vi "Lab Panel V4.8.vi"() -> ()   [LabVIEW 2013]
uses:
  <vilib>/Platform/TimedLoop/XDataNode/timing_clust.ctl
  <vilib>/Platform/TimedLoop/XDataNode/nitl_modes.ctl
  <vilib>/Platform/TimedLoop/XDataNode/wakeup.ctl
  Global 1.vi
  <vilib>/platform/TimedLoop/XDataNode/XDataNode.xnode
  <vilib>/Platform/TimedLoop/XDataNode/XDNodeRunTimeDep.lvlib
panel:
  in  "ADMIN PAGE":bool
  out "TEMP update":bool
  out "AI update":bool
  in  "Tab Control 2":T1(tab)
  out "SIG LAB05-2":T2 {"PF" format="%.2f"; "AMPS" format="%.1f"}
  out "SIG LAB05-1":T2 {"PF" format="%.2f"; "AMPS" format="%.1f"}
  out "SIG LAB04-2":T2 {"PF" format="%.2f"; "AMPS" format="%.1f"}
  out "SIG LAB04-1":T2 {"PF" format="%.2f"; "AMPS" format="%.1f"}
  out "SIG LAB03-2":T2 {"PF" format="%.2f"; "AMPS" format="%.1f"}
  out "SIG LAB03-1":T2 {"PF" format="%.2f"; "AMPS" format="%.1f"}
  out "SIG LAB02-2":T2 {"PF" format="%.2f"; "AMPS" format="%.1f"}
  in  "RUN LAB01-1":bool
  in  "O/I  LAB05-1":bool
  in  "O/I  LAB05-2":bool
  in  "O/I  LAB04-1":bool
  in  "O/I  LAB04-2":bool
  in  "O/I  LAB02-1":bool
  in  "O/I  LAB02-2":bool
  in  "O/I  LAB01-2":bool
  in  "O/I  LAB01-1":bool
  in  "O/I  LAB03-1":bool
  in  "RUN LAB05-2":bool
  in  "RUN LAB05-1":bool
  in  "RUN LAB04-2":bool
  in  "RUN LAB04-1":bool
  in  "RUN LAB03-2":bool
  in  "RUN LAB03-1":bool
  in  "RUN LAB02-2":bool
  in  "RUN LAB02-1":bool
  in  "RUN LAB01-2":bool
  in  "SELECT LAB05-2":T3(radio)
  in  "SELECT LAB05-1":T3(radio)
  in  "SELECT LAB04-2":T3(radio)
  in  "SELECT LAB04-1":T3(radio)
  in  "SELECT LAB03-2":T3(radio)
  in  "SELECT LAB03-1":T3(radio)
  in  "SELECT LAB02-2":T3(radio)
  in  "SELECT LAB02-1":T3(radio)
  in  "SELECT LAB01-2":T3(radio)
  in  "SELECT LAB01-1":T3(radio)
  in  "O/I  LAB03-2":bool
  out "SIG LAB01-1":T2 {"PF" format="%.2f"; "AMPS" format="%.1f"}
  out "SIG LAB01-2":T2 {"PF" format="%.2f"; "AMPS" format="%.1f"}
  out "SIG LAB02-1":T2 {"PF" format="%.2f"; "AMPS" format="%.1f"}
  out "DISP LAB05-2":T4 {"MINS" format="%.2g"}
  out "DISP LAB05-1":T4 {"MINS" format="%.2g"}
  out "DISP LAB04-2":T4 {"MINS" format="%.2g"}
  out "DISP LAB04-1":T4 {"MINS" format="%.2g"}
  out "DISP LAB03-2":T4 {"MINS" format="%.2g"}
  out "DISP LAB03-1":T4 {"MINS" format="%.2g"}
  in  "SET LAB05-2":T5={"NAME"="", "DESCRIPTION"="", "CYCLES"=5.0, "T-RISE mins"=0.0, "T-RISE deg C"=0.0} {"CYCLES" min=5.0 step=1.0}
  in  "SET LAB05-1":T5={"NAME"="", "DESCRIPTION"="", "CYCLES"=5.0, "T-RISE mins"=0.0, "T-RISE deg C"=0.0} {"CYCLES" min=5.0 step=1.0}
  in  "SET LAB04-2":T5={"NAME"="", "DESCRIPTION"="", "CYCLES"=5.0, "T-RISE mins"=0.0, "T-RISE deg C"=0.0} {"CYCLES" min=5.0 step=1.0}
  in  "SET LAB04-1":T5={"NAME"="", "DESCRIPTION"="", "CYCLES"=5.0, "T-RISE mins"=0.0, "T-RISE deg C"=0.0} {"CYCLES" min=5.0 step=1.0}
  in  "SET LAB03-2":T5={"NAME"="", "DESCRIPTION"="", "CYCLES"=5.0, "T-RISE mins"=0.0, "T-RISE deg C"=0.0} {"CYCLES" min=5.0 step=1.0}
  in  "SET LAB03-1":T5={"NAME"="", "DESCRIPTION"="", "CYCLES"=5.0, "T-RISE mins"=0.0, "T-RISE deg C"=0.0} {"CYCLES" min=5.0 step=1.0}
  out "DISP LAB02-2":T4 {"MINS" format="%.2g"}
  out "DISP LAB02-1":T4 {"MINS" format="%.2g"}
  in  "SET LAB02-2":T5={"NAME"="", "DESCRIPTION"="", "CYCLES"=5.0, "T-RISE mins"=0.0, "T-RISE deg C"=0.0} {"CYCLES" min=5.0 step=1.0}
  in  "SET LAB02-1":T5={"NAME"="", "DESCRIPTION"="", "CYCLES"=5.0, "T-RISE mins"=0.0, "T-RISE deg C"=0.0} {"CYCLES" min=5.0 step=1.0}
  out "RESULT LAB05-2":bool
  out "RESULT LAB05-1":bool
  out "RESULT LAB04-2":bool
  out "RESULT LAB04-1":bool
  out "RESULT LAB03-2":bool
  out "RESULT LAB03-1":bool
  out "RESULT LAB02-2":bool
  out "RESULT LAB02-1":bool
  out "RESULT LAB01-2":bool
  out "RESULT LAB01-1":bool
  in  "SET LAB01-1":T5={"NAME"="", "DESCRIPTION"="", "CYCLES"=5.0, "T-RISE mins"=0.0, "T-RISE deg C"=0.0} {"CYCLES" min=5.0 step=1.0}
  in  "SET LAB01-2":T5={"NAME"="", "DESCRIPTION"="", "CYCLES"=5.0, "T-RISE mins"=0.0, "T-RISE deg C"=0.0} {"CYCLES" min=5.0 step=1.0}
  out "DISP LAB01-1":T4 {"MINS" format="%.2g"}
  out "DISP LAB01-2":T4 {"MINS" format="%.2f"}
  out "TEMP RISE LAB05-2":cluster{"TL":dbl, "TN":dbl}
  out "TEMP RISE LAB05-1":cluster{"TL":dbl, "TN":dbl}
  out "TEMP RISE LAB04-2":cluster{"TL":dbl, "TN":dbl}
  out "TEMP RISE LAB04-1":cluster{"TL":dbl, "TN":dbl}
  out "TEMP RISE LAB03-2":cluster{"TL":dbl, "TN":dbl}
  out "TEMP RISE LAB03-1":cluster{"TL":dbl, "TN":dbl}
  out "TEMP RISE LAB02-2":cluster{"TL":dbl, "TN":dbl}
  out "TEMP RISE LAB02-1":cluster{"TL":dbl, "TN":dbl}
  out "TEMP RISE LAB01-2":cluster{"TL":dbl, "TN":dbl}
  out "TEMP RISE LAB01-1":cluster{"TL":dbl, "TN":dbl}
  in  "JIG OFF TIME (S)":dbl=2.0 min=2.0 max=10.0 step=0.5 format="%.1g"
  in  "JIG ON TIME (S)":dbl=1.0 min=1.0 max=10.0 step=0.5 format="%.1g"
  out "JIG LAB05-2":bool
  out "JIG LAB05-1":bool
  out "JIG LAB04-2":bool
  out "JIG LAB04-1":bool
  out "JIG LAB03-2":bool
  out "JIG LAB03-1":bool
  out "JIG LAB02-2":bool
  out "JIG LAB02-1":bool
  out "JIG LAB01-2":bool
  out "JIG LAB01-1":bool
  out "TEMP START LAB01-1":cluster{"TL":dbl, "TN":dbl}
  out "TEMP START LAB02-1":cluster{"TL":dbl, "TN":dbl}
  out "TEMP START LAB03-1":cluster{"TL":dbl, "TN":dbl}
  out "TEMP START LAB04-1":cluster{"TL":dbl, "TN":dbl}
  out "TEMP START LAB01-2":cluster{"TL":dbl, "TN":dbl}
  out "TEMP START LAB02-2":cluster{"TL":dbl, "TN":dbl}
  out "TEMP START LAB03-2":cluster{"TL":dbl, "TN":dbl}
  out "TEMP START LAB04-2":cluster{"TL":dbl, "TN":dbl}
  out "TEMP START LAB05-2":cluster{"TL":dbl, "TN":dbl}
  out "TEMP START LAB05-1":cluster{"TL":dbl, "TN":dbl}
  out "TEST VOLTS CHART":T6(graph)
  in  "Select  Cycle":enum32{"ON CYCLE", "OFF CYCLE"}(radio)
  out "TEST AMPS CHART":T6(graph)
  out "TEMPERATURE (N) CHART":T6(graph)
  out "TEMPERATURE (L) CHART":T6(graph)
  out "Message":string
  in  "MAIL SETTINGS":T7
  out "MAIL REPORT":string
  in  "TO (string):":string
  in  "Send Mail Now":bool
  in  "Auto Mail Send":bool
  in  "Network Directory":path
  out "CAL LAB01":T8 {"2 (TN) cal" min=0.0 step=0.01 format="%.2f"; "2 (TL) cal" min=0.0 step=0.01 format="%.2f"; "2 (PF) cal" min=0.0 step=0.01 format="%.2f"; "2 (V) cal" min=0.0 step=0.01 format="%.2f"; "2 (A) cal" min=0.0 step=0.01 format="%.2f"; "1 (TN) cal" min=0.0 step=0.01 format="%.2f"; "1 (TL) cal" min=0.0 step=0.01 format="%.2f"; "1 (PF) cal" min=0.0 step=0.01 format="%.2f"; "1 (V) cal" min=0.0 step=0.01 format="%.2f"; "1  (A) cal" min=0.0 step=0.01 format="%.2f"}
  out "CAL LAB03":T8 {"2 (TN) cal" min=0.0 step=0.01 format="%.2f"; "2 (TL) cal" min=0.0 step=0.01 format="%.2f"; "2 (PF) cal" min=0.0 step=0.01 format="%.2f"; "2 (V) cal" min=0.0 step=0.01 format="%.2f"; "2 (A) cal" min=0.0 step=0.01 format="%.2f"; "1 (TN) cal" min=0.0 step=0.01 format="%.2f"; "1 (TL) cal" min=0.0 step=0.01 format="%.2f"; "1 (PF) cal" min=0.0 step=0.01 format="%.2f"; "1 (V) cal" min=0.0 step=0.01 format="%.2f"; "1  (A) cal" min=0.0 step=0.01 format="%.2f"}
  out "CAL LAB02":T9 {"2 (TN) cal" min=0.0 step=0.01 format="%.2f"; "2 (TL) cal" min=0.0 step=0.01 format="%.2f"; "2 (PF) cal" min=0.0 step=0.01 format="%.2f"; "2 (V) cal" min=0.0 step=0.01 format="%.2f"; "2 (A) cal" min=0.0 step=0.01 format="%.2f"; "1 (TN) cal" min=0.0 step=0.01 format="%.2f"; "1 (TL) cal" min=0.0 step=0.01 format="%.2f"; "1 (PF) cal" min=0.0 step=0.01 format="%.2f"; "1 (V) cal" min=0.0 step=0.01 format="%.2f"; "1 (A) cal" min=0.0 step=0.01 format="%.2f"}
  out "CAL LAB05":T8 {"2 (TN) cal" min=0.0 step=0.01 format="%.2f"; "2 (TL) cal" min=0.0 step=0.01 format="%.2f"; "2 (PF) cal" min=0.0 step=0.01 format="%.2f"; "2 (V) cal" min=0.0 step=0.01 format="%.2f"; "2 (A) cal" min=0.0 step=0.01 format="%.2f"; "1 (TN) cal" min=0.0 step=0.01 format="%.2f"; "1 (TL) cal" min=0.0 step=0.01 format="%.2f"; "1 (PF) cal" min=0.0 step=0.01 format="%.2f"; "1 (V) cal" min=0.0 step=0.01 format="%.2f"; "1  (A) cal" min=0.0 step=0.01 format="%.2f"}
  out "CAL LAB04":T8 {"2 (TN) cal" min=0.0 step=0.01 format="%.2f"; "2 (TL) cal" min=0.0 step=0.01 format="%.2f"; "2 (PF) cal" min=0.0 step=0.01 format="%.2f"; "2 (V) cal" min=0.0 step=0.01 format="%.2f"; "2 (A) cal" min=0.0 step=0.01 format="%.2f"; "1 (TN) cal" min=0.0 step=0.01 format="%.2f"; "1 (TL) cal" min=0.0 step=0.01 format="%.2f"; "1 (PF) cal" min=0.0 step=0.01 format="%.2f"; "1 (V) cal" min=0.0 step=0.01 format="%.2f"; "1  (A) cal" min=0.0 step=0.01 format="%.2f"}
  out "calibration file error out":errorcluster
  in  "CALIBRATE":bool
  out "JIG RELAY CYCLES":T10
  out "ON L05-2":cluster{"amps":dbl, "volts":dbl, "pf":dbl}
  out "ON L05-1":cluster{"amps":dbl, "volts":dbl, "pf":dbl}
  out "FAIL LAB05-2":cluster{"LO":dbl, "HI":dbl}
  out "FAIL LAB05-1":cluster{"LO":dbl, "HI":dbl}
  out "FAIL LAB04-2":cluster{"LO":dbl, "HI":dbl}
  out "FAIL LAB04-1":cluster{"LO":dbl, "HI":dbl}
  out "FAIL LAB03-2":cluster{"LO":dbl, "HI":dbl}
  out "FAIL LAB03-1":cluster{"LO":dbl, "HI":dbl}
  out "FAIL LAB02-2":cluster{"LO":dbl, "HI":dbl}
  out "FAIL LAB02-1":cluster{"LO":dbl, "HI":dbl}
  out "FAIL LAB01-2":cluster{"LO":dbl, "HI":dbl}
  out "FAIL LAB01-1":cluster{"LO":dbl, "HI":dbl}
  out "ON L01-1":cluster{"amps":dbl, "volts":dbl, "pf":dbl}
  out "ON L01-2":cluster{"amps":dbl, "volts":dbl, "pf":dbl}
  out "ON L02-1":cluster{"amps":dbl, "volts":dbl, "pf":dbl}
  out "ON L02-2":cluster{"amps":dbl, "volts":dbl, "pf":dbl}
  out "ON L03-1":cluster{"amps":dbl, "volts":dbl, "pf":dbl}
  out "ON L03-2":cluster{"amps":dbl, "volts":dbl, "pf":dbl}
  out "ON L04-1":cluster{"amps":dbl, "volts":dbl, "pf":dbl}
  out "ON L04-2":cluster{"amps":dbl, "volts":dbl, "pf":dbl}
  out "TEMP LA05":T11
  out "TEMP LA04":T11
  out "TEMP LA03":T11
  out "TEMP LA02":T11
  out "TEMP LA01":T11
  in  "Fail Loops":dbl
  out "Save JC":bool
  out "simulate":bool
  in  "Temp Value":dbl
  in  "Temp Delay Lps":dbl
  in  "SAMPLES":dbl
  in  "RATE (Hz)":dbl
  in  "JIG TEST":T12
  in  "C drive data root dir":path
  out "run lab05-2":bool
  out "run lab05-1":bool
  out "run lab04-2":bool
  out "run lab04-1":bool
  out "run lab03-2":bool
  out "run lab03-1":bool
  out "run lab02-2":bool
  out "run lab02-1":bool
  out "run lab01-2":bool
  out "run lab01-1":bool
  in  "Tab Control":T13(tab)
  out "LAB01-2 (GRAPH)":dynamicdata(graph)
  out "LAB01-1 (GRAPH)":dynamicdata(graph)
  out "LAB02-2 (GRAPH)":dynamicdata(graph)
  out "LAB02-1 (GRAPH)":dynamicdata(graph)
  out "LAB03-2 (GRAPH)":dynamicdata(graph)
  out "LAB03-1 (GRAPH)":dynamicdata(graph)
  out "LAB04-2 (GRAPH)":dynamicdata(graph)
  out "LAB04-1 (GRAPH)":dynamicdata(graph)
  out "LAB05-2 (GRAPH)":dynamicdata(graph)
  out "LAB05-1 (GRAPH)":dynamicdata(graph)
  out "LAB05 TEMP":T14
  out "LAB04 TEMP":T14
  out "LAB02 TEMP":T14
  out "LAB01 TEMP":T14
  out "LAB03 TEMP":T14
  out "Analog Error Array":errorcluster[](array[cluster])
  out "AI loop time":dbl format="%.6g"
  out "loops":dbl
  in  "loop  delay(mS)":dbl
  out "on loops":dbl
  out "off loops":dbl
  out "jig cycle":dbl
  out "TDMS LAB01-1":refnum<k34>
  out "data file error":errorcluster
  out "TDMS LAB02-1":refnum<k34>
  out "TDMS LAB01-2":refnum<k34>
  out "TDMS LAB02-2":refnum<k34>
  out "TDMS LAB03-1":refnum<k34>
  out "TDMS LAB03-2":refnum<k34>
  out "TDMS LAB04-1":refnum<k34>
  out "TDMS LAB04-2":refnum<k34>
  out "TDMS LAB05-1":refnum<k34>
  out "TDMS LAB05-2":refnum<k34>
  out "mail control":string
  out "File Time Stamp":timestamp
  in  "stop":bool
  in  "Select COM port":refnum<visa-resource-name>="COM6"
  out "COM port":refnum<visa-resource-name>="COM6"
  # "LAB01"
  # "LAB02"
  # "LAB05"
  # "LAB03"
  # "LAB04"
  # "LAB01"
  # "LAB02"
  # "LAB03"
  # "LAB04"
  # "LAB05"
  # "JIG SET"
  # "(Enter recipients address seperated by comma)"
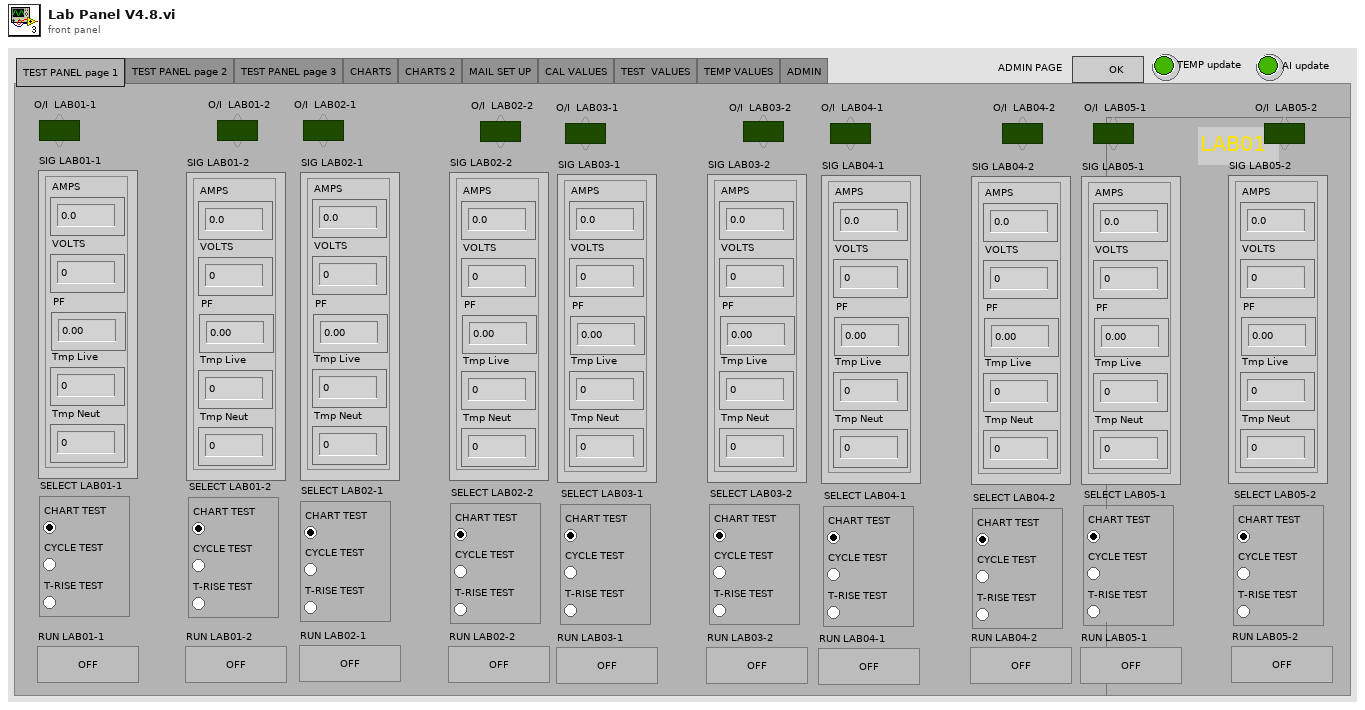
[diagram p1: front panel]
types:
  T1 = enum32{"TEST PANEL page 1", "TEST PANEL page 2", "TEST PANEL page 3", "CHARTS", "CHARTS 2", "MAIL SET UP", "CAL VALUES", "TEST  VALUES", "TEMP VALUES", "ADMIN"}
  T2 = cluster{"AMPS":dbl, "VOLTS":dbl, "PF":dbl, "Tmp Live":dbl, "Tmp Neut":dbl}
  T3 = enum32{"CHART TEST", "CYCLE TEST", "T-RISE TEST"}
  T4 = cluster{"CYCLE":dbl, "MINS":dbl, "STATUS":string}
  T5 = cluster{"NAME":string, "DESCRIPTION":string, "CYCLES":dbl, "T-RISE mins":dbl, "T-RISE deg C":dbl}
  T6 = cluster{"AMPS":dbl, "AMPS":dbl, "AMPS":dbl, "AMPS":dbl, "AMPS":dbl, "AMPS":dbl, "AMPS":dbl, "AMPS":dbl, "AMPS":dbl, "AMPS":dbl}
  T7 = cluster{"OUT SERVER ADDRESS":string, "FROM ACCOUNT":string, "USER NAME":string, "PASSWORD":string, "TEST MAIL":bool, "TEST MAIL STATUS":string, "mail error":errorcluster}
  T8 = cluster{"1  (A) cal":dbl, "1 (V) cal":dbl, "1 (PF) cal":dbl, "1 (TL) cal":dbl, "1 (TN) cal":dbl, "2 (A) cal":dbl, "2 (V) cal":dbl, "2 (PF) cal":dbl, "2 (TL) cal":dbl, "2 (TN) cal":dbl}
  T9 = cluster{"1 (A) cal":dbl, "1 (V) cal":dbl, "1 (PF) cal":dbl, "1 (TL) cal":dbl, "1 (TN) cal":dbl, "2 (A) cal":dbl, "2 (V) cal":dbl, "2 (PF) cal":dbl, "2 (TL) cal":dbl, "2 (TN) cal":dbl}
  T10 = cluster{"LAB01-1":dbl, "LAB01-2":dbl, "LAB02-1":dbl, "LAB02-2":dbl, "LAB03-1":dbl, "LAB03-2":dbl, "LAB04-1":dbl, "LAB04-2":dbl, "LAB05-1":dbl, "LAB05-2":dbl}
  T11 = cluster{"TL-1":dbl, "TN-1":dbl, "TL-2":dbl, "TN-2":dbl, "TL -1COUNT":dbl, "TN-1 COUNT":dbl, "TL-2 COUNT":dbl, "TN-2 COUNT":dbl}
  T12 = cluster{" LAB01-1":bool, " LAB01-2":bool, "LAB02-1":bool, " LAB02-2":bool, "LAB03-1":bool, "LAB03-2":bool, "LAB04-1":bool, "LAB04-2":bool, "LAB05-1":bool, "LAB05-2":bool}
  T13 = enum32{"LAB01", "LAB02", "LAB03", "LAB04", "LAB05", "TEMPERATURE", "ERROR"}
  T14 = cluster{"T1 Live":dbl, "T1 Neut":dbl, "T2 Live":dbl, "T2 Neut":dbl, "ID":dbl, "ER":dbl}
  T15 = enum8{"Enabled", "Disabled", "Disabled and Grayed Out"}
  T16 = typedef "XDNodeRunTimeDep.lvlib/timing_clust.ctl" = cluster{"Expected End [f-1]":u64, "Actual End [f-1]":u64, "Finished Late? [f-1]":bool, "Expected End [i-1]":u64, "Actual End [i-1]":u64, "Finished Late? [i-1]":bool, "Expected Start [i]":u64, "Actual Start [i]":u64, "Expected Start [f]":u64, "Actual Start [f]":u64, "Source Name":string, "Structure Name":string, "Period":i64, "Deadline":i64, "Offset":i64, "Start":i64, "Priority":i32, "Timeout":i32, "Mode":T17, "Wakeup Reason":T18, "Error":errorcluster, "Source Type":string, "Secondary Source Type":string, "Global End Time":u64, "Global Start Time":u64, "Frame Duration":u64, "Iteration Duration":u64, "Assigned CPU":i32, "I/O Scan Engine Mode":u32}
  T17 = typedef "XDNodeRunTimeDep.lvlib/nitl_modes.ctl" = enum32{"No Change", "Process missed periods, maintain original phase", "Discard missed periods, maintain original phase", "Process missed periods, ignore original phase", "Discard missed periods, ignore original phase"}
  T18 = typedef "XDNodeRunTimeDep.lvlib/wakeup.ctl" = enum32{"Normal", "Aborted", "Asynchronous wakeup", "Timing source error", "Timed loop error", "Timeout"}
  T19 = enum16{"open", "open or create", "create or replace", "create", "open (read-only)"}
  T20 = enum16{"open", "replace", "create", "open or create", "replace or create", "replace or create with confirmation"}
  T21 = cluster{"SET LAB01-1":cluster{"NAME":string, "DESCRIPTION":string, "CYCLES":dbl, "T-RISE mins":dbl, "T-RISE deg C":dbl}, "SET LAB01-2":cluster{"NAME":string, "DESCRIPTION":string, "CYCLES":dbl, "T-RISE mins":dbl, "T-RISE deg C":dbl}, "SET LAB02-1":cluster{"NAME":string, "DESCRIPTION":string, "CYCLES":dbl, "T-RISE mins":dbl, "T-RISE deg C":dbl}, "SET LAB02-2":cluster{"NAME":string, "DESCRIPTION":string, "CYCLES":dbl, "T-RISE mins":dbl, "T-RISE deg C":dbl}, "SET LAB03-1":cluster{"NAME":string, "DESCRIPTION":string, "CYCLES":dbl, "T-RISE mins":dbl, "T-RISE deg C":dbl}, "SET LAB03-2":cluster{"NAME":string, "DESCRIPTION":string, "CYCLES":dbl, "T-RISE mins":dbl, "T-RISE deg C":dbl}, "SET LAB04-1":cluster{"NAME":string, "DESCRIPTION":string, "CYCLES":dbl, "T-RISE mins":dbl, "T-RISE deg C":dbl}, "SET LAB04-2":cluster{"NAME":string, "DESCRIPTION":string, "CYCLES":dbl, "T-RISE mins":dbl, "T-RISE deg C":dbl}, "SET LAB05-1":cluster{"NAME":string, "DESCRIPTION":string, "CYCLES":dbl, "T-RISE mins":dbl, "T-RISE deg C":dbl}, "SET LAB05-2":cluster{"NAME":string, "DESCRIPTION":string, "CYCLES":dbl, "T-RISE mins":dbl, "T-RISE deg C":dbl}, "Network Directory":path, "C drive data root dir":path, "RATE (Hz)":dbl, "SAMPLES":dbl, "Select COM port":refnum<visa-resource-name>, "Temp Delay Lps":dbl, "Temp Value":dbl, "Fail Loops":dbl}
  T22 = cluster{"MAIL SETTINGS":cluster{"OUT SERVER ADDRESS":string, "FROM ACCOUNT":string, "USER NAME":string, "PASSWORD":string, "TEST MAIL":bool, "TEST MAIL STATUS":string, "mail error":errorcluster}, "Auto Mail Send":bool, string}
  T23 = cluster{"T1":dbl, "T2":dbl, "T3":dbl, "T4":dbl, "ID":dbl, "ER":dbl}
  T24 = cluster{"TP1-L":dbl, "TP1-N":dbl, "TP2-L":dbl, "TP2-N":dbl, "TP1-L COUNT":dbl, "TP1-N COUNT":dbl, "TP2-L COUNT":dbl, "TP2-N COUNT":dbl}
  T25 = cluster{"LAB01-1 (A)":dbl, "LAB01-1 (V)":dbl, "LAB01-1 (PF)":dbl, "LAB01-2 (A)":dbl, "LAB01-2 (V)":dbl, "LAB01-2 (PF)":dbl}
  T26 = cluster{"LAB02-1 (A)":dbl, "LAB02-1 (V)":dbl, "LAB02-1 (PF)":dbl, "LAB02-2 (A)":dbl, "LAB02-2 (V)":dbl, "LAB02-2 (PF)":dbl}
  T27 = cluster{"LAB03-1 (A)":dbl, "LAB03-1 (V)":dbl, "LAB03-1 (PF)":dbl, "LAB03-2 (A)":dbl, "LAB03-2 (V)":dbl, "LAB03-2 (PF)":dbl}
  T28 = cluster{"LAB04-1 (A)":dbl, "LAB04-1 (V)":dbl, "LAB04-1 (PF)":dbl, "LAB04-2 (A)":dbl, "LAB04-2 (V)":dbl, "LAB04-2 (PF)":dbl}
  T29 = cluster{"LAB05-1 (A)":dbl, "LAB05-1 (V)":dbl, "LAB05-1 (PF)":dbl, "LAB05-2 (A)":dbl, "LAB05-2 (V)":dbl, "LAB05-2 (PF)":dbl}
  T30 = cluster{"VOLTS":dbl, "VOLTS":dbl, "VOLTS":dbl, "VOLTS":dbl, "VOLTS":dbl, "VOLTS":dbl, "VOLTS":dbl, "VOLTS":dbl, "VOLTS":dbl, "VOLTS":dbl}
  T31 = cluster{"Tmp Live":dbl, "Tmp Live":dbl, "Tmp Live":dbl, "Tmp Live":dbl, "Tmp Live":dbl, "Tmp Live":dbl, "Tmp Live":dbl, "Tmp Live":dbl, "Tmp Live":dbl, "Tmp Live":dbl}
  T32 = cluster{"Tmp Neut":dbl, "Tmp Neut":dbl, "Tmp Neut":dbl, "Tmp Neut":dbl, "Tmp Neut":dbl, "Tmp Neut":dbl, "Tmp Neut":dbl, "Tmp Neut":dbl, "Tmp Neut":dbl, "Tmp Neut":dbl}
  T33 = cluster{"FAIL LAB01-1":cluster{"LO":dbl, "HI":dbl}, "SIG LAB01-1":cluster{"AMPS":dbl, "VOLTS":dbl, "PF":dbl, "Tmp Live":dbl, "Tmp Neut":dbl}, "TEMP START LAB01-1":cluster{"TL":dbl, "TN":dbl}, "DISP LAB01-1":cluster{"CYCLE":dbl, "MINS":dbl, "STATUS":string}, "SET LAB01-1":cluster{"NAME":string, "DESCRIPTION":string, "CYCLES":dbl, "T-RISE mins":dbl, "T-RISE deg C":dbl}, "TDMS LAB01-1":refnum<k34>}
  T34 = cluster{"FAIL LAB01-2":cluster{"LO":dbl, "HI":dbl}, "SIG LAB01-2":cluster{"AMPS":dbl, "VOLTS":dbl, "PF":dbl, "Tmp Live":dbl, "Tmp Neut":dbl}, "TEMP START LAB01-2":cluster{"TL":dbl, "TN":dbl}, "DISP LAB01-2":cluster{"CYCLE":dbl, "MINS":dbl, "STATUS":string}, "SET LAB01-2":cluster{"NAME":string, "DESCRIPTION":string, "CYCLES":dbl, "T-RISE mins":dbl, "T-RISE deg C":dbl}, "TDMS LAB01-2":refnum<k34>}
  T35 = cluster{"FAIL LAB02-1":cluster{"LO":dbl, "HI":dbl}, "SIG LAB02-1":cluster{"AMPS":dbl, "VOLTS":dbl, "PF":dbl, "Tmp Live":dbl, "Tmp Neut":dbl}, "TEMP START LAB02-1":cluster{"TL":dbl, "TN":dbl}, "DISP LAB02-1":cluster{"CYCLE":dbl, "MINS":dbl, "STATUS":string}, "SET LAB02-1":cluster{"NAME":string, "DESCRIPTION":string, "CYCLES":dbl, "T-RISE mins":dbl, "T-RISE deg C":dbl}, "TDMS LAB02-1":refnum<k34>}
  T36 = cluster{"FAIL LAB02-2":cluster{"LO":dbl, "HI":dbl}, "SIG LAB02-2":cluster{"AMPS":dbl, "VOLTS":dbl, "PF":dbl, "Tmp Live":dbl, "Tmp Neut":dbl}, "TEMP START LAB02-2":cluster{"TL":dbl, "TN":dbl}, "DISP LAB02-2":cluster{"CYCLE":dbl, "MINS":dbl, "STATUS":string}, "SET LAB02-2":cluster{"NAME":string, "DESCRIPTION":string, "CYCLES":dbl, "T-RISE mins":dbl, "T-RISE deg C":dbl}, "TDMS LAB02-2":refnum<k34>}
  T37 = cluster{"FAIL LAB03-1":cluster{"LO":dbl, "HI":dbl}, "SIG LAB03-1":cluster{"AMPS":dbl, "VOLTS":dbl, "PF":dbl, "Tmp Live":dbl, "Tmp Neut":dbl}, "TEMP START LAB03-1":cluster{"TL":dbl, "TN":dbl}, "DISP LAB03-1":cluster{"CYCLE":dbl, "MINS":dbl, "STATUS":string}, "SET LAB03-1":cluster{"NAME":string, "DESCRIPTION":string, "CYCLES":dbl, "T-RISE mins":dbl, "T-RISE deg C":dbl}, "TDMS LAB03-1":refnum<k34>}
  T38 = cluster{"FAIL LAB03-2":cluster{"LO":dbl, "HI":dbl}, "SIG LAB03-2":cluster{"AMPS":dbl, "VOLTS":dbl, "PF":dbl, "Tmp Live":dbl, "Tmp Neut":dbl}, "TEMP START LAB03-2":cluster{"TL":dbl, "TN":dbl}, "DISP LAB03-2":cluster{"CYCLE":dbl, "MINS":dbl, "STATUS":string}, "SET LAB03-2":cluster{"NAME":string, "DESCRIPTION":string, "CYCLES":dbl, "T-RISE mins":dbl, "T-RISE deg C":dbl}, "TDMS LAB03-2":refnum<k34>}
  T39 = cluster{"FAIL LAB04-1":cluster{"LO":dbl, "HI":dbl}, "SIG LAB04-1":cluster{"AMPS":dbl, "VOLTS":dbl, "PF":dbl, "Tmp Live":dbl, "Tmp Neut":dbl}, "TEMP START LAB04-1":cluster{"TL":dbl, "TN":dbl}, "DISP LAB04-1":cluster{"CYCLE":dbl, "MINS":dbl, "STATUS":string}, "SET LAB04-1":cluster{"NAME":string, "DESCRIPTION":string, "CYCLES":dbl, "T-RISE mins":dbl, "T-RISE deg C":dbl}, "TDMS LAB04-1":refnum<k34>}
  T40 = cluster{"FAIL LAB04-2":cluster{"LO":dbl, "HI":dbl}, "SIG LAB04-2":cluster{"AMPS":dbl, "VOLTS":dbl, "PF":dbl, "Tmp Live":dbl, "Tmp Neut":dbl}, "TEMP START LAB04-2":cluster{"TL":dbl, "TN":dbl}, "DISP LAB04-2":cluster{"CYCLE":dbl, "MINS":dbl, "STATUS":string}, "SET LAB04-2":cluster{"NAME":string, "DESCRIPTION":string, "CYCLES":dbl, "T-RISE mins":dbl, "T-RISE deg C":dbl}, "TDMS LAB04-2":refnum<k34>}
  T41 = cluster{"FAIL LAB05-1":cluster{"LO":dbl, "HI":dbl}, "SIG LAB05-1":cluster{"AMPS":dbl, "VOLTS":dbl, "PF":dbl, "Tmp Live":dbl, "Tmp Neut":dbl}, "TEMP START LAB05-1":cluster{"TL":dbl, "TN":dbl}, "DISP LAB05-1":cluster{"CYCLE":dbl, "MINS":dbl, "STATUS":string}, "SET LAB05-1":cluster{"NAME":string, "DESCRIPTION":string, "CYCLES":dbl, "T-RISE mins":dbl, "T-RISE deg C":dbl}, "TDMS LAB05-1":refnum<k34>}
  T42 = cluster{"FAIL LAB05-2":cluster{"LO":dbl, "HI":dbl}, "SIG LAB05-2":cluster{"AMPS":dbl, "VOLTS":dbl, "PF":dbl, "Tmp Live":dbl, "Tmp Neut":dbl}, "TEMP START LAB05-2":cluster{"TL":dbl, "TN":dbl}, "DISP LAB05-2":cluster{"CYCLE":dbl, "MINS":dbl, "STATUS":string}, "SET LAB05-2":cluster{"NAME":string, "DESCRIPTION":string, "CYCLES":dbl, "T-RISE mins":dbl, "T-RISE deg C":dbl}, "TDMS LAB05-2":refnum<k34>}
  T43 = cluster{"MAIL SETTINGS":cluster{"OUT SERVER ADDRESS":string, "FROM ACCOUNT":string, "USER NAME":string, "PASSWORD":string, "TEST MAIL":bool, "TEST MAIL STATUS":string, "mail error":errorcluster}, "Auto Mail Send":bool, "TO (string):":string}
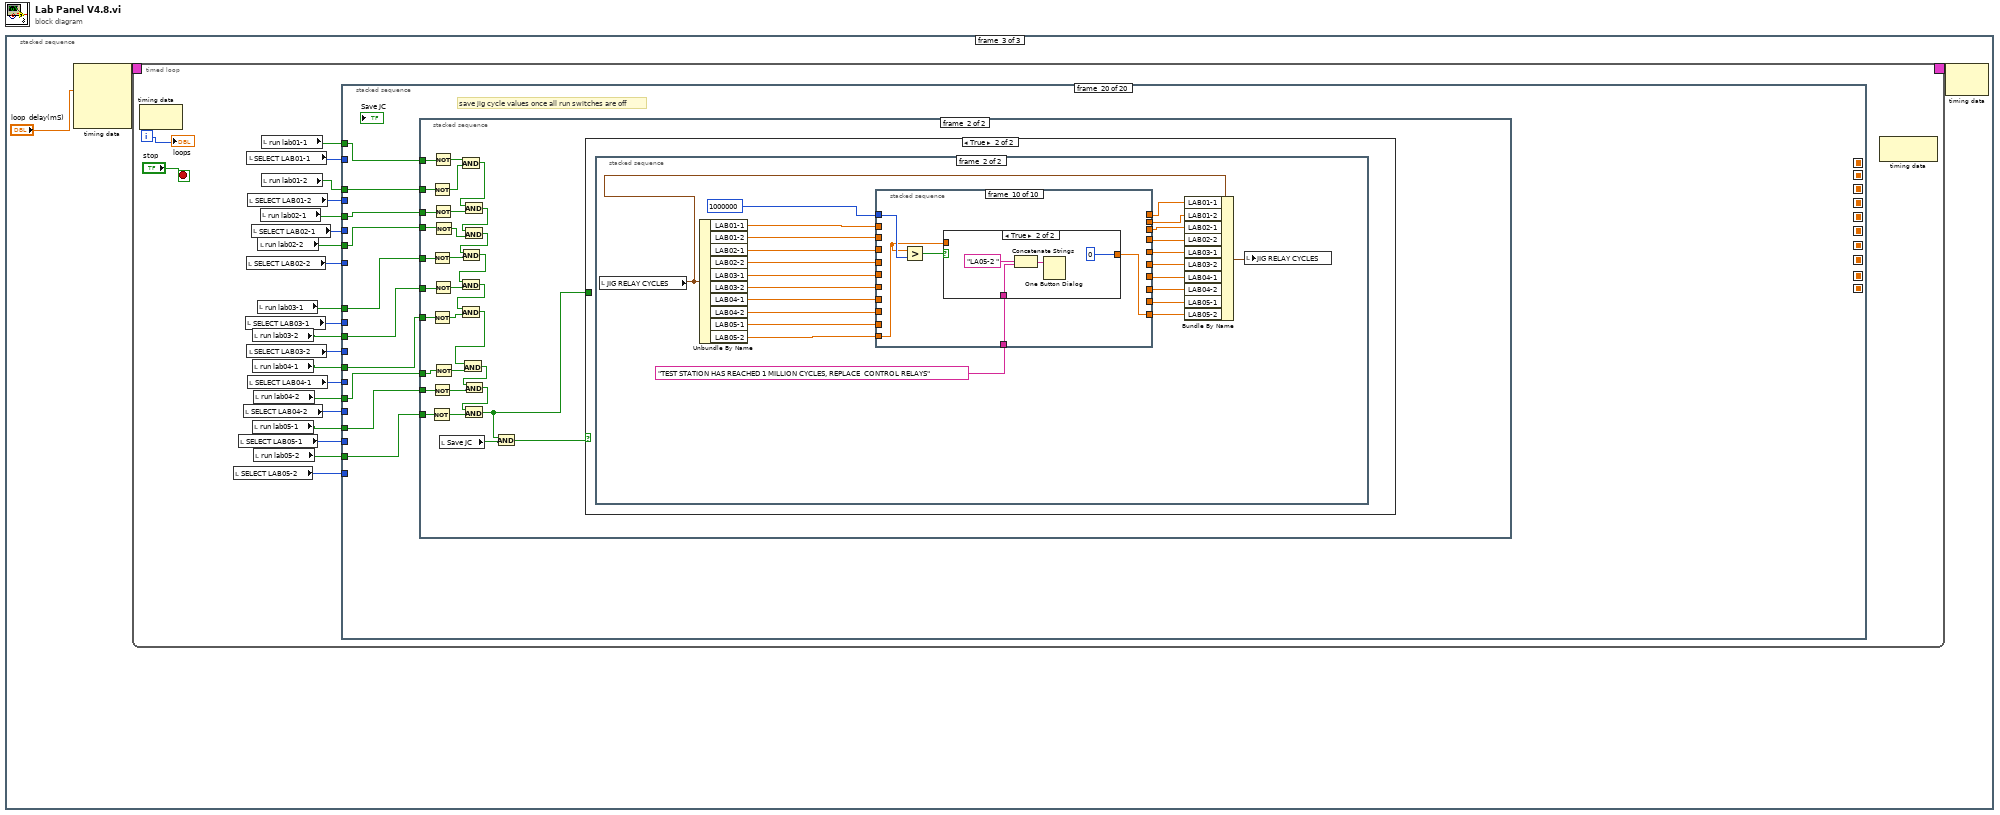
[diagram p0: block diagram]
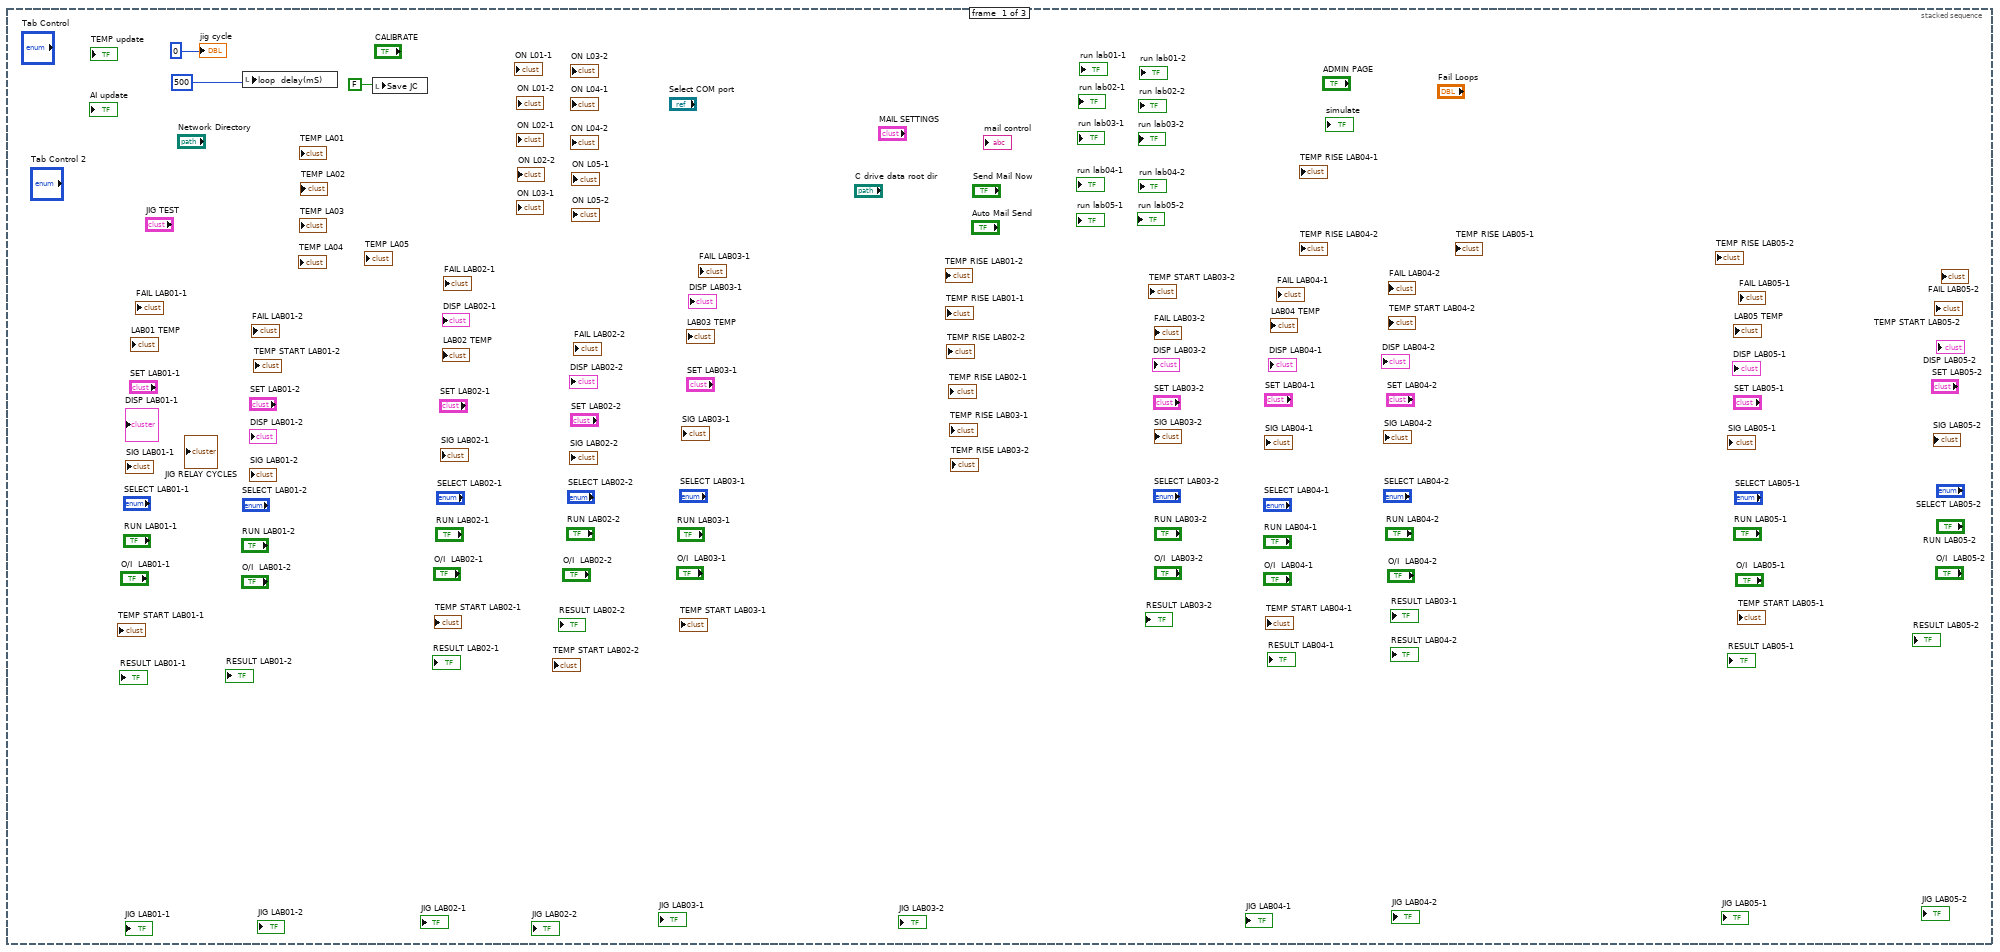
[diagram p2: hidden frame]
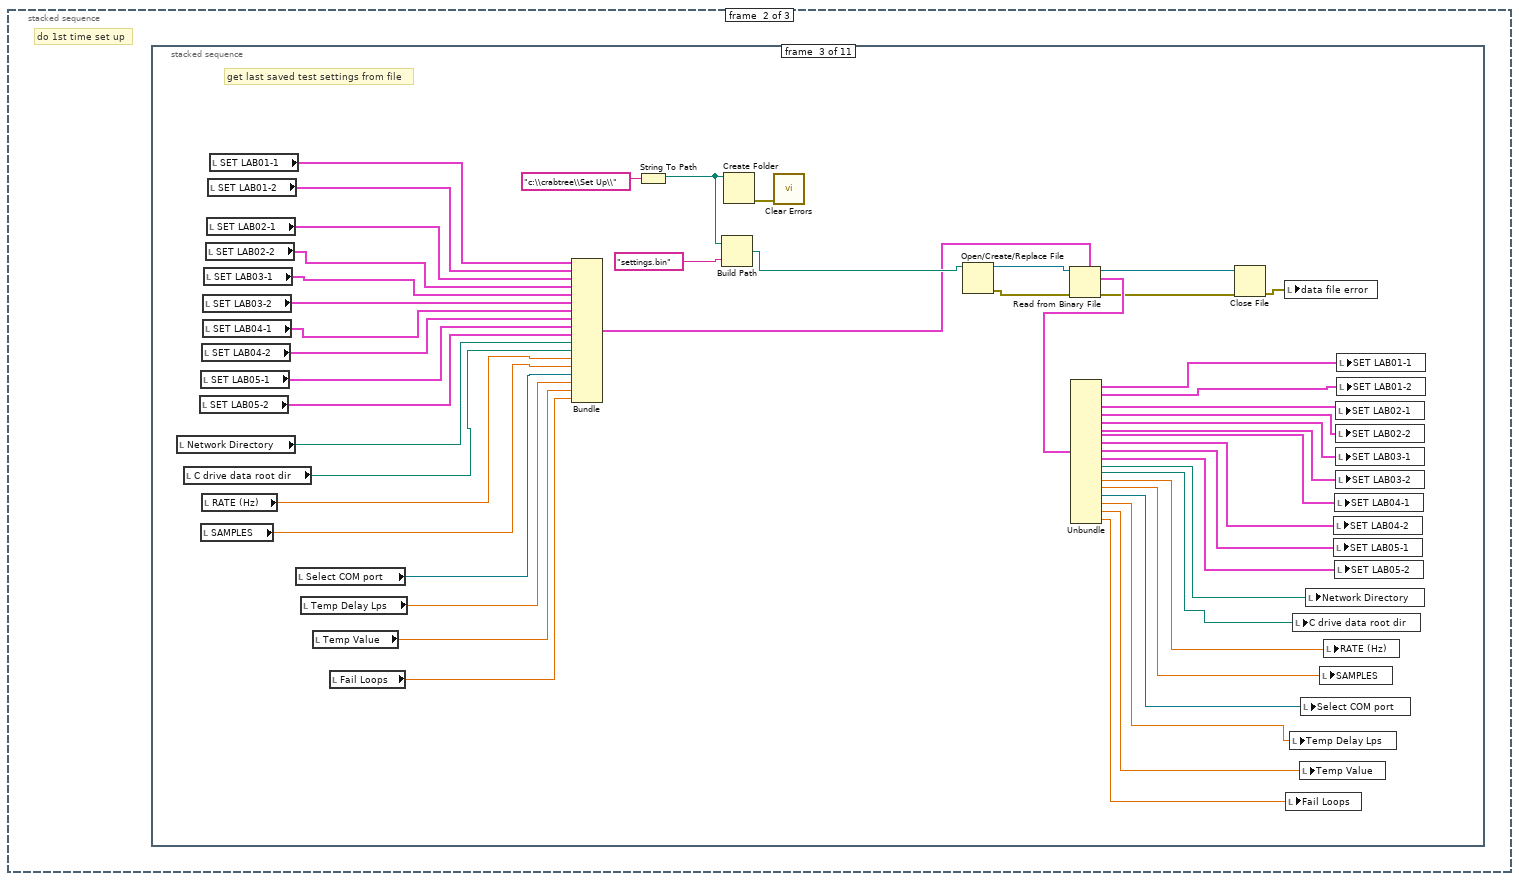
[diagram p3: hidden frame]
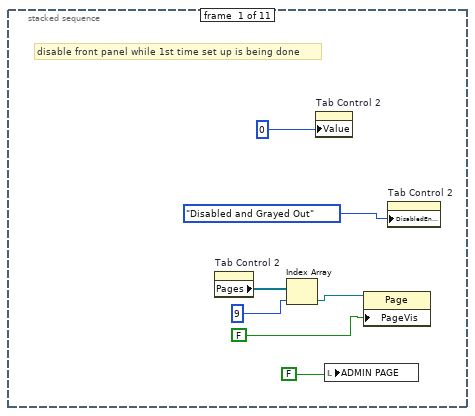
[diagram p4: hidden frame]
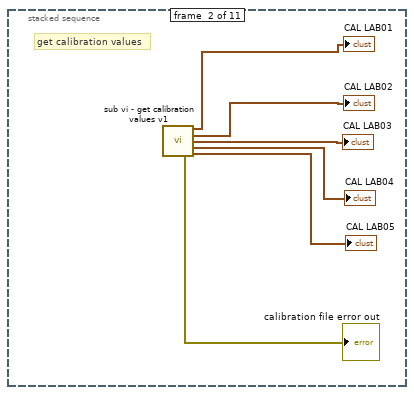
[diagram p5: hidden frame]
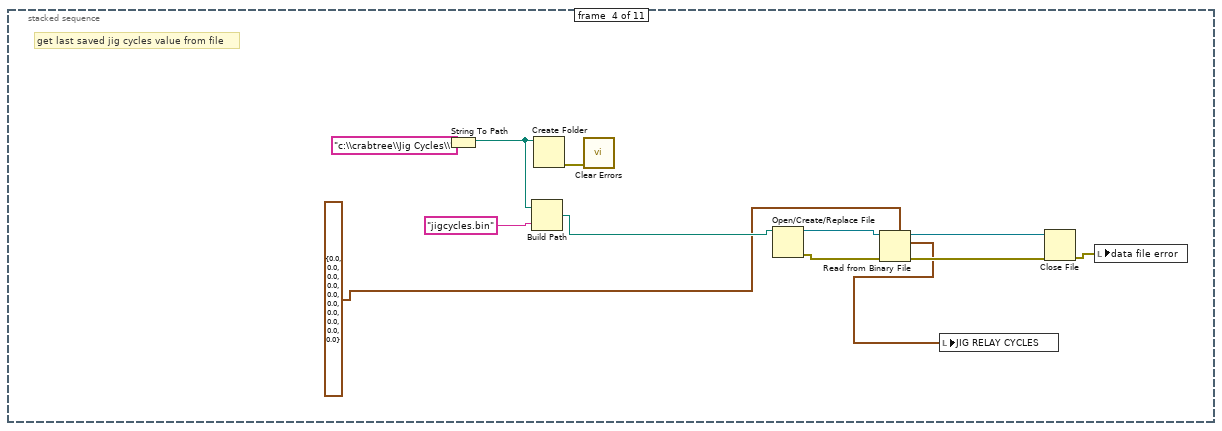
[diagram p6: hidden frame]
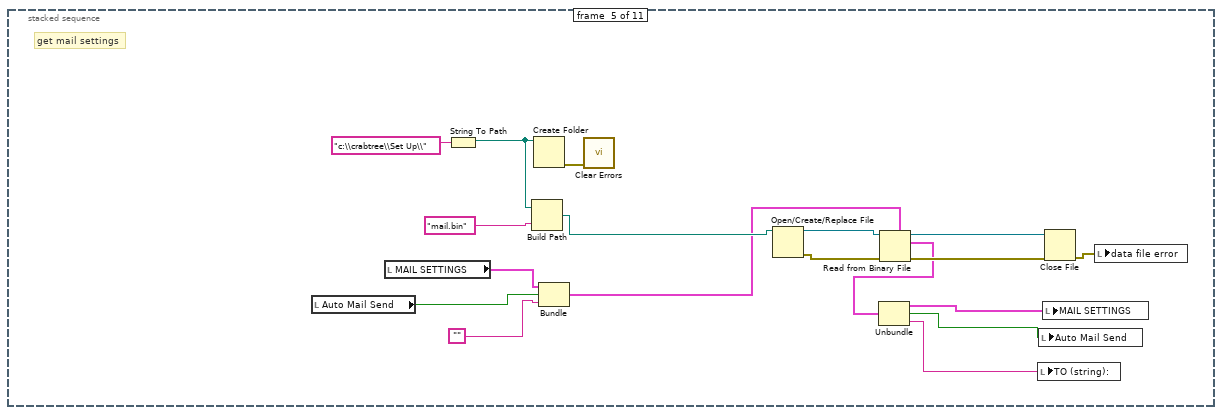
[diagram p7: hidden frame]
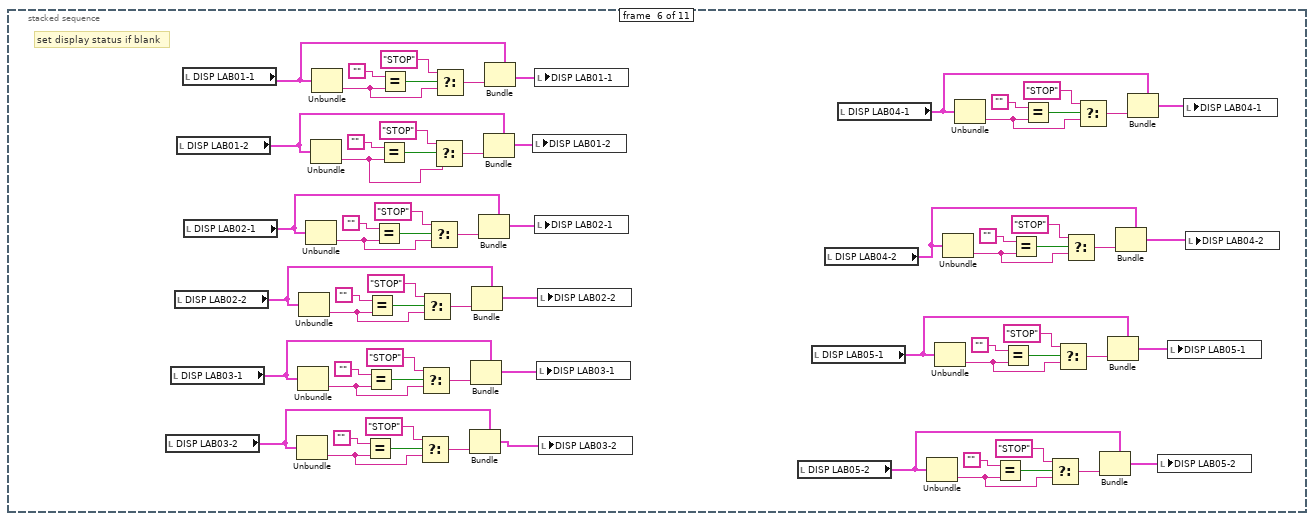
[diagram p8: hidden frame]
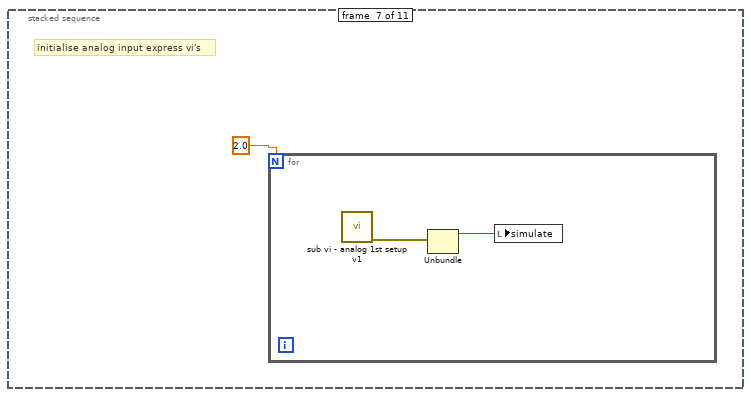
[diagram p9: hidden frame]
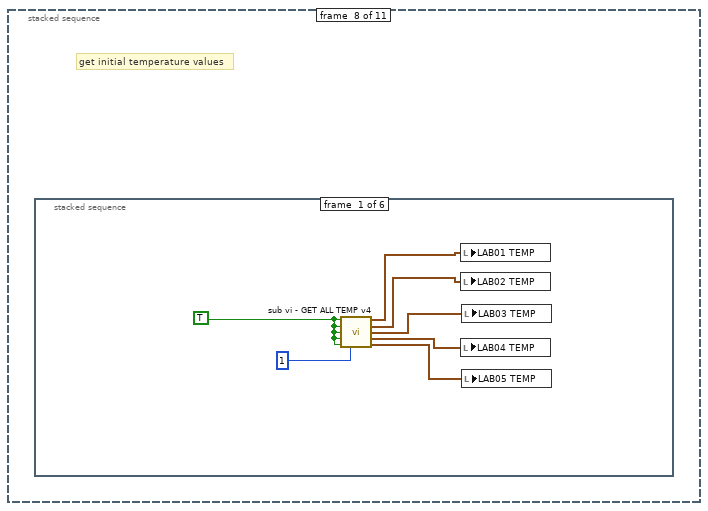
[diagram p10: hidden frame]
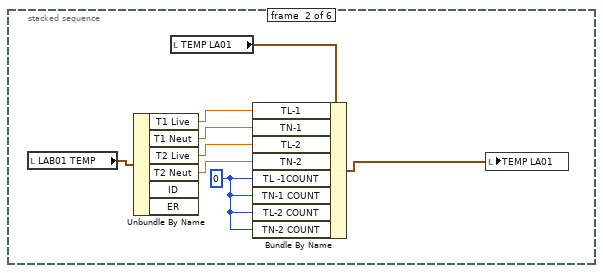
[diagram p11: hidden frame]
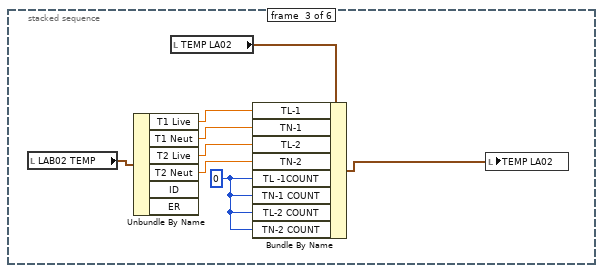
[diagram p12: hidden frame]
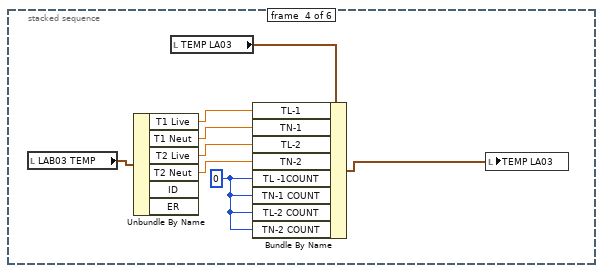
[diagram p13: hidden frame]
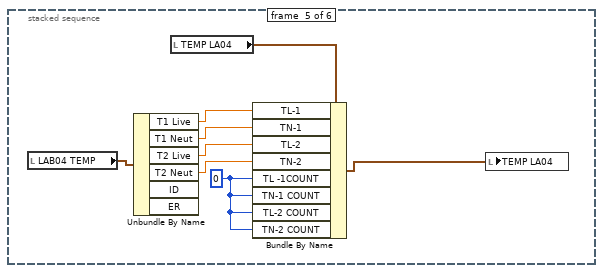
[diagram p14: hidden frame]
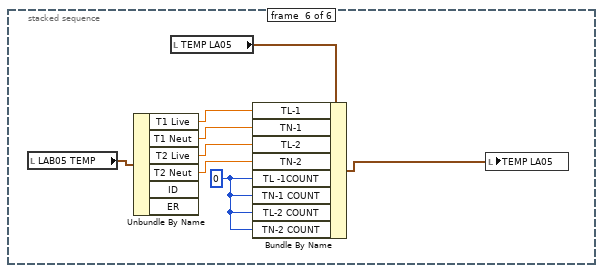
[diagram p15: hidden frame]
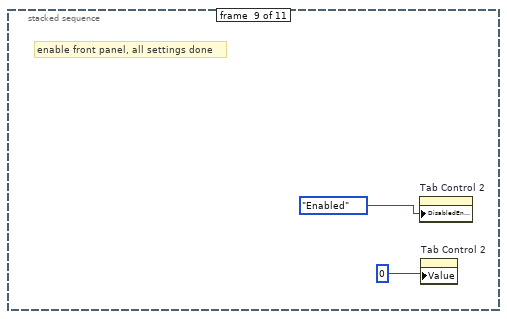
[diagram p16: hidden frame]
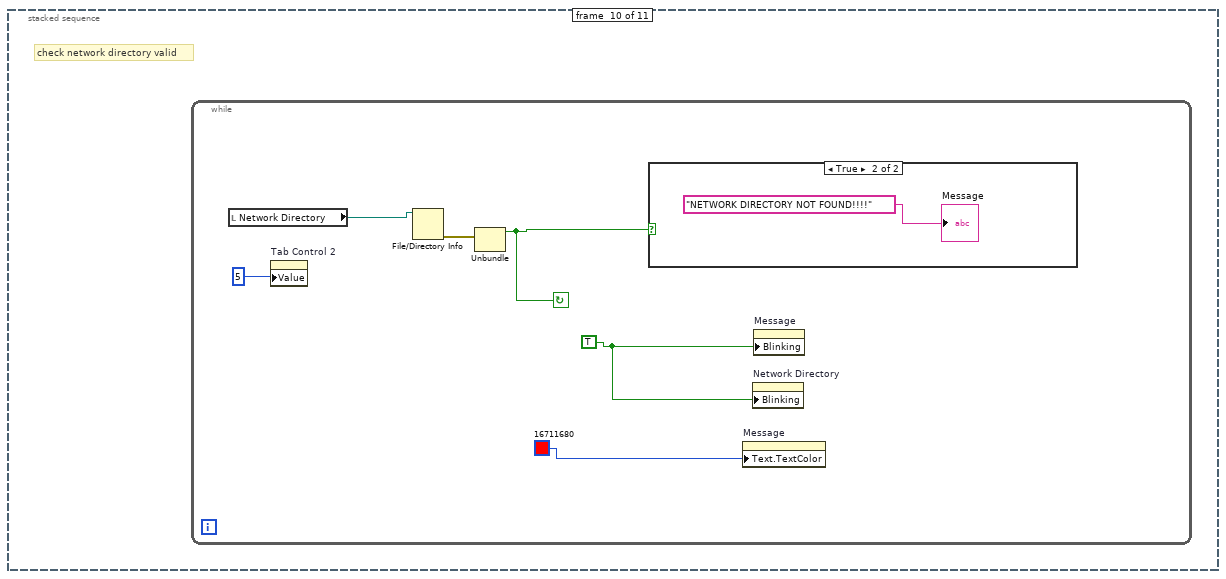
[diagram p17: hidden frame]
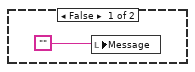
[diagram p18: hidden frame]
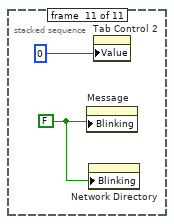
[diagram p19: hidden frame]
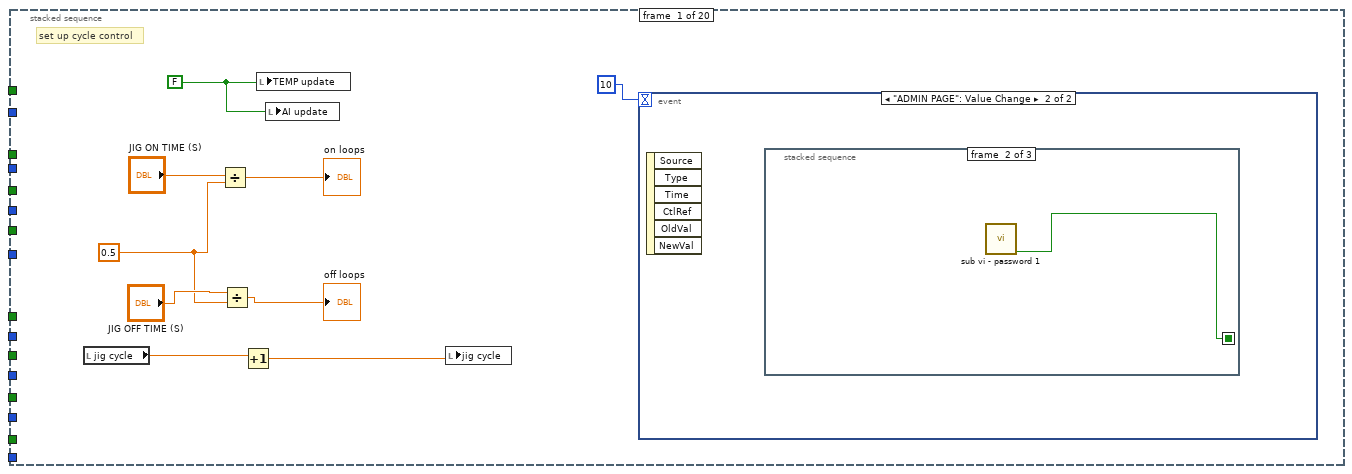
[diagram p20: hidden frame]
diagram:
  n1 = stacked-sequence {
    frame #0 {
      n2 = local write "loop  delay(mS)"(500) -> ()
      n3 = local write "Save JC"(FALSE) -> ()
      "jig cycle" <- 0
    }
    frame #1 {
      # "do 1st time set up"
      n4 = stacked-sequence {
        frame #0 {
          # "disable front panel while 1st time set up is being done"
          n5 = property on="Tab Control 2" class="TabCtl (strict)"() -> ("Pages"=w9:refnum<vi>[])  [unwired: 2 in, 2 out]
          n6 = Index Array(array=w9, index=9) -> (element=w7:refnum<vi>)
          n7 = property on="Tab Control 2" class="TabCtl (strict)"("Value"=0) -> ()  [unwired: 2 in, 2 out]
          n8 = local write "ADMIN PAGE"(FALSE) -> ()
          n9 = property class="Page"(reference=w7, "PageVis"=FALSE) -> ()  [unwired: 1 in, 2 out]
          n10 = property on="Tab Control 2" class="TabCtl (strict)"("DisabledEnum"=T15."Disabled and Grayed Out" ("Disabled")) -> ()  [unwired: 2 in, 2 out]
        }
        frame #1 {
          # "get calibration values"
          n11 = call "sub vi - get calibration values v1.vi"() -> ("LAB01 (CAL)"=→"CAL LAB01":T8, "LAB02 (CAL)"=→"CAL LAB02":T9, "LAB03 (CAL)"=→"CAL LAB03":T8, "LAB04 (CAL)"=→"CAL LAB04":T8, "calibration file error out"=→"calibration file error out":errorcluster, "LAB05 (CAL)"=→"CAL LAB05":T8)  [unwired: 10 in]
        }
        frame #2 {
          # "get last saved test settings from file"
          n12 = local read "Network Directory"() -> (w31:path)
          n13 = local read "C drive data root dir"() -> (w29:path)
          n14 = local read "SET LAB05-2"() -> (w61:T5)
          n15 = local read "SET LAB05-1"() -> (w62:T5)
          n16 = local read "SAMPLES"() -> (w27:dbl)
          n17 = local read "SET LAB04-2"() -> (w63:T5)
          n18 = local read "RATE (Hz)"() -> (w28:dbl)
          n19 = local read "SET LAB03-2"() -> (w60:T5)
          n20 = local read "SET LAB04-1"() -> (w64:T5)
          n21 = local read "SET LAB03-1"() -> (w59:T5)
          n22 = local read "SET LAB02-2"() -> (w58:T5)
          n23 = local read "SET LAB02-1"() -> (w57:T5)
          n24 = local read "SET LAB01-2"() -> (w56:T5)
          n25 = local read "SET LAB01-1"() -> (w55:T5)
          n26 = local read "Select COM port"() -> (w23:refnum<visa-resource-name>)
          n27 = local read "Temp Delay Lps"() -> (w22:dbl)
          n28 = local read "Temp Value"() -> (w21:dbl)
          n29 = local read "Fail Loops"() -> (w18:dbl)
          n30 = Bundle("SET LAB01-1"=w55, "SET LAB01-2"=w56, "SET LAB02-1"=w57, "SET LAB02-2"=w58, "SET LAB03-1"=w59, "SET LAB03-2"=w60, "SET LAB04-1"=w64, "SET LAB04-2"=w63, "SET LAB05-1"=w62, "SET LAB05-2"=w61, "Network Directory"=w31, "C drive data root dir"=w29, "RATE (Hz)"=w28, "SAMPLES"=w27, "Select COM port"=w23, "Temp Delay Lps"=w22, "Temp Value"=w21, "Fail Loops"=w18) -> (w48:T21)  [unwired: 1 in]
          n31 = String To Path(string="c:\\crabtree\\Set Up\\") -> (path=w52:path)
          n32 = Build Path(base path=w52, name or relative path="settings.bin") -> (appended path=w50:path)
          n33 = Create Folder(path (use dialog)=w52) -> (error out=w54:errorcluster)  [unwired: 2 in, 2 out]
          n34 = call <vilib>:"Clear Errors.vi"("error in (no error)"=w54) -> ()  [unwired: 6 in, 1 out]
          n35 = Open/Create/Replace File(file path (use dialog)=w50) -> (refnum out=w47:refnum<file>, error out=w49:errorcluster)  [unwired: 5 in, 1 out]
          n36 = Read from Binary File(5:w48, 8:w49, 11:w47) -> (0:w44:errorcluster, 2:w46:T21, 3:w45:refnum<file>)  [unwired: 3 in, 1 out]
          n37 = Unbundle(w46) -> ("SET LAB01-1"=w42:T5, "SET LAB01-2"=w41:T5, "SET LAB02-1"=w40:T5, "SET LAB02-2"=w39:T5, "SET LAB03-1"=w38:T5, "SET LAB03-2"=w37:T5, "SET LAB04-1"=w36:T5, "SET LAB04-2"=w35:T5, "SET LAB05-1"=w34:T5, "SET LAB05-2"=w33:T5, "Network Directory"=w32:path, "C drive data root dir"=w30:path, "RATE (Hz)"=w25:dbl, "SAMPLES"=w26:dbl, "Select COM port"=w24:refnum<visa-resource-name>, "Temp Delay Lps"=w20:dbl, "Temp Value"=w19:dbl, "Fail Loops"=w17:dbl)
          n38 = Close File(refnum=w45, error in=w44) -> (error out=w43:errorcluster)  [unwired: 1 out]
          n39 = local write "data file error"(w43) -> ()
          n40 = local write "Fail Loops"(w17) -> ()
          n41 = local write "Temp Delay Lps"(w20) -> ()
          n42 = local write "C drive data root dir"(w30) -> ()
          n43 = local write "Temp Value"(w19) -> ()
          n44 = local write "Select COM port"(w24) -> ()
          n45 = local write "Network Directory"(w32) -> ()
          n46 = local write "SAMPLES"(w26) -> ()
          n47 = local write "RATE (Hz)"(w25) -> ()
          n48 = local write "SET LAB04-2"(w35) -> ()
          n49 = local write "SET LAB05-1"(w34) -> ()
          n50 = local write "SET LAB04-1"(w36) -> ()
          n51 = local write "SET LAB05-2"(w33) -> ()
          n52 = local write "SET LAB02-1"(w40) -> ()
          n53 = local write "SET LAB02-2"(w39) -> ()
          n54 = local write "SET LAB03-1"(w38) -> ()
          n55 = local write "SET LAB03-2"(w37) -> ()
          n56 = local write "SET LAB01-1"(w42) -> ()
          n57 = local write "SET LAB01-2"(w41) -> ()
        }
        frame #3 {
          # "get last saved jig cycles value from file"
          n58 = String To Path(string="c:\\crabtree\\Jig Cycles\\") -> (path=w74:path)
          n59 = Build Path(base path=w74, name or relative path="jigcycles.bin") -> (appended path=w72:path)
          n60 = Create Folder(path (use dialog)=w74) -> (error out=w76:errorcluster)  [unwired: 2 in, 2 out]
          n61 = call <vilib>:"Clear Errors.vi"("error in (no error)"=w76) -> ()  [unwired: 6 in, 1 out]
          n62 = Open/Create/Replace File(file path (use dialog)=w72) -> (refnum out=w70:refnum<file>, error out=w71:errorcluster)  [unwired: 5 in, 1 out]
          n63 = Read from Binary File(5:T10 {"LAB01-1"=0.0, "LAB01-2"=0.0, "LAB02-1"=0.0, "LAB02-2"=0.0, "LAB03-1"=0.0, "LAB03-2"=0.0, "LAB04-1"=0.0, "LAB04-2"=0.0, "LAB05-1"=0.0, "LAB05-2"=0.0} ("JIG RELAY CYCLES"), 8:w71, 11:w70) -> (0:w68:errorcluster, 2:w65:T10, 3:w69:refnum<file>)  [unwired: 3 in, 1 out]
          n64 = local write "JIG RELAY CYCLES"(w65) -> ()
          n65 = Close File(refnum=w69, error in=w68) -> (error out=w67:errorcluster)  [unwired: 1 out]
          n66 = local write "data file error"(w67) -> ()
        }
        frame #4 {
          # "get mail settings"
          n67 = local read "Auto Mail Send"() -> (w80:bool)
          n68 = local read "MAIL SETTINGS"() -> (w84:T7)
          n69 = String To Path(string="c:\\crabtree\\Set Up\\") -> (path=w92:path)
          n70 = Build Path(base path=w92, name or relative path="mail.bin") -> (appended path=w90:path)
          n71 = Create Folder(path (use dialog)=w92) -> (error out=w94:errorcluster)  [unwired: 2 in, 2 out]
          n72 = Bundle("MAIL SETTINGS"=w84, "Auto Mail Send"=w80, "") -> (w83:T22)  [unwired: 1 in]
          n73 = call <vilib>:"Clear Errors.vi"("error in (no error)"=w94) -> ()  [unwired: 6 in, 1 out]
          n74 = Open/Create/Replace File(file path (use dialog)=w90) -> (refnum out=w88:refnum<file>, error out=w89:errorcluster)  [unwired: 5 in, 1 out]
          n75 = Read from Binary File(5:w83, 8:w89, 11:w88) -> (0:w86:errorcluster, 2:w82:T22, 3:w87:refnum<file>)  [unwired: 3 in, 1 out]
          n76 = Unbundle(w82) -> ("MAIL SETTINGS"=w81:T7, "Auto Mail Send"=w79:bool, w78:string)
          n77 = local write "TO (string):"(w78) -> ()
          n78 = local write "Auto Mail Send"(w79) -> ()
          n79 = local write "MAIL SETTINGS"(w81) -> ()
          n80 = Close File(refnum=w87, error in=w86) -> (error out=w85:errorcluster)  [unwired: 1 out]
          n81 = local write "data file error"(w85) -> ()
        }
        frame #5 {
          # "set display status if blank"
          n82 = local read "DISP LAB03-2"() -> (w124:T4)
          n83 = local read "DISP LAB03-1"() -> (w131:T4)
          n84 = local read "DISP LAB02-2"() -> (w138:T4)
          n85 = local read "DISP LAB01-2"() -> (w151:T4)
          n86 = local read "DISP LAB01-1"() -> (w160:T4)
          n87 = local read "DISP LAB02-1"() -> (w145:T4)
          n88 = Unbundle(w124) -> ("STATUS"=w126:string)  [unwired: 2 out]
          n89 = Unbundle(w131) -> ("STATUS"=w133:string)  [unwired: 2 out]
          n90 = Unbundle(w138) -> ("STATUS"=w140:string)  [unwired: 2 out]
          n91 = Unbundle(w145) -> ("STATUS"=w147:string)  [unwired: 2 out]
          n92 = Unbundle(w151) -> ("STATUS"=w154:string)  [unwired: 2 out]
          n93 = Unbundle(w160) -> ("STATUS"=w161:string)  [unwired: 2 out]
          n94 = Equal?(x="", y=w126) -> (x = y?=w128:bool)
          n95 = Equal?(x="", y=w133) -> (x = y?=w135:bool)
          n96 = Equal?(x="", y=w140) -> (x = y?=w142:bool)
          n97 = Equal?(x="", y=w147) -> (x = y?=w149:bool)
          n98 = Equal?(x="", y=w154) -> (x = y?=w156:bool)
          n99 = Equal?(x="", y=w161) -> (x = y?=w163:bool)
          n100 = Select(t="STOP", s=w128, f=w126) -> (s? t:f=w125:string)
          n101 = Select(t="STOP", s=w135, f=w133) -> (s? t:f=w132:string)
          n102 = Select(t="STOP", s=w142, f=w140) -> (s? t:f=w139:string)
          n103 = Select(t="STOP", s=w149, f=w147) -> (s? t:f=w146:string)
          n104 = Select(t="STOP", s=w156, f=w154) -> (s? t:f=w153:string)
          n105 = Select(t="STOP", s=w163, f=w161) -> (s? t:f=w159:string)
          n106 = Bundle(cluster=w124, "STATUS"=w125) -> (w123:T4)  [unwired: 2 in]
          n107 = Bundle(cluster=w131, "STATUS"=w132) -> (w130:T4)  [unwired: 2 in]
          n108 = Bundle(cluster=w138, "STATUS"=w139) -> (w137:T4)  [unwired: 2 in]
          n109 = Bundle(cluster=w145, "STATUS"=w146) -> (w144:T4)  [unwired: 2 in]
          n110 = Bundle(cluster=w151, "STATUS"=w153) -> (w152:T4)  [unwired: 2 in]
          n111 = Bundle(cluster=w160, "STATUS"=w159) -> (w158:T4)  [unwired: 2 in]
          n112 = local write "DISP LAB01-2"(w152) -> ()
          n113 = local write "DISP LAB01-1"(w158) -> ()
          n114 = local write "DISP LAB02-1"(w144) -> ()
          n115 = local write "DISP LAB03-1"(w130) -> ()
          n116 = local write "DISP LAB02-2"(w137) -> ()
          n117 = local write "DISP LAB03-2"(w123) -> ()
          n118 = local read "DISP LAB05-2"() -> (w96:T4)
          n119 = local read "DISP LAB05-1"() -> (w103:T4)
          n120 = local read "DISP LAB04-2"() -> (w105:T4)
          n121 = local read "DISP LAB04-1"() -> (w107:T4)
          n122 = Unbundle(w96) -> ("STATUS"=w98:string)  [unwired: 2 out]
          n123 = Unbundle(w103) -> ("STATUS"=w109:string)  [unwired: 2 out]
          n124 = Unbundle(w105) -> ("STATUS"=w114:string)  [unwired: 2 out]
          n125 = Unbundle(w107) -> ("STATUS"=w119:string)  [unwired: 2 out]
          n126 = Equal?(x="", y=w98) -> (x = y?=w100:bool)
          n127 = Equal?(x="", y=w109) -> (x = y?=w111:bool)
          n128 = Equal?(x="", y=w114) -> (x = y?=w116:bool)
          n129 = Equal?(x="", y=w119) -> (x = y?=w121:bool)
          n130 = Select(t="STOP", s=w100, f=w98) -> (s? t:f=w97:string)
          n131 = Select(t="STOP", s=w111, f=w109) -> (s? t:f=w108:string)
          n132 = Select(t="STOP", s=w116, f=w114) -> (s? t:f=w113:string)
          n133 = Select(t="STOP", s=w121, f=w119) -> (s? t:f=w118:string)
          n134 = Bundle(cluster=w96, "STATUS"=w97) -> (w95:T4)  [unwired: 2 in]
          n135 = Bundle(cluster=w103, "STATUS"=w108) -> (w102:T4)  [unwired: 2 in]
          n136 = Bundle(cluster=w105, "STATUS"=w113) -> (w104:T4)  [unwired: 2 in]
          n137 = Bundle(cluster=w107, "STATUS"=w118) -> (w106:T4)  [unwired: 2 in]
          n138 = local write "DISP LAB05-2"(w95) -> ()
          n139 = local write "DISP LAB05-1"(w102) -> ()
          n140 = local write "DISP LAB04-1"(w106) -> ()
          n141 = local write "DISP LAB04-2"(w104) -> ()
        }
        frame #6 {
          # "initialise analog input express vi's"
          n142 = for {
            N: 2.0 -> [_]
            n143 = call "sub vi - analog 1st setup v1.vi"() -> ("error out"=w167:errorcluster)  [unwired: 11 in, 4 out]
            n144 = Unbundle(w167) -> ("status"=w166:bool)  [unwired: 2 out]
            n145 = local write "simulate"(w166) -> ()
          }
        }
        frame #7 {
          # "get initial temperature values"
          n146 = stacked-sequence {
            frame #0 {
              w174 = TRUE
              n147 = call "sub vi - GET ALL TEMP v4.vi"("LA01-EN"=w174, "LA02-EN"=w174, "LA03-EN"=w174, "LA04-EN"=w174, "LA05-EN"=w174, "Gen Cal Value"=1) -> ("LA01 TEMP"=w172:T23, "LA02 TEMP"=w171:T23, "LA03 TEMP"=w170:T23, "LA04 TEMP"=w169:T23, "LA05 TEMP"=w168:T23)  [unwired: 4 in, 1 out]
              n148 = local write "LAB01 TEMP"(w172) -> ()
              n149 = local write "LAB02 TEMP"(w171) -> ()
              n150 = local write "LAB04 TEMP"(w169) -> ()
              n151 = local write "LAB03 TEMP"(w170) -> ()
              n152 = local write "LAB05 TEMP"(w168) -> ()
            }
            frame #1 {
              w175 = 0
              n153 = local read "LAB01 TEMP"() -> (w181:T14)
              n154 = Unbundle By Name(w181) -> ("T1 Live"=w180:dbl, "T1 Neut"=w179:dbl, "T2 Live"=w178:dbl, "T2 Neut"=w177:dbl)  [unwired: 2 out]
              n155 = local read "TEMP LA01"() -> (w182:T11)
              n156 = Bundle By Name(cluster=w182, "TL-1"=w180, "TN-1"=w179, "TL-2"=w178, "TN-2"=w177, "TL -1COUNT"=w175, "TN-1 COUNT"=w175, "TL-2 COUNT"=w175, "TN-2 COUNT"=w175) -> (w176:T11)
              n157 = local write "TEMP LA01"(w176) -> ()
            }
            frame #2 {
              w183 = 0
              n158 = local read "LAB02 TEMP"() -> (w189:T14)
              n159 = Unbundle By Name(w189) -> ("T1 Live"=w188:dbl, "T1 Neut"=w187:dbl, "T2 Live"=w186:dbl, "T2 Neut"=w185:dbl)  [unwired: 2 out]
              n160 = local read "TEMP LA02"() -> (w190:T11)
              n161 = Bundle By Name(cluster=w190, "TL-1"=w188, "TN-1"=w187, "TL-2"=w186, "TN-2"=w185, "TL -1COUNT"=w183, "TN-1 COUNT"=w183, "TL-2 COUNT"=w183, "TN-2 COUNT"=w183) -> (w184:T11)
              n162 = local write "TEMP LA02"(w184) -> ()
            }
            frame #3 {
              w191 = 0
              n163 = local read "LAB03 TEMP"() -> (w197:T14)
              n164 = Unbundle By Name(w197) -> ("T1 Live"=w196:dbl, "T1 Neut"=w195:dbl, "T2 Live"=w194:dbl, "T2 Neut"=w193:dbl)  [unwired: 2 out]
              n165 = local read "TEMP LA03"() -> (w198:T11)
              n166 = Bundle By Name(cluster=w198, "TL-1"=w196, "TN-1"=w195, "TL-2"=w194, "TN-2"=w193, "TL -1COUNT"=w191, "TN-1 COUNT"=w191, "TL-2 COUNT"=w191, "TN-2 COUNT"=w191) -> (w192:T11)
              n167 = local write "TEMP LA03"(w192) -> ()
            }
            frame #4 {
              w199 = 0
              n168 = local read "LAB04 TEMP"() -> (w205:T14)
              n169 = Unbundle By Name(w205) -> ("T1 Live"=w204:dbl, "T1 Neut"=w203:dbl, "T2 Live"=w202:dbl, "T2 Neut"=w201:dbl)  [unwired: 2 out]
              n170 = local read "TEMP LA04"() -> (w206:T11)
              n171 = Bundle By Name(cluster=w206, "TL-1"=w204, "TN-1"=w203, "TL-2"=w202, "TN-2"=w201, "TL -1COUNT"=w199, "TN-1 COUNT"=w199, "TL-2 COUNT"=w199, "TN-2 COUNT"=w199) -> (w200:T11)
              n172 = local write "TEMP LA04"(w200) -> ()
            }
            frame #5 {
              w207 = 0
              n173 = local read "LAB05 TEMP"() -> (w213:T14)
              n174 = Unbundle By Name(w213) -> ("T1 Live"=w212:dbl, "T1 Neut"=w211:dbl, "T2 Live"=w210:dbl, "T2 Neut"=w209:dbl)  [unwired: 2 out]
              n175 = local read "TEMP LA05"() -> (w214:T11)
              n176 = Bundle By Name(cluster=w214, "TL-1"=w212, "TN-1"=w211, "TL-2"=w210, "TN-2"=w209, "TL -1COUNT"=w207, "TN-1 COUNT"=w207, "TL-2 COUNT"=w207, "TN-2 COUNT"=w207) -> (w208:T11)
              n177 = local write "TEMP LA05"(w208) -> ()
            }
          }
        }
        frame #8 {
          # "enable front panel, all settings done"
          n178 = property on="Tab Control 2" class="TabCtl (strict)"("DisabledEnum"=T15."Enabled" ("Disabled")) -> ()  [unwired: 2 in, 2 out]
          n179 = property on="Tab Control 2" class="TabCtl (strict)"("Value"=0) -> ()  [unwired: 2 in, 2 out]
        }
        frame #9 {
          # "check network directory valid"
          n180 = while {
            stop <- w219 continue-if-true
            w217 = TRUE
            n181 = local read "Network Directory"() -> (w221:path)
            n182 = property on="Tab Control 2" class="TabCtl (strict)"("Value"=5) -> ()  [unwired: 2 in, 2 out]
            n183 = File/Directory Info(path=w221) -> (error out=w222:errorcluster)  [unwired: 1 in, 6 out]
            n184 = Unbundle(w222) -> ("status"=w219:bool)  [unwired: 2 out]
            n185 = case shown="True" w219 {
              frame False {
                n186 = local write "Message"("") -> ()
              }
              frame True {
                "Message" <- "NETWORK DIRECTORY NOT FOUND!!!!"
              }
            }
            n187 = property on="Message" class="Str"("Text.TextColor"=u32 16711680) -> ()  [unwired: 2 in, 2 out]
            n188 = property on="Network Directory" class="Path"("Blinking"=w217) -> ()  [unwired: 2 in, 2 out]
            n189 = property on="Message" class="Str"("Blinking"=w217) -> ()  [unwired: 2 in, 2 out]
          }
        }
        frame #10 {
          w225 = FALSE
          n190 = property on="Message" class="Str"("Blinking"=w225) -> ()  [unwired: 2 in, 2 out]
          n191 = property on="Network Directory" class="Path"("Blinking"=w225) -> ()  [unwired: 2 in, 2 out]
          n192 = property on="Tab Control 2" class="TabCtl (strict)"("Value"=0) -> ()  [unwired: 2 in, 2 out]
        }
      }
    }
    frame #2 {
      n193 = node-c288("loop  delay(mS)") -> (w229:T16)  [unwired: 3 in]
      n194 = timed-loop {
        timing: w229 -> [_]
        timing-out: [_] -> w228
        i -> [w251]
        stop <- "stop" stop-if-true
        n195 = node-c288() -> ()  [unwired: 1 in, 1 out]
        n196 = local read "SELECT LAB05-2"() -> (w231:T3)
        n197 = local read "SELECT LAB05-1"() -> (w232:T3)
        n198 = local read "SELECT LAB04-2"() -> (w233:T3)
        n199 = local read "SELECT LAB03-1"() -> (w236:T3)
        n200 = local read "SELECT LAB02-2"() -> (w237:T3)
        n201 = local read "SELECT LAB01-1"() -> (w240:T3)
        n202 = local read "SELECT LAB03-2"() -> (w235:T3)
        n203 = local read "SELECT LAB01-2"() -> (w239:T3)
        n204 = local read "SELECT LAB04-1"() -> (w234:T3)
        n205 = local read "SELECT LAB02-1"() -> (w238:T3)
        n206 = local read "run lab03-2"() -> (w245:bool)
        n207 = local read "run lab04-1"() -> (w244:bool)
        n208 = local read "run lab05-1"() -> (w242:bool)
        n209 = local read "run lab04-2"() -> (w243:bool)
        n210 = local read "run lab05-2"() -> (w241:bool)
        n211 = local read "run lab03-1"() -> (w246:bool)
        n212 = local read "run lab02-2"() -> (w247:bool)
        n213 = local read "run lab02-1"() -> (w248:bool)
        n214 = local read "run lab01-1"() -> (w250:bool)
        n215 = local read "run lab01-2"() -> (w249:bool)
        n216 = stacked-sequence {
          seq-local: [_ w313 _ _ _ _ _ _ _ _ _ _ _ _ _ _ _ _ _ _] -> [_ _ _ _ _ w1920 _ _ _ _ _ _ _ _ _ _ _ _ _ _]
          seq-local: [_ w312 _ _ _ _ _ _ _ _ _ _ _ _ _ _ _ _ _ _] -> [_ _ _ _ _ w1919 _ _ _ _ _ _ _ _ _ _ _ _ _ _]
          seq-local: [_ w299 _ _ _ _ _ _ _ _ _ _ _ _ _ _ _ _ _ _] -> [_ _ _ _ _ w1918 _ _ _ _ _ _ _ _ _ _ _ _ _ _]
          seq-local: [_ w298 _ _ _ _ _ _ _ _ _ _ _ _ _ _ _ _ _ _] -> [_ _ _ _ _ w1917 _ _ _ _ _ _ _ _ _ _ _ _ _ _]
          seq-local: [_ w297 _ _ _ _ _ _ _ _ _ _ _ _ _ _ _ _ _ _] -> [_ _ _ _ _ w1916 _ _ _ _ _ _ _ _ _ _ _ _ _ _]
          seq-local: [_ w296 _ _ _ _ _ _ _ _ _ _ _ _ _ _ _ _ _ _] -> [_ _ _ _ _ w1915 _ _ _ _ _ _ _ _ _ _ _ _ _ _]
          seq-local: [_ w295 _ _ _ _ _ _ _ _ _ _ _ _ _ _ _ _ _ _] -> [_ _ _ _ _ w1914 _ _ _ _ _ _ _ _ _ _ _ _ _ _]
          seq-local: [_ w294 _ _ _ _ _ _ _ _ _ _ _ _ _ _ _ _ _ _] -> [_ _ _ _ _ w1913 _ _ _ _ _ _ _ _ _ _ _ _ _ _]
          seq-local: [_ w293 _ _ _ _ _ _ _ _ _ _ _ _ _ _ _ _ _ _] -> [_ _ _ _ _ w1912 _ _ _ _ _ _ _ _ _ _ _ _ _ _]
          seq-local: [_ w292 _ _ _ _ _ _ _ _ _ _ _ _ _ _ _ _ _ _] -> [_ _ _ _ _ w1911 _ _ _ _ _ _ _ _ _ _ _ _ _ _]
          tunnel: w250 -> [_ _ w329 w566 w1510 w1940 w2250 w2495 _ _ _ _ _ w3054 _ w3982 _ _ w4263 w4566]
          tunnel: w249 -> [_ _ w328 w564 w1509 w1939 w2251 w2494 _ _ _ _ _ w3053 _ w3980 _ _ w4262 w4565]
          tunnel: w248 -> [_ _ w327 w562 w1508 w1938 w2249 w2493 _ _ _ _ _ w3052 _ w3978 _ _ w4261 w4564]
          tunnel: w247 -> [_ _ w326 w560 w1507 w1937 w2248 w2492 _ _ _ _ _ w3051 _ w3976 _ _ w4260 w4563]
          tunnel: w246 -> [_ _ w325 w558 w1506 w1936 w2247 w2491 _ _ _ _ _ w3050 _ w3974 _ _ w4259 w4562]
          tunnel: w245 -> [_ _ w324 w556 w1505 w1935 w2246 w2490 _ _ _ _ _ w3049 _ w3972 _ _ w4258 w4561]
          tunnel: w244 -> [_ _ w323 w554 w1504 w1934 w2245 w2489 _ _ _ _ _ w3048 _ w3970 _ _ w4257 w4560]
          tunnel: w243 -> [_ _ w322 w552 w1503 w1933 w2244 w2488 _ _ _ _ _ w3047 _ w3968 _ _ w4256 w4559]
          tunnel: w242 -> [_ _ w321 w550 w1502 w1932 w2243 w2487 _ _ _ _ _ w3046 _ w3966 _ _ w4255 w4558]
          tunnel: w241 -> [_ _ w320 w548 w1501 w1931 w2242 w2486 _ _ _ _ _ w3045 _ w3964 _ _ w4254 w4557]
          tunnel: w240 -> [_ _ _ w565 w1500 w1930 _ _ _ _ _ _ _ _ _ w3984 _ _ _ _]
          tunnel: w239 -> [_ _ _ w563 w1499 w1929 _ _ _ _ _ _ _ _ _ w3979 _ _ _ _]
          tunnel: w238 -> [_ _ _ w561 w1498 w1928 _ _ _ _ _ _ _ _ _ w3977 _ _ _ _]
          tunnel: w237 -> [_ _ _ w559 w1497 w1927 _ _ _ _ _ _ _ _ _ w3975 _ _ _ _]
          tunnel: w236 -> [_ _ _ w557 w1496 w1926 _ _ _ _ _ _ _ _ _ w3973 _ _ _ _]
          tunnel: w235 -> [_ _ _ w555 w1495 w1925 _ _ _ _ _ _ _ _ _ w3971 _ _ _ _]
          tunnel: w234 -> [_ _ _ w553 w1494 w1924 _ _ _ _ _ _ _ _ _ w3969 _ _ _ _]
          tunnel: w233 -> [_ _ _ w551 w1493 w1923 _ _ _ _ _ _ _ _ _ w3967 _ _ _ _]
          tunnel: w232 -> [_ _ _ w549 w1492 w1922 _ _ _ _ _ _ _ _ _ w3965 _ _ _ _]
          tunnel: w231 -> [_ _ _ w547 w1491 w1921 _ _ _ _ _ _ _ _ _ w3963 _ _ _ _]
          frame #0 {
            w255 = FALSE
            w260 = 0.5
            # "set up cycle control"
            n217 = local read "jig cycle"() -> (w259:dbl)
            n218 = Divide(x="JIG ON TIME (S)", y=w260) -> (x/y=→"on loops":dbl)
            n219 = Divide(x="JIG OFF TIME (S)", y=w260) -> (x/y=→"off loops":dbl)
            n220 = Increment(x=w259) -> (x+1=w258:dbl)
            n221 = local write "TEMP update"(w255) -> ()
            n222 = local write "AI update"(w255) -> ()
            n223 = local write "jig cycle"(w258) -> ()
            n224 = event shown="[1] \"ADMIN PAGE\": Value Change" {
              selector: _ -> [_ _]
              dyn-events: _ -> [_ _]
              timeout: 10 -> [_ _]
              event Timeout {
                n225 = event-data() -> ()  [unwired: 1 in, 3 out]
              }
              event "ADMIN PAGE": Value Change {
                n226 = event-data() -> ()  [unwired: 1 in, 6 out]
                n227 = stacked-sequence {
                  seq-local: [_ w264 _] -> [_ _ w265]
                  frame #0 {
                    n228 = global write "Global 1.vi" "password"("9999") -> ()
                  }
                  frame #1 {
                    n229 = call "sub vi - password 1.vi"() -> ("RESULT"=w264:bool)  [unwired: 11 in]
                  }
                  frame #2 {
                    w267 = FALSE
                    n230 = property on="Tab Control 2" class="TabCtl (strict)"() -> ("Pages"=w271:refnum<vi>[])  [unwired: 2 in, 2 out]
                    n231 = Select(t=TRUE, s=w265, f=w267) -> (s? t:f=w266:bool)
                    n232 = Index Array(array=w271, index=9) -> (element=w269:refnum<vi>)
                    n233 = property class="Page"(reference=w269, "PageVis"=w266) -> ()  [unwired: 1 in, 2 out]
                    n234 = local write "ADMIN PAGE"(w267) -> ()
                  }
                }
              }
            }
          }
          frame #1 {
            w309 = 60.0
            # "convert temperature rise minutes to cycles"
            n235 = local read "SET LAB05-2"() -> (w273:T5)
            n236 = local read "SET LAB05-1"() -> (w275:T5)
            n237 = local read "SET LAB04-2"() -> (w277:T5)
            n238 = local read "SET LAB01-1"() -> (w291:T5)
            n239 = local read "SET LAB01-2"() -> (w289:T5)
            n240 = local read "SET LAB02-2"() -> (w285:T5)
            n241 = local read "SET LAB04-1"() -> (w279:T5)
            n242 = local read "SET LAB03-1"() -> (w283:T5)
            n243 = local read "SET LAB03-2"() -> (w281:T5)
            n244 = local read "SET LAB02-1"() -> (w287:T5)
            n245 = local read "JIG OFF TIME (S)"() -> (w314:dbl)
            n246 = local read "JIG ON TIME (S)"() -> (w315:dbl)
            n247 = Unbundle(w273) -> ("T-RISE mins"=w272:dbl)  [unwired: 4 out]
            n248 = Unbundle(w275) -> ("T-RISE mins"=w274:dbl)  [unwired: 4 out]
            n249 = Unbundle(w291) -> ("T-RISE mins"=w290:dbl)  [unwired: 4 out]
            n250 = Unbundle(w277) -> ("T-RISE mins"=w276:dbl)  [unwired: 4 out]
            n251 = Unbundle(w289) -> ("T-RISE mins"=w288:dbl)  [unwired: 4 out]
            n252 = Unbundle(w287) -> ("T-RISE mins"=w286:dbl)  [unwired: 4 out]
            n253 = Unbundle(w279) -> ("T-RISE mins"=w278:dbl)  [unwired: 4 out]
            n254 = Unbundle(w285) -> ("T-RISE mins"=w284:dbl)  [unwired: 4 out]
            n255 = Unbundle(w281) -> ("T-RISE mins"=w280:dbl)  [unwired: 4 out]
            n256 = Unbundle(w283) -> ("T-RISE mins"=w282:dbl)  [unwired: 4 out]
            n257 = Add(x=w315, y=w314) -> (x+y=w308:dbl)
            n258 = Multiply(x=w309, y=w280) -> (x*y=w304:dbl)
            n259 = Multiply(x=w309, y=w278) -> (x*y=w303:dbl)
            n260 = Multiply(x=w309, y=w276) -> (x*y=w302:dbl)
            n261 = Multiply(x=w309, y=w274) -> (x*y=w301:dbl)
            n262 = Multiply(x=w309, y=w272) -> (x*y=w300:dbl)
            n263 = Multiply(x=w309, y=w288) -> (x*y=w310:dbl)
            n264 = Multiply(x=w309, y=w282) -> (x*y=w305:dbl)
            n265 = Multiply(x=w309, y=w290) -> (x*y=w311:dbl)
            n266 = Multiply(x=w309, y=w286) -> (x*y=w307:dbl)
            n267 = Multiply(x=w309, y=w284) -> (x*y=w306:dbl)
            n268 = Divide(x=w301, y=w308) -> (x/y=w293:dbl)
            n269 = Divide(x=w302, y=w308) -> (x/y=w294:dbl)
            n270 = Divide(x=w303, y=w308) -> (x/y=w295:dbl)
            n271 = Divide(x=w300, y=w308) -> (x/y=w292:dbl)
            n272 = Divide(x=w305, y=w308) -> (x/y=w297:dbl)
            n273 = Divide(x=w311, y=w308) -> (x/y=w313:dbl)
            n274 = Divide(x=w310, y=w308) -> (x/y=w312:dbl)
            n275 = Divide(x=w307, y=w308) -> (x/y=w299:dbl)
            n276 = Divide(x=w306, y=w308) -> (x/y=w298:dbl)
            n277 = Divide(x=w304, y=w308) -> (x/y=w296:dbl)
          }
          frame #2 {
            # "control cycle loops"
            n278 = local read "JIG OFF TIME (S)"() -> (w318:dbl)
            n279 = local read "JIG ON TIME (S)"() -> (w317:dbl)
            n280 = local read "jig cycle"() -> (w331:dbl)
            n281 = local read "on loops"() -> (w333:dbl)
            n282 = local read "off loops"() -> (w332:dbl)
            n283 = Add(x=w318, y=w317) -> (x+y=w316:dbl)
            n284 = Add(x=w333, y=w332) -> (x+y=w319:dbl)
            n285 = Greater Or Equal?(x=w331, y=w319) -> (x >= y?=w330:bool)
            n286 = case shown="True" w330 {
              tunnel: w329 -> [_ w366]
              tunnel: w328 -> [_ w365]
              tunnel: w327 -> [_ w364]
              tunnel: w326 -> [_ w363]
              tunnel: w325 -> [_ w362]
              tunnel: w324 -> [_ w361]
              tunnel: w323 -> [_ w360]
              tunnel: w322 -> [_ w359]
              tunnel: w321 -> [_ w358]
              tunnel: w320 -> [_ w357]
              tunnel: w316 -> [_ w356]
              frame False {
              }
              frame True {
                # "increment cycle value and convert cycles to minutes for temp rise"
                n287 = local read "JIG RELAY CYCLES"() -> (w355:T10)
                n288 = Unbundle By Name(w355) -> ("LAB01-1"=w353:dbl, "LAB01-2"=w351:dbl, "LAB02-1"=w349:dbl, "LAB02-2"=w347:dbl, "LAB03-1"=w345:dbl, "LAB03-2"=w343:dbl, "LAB04-1"=w341:dbl, "LAB04-2"=w339:dbl, "LAB05-1"=w337:dbl, "LAB05-2"=w335:dbl)
                n289 = stacked-sequence {
                  tunnel: w366 -> [w378 _ _ _ _ _ _ _ _ _]
                  tunnel: w365 -> [_ w395 _ _ _ _ _ _ _ _]
                  tunnel: w364 -> [_ _ w412 _ _ _ _ _ _ _]
                  tunnel: w363 -> [_ _ _ w429 _ _ _ _ _ _]
                  tunnel: w362 -> [_ _ _ _ w446 _ _ _ _ _]
                  tunnel: w361 -> [_ _ _ _ _ w463 _ _ _ _]
                  tunnel: w360 -> [_ _ _ _ _ _ w480 _ _ _]
                  tunnel: w359 -> [_ _ _ _ _ _ _ w497 _ _]
                  tunnel: w358 -> [_ _ _ _ _ _ _ _ w514 _]
                  tunnel: w357 -> [_ _ _ _ _ _ _ _ _ w531]
                  tunnel: w356 -> [w375 w392 w409 w426 w443 w460 w477 w494 w511 w528]
                  tunnel: w353 -> [w369 _ _ _ _ _ _ _ _ _]
                  tunnel: [w368 _ _ _ _ _ _ _ _ _] -> w352
                  tunnel: w351 -> [_ w386 _ _ _ _ _ _ _ _]
                  tunnel: [_ w385 _ _ _ _ _ _ _ _] -> w350
                  tunnel: w349 -> [_ _ w403 _ _ _ _ _ _ _]
                  tunnel: [_ _ w402 _ _ _ _ _ _ _] -> w348
                  tunnel: w347 -> [_ _ _ w420 _ _ _ _ _ _]
                  tunnel: [_ _ _ w419 _ _ _ _ _ _] -> w346
                  tunnel: w345 -> [_ _ _ _ w437 _ _ _ _ _]
                  tunnel: [_ _ _ _ w436 _ _ _ _ _] -> w344
                  tunnel: w343 -> [_ _ _ _ _ w454 _ _ _ _]
                  tunnel: [_ _ _ _ _ w453 _ _ _ _] -> w342
                  tunnel: w341 -> [_ _ _ _ _ _ w471 _ _ _]
                  tunnel: [_ _ _ _ _ _ w470 _ _ _] -> w340
                  tunnel: w339 -> [_ _ _ _ _ _ _ w488 _ _]
                  tunnel: [_ _ _ _ _ _ _ w487 _ _] -> w338
                  tunnel: w337 -> [_ _ _ _ _ _ _ _ w505 _]
                  tunnel: [_ _ _ _ _ _ _ _ w504 _] -> w336
                  tunnel: w335 -> [_ _ _ _ _ _ _ _ _ w522]
                  tunnel: [_ _ _ _ _ _ _ _ _ w521] -> w334
                  frame #0 {
                    n290 = local read "DISP LAB01-1"() -> (w373:T4)
                    n291 = Unbundle(w373) -> ("CYCLE"=w374:dbl)  [unwired: 2 out]
                    n292 = case shown="True" w378 {
                      tunnel: w374 -> [w380 w384]
                      tunnel: [w380 w383] -> w372
                      tunnel: w369 -> [w379 w382]
                      tunnel: [w379 w381] -> w368
                      frame False {
                      }
                      frame True {
                        n293 = Increment(x=w382) -> (x+1=w381:dbl)
                        n294 = Increment(x=w384) -> (x+1=w383:dbl)
                      }
                    }
                    n295 = Multiply(x=w372, y=w375) -> (x*y=w376:dbl)
                    n296 = Divide(x=w376, y=60.0) -> (x/y=w371:dbl)
                    n297 = Bundle(cluster=w373, "CYCLE"=w372, "MINS"=w371) -> (w370:T4)  [unwired: 1 in]
                    n298 = local write "DISP LAB01-1"(w370) -> ()
                  }
                  frame #1 {
                    n299 = local read "DISP LAB01-2"() -> (w390:T4)
                    n300 = Unbundle(w390) -> ("CYCLE"=w391:dbl)  [unwired: 2 out]
                    n301 = case shown="True" w395 {
                      tunnel: w391 -> [w397 w401]
                      tunnel: [w397 w400] -> w388
                      tunnel: w386 -> [w396 w399]
                      tunnel: [w396 w398] -> w385
                      frame False {
                      }
                      frame True {
                        n302 = Increment(x=w399) -> (x+1=w398:dbl)
                        n303 = Increment(x=w401) -> (x+1=w400:dbl)
                      }
                    }
                    n304 = Multiply(x=w388, y=w392) -> (x*y=w393:dbl)
                    n305 = Divide(x=w393, y=60.0) -> (x/y=w387:dbl)
                    n306 = Bundle(cluster=w390, "CYCLE"=w388, "MINS"=w387) -> (w389:T4)  [unwired: 1 in]
                    n307 = local write "DISP LAB01-2"(w389) -> ()
                  }
                  frame #2 {
                    n308 = local read "DISP LAB02-1"() -> (w407:T4)
                    n309 = Unbundle(w407) -> ("CYCLE"=w408:dbl)  [unwired: 2 out]
                    n310 = case shown="True" w412 {
                      tunnel: [w414 w418] -> w405
                      tunnel: w408 -> [w414 w417]
                      tunnel: w403 -> [w413 w416]
                      tunnel: [w413 w415] -> w402
                      frame False {
                      }
                      frame True {
                        n311 = Increment(x=w416) -> (x+1=w415:dbl)
                        n312 = Increment(x=w417) -> (x+1=w418:dbl)
                      }
                    }
                    n313 = Multiply(x=w405, y=w409) -> (x*y=w410:dbl)
                    n314 = Divide(x=w410, y=60.0) -> (x/y=w404:dbl)
                    n315 = Bundle(cluster=w407, "CYCLE"=w405, "MINS"=w404) -> (w406:T4)  [unwired: 1 in]
                    n316 = local write "DISP LAB02-1"(w406) -> ()
                  }
                  frame #3 {
                    n317 = local read "DISP LAB02-2"() -> (w424:T4)
                    n318 = Unbundle(w424) -> ("CYCLE"=w425:dbl)  [unwired: 2 out]
                    n319 = case shown="True" w429 {
                      tunnel: [w431 w435] -> w423
                      tunnel: w425 -> [w431 w434]
                      tunnel: w420 -> [w430 w433]
                      tunnel: [w430 w432] -> w419
                      frame False {
                      }
                      frame True {
                        n320 = Increment(x=w433) -> (x+1=w432:dbl)
                        n321 = Increment(x=w434) -> (x+1=w435:dbl)
                      }
                    }
                    n322 = Multiply(x=w423, y=w426) -> (x*y=w427:dbl)
                    n323 = Divide(x=w427, y=60.0) -> (x/y=w422:dbl)
                    n324 = Bundle(cluster=w424, "CYCLE"=w423, "MINS"=w422) -> (w421:T4)  [unwired: 1 in]
                    n325 = local write "DISP LAB02-2"(w421) -> ()
                  }
                  frame #4 {
                    n326 = local read "DISP LAB03-1"() -> (w441:T4)
                    n327 = Unbundle(w441) -> ("CYCLE"=w442:dbl)  [unwired: 2 out]
                    n328 = case shown="True" w446 {
                      tunnel: [w448 w452] -> w438
                      tunnel: w442 -> [w448 w451]
                      tunnel: w437 -> [w447 w450]
                      tunnel: [w447 w449] -> w436
                      frame False {
                      }
                      frame True {
                        n329 = Increment(x=w450) -> (x+1=w449:dbl)
                        n330 = Increment(x=w451) -> (x+1=w452:dbl)
                      }
                    }
                    n331 = Multiply(x=w438, y=w443) -> (x*y=w444:dbl)
                    n332 = Divide(x=w444, y=60.0) -> (x/y=w439:dbl)
                    n333 = Bundle(cluster=w441, "CYCLE"=w438, "MINS"=w439) -> (w440:T4)  [unwired: 1 in]
                    n334 = local write "DISP LAB03-1"(w440) -> ()
                  }
                  frame #5 {
                    n335 = local read "DISP LAB03-2"() -> (w458:T4)
                    n336 = Unbundle(w458) -> ("CYCLE"=w459:dbl)  [unwired: 2 out]
                    n337 = case shown="True" w463 {
                      tunnel: [w465 w469] -> w457
                      tunnel: w459 -> [w465 w468]
                      tunnel: w454 -> [w464 w467]
                      tunnel: [w464 w466] -> w453
                      frame False {
                      }
                      frame True {
                        n338 = Increment(x=w467) -> (x+1=w466:dbl)
                        n339 = Increment(x=w468) -> (x+1=w469:dbl)
                      }
                    }
                    n340 = Multiply(x=w457, y=w460) -> (x*y=w461:dbl)
                    n341 = Divide(x=w461, y=60.0) -> (x/y=w456:dbl)
                    n342 = Bundle(cluster=w458, "CYCLE"=w457, "MINS"=w456) -> (w455:T4)  [unwired: 1 in]
                    n343 = local write "DISP LAB03-2"(w455) -> ()
                  }
                  frame #6 {
                    n344 = local read "DISP LAB04-1"() -> (w475:T4)
                    n345 = Unbundle(w475) -> ("CYCLE"=w476:dbl)  [unwired: 2 out]
                    n346 = case shown="True" w480 {
                      tunnel: [w482 w486] -> w473
                      tunnel: w476 -> [w482 w485]
                      tunnel: w471 -> [w481 w484]
                      tunnel: [w481 w483] -> w470
                      frame False {
                      }
                      frame True {
                        n347 = Increment(x=w484) -> (x+1=w483:dbl)
                        n348 = Increment(x=w485) -> (x+1=w486:dbl)
                      }
                    }
                    n349 = Multiply(x=w473, y=w477) -> (x*y=w478:dbl)
                    n350 = Divide(x=w478, y=60.0) -> (x/y=w472:dbl)
                    n351 = Bundle(cluster=w475, "CYCLE"=w473, "MINS"=w472) -> (w474:T4)  [unwired: 1 in]
                    n352 = local write "DISP LAB04-1"(w474) -> ()
                  }
                  frame #7 {
                    n353 = local read "DISP LAB04-2"() -> (w492:T4)
                    n354 = Unbundle(w492) -> ("CYCLE"=w493:dbl)  [unwired: 2 out]
                    n355 = case shown="True" w497 {
                      tunnel: [w499 w503] -> w490
                      tunnel: w493 -> [w499 w502]
                      tunnel: w488 -> [w498 w501]
                      tunnel: [w498 w500] -> w487
                      frame False {
                      }
                      frame True {
                        n356 = Increment(x=w501) -> (x+1=w500:dbl)
                        n357 = Increment(x=w502) -> (x+1=w503:dbl)
                      }
                    }
                    n358 = Multiply(x=w490, y=w494) -> (x*y=w496:dbl)
                    n359 = Divide(x=w496, y=60.0) -> (x/y=w489:dbl)
                    n360 = Bundle(cluster=w492, "CYCLE"=w490, "MINS"=w489) -> (w491:T4)  [unwired: 1 in]
                    n361 = local write "DISP LAB04-2"(w491) -> ()
                  }
                  frame #8 {
                    n362 = local read "DISP LAB05-1"() -> (w509:T4)
                    n363 = Unbundle(w509) -> ("CYCLE"=w510:dbl)  [unwired: 2 out]
                    n364 = case shown="True" w514 {
                      tunnel: [w516 w520] -> w507
                      tunnel: w510 -> [w516 w519]
                      tunnel: w505 -> [w515 w518]
                      tunnel: [w515 w517] -> w504
                      frame False {
                      }
                      frame True {
                        n365 = Increment(x=w518) -> (x+1=w517:dbl)
                        n366 = Increment(x=w519) -> (x+1=w520:dbl)
                      }
                    }
                    n367 = Multiply(x=w507, y=w511) -> (x*y=w512:dbl)
                    n368 = Divide(x=w512, y=60.0) -> (x/y=w506:dbl)
                    n369 = Bundle(cluster=w509, "CYCLE"=w507, "MINS"=w506) -> (w508:T4)  [unwired: 1 in]
                    n370 = local write "DISP LAB05-1"(w508) -> ()
                  }
                  frame #9 {
                    n371 = local read "DISP LAB05-2"() -> (w527:T4)
                    n372 = Unbundle(w527) -> ("CYCLE"=w526:dbl)  [unwired: 2 out]
                    n373 = case shown="False" w531 {
                      tunnel: [w533 w537] -> w525
                      tunnel: w526 -> [w533 w536]
                      tunnel: w522 -> [w532 w535]
                      tunnel: [w532 w534] -> w521
                      frame False {
                      }
                      frame True {
                        n374 = Increment(x=w535) -> (x+1=w534:dbl)
                        n375 = Increment(x=w536) -> (x+1=w537:dbl)
                      }
                    }
                    n376 = Multiply(x=w525, y=w528) -> (x*y=w529:dbl)
                    n377 = Divide(x=w529, y=60.0) -> (x/y=w524:dbl)
                    n378 = Bundle(cluster=w527, "CYCLE"=w525, "MINS"=w524) -> (w523:T4)  [unwired: 1 in]
                    n379 = local write "DISP LAB05-2"(w523) -> ()
                  }
                }
                n380 = local write "jig cycle"(0) -> ()
                n381 = Bundle By Name(cluster=w355, "LAB01-1"=w352, "LAB01-2"=w350, "LAB02-1"=w348, "LAB02-2"=w346, "LAB03-1"=w344, "LAB03-2"=w342, "LAB04-1"=w340, "LAB04-2"=w338, "LAB05-1"=w336, "LAB05-2"=w334) -> (w354:T10)
                n382 = local write "JIG RELAY CYCLES"(w354) -> ()
              }
            }
          }
          frame #3 {
            # "START & STOP test RUN switch change, start test if true and stop test if false"
            n383 = Get Date/Time In Seconds() -> (seconds since 1Jan1904=w545:timestamp)
            n384 = local read "C drive data root dir"() -> (w538:path)
            n385 = Format Date/Time String(time format string (%c)="%b\\%a%d", seconds (now)=w545) -> (date/time string=w569:string)  [unwired: 1 in]
            n386 = Format Date/Time String(time format string (%c)="%H%M", seconds (now)=w545) -> (date/time string=w567:string)  [unwired: 1 in]
            n387 = Format Date/Time String(time format string (%c)="LabPanel%Y", seconds (now)=w545) -> (date/time string=w544:string)  [unwired: 1 in]
            n388 = Path To String(path=w538) -> (string=w541:string)
            n389 = global write "Global 1.vi" "C drive root path"(w538) -> ()
            n390 = Concatenate Strings(w541, "\\") -> (w539:string)
            n391 = event shown="[5] \"RUN LAB03-1\": Value Change" {
              selector: _ -> [_ _ _ _ _ _ _ _ _ _ _]
              dyn-events: _ -> [_ _ _ _ _ _ _ _ _ _ _]
              timeout: 10 -> [_ _ _ _ _ _ _ _ _ _ _]
              tunnel: w539 -> [_ w577 w669 w761 w853 w945 w1037 w1129 w1221 w1313 w1405]
              tunnel: w569 -> [_ w576 w668 w760 w852 w944 w1036 w1128 w1220 w1312 w1404]
              tunnel: w567 -> [_ w574 w667 w759 w851 w943 w1035 w1127 w1219 w1311 w1403]
              tunnel: w565 -> [_ w575 _ _ _ _ _ _ _ _ _]
              tunnel: w566 -> [_ _ _ _ _ _ _ _ _ _ _]
              tunnel: w564 -> [_ _ _ _ _ _ _ _ _ _ _]
              tunnel: w563 -> [_ _ w666 _ _ _ _ _ _ _ _]
              tunnel: w562 -> [_ _ _ _ _ _ _ _ _ _ _]
              tunnel: w561 -> [_ _ _ w758 _ _ _ _ _ _ _]
              tunnel: w560 -> [_ _ _ _ _ _ _ _ _ _ _]
              tunnel: w559 -> [_ _ _ _ w850 _ _ _ _ _ _]
              tunnel: w558 -> [_ _ _ _ _ _ _ _ _ _ _]
              tunnel: w557 -> [_ _ _ _ _ w942 _ _ _ _ _]
              tunnel: w556 -> [_ _ _ _ _ _ _ _ _ _ _]
              tunnel: w555 -> [_ _ _ _ _ _ w1034 _ _ _ _]
              tunnel: w554 -> [_ _ _ _ _ _ _ _ _ _ _]
              tunnel: w553 -> [_ _ _ _ _ _ _ w1126 _ _ _]
              tunnel: w552 -> [_ _ _ _ _ _ _ _ _ _ _]
              tunnel: w551 -> [_ _ _ _ _ _ _ _ w1218 _ _]
              tunnel: w550 -> [_ _ _ _ _ _ _ _ _ _ _]
              tunnel: w549 -> [_ _ _ _ _ _ _ _ _ w1310 _]
              tunnel: w548 -> [_ _ _ _ _ _ _ _ _ _ _]
              tunnel: w547 -> [_ _ _ _ _ _ _ _ _ _ w1402]
              tunnel: w544 -> [_ w573 w665 w757 w849 w941 w1033 w1125 w1217 w1309 w1401]
              tunnel: [_ w572 w664 w756 w848 w940 w1032 w1124 w1216 w1308 w1400] -> w542
              event Timeout {
                n392 = event-data() -> ()  [unwired: 1 in, 3 out]
              }
              event "RUN LAB01-1": Value Change {
                n393 = event-data() -> ("NewVal"=w571:bool)  [unwired: 1 in, 5 out]
                n394 = local write "run lab01-1"(w571) -> ()
                n395 = case shown="True" w571 {
                  tunnel: w577 -> [_ w610]
                  tunnel: w576 -> [_ w609]
                  tunnel: w575 -> [w579 w608]
                  tunnel: w574 -> [_ w607]
                  tunnel: w573 -> [_ w606]
                  tunnel: [w578 w605] -> w572
                  frame False {
                    # "stop test"
                    n396 = stacked-sequence {
                      tunnel: w579 -> [_ w591 _ _]
                      tunnel: [_ w583 _ _] -> w578
                      frame #0 {
                        n397 = local read "DISP LAB01-1"() -> (w582:T4)
                        n398 = Bundle(cluster=w582, "STATUS"="STOP") -> (w580:T4)  [unwired: 2 in]
                        n399 = local write "DISP LAB01-1"(w580) -> ()
                      }
                      frame #1 {
                        n400 = local read "DISP LAB01-1"() -> (w590:T4)
                        n401 = Unbundle(w590) -> ("CYCLE"=w588:dbl, "MINS"=w589:dbl)  [unwired: 1 out]
                        n402 = case shown="\"CYCLE TEST\"" w591 {
                          tunnel: w589 -> [_ _ w598]
                          tunnel: w588 -> [w596 w597 _]
                          tunnel: [w596 w597 w598] -> w587
                          frame "CHART TEST", Default {
                          }
                          frame "CYCLE TEST" {
                          }
                          frame "T-RISE TEST" {
                          }
                        }
                        n403 = local read "TDMS LAB01-1"() -> (w595:refnum<k34>)
                        n404 = Build Array("STOPPED") -> (w592:string[])
                        n405 = Build Array(w587) -> (w586:dbl[])
                        n406 = TDMS Write(0:w595, 5:"TEST RESULT", 7:w592, 9:w586) -> (4:w584:refnum<k34>, 15:w585:errorcluster)  [unwired: 2 in, 2 out]
                        n407 = TDMS Close(8:w585, 11:w584) -> (0:w583:errorcluster)  [unwired: 1 out]
                      }
                      frame #2 {
                        n408 = stacked-sequence {
                          tunnel: "LAB01-1" -> [w601 w603]
                          frame #0 {
                            n409 = call "sub vi - defrag tdms v1.vi"("panel id"=w601) -> ("error out"=w600:errorcluster)  [unwired: 10 in]
                            n410 = local write "data file error"(w600) -> ()
                          }
                          frame #1 {
                            n411 = call "Save data file to network drive v1.vi"("panel id"=w603) -> ("network file save error"=w602:errorcluster)  [unwired: 9 in, 1 out]
                            n412 = local write "RESULT LAB01-1"(FALSE) -> ()
                            n413 = local write "data file error"(w602) -> ()
                          }
                        }
                      }
                      frame #3 {
                      }
                    }
                  }
                  frame True {
                    # "start new test and create test file"
                    n414 = stacked-sequence {
                      seq-local: [w611 _ _ _ _] -> [_ w632 _ _ _]
                      tunnel: w610 -> [w616 _ _ _ _]
                      tunnel: w609 -> [w612 _ _ _ _]
                      tunnel: w608 -> [w626 _ _ _ _]
                      tunnel: w607 -> [w619 _ _ _ _]
                      tunnel: w606 -> [w614 _ _ _ _]
                      tunnel: [_ w633 _ _ _] -> w605
                      frame #0 {
                        w613 = "\\"
                        n415 = case shown="\"CHART TEST\", Default" w626 {
                          tunnel: ["L01-1-CHART TEST-" "L01-1-CYCLE TEST-" "L01-1-T-RISE TEST-"] -> w622
                          frame "CHART TEST", Default {
                          }
                          frame "CYCLE TEST" {
                          }
                          frame "T-RISE TEST" {
                          }
                        }
                        n416 = local read "SET LAB01-1"() -> (w621:T5)
                        n417 = Unbundle(w621) -> ("DESCRIPTION"=w620:string)  [unwired: 4 out]
                        n418 = Concatenate Strings(w616, "\\", w614, w613, w612, w613) -> (w623:string)
                        n419 = String To Path(string=w623) -> (path=w625:path)
                        n420 = Concatenate Strings(w623, w622, w620, "-", w619, ".tdms") -> (w611:string)
                        n421 = Create Folder(path (use dialog)=w625) -> (error out=w624:errorcluster)  [unwired: 2 in, 2 out]
                        n422 = call <vilib>:"Clear Errors.vi"("error in (no error)"=w624) -> ()  [unwired: 6 in, 1 out]
                        n423 = global write "Global 1.vi" "LAB01-1 FILE"(w611) -> ()
                      }
                      frame #1 {
                        n424 = String To Path(string=w632) -> (path=w630:path)
                        n425 = TDMS Open(5:FALSE, 6:FALSE, 10:T19."create or replace" ("operation (0:open)"), 11:w630) -> (0:w633:errorcluster, 3:→"TDMS LAB01-1":refnum<k34>)  [unwired: 3 in]
                      }
                      frame #2 {
                        n426 = local read "TDMS LAB01-1"() -> (w653:refnum<k34>)
                        n427 = local read "SET LAB01-1"() -> (w642:T5)
                        n428 = Build Array("Testers Name", "Description", "Set Test Cycles", "T-Rise minutes", "T-Rise Deg C") -> (w643:string[])
                        n429 = Unbundle(w642) -> ("NAME"=w641:string, "DESCRIPTION"=w640:string, "CYCLES"=w639:dbl, "T-RISE mins"=w638:dbl, "T-RISE deg C"=w637:dbl)
                        n430 = Number To Decimal String(number=w639) -> (decimal integer string=w652:string)  [unwired: 1 in]
                        n431 = Number To Decimal String(number=w638) -> (decimal integer string=w651:string)  [unwired: 1 in]
                        n432 = Number To Decimal String(number=w637) -> (decimal integer string=w650:string)  [unwired: 1 in]
                        n433 = Build Array(w641, w640, w652, w651, w650) -> (w649:string[])
                        n434 = TDMS Set Properties(5:w649, 7:w643, 11:w653) -> ()  [unwired: 3 in, 4 out]
                      }
                      frame #3 {
                        w654 = 0.0
                        n435 = local read "DISP LAB01-1"() -> (w657:T4)
                        n436 = Bundle(cluster=w657, "CYCLE"=w654, "MINS"=w654, "STATUS"="RUN") -> (w656:T4)
                        n437 = local write "DISP LAB01-1"(w656) -> ()
                      }
                      frame #4 {
                        n438 = local read "SIG LAB01-1"() -> (w660:T2)
                        n439 = local read "TEMP START LAB01-1"() -> (w662:cluster{"TL":dbl, "TN":dbl})
                        n440 = Unbundle(w660) -> ("Tmp Live"=w659:dbl, "Tmp Neut"=w658:dbl)  [unwired: 3 out]
                        n441 = Bundle(cluster=w662, "TL"=w659, "TN"=w658) -> (w661:cluster{"TL":dbl, "TN":dbl})
                        n442 = local write "TEMP START LAB01-1"(w661) -> ()
                      }
                    }
                  }
                }
              }
              event "RUN LAB01-2": Value Change {
                n443 = event-data() -> ("NewVal"=w663:bool)  [unwired: 1 in, 5 out]
                n444 = local write "run lab01-2"(w663) -> ()
                n445 = case shown="True" w663 {
                  tunnel: w669 -> [_ w702]
                  tunnel: w668 -> [_ w701]
                  tunnel: w666 -> [w671 w700]
                  tunnel: w667 -> [_ w699]
                  tunnel: w665 -> [_ w698]
                  tunnel: [w670 w697] -> w664
                  frame False {
                    # "stop test"
                    n446 = stacked-sequence {
                      tunnel: w671 -> [w680 _]
                      tunnel: [w672 _] -> w670
                      frame #0 {
                        n447 = local read "DISP LAB01-2"() -> (w679:T4)
                        n448 = Unbundle(w679) -> ("CYCLE"=w677:dbl, "MINS"=w678:dbl)  [unwired: 1 out]
                        n449 = case shown="\"CHART TEST\", Default" w680 {
                          tunnel: w678 -> [_ _ w687]
                          tunnel: w677 -> [w685 w686 _]
                          tunnel: [w685 w686 w687] -> w676
                          frame "CHART TEST", Default {
                          }
                          frame "CYCLE TEST" {
                          }
                          frame "T-RISE TEST" {
                          }
                        }
                        n450 = local read "TDMS LAB01-2"() -> (w684:refnum<k34>)
                        n451 = Build Array("STOPPED") -> (w681:string[])
                        n452 = Build Array(w676) -> (w675:dbl[])
                        n453 = TDMS Write(0:w684, 5:"TEST RESULT", 7:w681, 9:w675) -> (4:w673:refnum<k34>, 15:w674:errorcluster)  [unwired: 2 in, 2 out]
                        n454 = TDMS Close(8:w674, 11:w673) -> (0:w672:errorcluster)  [unwired: 1 out]
                      }
                      frame #1 {
                        n455 = local read "DISP LAB01-2"() -> (w691:T4)
                        n456 = stacked-sequence {
                          tunnel: "LAB01-2" -> [w693 w695]
                          frame #0 {
                            n457 = call "sub vi - defrag tdms v1.vi"("panel id"=w693) -> ("error out"=w692:errorcluster)  [unwired: 10 in]
                            n458 = local write "data file error"(w692) -> ()
                          }
                          frame #1 {
                            n459 = call "Save data file to network drive v1.vi"("panel id"=w695) -> ("network file save error"=w694:errorcluster)  [unwired: 9 in, 1 out]
                            n460 = local write "RESULT LAB01-2"(FALSE) -> ()
                            n461 = local write "data file error"(w694) -> ()
                          }
                        }
                        n462 = Bundle(cluster=w691, "STATUS"="STOP") -> (w689:T4)  [unwired: 2 in]
                        n463 = local write "DISP LAB01-2"(w689) -> ()
                      }
                    }
                  }
                  frame True {
                    # "start new test and create test file"
                    n464 = stacked-sequence {
                      seq-local: [w703 _ _ _ _] -> [_ w728 _ _ _]
                      tunnel: w702 -> [w708 _ _ _ _]
                      tunnel: w701 -> [w705 _ _ _ _]
                      tunnel: w700 -> [w718 _ _ _ _]
                      tunnel: w699 -> [w711 _ _ _ _]
                      tunnel: w698 -> [w706 _ _ _ _]
                      tunnel: [_ w722 _ _ _] -> w697
                      frame #0 {
                        w704 = "\\"
                        n465 = local read "SET LAB01-2"() -> (w713:T5)
                        n466 = case shown="\"CYCLE TEST\"" w718 {
                          tunnel: ["L01-2-CHART TEST-" "L01-2-CYCLE TEST-" "L01-2-T-RISE TEST-"] -> w714
                          frame "CHART TEST", Default {
                          }
                          frame "CYCLE TEST" {
                          }
                          frame "T-RISE TEST" {
                          }
                        }
                        n467 = Unbundle(w713) -> ("DESCRIPTION"=w712:string)  [unwired: 4 out]
                        n468 = Concatenate Strings(w708, "\\", w706, w704, w705, w704) -> (w715:string)
                        n469 = String To Path(string=w715) -> (path=w717:path)
                        n470 = Concatenate Strings(w715, w714, w712, "-", w711, ".tdms") -> (w703:string)
                        n471 = Create Folder(path (use dialog)=w717) -> (error out=w716:errorcluster)  [unwired: 2 in, 2 out]
                        n472 = global write "Global 1.vi" "LAB01-2 FILE"(w703) -> ()
                        n473 = call <vilib>:"Clear Errors.vi"("error in (no error)"=w716) -> ()  [unwired: 6 in, 1 out]
                      }
                      frame #1 {
                        n474 = String To Path(string=w728) -> (path=w723:path)
                        n475 = TDMS Open(5:FALSE, 6:FALSE, 10:T19."create or replace" ("operation (0:open)"), 11:w723) -> (0:w722:errorcluster, 3:→"TDMS LAB01-2":refnum<k34>)  [unwired: 3 in]
                      }
                      frame #2 {
                        n476 = local read "SET LAB01-2"() -> (w734:T5)
                        n477 = local read "TDMS LAB01-2"() -> (w745:refnum<k34>)
                        n478 = Build Array("Testers Name", "Description", "Set Test Cycles", "T-Rise minutes", "T-Rise Deg C") -> (w735:string[])
                        n479 = Unbundle(w734) -> ("NAME"=w733:string, "DESCRIPTION"=w732:string, "CYCLES"=w731:dbl, "T-RISE mins"=w730:dbl, "T-RISE deg C"=w729:dbl)
                        n480 = Number To Decimal String(number=w731) -> (decimal integer string=w744:string)  [unwired: 1 in]
                        n481 = Number To Decimal String(number=w730) -> (decimal integer string=w743:string)  [unwired: 1 in]
                        n482 = Number To Decimal String(number=w729) -> (decimal integer string=w742:string)  [unwired: 1 in]
                        n483 = Build Array(w733, w732, w744, w743, w742) -> (w741:string[])
                        n484 = TDMS Set Properties(5:w741, 7:w735, 11:w745) -> ()  [unwired: 3 in, 4 out]
                      }
                      frame #3 {
                        w747 = 0.0
                        n485 = local read "DISP LAB01-2"() -> (w749:T4)
                        n486 = Bundle(cluster=w749, "CYCLE"=w747, "MINS"=w747, "STATUS"="RUN") -> (w748:T4)
                        n487 = local write "DISP LAB01-2"(w748) -> ()
                      }
                      frame #4 {
                        n488 = local read "SIG LAB01-2"() -> (w752:T2)
                        n489 = local read "TEMP START LAB01-2"() -> (w754:cluster{"TL":dbl, "TN":dbl})
                        n490 = Unbundle(w752) -> ("Tmp Live"=w751:dbl, "Tmp Neut"=w750:dbl)  [unwired: 3 out]
                        n491 = Bundle(cluster=w754, "TL"=w751, "TN"=w750) -> (w753:cluster{"TL":dbl, "TN":dbl})
                        n492 = local write "TEMP START LAB01-2"(w753) -> ()
                      }
                    }
                  }
                }
              }
              event "RUN LAB02-1": Value Change {
                n493 = event-data() -> ("NewVal"=w755:bool)  [unwired: 1 in, 5 out]
                n494 = local write "run lab02-1"(w755) -> ()
                n495 = case shown="True" w755 {
                  tunnel: w761 -> [_ w794]
                  tunnel: w760 -> [_ w793]
                  tunnel: w758 -> [w763 w792]
                  tunnel: w759 -> [_ w791]
                  tunnel: w757 -> [_ w790]
                  tunnel: [w762 w789] -> w756
                  frame False {
                    # "stop test"
                    n496 = stacked-sequence {
                      tunnel: w763 -> [w772 _]
                      tunnel: [w764 _] -> w762
                      frame #0 {
                        n497 = local read "DISP LAB02-1"() -> (w771:T4)
                        n498 = Unbundle(w771) -> ("CYCLE"=w769:dbl, "MINS"=w770:dbl)  [unwired: 1 out]
                        n499 = case shown="\"CYCLE TEST\"" w772 {
                          tunnel: w770 -> [_ _ w779]
                          tunnel: w769 -> [w777 w778 _]
                          tunnel: [w777 w778 w779] -> w768
                          frame "CHART TEST", Default {
                          }
                          frame "CYCLE TEST" {
                          }
                          frame "T-RISE TEST" {
                          }
                        }
                        n500 = local read "TDMS LAB02-1"() -> (w776:refnum<k34>)
                        n501 = Build Array("STOPPED") -> (w773:string[])
                        n502 = Build Array(w768) -> (w767:dbl[])
                        n503 = TDMS Write(0:w776, 5:"TEST RESULT", 7:w773, 9:w767) -> (4:w765:refnum<k34>, 15:w766:errorcluster)  [unwired: 2 in, 2 out]
                        n504 = TDMS Close(8:w766, 11:w765) -> (0:w764:errorcluster)  [unwired: 1 out]
                      }
                      frame #1 {
                        n505 = local read "DISP LAB02-1"() -> (w783:T4)
                        n506 = stacked-sequence {
                          tunnel: "LAB02-1" -> [w785 w787]
                          frame #0 {
                            n507 = call "sub vi - defrag tdms v1.vi"("panel id"=w785) -> ("error out"=w784:errorcluster)  [unwired: 10 in]
                            n508 = local write "data file error"(w784) -> ()
                          }
                          frame #1 {
                            n509 = local write "RESULT LAB02-1"(FALSE) -> ()
                            n510 = call "Save data file to network drive v1.vi"("panel id"=w787) -> ("network file save error"=w786:errorcluster)  [unwired: 9 in, 1 out]
                            n511 = local write "data file error"(w786) -> ()
                          }
                        }
                        n512 = Bundle(cluster=w783, "STATUS"="STOP") -> (w781:T4)  [unwired: 2 in]
                        n513 = local write "DISP LAB02-1"(w781) -> ()
                      }
                    }
                  }
                  frame True {
                    # "start new test and create test file"
                    n514 = stacked-sequence {
                      seq-local: [w795 _ _ _ _] -> [_ w820 _ _ _]
                      tunnel: w794 -> [w800 _ _ _ _]
                      tunnel: w793 -> [w797 _ _ _ _]
                      tunnel: w792 -> [w810 _ _ _ _]
                      tunnel: w791 -> [w803 _ _ _ _]
                      tunnel: w790 -> [w798 _ _ _ _]
                      tunnel: [_ w814 _ _ _] -> w789
                      frame #0 {
                        w796 = "\\"
                        n515 = local read "SET LAB02-1"() -> (w805:T5)
                        n516 = case shown="\"CYCLE TEST\"" w810 {
                          tunnel: ["L02-1-CHART TEST-" "L02-1-CYCLE TEST-" "L02-1-T-RISE TEST-"] -> w806
                          frame "CHART TEST", Default {
                          }
                          frame "CYCLE TEST" {
                          }
                          frame "T-RISE TEST" {
                          }
                        }
                        n517 = Unbundle(w805) -> ("DESCRIPTION"=w804:string)  [unwired: 4 out]
                        n518 = Concatenate Strings(w800, "\\", w798, w796, w797, w796) -> (w807:string)
                        n519 = String To Path(string=w807) -> (path=w809:path)
                        n520 = Concatenate Strings(w807, w806, w804, "-", w803, ".tdms") -> (w795:string)
                        n521 = Create Folder(path (use dialog)=w809) -> (error out=w808:errorcluster)  [unwired: 2 in, 2 out]
                        n522 = global write "Global 1.vi" "LAB02-1 FILE"(w795) -> ()
                        n523 = call <vilib>:"Clear Errors.vi"("error in (no error)"=w808) -> ()  [unwired: 6 in, 1 out]
                      }
                      frame #1 {
                        n524 = String To Path(string=w820) -> (path=w815:path)
                        n525 = TDMS Open(5:FALSE, 6:FALSE, 10:T19."create or replace" ("operation (0:open)"), 11:w815) -> (0:w814:errorcluster, 3:→"TDMS LAB02-1":refnum<k34>)  [unwired: 3 in]
                      }
                      frame #2 {
                        n526 = local read "SET LAB02-1"() -> (w826:T5)
                        n527 = local read "TDMS LAB02-1"() -> (w837:refnum<k34>)
                        n528 = Build Array("Testers Name", "Description", "Set Test Cycles", "T-Rise minutes", "T-Rise Deg C") -> (w827:string[])
                        n529 = Unbundle(w826) -> ("NAME"=w825:string, "DESCRIPTION"=w824:string, "CYCLES"=w823:dbl, "T-RISE mins"=w822:dbl, "T-RISE deg C"=w821:dbl)
                        n530 = Number To Decimal String(number=w823) -> (decimal integer string=w836:string)  [unwired: 1 in]
                        n531 = Number To Decimal String(number=w822) -> (decimal integer string=w835:string)  [unwired: 1 in]
                        n532 = Number To Decimal String(number=w821) -> (decimal integer string=w834:string)  [unwired: 1 in]
                        n533 = Build Array(w825, w824, w836, w835, w834) -> (w833:string[])
                        n534 = TDMS Set Properties(5:w833, 7:w827, 11:w837) -> ()  [unwired: 3 in, 4 out]
                      }
                      frame #3 {
                        w839 = 0.0
                        n535 = local read "DISP LAB02-1"() -> (w841:T4)
                        n536 = Bundle(cluster=w841, "CYCLE"=w839, "MINS"=w839, "STATUS"="RUN") -> (w840:T4)
                        n537 = local write "DISP LAB02-1"(w840) -> ()
                      }
                      frame #4 {
                        n538 = local read "SIG LAB02-1"() -> (w844:T2)
                        n539 = local read "TEMP START LAB02-1"() -> (w846:cluster{"TL":dbl, "TN":dbl})
                        n540 = Unbundle(w844) -> ("Tmp Live"=w843:dbl, "Tmp Neut"=w842:dbl)  [unwired: 3 out]
                        n541 = Bundle(cluster=w846, "TL"=w843, "TN"=w842) -> (w845:cluster{"TL":dbl, "TN":dbl})
                        n542 = local write "TEMP START LAB02-1"(w845) -> ()
                      }
                    }
                  }
                }
              }
              event "RUN LAB02-2": Value Change {
                n543 = event-data() -> ("NewVal"=w847:bool)  [unwired: 1 in, 5 out]
                n544 = local write "run lab02-2"(w847) -> ()
                n545 = case shown="True" w847 {
                  tunnel: w853 -> [_ w886]
                  tunnel: w852 -> [_ w885]
                  tunnel: w850 -> [w855 w884]
                  tunnel: w851 -> [_ w883]
                  tunnel: w849 -> [_ w882]
                  tunnel: [w854 w881] -> w848
                  frame False {
                    # "stop test"
                    n546 = stacked-sequence {
                      tunnel: w855 -> [w864 _]
                      tunnel: [w856 _] -> w854
                      frame #0 {
                        n547 = local read "DISP LAB02-2"() -> (w863:T4)
                        n548 = Unbundle(w863) -> ("CYCLE"=w861:dbl, "MINS"=w862:dbl)  [unwired: 1 out]
                        n549 = case shown="\"CYCLE TEST\"" w864 {
                          tunnel: w862 -> [_ _ w871]
                          tunnel: w861 -> [w869 w870 _]
                          tunnel: [w869 w870 w871] -> w860
                          frame "CHART TEST", Default {
                          }
                          frame "CYCLE TEST" {
                          }
                          frame "T-RISE TEST" {
                          }
                        }
                        n550 = local read "TDMS LAB02-2"() -> (w868:refnum<k34>)
                        n551 = Build Array("STOPPED") -> (w865:string[])
                        n552 = Build Array(w860) -> (w859:dbl[])
                        n553 = TDMS Write(0:w868, 5:"TEST RESULT", 7:w865, 9:w859) -> (4:w857:refnum<k34>, 15:w858:errorcluster)  [unwired: 2 in, 2 out]
                        n554 = TDMS Close(8:w858, 11:w857) -> (0:w856:errorcluster)  [unwired: 1 out]
                      }
                      frame #1 {
                        n555 = local read "DISP LAB02-2"() -> (w875:T4)
                        n556 = stacked-sequence {
                          tunnel: "LAB02-2" -> [w877 w879]
                          frame #0 {
                            n557 = call "sub vi - defrag tdms v1.vi"("panel id"=w877) -> ("error out"=w876:errorcluster)  [unwired: 10 in]
                            n558 = local write "data file error"(w876) -> ()
                          }
                          frame #1 {
                            n559 = call "Save data file to network drive v1.vi"("panel id"=w879) -> ("network file save error"=w878:errorcluster)  [unwired: 9 in, 1 out]
                            n560 = local write "RESULT LAB02-2"(FALSE) -> ()
                            n561 = local write "data file error"(w878) -> ()
                          }
                        }
                        n562 = Bundle(cluster=w875, "STATUS"="STOP") -> (w873:T4)  [unwired: 2 in]
                        n563 = local write "DISP LAB02-2"(w873) -> ()
                      }
                    }
                  }
                  frame True {
                    # "start new test and create test file"
                    n564 = stacked-sequence {
                      seq-local: [w887 _ _ _ _] -> [_ w912 _ _ _]
                      tunnel: w886 -> [w892 _ _ _ _]
                      tunnel: w885 -> [w889 _ _ _ _]
                      tunnel: w884 -> [w902 _ _ _ _]
                      tunnel: w883 -> [w895 _ _ _ _]
                      tunnel: w882 -> [w890 _ _ _ _]
                      tunnel: [_ w906 _ _ _] -> w881
                      frame #0 {
                        w888 = "\\"
                        n565 = local read "SET LAB02-2"() -> (w897:T5)
                        n566 = case shown="\"CYCLE TEST\"" w902 {
                          tunnel: ["L02-2-CHART TEST-" "L02-2-CYCLE TEST-" "L02-2-T-RISE TEST-"] -> w898
                          frame "CHART TEST", Default {
                          }
                          frame "CYCLE TEST" {
                          }
                          frame "T-RISE TEST" {
                          }
                        }
                        n567 = Unbundle(w897) -> ("DESCRIPTION"=w896:string)  [unwired: 4 out]
                        n568 = Concatenate Strings(w892, "\\", w890, w888, w889, w888) -> (w899:string)
                        n569 = String To Path(string=w899) -> (path=w901:path)
                        n570 = Concatenate Strings(w899, w898, w896, "-", w895, ".tdms") -> (w887:string)
                        n571 = Create Folder(path (use dialog)=w901) -> (error out=w900:errorcluster)  [unwired: 2 in, 2 out]
                        n572 = global write "Global 1.vi" "LAB02-2 FILE"(w887) -> ()
                        n573 = call <vilib>:"Clear Errors.vi"("error in (no error)"=w900) -> ()  [unwired: 6 in, 1 out]
                      }
                      frame #1 {
                        n574 = String To Path(string=w912) -> (path=w907:path)
                        n575 = TDMS Open(5:FALSE, 6:FALSE, 10:T19."create or replace" ("operation (0:open)"), 11:w907) -> (0:w906:errorcluster, 3:→"TDMS LAB02-2":refnum<k34>)  [unwired: 3 in]
                      }
                      frame #2 {
                        n576 = local read "SET LAB02-2"() -> (w918:T5)
                        n577 = local read "TDMS LAB02-2"() -> (w929:refnum<k34>)
                        n578 = Build Array("Testers Name", "Description", "Set Test Cycles", "T-Rise minutes", "T-Rise Deg C") -> (w919:string[])
                        n579 = Unbundle(w918) -> ("NAME"=w917:string, "DESCRIPTION"=w916:string, "CYCLES"=w915:dbl, "T-RISE mins"=w914:dbl, "T-RISE deg C"=w913:dbl)
                        n580 = Number To Decimal String(number=w915) -> (decimal integer string=w928:string)  [unwired: 1 in]
                        n581 = Number To Decimal String(number=w914) -> (decimal integer string=w927:string)  [unwired: 1 in]
                        n582 = Number To Decimal String(number=w913) -> (decimal integer string=w926:string)  [unwired: 1 in]
                        n583 = Build Array(w917, w916, w928, w927, w926) -> (w925:string[])
                        n584 = TDMS Set Properties(5:w925, 7:w919, 11:w929) -> ()  [unwired: 3 in, 4 out]
                      }
                      frame #3 {
                        w931 = 0.0
                        n585 = local read "DISP LAB02-2"() -> (w933:T4)
                        n586 = Bundle(cluster=w933, "CYCLE"=w931, "MINS"=w931, "STATUS"="RUN") -> (w932:T4)
                        n587 = local write "DISP LAB02-2"(w932) -> ()
                      }
                      frame #4 {
                        n588 = local read "SIG LAB02-2"() -> (w936:T2)
                        n589 = local read "TEMP START LAB02-2"() -> (w938:cluster{"TL":dbl, "TN":dbl})
                        n590 = Unbundle(w936) -> ("Tmp Live"=w935:dbl, "Tmp Neut"=w934:dbl)  [unwired: 3 out]
                        n591 = Bundle(cluster=w938, "TL"=w935, "TN"=w934) -> (w937:cluster{"TL":dbl, "TN":dbl})
                        n592 = local write "TEMP START LAB02-2"(w937) -> ()
                      }
                    }
                  }
                }
              }
              event "RUN LAB03-1": Value Change {
                n593 = event-data() -> ("NewVal"=w939:bool)  [unwired: 1 in, 5 out]
                n594 = local write "run lab03-1"(w939) -> ()
                n595 = case shown="True" w939 {
                  tunnel: w945 -> [_ w978]
                  tunnel: w944 -> [_ w977]
                  tunnel: w942 -> [w947 w976]
                  tunnel: w943 -> [_ w975]
                  tunnel: w941 -> [_ w974]
                  tunnel: [w946 w973] -> w940
                  frame False {
                    # "stop test"
                    n596 = stacked-sequence {
                      tunnel: w947 -> [w956 _]
                      tunnel: [w948 _] -> w946
                      frame #0 {
                        n597 = local read "DISP LAB03-1"() -> (w955:T4)
                        n598 = Unbundle(w955) -> ("CYCLE"=w953:dbl, "MINS"=w954:dbl)  [unwired: 1 out]
                        n599 = case shown="\"CYCLE TEST\"" w956 {
                          tunnel: w954 -> [_ _ w963]
                          tunnel: w953 -> [w961 w962 _]
                          tunnel: [w961 w962 w963] -> w952
                          frame "CHART TEST", Default {
                          }
                          frame "CYCLE TEST" {
                          }
                          frame "T-RISE TEST" {
                          }
                        }
                        n600 = local read "TDMS LAB03-1"() -> (w960:refnum<k34>)
                        n601 = Build Array("STOPPED") -> (w957:string[])
                        n602 = Build Array(w952) -> (w951:dbl[])
                        n603 = TDMS Write(0:w960, 5:"TEST RESULT", 7:w957, 9:w951) -> (4:w949:refnum<k34>, 15:w950:errorcluster)  [unwired: 2 in, 2 out]
                        n604 = TDMS Close(8:w950, 11:w949) -> (0:w948:errorcluster)  [unwired: 1 out]
                      }
                      frame #1 {
                        n605 = local read "DISP LAB03-1"() -> (w967:T4)
                        n606 = stacked-sequence {
                          tunnel: "LAB03-1" -> [w969 w971]
                          frame #0 {
                            n607 = call "sub vi - defrag tdms v1.vi"("panel id"=w969) -> ("error out"=w968:errorcluster)  [unwired: 10 in]
                            n608 = local write "data file error"(w968) -> ()
                          }
                          frame #1 {
                            n609 = call "Save data file to network drive v1.vi"("panel id"=w971) -> ("network file save error"=w970:errorcluster)  [unwired: 9 in, 1 out]
                            n610 = local write "RESULT LAB03-1"(FALSE) -> ()
                            n611 = local write "data file error"(w970) -> ()
                          }
                        }
                        n612 = Bundle(cluster=w967, "STATUS"="STOP") -> (w965:T4)  [unwired: 2 in]
                        n613 = local write "DISP LAB03-1"(w965) -> ()
                      }
                    }
                  }
                  frame True {
                    # "start new test and create test file"
                    n614 = stacked-sequence {
                      seq-local: [w979 _ _ _ _] -> [_ w1004 _ _ _]
                      tunnel: w978 -> [w984 _ _ _ _]
                      tunnel: w977 -> [w981 _ _ _ _]
                      tunnel: w976 -> [w994 _ _ _ _]
                      tunnel: w975 -> [w987 _ _ _ _]
                      tunnel: w974 -> [w982 _ _ _ _]
                      tunnel: [_ w998 _ _ _] -> w973
                      frame #0 {
                        w980 = "\\"
                        n615 = local read "SET LAB03-1"() -> (w989:T5)
                        n616 = case shown="\"T-RISE TEST\"" w994 {
                          tunnel: ["L03-1-CHART TEST-" "L03-1-CYCLE TEST-" "L03-1-T-RISE TEST-"] -> w990
                          frame "CHART TEST", Default {
                          }
                          frame "CYCLE TEST" {
                          }
                          frame "T-RISE TEST" {
                          }
                        }
                        n617 = Unbundle(w989) -> ("DESCRIPTION"=w988:string)  [unwired: 4 out]
                        n618 = Concatenate Strings(w984, "\\", w982, w980, w981, w980) -> (w991:string)
                        n619 = String To Path(string=w991) -> (path=w993:path)
                        n620 = Concatenate Strings(w991, w990, w988, "-", w987, ".tdms") -> (w979:string)
                        n621 = Create Folder(path (use dialog)=w993) -> (error out=w992:errorcluster)  [unwired: 2 in, 2 out]
                        n622 = global write "Global 1.vi" "LAB03-1 FILE"(w979) -> ()
                        n623 = call <vilib>:"Clear Errors.vi"("error in (no error)"=w992) -> ()  [unwired: 6 in, 1 out]
                      }
                      frame #1 {
                        n624 = String To Path(string=w1004) -> (path=w999:path)
                        n625 = TDMS Open(5:FALSE, 6:FALSE, 10:T19."create or replace" ("operation (0:open)"), 11:w999) -> (0:w998:errorcluster, 3:→"TDMS LAB03-1":refnum<k34>)  [unwired: 3 in]
                      }
                      frame #2 {
                        n626 = local read "SET LAB03-1"() -> (w1010:T5)
                        n627 = local read "TDMS LAB03-1"() -> (w1021:refnum<k34>)
                        n628 = Build Array("Testers Name", "Description", "Set Test Cycles", "T-Rise minutes", "T-Rise Deg C") -> (w1011:string[])
                        n629 = Unbundle(w1010) -> ("NAME"=w1009:string, "DESCRIPTION"=w1008:string, "CYCLES"=w1007:dbl, "T-RISE mins"=w1006:dbl, "T-RISE deg C"=w1005:dbl)
                        n630 = Number To Decimal String(number=w1007) -> (decimal integer string=w1020:string)  [unwired: 1 in]
                        n631 = Number To Decimal String(number=w1006) -> (decimal integer string=w1019:string)  [unwired: 1 in]
                        n632 = Number To Decimal String(number=w1005) -> (decimal integer string=w1018:string)  [unwired: 1 in]
                        n633 = Build Array(w1009, w1008, w1020, w1019, w1018) -> (w1017:string[])
                        n634 = TDMS Set Properties(5:w1017, 7:w1011, 11:w1021) -> ()  [unwired: 3 in, 4 out]
                      }
                      frame #3 {
                        w1023 = 0.0
                        n635 = local read "DISP LAB03-1"() -> (w1025:T4)
                        n636 = Bundle(cluster=w1025, "CYCLE"=w1023, "MINS"=w1023, "STATUS"="RUN") -> (w1024:T4)
                        n637 = local write "DISP LAB03-1"(w1024) -> ()
                      }
                      frame #4 {
                        n638 = local read "SIG LAB03-1"() -> (w1028:T2)
                        n639 = local read "TEMP START LAB03-1"() -> (w1030:cluster{"TL":dbl, "TN":dbl})
                        n640 = Unbundle(w1028) -> ("Tmp Live"=w1027:dbl, "Tmp Neut"=w1026:dbl)  [unwired: 3 out]
                        n641 = Bundle(cluster=w1030, "TL"=w1027, "TN"=w1026) -> (w1029:cluster{"TL":dbl, "TN":dbl})
                        n642 = local write "TEMP START LAB03-1"(w1029) -> ()
                      }
                    }
                  }
                }
              }
              event "RUN LAB03-2": Value Change {
                n643 = event-data() -> ("NewVal"=w1031:bool)  [unwired: 1 in, 5 out]
                n644 = local write "run lab03-2"(w1031) -> ()
                n645 = case shown="True" w1031 {
                  tunnel: w1037 -> [_ w1070]
                  tunnel: w1036 -> [_ w1069]
                  tunnel: w1034 -> [w1039 w1068]
                  tunnel: w1035 -> [_ w1067]
                  tunnel: w1033 -> [_ w1066]
                  tunnel: [w1038 w1065] -> w1032
                  frame False {
                    # "stop test"
                    n646 = stacked-sequence {
                      tunnel: w1039 -> [w1048 _]
                      tunnel: [w1040 _] -> w1038
                      frame #0 {
                        n647 = local read "DISP LAB03-2"() -> (w1047:T4)
                        n648 = Unbundle(w1047) -> ("CYCLE"=w1045:dbl, "MINS"=w1046:dbl)  [unwired: 1 out]
                        n649 = case shown="\"CYCLE TEST\"" w1048 {
                          tunnel: w1046 -> [_ _ w1055]
                          tunnel: w1045 -> [w1053 w1054 _]
                          tunnel: [w1053 w1054 w1055] -> w1044
                          frame "CHART TEST", Default {
                          }
                          frame "CYCLE TEST" {
                          }
                          frame "T-RISE TEST" {
                          }
                        }
                        n650 = local read "TDMS LAB03-2"() -> (w1052:refnum<k34>)
                        n651 = Build Array("STOPPED") -> (w1049:string[])
                        n652 = Build Array(w1044) -> (w1043:dbl[])
                        n653 = TDMS Write(0:w1052, 5:"TEST RESULT", 7:w1049, 9:w1043) -> (4:w1041:refnum<k34>, 15:w1042:errorcluster)  [unwired: 2 in, 2 out]
                        n654 = TDMS Close(8:w1042, 11:w1041) -> (0:w1040:errorcluster)  [unwired: 1 out]
                      }
                      frame #1 {
                        n655 = local read "DISP LAB03-2"() -> (w1059:T4)
                        n656 = stacked-sequence {
                          tunnel: "LAB03-2" -> [w1061 w1063]
                          frame #0 {
                            n657 = call "sub vi - defrag tdms v1.vi"("panel id"=w1061) -> ("error out"=w1060:errorcluster)  [unwired: 10 in]
                            n658 = local write "data file error"(w1060) -> ()
                          }
                          frame #1 {
                            n659 = call "Save data file to network drive v1.vi"("panel id"=w1063) -> ("network file save error"=w1062:errorcluster)  [unwired: 9 in, 1 out]
                            n660 = local write "RESULT LAB03-2"(FALSE) -> ()
                            n661 = local write "data file error"(w1062) -> ()
                          }
                        }
                        n662 = Bundle(cluster=w1059, "STATUS"="STOP") -> (w1057:T4)  [unwired: 2 in]
                        n663 = local write "DISP LAB03-2"(w1057) -> ()
                      }
                    }
                  }
                  frame True {
                    # "start new test and create test file"
                    n664 = stacked-sequence {
                      seq-local: [w1071 _ _ _ _] -> [_ w1096 _ _ _]
                      tunnel: w1070 -> [w1076 _ _ _ _]
                      tunnel: w1069 -> [w1073 _ _ _ _]
                      tunnel: w1068 -> [w1086 _ _ _ _]
                      tunnel: w1067 -> [w1079 _ _ _ _]
                      tunnel: w1066 -> [w1074 _ _ _ _]
                      tunnel: [_ w1090 _ _ _] -> w1065
                      frame #0 {
                        w1072 = "\\"
                        n665 = local read "SET LAB03-2"() -> (w1081:T5)
                        n666 = case shown="\"T-RISE TEST\"" w1086 {
                          tunnel: ["L03-2-CHART TEST-" "L03-2-CYCLE TEST-" "L03-2-T-RISE TEST-"] -> w1082
                          frame "CHART TEST", Default {
                          }
                          frame "CYCLE TEST" {
                          }
                          frame "T-RISE TEST" {
                          }
                        }
                        n667 = Unbundle(w1081) -> ("DESCRIPTION"=w1080:string)  [unwired: 4 out]
                        n668 = Concatenate Strings(w1076, "\\", w1074, w1072, w1073, w1072) -> (w1083:string)
                        n669 = String To Path(string=w1083) -> (path=w1085:path)
                        n670 = Concatenate Strings(w1083, w1082, w1080, "-", w1079, ".tdms") -> (w1071:string)
                        n671 = Create Folder(path (use dialog)=w1085) -> (error out=w1084:errorcluster)  [unwired: 2 in, 2 out]
                        n672 = global write "Global 1.vi" "LAB03-2 FILE"(w1071) -> ()
                        n673 = call <vilib>:"Clear Errors.vi"("error in (no error)"=w1084) -> ()  [unwired: 6 in, 1 out]
                      }
                      frame #1 {
                        n674 = String To Path(string=w1096) -> (path=w1091:path)
                        n675 = TDMS Open(5:FALSE, 6:FALSE, 10:T19."create or replace" ("operation (0:open)"), 11:w1091) -> (0:w1090:errorcluster, 3:→"TDMS LAB03-2":refnum<k34>)  [unwired: 3 in]
                      }
                      frame #2 {
                        n676 = local read "SET LAB03-2"() -> (w1102:T5)
                        n677 = local read "TDMS LAB03-2"() -> (w1113:refnum<k34>)
                        n678 = Build Array("Testers Name", "Description", "Set Test Cycles", "T-Rise minutes", "T-Rise Deg C") -> (w1103:string[])
                        n679 = Unbundle(w1102) -> ("NAME"=w1101:string, "DESCRIPTION"=w1100:string, "CYCLES"=w1099:dbl, "T-RISE mins"=w1098:dbl, "T-RISE deg C"=w1097:dbl)
                        n680 = Number To Decimal String(number=w1099) -> (decimal integer string=w1112:string)  [unwired: 1 in]
                        n681 = Number To Decimal String(number=w1098) -> (decimal integer string=w1111:string)  [unwired: 1 in]
                        n682 = Number To Decimal String(number=w1097) -> (decimal integer string=w1110:string)  [unwired: 1 in]
                        n683 = Build Array(w1101, w1100, w1112, w1111, w1110) -> (w1109:string[])
                        n684 = TDMS Set Properties(5:w1109, 7:w1103, 11:w1113) -> ()  [unwired: 3 in, 4 out]
                      }
                      frame #3 {
                        w1115 = 0.0
                        n685 = local read "DISP LAB03-2"() -> (w1117:T4)
                        n686 = Bundle(cluster=w1117, "CYCLE"=w1115, "MINS"=w1115, "STATUS"="RUN") -> (w1116:T4)
                        n687 = local write "DISP LAB03-2"(w1116) -> ()
                      }
                      frame #4 {
                        n688 = local read "SIG LAB03-2"() -> (w1120:T2)
                        n689 = local read "TEMP START LAB03-2"() -> (w1122:cluster{"TL":dbl, "TN":dbl})
                        n690 = Unbundle(w1120) -> ("Tmp Live"=w1119:dbl, "Tmp Neut"=w1118:dbl)  [unwired: 3 out]
                        n691 = Bundle(cluster=w1122, "TL"=w1119, "TN"=w1118) -> (w1121:cluster{"TL":dbl, "TN":dbl})
                        n692 = local write "TEMP START LAB03-2"(w1121) -> ()
                      }
                    }
                  }
                }
              }
              event "RUN LAB04-1": Value Change {
                n693 = event-data() -> ("NewVal"=w1123:bool)  [unwired: 1 in, 5 out]
                n694 = local write "run lab04-1"(w1123) -> ()
                n695 = case shown="True" w1123 {
                  tunnel: w1129 -> [_ w1162]
                  tunnel: w1128 -> [_ w1161]
                  tunnel: w1126 -> [w1131 w1160]
                  tunnel: w1127 -> [_ w1159]
                  tunnel: w1125 -> [_ w1158]
                  tunnel: [w1130 w1157] -> w1124
                  frame False {
                    # "stop test"
                    n696 = stacked-sequence {
                      tunnel: w1131 -> [w1140 _]
                      tunnel: [w1132 _] -> w1130
                      frame #0 {
                        n697 = local read "DISP LAB04-1"() -> (w1139:T4)
                        n698 = Unbundle(w1139) -> ("CYCLE"=w1137:dbl, "MINS"=w1138:dbl)  [unwired: 1 out]
                        n699 = case shown="\"CYCLE TEST\"" w1140 {
                          tunnel: w1138 -> [_ _ w1147]
                          tunnel: w1137 -> [w1145 w1146 _]
                          tunnel: [w1145 w1146 w1147] -> w1136
                          frame "CHART TEST", Default {
                          }
                          frame "CYCLE TEST" {
                          }
                          frame "T-RISE TEST" {
                          }
                        }
                        n700 = local read "TDMS LAB04-1"() -> (w1144:refnum<k34>)
                        n701 = Build Array("STOPPED") -> (w1141:string[])
                        n702 = Build Array(w1136) -> (w1135:dbl[])
                        n703 = TDMS Write(0:w1144, 5:"TEST RESULT", 7:w1141, 9:w1135) -> (4:w1133:refnum<k34>, 15:w1134:errorcluster)  [unwired: 2 in, 2 out]
                        n704 = TDMS Close(8:w1134, 11:w1133) -> (0:w1132:errorcluster)  [unwired: 1 out]
                      }
                      frame #1 {
                        n705 = local read "DISP LAB04-1"() -> (w1151:T4)
                        n706 = stacked-sequence {
                          tunnel: "LAB04-1" -> [w1153 w1155]
                          frame #0 {
                            n707 = call "sub vi - defrag tdms v1.vi"("panel id"=w1153) -> ("error out"=w1152:errorcluster)  [unwired: 10 in]
                            n708 = local write "data file error"(w1152) -> ()
                          }
                          frame #1 {
                            n709 = call "Save data file to network drive v1.vi"("panel id"=w1155) -> ("network file save error"=w1154:errorcluster)  [unwired: 9 in, 1 out]
                            n710 = local write "RESULT LAB04-1"(FALSE) -> ()
                            n711 = local write "data file error"(w1154) -> ()
                          }
                        }
                        n712 = Bundle(cluster=w1151, "STATUS"="STOP") -> (w1149:T4)  [unwired: 2 in]
                        n713 = local write "DISP LAB04-1"(w1149) -> ()
                      }
                    }
                  }
                  frame True {
                    # "start new test and create test file"
                    n714 = stacked-sequence {
                      seq-local: [w1163 _ _ _ _] -> [_ w1188 _ _ _]
                      tunnel: w1162 -> [w1168 _ _ _ _]
                      tunnel: w1161 -> [w1164 _ _ _ _]
                      tunnel: w1160 -> [w1178 _ _ _ _]
                      tunnel: w1159 -> [w1171 _ _ _ _]
                      tunnel: w1158 -> [w1166 _ _ _ _]
                      tunnel: [_ w1182 _ _ _] -> w1157
                      frame #0 {
                        w1165 = "\\"
                        n715 = local read "SET LAB04-1"() -> (w1173:T5)
                        n716 = case shown="\"CYCLE TEST\"" w1178 {
                          tunnel: ["L04-1-CHART TEST-" "L04-1-CYCLE TEST-" "L04-1-T-RISE TEST-"] -> w1174
                          frame "CHART TEST", Default {
                          }
                          frame "CYCLE TEST" {
                          }
                          frame "T-RISE TEST" {
                          }
                        }
                        n717 = Unbundle(w1173) -> ("DESCRIPTION"=w1172:string)  [unwired: 4 out]
                        n718 = Concatenate Strings(w1168, "\\", w1166, w1165, w1164, w1165) -> (w1175:string)
                        n719 = String To Path(string=w1175) -> (path=w1177:path)
                        n720 = Concatenate Strings(w1175, w1174, w1172, "-", w1171, ".tdms") -> (w1163:string)
                        n721 = Create Folder(path (use dialog)=w1177) -> (error out=w1176:errorcluster)  [unwired: 2 in, 2 out]
                        n722 = global write "Global 1.vi" "LAB04-1 FILE"(w1163) -> ()
                        n723 = call <vilib>:"Clear Errors.vi"("error in (no error)"=w1176) -> ()  [unwired: 6 in, 1 out]
                      }
                      frame #1 {
                        n724 = String To Path(string=w1188) -> (path=w1183:path)
                        n725 = TDMS Open(5:FALSE, 6:FALSE, 10:T19."create or replace" ("operation (0:open)"), 11:w1183) -> (0:w1182:errorcluster, 3:→"TDMS LAB04-1":refnum<k34>)  [unwired: 3 in]
                      }
                      frame #2 {
                        n726 = local read "SET LAB04-1"() -> (w1194:T5)
                        n727 = local read "TDMS LAB04-1"() -> (w1205:refnum<k34>)
                        n728 = Build Array("Testers Name", "Description", "Set Test Cycles", "T-Rise minutes", "T-Rise Deg C") -> (w1195:string[])
                        n729 = Unbundle(w1194) -> ("NAME"=w1193:string, "DESCRIPTION"=w1192:string, "CYCLES"=w1191:dbl, "T-RISE mins"=w1190:dbl, "T-RISE deg C"=w1189:dbl)
                        n730 = Number To Decimal String(number=w1191) -> (decimal integer string=w1204:string)  [unwired: 1 in]
                        n731 = Number To Decimal String(number=w1190) -> (decimal integer string=w1203:string)  [unwired: 1 in]
                        n732 = Number To Decimal String(number=w1189) -> (decimal integer string=w1202:string)  [unwired: 1 in]
                        n733 = Build Array(w1193, w1192, w1204, w1203, w1202) -> (w1201:string[])
                        n734 = TDMS Set Properties(5:w1201, 7:w1195, 11:w1205) -> ()  [unwired: 3 in, 4 out]
                      }
                      frame #3 {
                        w1207 = 0.0
                        n735 = local read "DISP LAB04-1"() -> (w1209:T4)
                        n736 = Bundle(cluster=w1209, "CYCLE"=w1207, "MINS"=w1207, "STATUS"="RUN") -> (w1208:T4)
                        n737 = local write "DISP LAB04-1"(w1208) -> ()
                      }
                      frame #4 {
                        n738 = local read "SIG LAB04-1"() -> (w1212:T2)
                        n739 = local read "TEMP START LAB04-1"() -> (w1214:cluster{"TL":dbl, "TN":dbl})
                        n740 = Unbundle(w1212) -> ("Tmp Live"=w1211:dbl, "Tmp Neut"=w1210:dbl)  [unwired: 3 out]
                        n741 = Bundle(cluster=w1214, "TL"=w1211, "TN"=w1210) -> (w1213:cluster{"TL":dbl, "TN":dbl})
                        n742 = local write "TEMP START LAB04-1"(w1213) -> ()
                      }
                    }
                  }
                }
              }
              event "RUN LAB04-2": Value Change {
                n743 = event-data() -> ("NewVal"=w1215:bool)  [unwired: 1 in, 5 out]
                n744 = local write "run lab04-2"(w1215) -> ()
                n745 = case shown="True" w1215 {
                  tunnel: w1221 -> [_ w1254]
                  tunnel: w1220 -> [_ w1253]
                  tunnel: w1218 -> [w1223 w1252]
                  tunnel: w1219 -> [_ w1251]
                  tunnel: w1217 -> [_ w1250]
                  tunnel: [w1222 w1249] -> w1216
                  frame False {
                    # "stop test"
                    n746 = stacked-sequence {
                      tunnel: w1223 -> [w1232 _]
                      tunnel: [w1224 _] -> w1222
                      frame #0 {
                        n747 = local read "DISP LAB04-2"() -> (w1231:T4)
                        n748 = Unbundle(w1231) -> ("CYCLE"=w1229:dbl, "MINS"=w1230:dbl)  [unwired: 1 out]
                        n749 = case shown="\"CYCLE TEST\"" w1232 {
                          tunnel: w1230 -> [_ _ w1239]
                          tunnel: w1229 -> [w1237 w1238 _]
                          tunnel: [w1237 w1238 w1239] -> w1228
                          frame "CHART TEST", Default {
                          }
                          frame "CYCLE TEST" {
                          }
                          frame "T-RISE TEST" {
                          }
                        }
                        n750 = local read "TDMS LAB04-2"() -> (w1236:refnum<k34>)
                        n751 = Build Array("STOPPED") -> (w1233:string[])
                        n752 = Build Array(w1228) -> (w1227:dbl[])
                        n753 = TDMS Write(0:w1236, 5:"TEST RESULT", 7:w1233, 9:w1227) -> (4:w1225:refnum<k34>, 15:w1226:errorcluster)  [unwired: 2 in, 2 out]
                        n754 = TDMS Close(8:w1226, 11:w1225) -> (0:w1224:errorcluster)  [unwired: 1 out]
                      }
                      frame #1 {
                        n755 = local read "DISP LAB04-2"() -> (w1243:T4)
                        n756 = stacked-sequence {
                          tunnel: "LAB04-2" -> [w1245 w1247]
                          frame #0 {
                            n757 = call "sub vi - defrag tdms v1.vi"("panel id"=w1245) -> ("error out"=w1244:errorcluster)  [unwired: 10 in]
                            n758 = local write "data file error"(w1244) -> ()
                          }
                          frame #1 {
                            n759 = call "Save data file to network drive v1.vi"("panel id"=w1247) -> ("network file save error"=w1246:errorcluster)  [unwired: 9 in, 1 out]
                            n760 = local write "RESULT LAB04-2"(FALSE) -> ()
                            n761 = local write "data file error"(w1246) -> ()
                          }
                        }
                        n762 = Bundle(cluster=w1243, "STATUS"="STOP") -> (w1241:T4)  [unwired: 2 in]
                        n763 = local write "DISP LAB04-2"(w1241) -> ()
                      }
                    }
                  }
                  frame True {
                    # "start new test and create test file"
                    n764 = stacked-sequence {
                      seq-local: [w1255 _ _ _ _] -> [_ w1280 _ _ _]
                      tunnel: w1254 -> [w1260 _ _ _ _]
                      tunnel: w1253 -> [w1256 _ _ _ _]
                      tunnel: w1252 -> [w1270 _ _ _ _]
                      tunnel: w1251 -> [w1263 _ _ _ _]
                      tunnel: w1250 -> [w1258 _ _ _ _]
                      tunnel: [_ w1274 _ _ _] -> w1249
                      frame #0 {
                        w1257 = "\\"
                        n765 = local read "SET LAB04-2"() -> (w1265:T5)
                        n766 = case shown="\"CHART TEST\", Default" w1270 {
                          tunnel: ["L04-2-CHART TEST-" "L04-2-CYCLE TEST-" "L04-2-T-RISE TEST-"] -> w1266
                          frame "CHART TEST", Default {
                          }
                          frame "CYCLE TEST" {
                          }
                          frame "T-RISE TEST" {
                          }
                        }
                        n767 = Unbundle(w1265) -> ("DESCRIPTION"=w1264:string)  [unwired: 4 out]
                        n768 = Concatenate Strings(w1260, "\\", w1258, w1257, w1256, w1257) -> (w1267:string)
                        n769 = String To Path(string=w1267) -> (path=w1269:path)
                        n770 = Concatenate Strings(w1267, w1266, w1264, "-", w1263, ".tdms") -> (w1255:string)
                        n771 = Create Folder(path (use dialog)=w1269) -> (error out=w1268:errorcluster)  [unwired: 2 in, 2 out]
                        n772 = global write "Global 1.vi" "LAB04-2 FILE"(w1255) -> ()
                        n773 = call <vilib>:"Clear Errors.vi"("error in (no error)"=w1268) -> ()  [unwired: 6 in, 1 out]
                      }
                      frame #1 {
                        n774 = String To Path(string=w1280) -> (path=w1275:path)
                        n775 = TDMS Open(5:FALSE, 6:FALSE, 10:T19."create or replace" ("operation (0:open)"), 11:w1275) -> (0:w1274:errorcluster, 3:→"TDMS LAB04-2":refnum<k34>)  [unwired: 3 in]
                      }
                      frame #2 {
                        n776 = local read "SET LAB04-2"() -> (w1286:T5)
                        n777 = local read "TDMS LAB04-2"() -> (w1297:refnum<k34>)
                        n778 = Build Array("Testers Name", "Description", "Set Test Cycles", "T-Rise minutes", "T-Rise Deg C") -> (w1287:string[])
                        n779 = Unbundle(w1286) -> ("NAME"=w1285:string, "DESCRIPTION"=w1284:string, "CYCLES"=w1283:dbl, "T-RISE mins"=w1282:dbl, "T-RISE deg C"=w1281:dbl)
                        n780 = Number To Decimal String(number=w1283) -> (decimal integer string=w1296:string)  [unwired: 1 in]
                        n781 = Number To Decimal String(number=w1282) -> (decimal integer string=w1295:string)  [unwired: 1 in]
                        n782 = Number To Decimal String(number=w1281) -> (decimal integer string=w1294:string)  [unwired: 1 in]
                        n783 = Build Array(w1285, w1284, w1296, w1295, w1294) -> (w1293:string[])
                        n784 = TDMS Set Properties(5:w1293, 7:w1287, 11:w1297) -> ()  [unwired: 3 in, 4 out]
                      }
                      frame #3 {
                        w1299 = 0.0
                        n785 = local read "DISP LAB04-2"() -> (w1301:T4)
                        n786 = Bundle(cluster=w1301, "CYCLE"=w1299, "MINS"=w1299, "STATUS"="RUN") -> (w1300:T4)
                        n787 = local write "DISP LAB04-2"(w1300) -> ()
                      }
                      frame #4 {
                        n788 = local read "SIG LAB04-2"() -> (w1304:T2)
                        n789 = local read "TEMP START LAB04-2"() -> (w1306:cluster{"TL":dbl, "TN":dbl})
                        n790 = Unbundle(w1304) -> ("Tmp Live"=w1303:dbl, "Tmp Neut"=w1302:dbl)  [unwired: 3 out]
                        n791 = Bundle(cluster=w1306, "TL"=w1303, "TN"=w1302) -> (w1305:cluster{"TL":dbl, "TN":dbl})
                        n792 = local write "TEMP START LAB04-2"(w1305) -> ()
                      }
                    }
                  }
                }
              }
              event "RUN LAB05-1": Value Change {
                n793 = event-data() -> ("NewVal"=w1307:bool)  [unwired: 1 in, 5 out]
                n794 = local write "run lab05-1"(w1307) -> ()
                n795 = case shown="True" w1307 {
                  tunnel: w1313 -> [_ w1346]
                  tunnel: w1312 -> [_ w1345]
                  tunnel: w1310 -> [w1315 w1344]
                  tunnel: w1311 -> [_ w1343]
                  tunnel: w1309 -> [_ w1342]
                  tunnel: [w1314 w1341] -> w1308
                  frame False {
                    # "stop test"
                    n796 = stacked-sequence {
                      tunnel: w1315 -> [w1324 _]
                      tunnel: [w1316 _] -> w1314
                      frame #0 {
                        n797 = local read "DISP LAB05-1"() -> (w1323:T4)
                        n798 = Unbundle(w1323) -> ("CYCLE"=w1321:dbl, "MINS"=w1322:dbl)  [unwired: 1 out]
                        n799 = case shown="\"CYCLE TEST\"" w1324 {
                          tunnel: w1322 -> [_ _ w1331]
                          tunnel: w1321 -> [w1329 w1330 _]
                          tunnel: [w1329 w1330 w1331] -> w1320
                          frame "CHART TEST", Default {
                          }
                          frame "CYCLE TEST" {
                          }
                          frame "T-RISE TEST" {
                          }
                        }
                        n800 = local read "TDMS LAB05-1"() -> (w1328:refnum<k34>)
                        n801 = Build Array("STOPPED") -> (w1325:string[])
                        n802 = Build Array(w1320) -> (w1319:dbl[])
                        n803 = TDMS Write(0:w1328, 5:"TEST RESULT", 7:w1325, 9:w1319) -> (4:w1317:refnum<k34>, 15:w1318:errorcluster)  [unwired: 2 in, 2 out]
                        n804 = TDMS Close(8:w1318, 11:w1317) -> (0:w1316:errorcluster)  [unwired: 1 out]
                      }
                      frame #1 {
                        n805 = local read "DISP LAB05-1"() -> (w1335:T4)
                        n806 = stacked-sequence {
                          tunnel: "LAB05-1" -> [w1337 w1339]
                          frame #0 {
                            n807 = call "sub vi - defrag tdms v1.vi"("panel id"=w1337) -> ("error out"=w1336:errorcluster)  [unwired: 10 in]
                            n808 = local write "data file error"(w1336) -> ()
                          }
                          frame #1 {
                            n809 = call "Save data file to network drive v1.vi"("panel id"=w1339) -> ("network file save error"=w1338:errorcluster)  [unwired: 9 in, 1 out]
                            n810 = local write "RESULT LAB05-1"(FALSE) -> ()
                            n811 = local write "data file error"(w1338) -> ()
                          }
                        }
                        n812 = Bundle(cluster=w1335, "STATUS"="STOP") -> (w1333:T4)  [unwired: 2 in]
                        n813 = local write "DISP LAB05-1"(w1333) -> ()
                      }
                    }
                  }
                  frame True {
                    # "start new test and create test file"
                    n814 = stacked-sequence {
                      seq-local: [w1347 _ _ _ _] -> [_ w1372 _ _ _]
                      tunnel: w1346 -> [w1352 _ _ _ _]
                      tunnel: w1345 -> [w1348 _ _ _ _]
                      tunnel: w1344 -> [w1362 _ _ _ _]
                      tunnel: w1343 -> [w1355 _ _ _ _]
                      tunnel: w1342 -> [w1350 _ _ _ _]
                      tunnel: [_ w1366 _ _ _] -> w1341
                      frame #0 {
                        w1349 = "\\"
                        n815 = local read "SET LAB05-1"() -> (w1357:T5)
                        n816 = case shown="\"CYCLE TEST\"" w1362 {
                          tunnel: ["L05-1-CHART TEST-" "L05-1-CYCLE TEST-" "L05-1-T-RISE TEST-"] -> w1358
                          frame "CHART TEST", Default {
                          }
                          frame "CYCLE TEST" {
                          }
                          frame "T-RISE TEST" {
                          }
                        }
                        n817 = Unbundle(w1357) -> ("DESCRIPTION"=w1356:string)  [unwired: 4 out]
                        n818 = Concatenate Strings(w1352, "\\", w1350, w1349, w1348, w1349) -> (w1359:string)
                        n819 = String To Path(string=w1359) -> (path=w1361:path)
                        n820 = Concatenate Strings(w1359, w1358, w1356, "-", w1355, ".tdms") -> (w1347:string)
                        n821 = Create Folder(path (use dialog)=w1361) -> (error out=w1360:errorcluster)  [unwired: 2 in, 2 out]
                        n822 = global write "Global 1.vi" "LAB05-1 FILE"(w1347) -> ()
                        n823 = call <vilib>:"Clear Errors.vi"("error in (no error)"=w1360) -> ()  [unwired: 6 in, 1 out]
                      }
                      frame #1 {
                        n824 = String To Path(string=w1372) -> (path=w1367:path)
                        n825 = TDMS Open(5:FALSE, 6:FALSE, 10:T19."create or replace" ("operation (0:open)"), 11:w1367) -> (0:w1366:errorcluster, 3:→"TDMS LAB05-1":refnum<k34>)  [unwired: 3 in]
                      }
                      frame #2 {
                        n826 = local read "SET LAB05-1"() -> (w1378:T5)
                        n827 = local read "TDMS LAB05-1"() -> (w1389:refnum<k34>)
                        n828 = Build Array("Testers Name", "Description", "Set Test Cycles", "T-Rise minutes", "T-Rise Deg C") -> (w1379:string[])
                        n829 = Unbundle(w1378) -> ("NAME"=w1377:string, "DESCRIPTION"=w1376:string, "CYCLES"=w1375:dbl, "T-RISE mins"=w1374:dbl, "T-RISE deg C"=w1373:dbl)
                        n830 = Number To Decimal String(number=w1375) -> (decimal integer string=w1388:string)  [unwired: 1 in]
                        n831 = Number To Decimal String(number=w1374) -> (decimal integer string=w1387:string)  [unwired: 1 in]
                        n832 = Number To Decimal String(number=w1373) -> (decimal integer string=w1386:string)  [unwired: 1 in]
                        n833 = Build Array(w1377, w1376, w1388, w1387, w1386) -> (w1385:string[])
                        n834 = TDMS Set Properties(5:w1385, 7:w1379, 11:w1389) -> ()  [unwired: 3 in, 4 out]
                      }
                      frame #3 {
                        w1391 = 0.0
                        n835 = local read "DISP LAB05-1"() -> (w1393:T4)
                        n836 = Bundle(cluster=w1393, "CYCLE"=w1391, "MINS"=w1391, "STATUS"="RUN") -> (w1392:T4)
                        n837 = local write "DISP LAB05-1"(w1392) -> ()
                      }
                      frame #4 {
                        n838 = local read "SIG LAB05-1"() -> (w1396:T2)
                        n839 = local read "TEMP START LAB05-1"() -> (w1398:cluster{"TL":dbl, "TN":dbl})
                        n840 = Unbundle(w1396) -> ("Tmp Live"=w1395:dbl, "Tmp Neut"=w1394:dbl)  [unwired: 3 out]
                        n841 = Bundle(cluster=w1398, "TL"=w1395, "TN"=w1394) -> (w1397:cluster{"TL":dbl, "TN":dbl})
                        n842 = local write "TEMP START LAB05-1"(w1397) -> ()
                      }
                    }
                  }
                }
              }
              event "RUN LAB05-2": Value Change {
                n843 = event-data() -> ("NewVal"=w1399:bool)  [unwired: 1 in, 5 out]
                n844 = local write "run lab05-2"(w1399) -> ()
                n845 = case shown="True" w1399 {
                  tunnel: w1405 -> [_ w1438]
                  tunnel: w1404 -> [_ w1437]
                  tunnel: w1402 -> [w1407 w1436]
                  tunnel: w1403 -> [_ w1435]
                  tunnel: w1401 -> [_ w1434]
                  tunnel: [w1406 w1433] -> w1400
                  frame False {
                    # "stop test"
                    n846 = stacked-sequence {
                      tunnel: w1407 -> [w1416 _]
                      tunnel: [w1408 _] -> w1406
                      frame #0 {
                        n847 = local read "DISP LAB05-2"() -> (w1415:T4)
                        n848 = Unbundle(w1415) -> ("CYCLE"=w1413:dbl, "MINS"=w1414:dbl)  [unwired: 1 out]
                        n849 = case shown="\"CYCLE TEST\"" w1416 {
                          tunnel: w1414 -> [_ _ w1423]
                          tunnel: w1413 -> [w1421 w1422 _]
                          tunnel: [w1421 w1422 w1423] -> w1412
                          frame "CHART TEST", Default {
                          }
                          frame "CYCLE TEST" {
                          }
                          frame "T-RISE TEST" {
                          }
                        }
                        n850 = local read "TDMS LAB05-2"() -> (w1420:refnum<k34>)
                        n851 = Build Array("STOPPED") -> (w1417:string[])
                        n852 = Build Array(w1412) -> (w1411:dbl[])
                        n853 = TDMS Write(0:w1420, 5:"TEST RESULT", 7:w1417, 9:w1411) -> (4:w1409:refnum<k34>, 15:w1410:errorcluster)  [unwired: 2 in, 2 out]
                        n854 = TDMS Close(8:w1410, 11:w1409) -> (0:w1408:errorcluster)  [unwired: 1 out]
                      }
                      frame #1 {
                        n855 = local read "DISP LAB05-2"() -> (w1427:T4)
                        n856 = stacked-sequence {
                          tunnel: "LAB05-2" -> [w1429 w1431]
                          frame #0 {
                            n857 = call "sub vi - defrag tdms v1.vi"("panel id"=w1429) -> ("error out"=w1428:errorcluster)  [unwired: 10 in]
                            n858 = local write "data file error"(w1428) -> ()
                          }
                          frame #1 {
                            n859 = local write "RESULT LAB05-2"(FALSE) -> ()
                            n860 = call "Save data file to network drive v1.vi"("panel id"=w1431) -> ("network file save error"=w1430:errorcluster)  [unwired: 9 in, 1 out]
                            n861 = local write "data file error"(w1430) -> ()
                          }
                        }
                        n862 = Bundle(cluster=w1427, "STATUS"="STOP") -> (w1425:T4)  [unwired: 2 in]
                        n863 = local write "DISP LAB05-2"(w1425) -> ()
                      }
                    }
                  }
                  frame True {
                    # "start new test and create test file"
                    n864 = stacked-sequence {
                      seq-local: [w1439 _ _ _ _] -> [_ w1464 _ _ _]
                      tunnel: w1438 -> [w1444 _ _ _ _]
                      tunnel: w1437 -> [w1440 _ _ _ _]
                      tunnel: w1436 -> [w1454 _ _ _ _]
                      tunnel: w1435 -> [w1447 _ _ _ _]
                      tunnel: w1434 -> [w1442 _ _ _ _]
                      tunnel: [_ w1458 _ _ _] -> w1433
                      frame #0 {
                        w1441 = "\\"
                        n865 = local read "SET LAB05-2"() -> (w1449:T5)
                        n866 = case shown="\"CYCLE TEST\"" w1454 {
                          tunnel: ["L05-2-CHART TEST-" "L05-2-CYCLE TEST-" "L05-2-T-RISE TEST-"] -> w1450
                          frame "CHART TEST", Default {
                          }
                          frame "CYCLE TEST" {
                          }
                          frame "T-RISE TEST" {
                          }
                        }
                        n867 = Unbundle(w1449) -> ("DESCRIPTION"=w1448:string)  [unwired: 4 out]
                        n868 = Concatenate Strings(w1444, "\\", w1442, w1441, w1440, w1441) -> (w1451:string)
                        n869 = String To Path(string=w1451) -> (path=w1453:path)
                        n870 = Concatenate Strings(w1451, w1450, w1448, "-", w1447, ".tdms") -> (w1439:string)
                        n871 = Create Folder(path (use dialog)=w1453) -> (error out=w1452:errorcluster)  [unwired: 2 in, 2 out]
                        n872 = global write "Global 1.vi" "LAB05-2 FILE"(w1439) -> ()
                        n873 = call <vilib>:"Clear Errors.vi"("error in (no error)"=w1452) -> ()  [unwired: 6 in, 1 out]
                      }
                      frame #1 {
                        n874 = String To Path(string=w1464) -> (path=w1459:path)
                        n875 = TDMS Open(5:FALSE, 6:FALSE, 10:T19."create or replace" ("operation (0:open)"), 11:w1459) -> (0:w1458:errorcluster, 3:→"TDMS LAB05-2":refnum<k34>)  [unwired: 3 in]
                      }
                      frame #2 {
                        n876 = local read "SET LAB05-2"() -> (w1470:T5)
                        n877 = local read "TDMS LAB05-2"() -> (w1481:refnum<k34>)
                        n878 = Build Array("Testers Name", "Description", "Set Test Cycles", "T-Rise minutes", "T-Rise Deg C") -> (w1471:string[])
                        n879 = Unbundle(w1470) -> ("NAME"=w1469:string, "DESCRIPTION"=w1468:string, "CYCLES"=w1467:dbl, "T-RISE mins"=w1466:dbl, "T-RISE deg C"=w1465:dbl)
                        n880 = Number To Decimal String(number=w1467) -> (decimal integer string=w1480:string)  [unwired: 1 in]
                        n881 = Number To Decimal String(number=w1466) -> (decimal integer string=w1479:string)  [unwired: 1 in]
                        n882 = Number To Decimal String(number=w1465) -> (decimal integer string=w1478:string)  [unwired: 1 in]
                        n883 = Build Array(w1469, w1468, w1480, w1479, w1478) -> (w1477:string[])
                        n884 = TDMS Set Properties(5:w1477, 7:w1471, 11:w1481) -> ()  [unwired: 3 in, 4 out]
                      }
                      frame #3 {
                        w1483 = 0.0
                        n885 = local read "DISP LAB05-2"() -> (w1485:T4)
                        n886 = Bundle(cluster=w1485, "CYCLE"=w1483, "MINS"=w1483, "STATUS"="RUN") -> (w1484:T4)
                        n887 = local write "DISP LAB05-2"(w1484) -> ()
                      }
                      frame #4 {
                        n888 = local read "SIG LAB05-2"() -> (w1488:T2)
                        n889 = local read "TEMP START LAB05-2"() -> (w1490:cluster{"TL":dbl, "TN":dbl})
                        n890 = Unbundle(w1488) -> ("Tmp Live"=w1487:dbl, "Tmp Neut"=w1486:dbl)  [unwired: 3 out]
                        n891 = Bundle(cluster=w1490, "TL"=w1487, "TN"=w1486) -> (w1489:cluster{"TL":dbl, "TN":dbl})
                        n892 = local write "TEMP START LAB05-2"(w1489) -> ()
                      }
                    }
                  }
                }
              }
            }
            n893 = local write "data file error"(w542) -> ()
          }
          frame #4 {
            # "check if test cycles reached for cycle tests, if so then test pass"
            n894 = stacked-sequence {
              tunnel: w1510 -> [_ _ _ _ _ _ _ _ _ _]
              tunnel: w1509 -> [_ _ _ _ _ _ _ _ _ _]
              tunnel: w1508 -> [_ _ _ _ _ _ _ _ _ _]
              tunnel: w1507 -> [_ _ _ _ _ _ _ _ _ _]
              tunnel: w1506 -> [_ _ _ _ _ _ _ _ _ _]
              tunnel: w1505 -> [_ _ _ _ _ _ _ _ _ _]
              tunnel: w1504 -> [_ _ _ _ _ _ _ _ _ _]
              tunnel: w1503 -> [_ _ _ _ _ _ _ _ _ _]
              tunnel: w1502 -> [_ _ _ _ _ _ _ _ _ _]
              tunnel: w1501 -> [_ _ _ _ _ _ _ _ _ _]
              tunnel: w1500 -> [w1516 _ _ _ _ _ _ _ _ _]
              tunnel: w1499 -> [_ w1551 _ _ _ _ _ _ _ _]
              tunnel: w1498 -> [_ _ w1591 _ _ _ _ _ _ _]
              tunnel: w1497 -> [_ _ _ w1631 _ _ _ _ _ _]
              tunnel: w1496 -> [_ _ _ _ w1671 _ _ _ _ _]
              tunnel: w1495 -> [_ _ _ _ _ w1711 _ _ _ _]
              tunnel: w1494 -> [_ _ _ _ _ _ w1751 _ _ _]
              tunnel: w1493 -> [_ _ _ _ _ _ _ w1791 _ _]
              tunnel: w1492 -> [_ _ _ _ _ _ _ _ w1831 _]
              tunnel: w1491 -> [_ _ _ _ _ _ _ _ _ w1871]
              frame #0 {
                # "LAB01-1"
                n895 = Less?(x=w1516, y=2) -> (x < y?=w1514:bool)
                n896 = local read "DISP LAB01-1"() -> (w1517:T4)
                n897 = Unbundle(w1517) -> ("STATUS"=w1511:string)  [unwired: 2 out]
                n898 = Equal?(x=w1511, y="RUN") -> (x = y?=w1513:bool)
                n899 = And(x=w1513, y=w1514) -> (x .and. y?=w1512:bool)
                n900 = case shown="True" w1512 {
                  tunnel: w1517 -> [_ w1522]
                  tunnel: w1516 -> [_ w1526]
                  frame False {
                  }
                  frame True {
                    n901 = local read "SET LAB01-1"() -> (w1528:T5)
                    n902 = local read "TDMS LAB01-1"() -> (w1521:refnum<k34>)
                    n903 = Unbundle(w1528) -> ("CYCLES"=w1519:dbl, "T-RISE mins"=w1525:dbl)  [unwired: 3 out]
                    n904 = case shown="\"CYCLE TEST\"" w1526 {
                      tunnel: w1525 -> [_ _ w1535]
                      tunnel: [w1530 w1532 w1535] -> w1524
                      tunnel: w1519 -> [w1530 w1532 _]
                      tunnel: ["CHART PASS" "CYCLE PASS" "T-RISE PASS"] -> w1523
                      frame "CHART TEST", Default {
                      }
                      frame "CYCLE TEST" {
                      }
                      frame "T-RISE TEST" {
                      }
                    }
                    n905 = Unbundle(w1522) -> ("CYCLE"=w1527:dbl)  [unwired: 2 out]
                    n906 = Increment(x=w1519) -> (x+1=w1520:dbl)
                    n907 = Greater Or Equal?(x=w1527, y=w1520) -> (x >= y?=w1529:bool)
                    n908 = case shown="True" w1529 {
                      tunnel: w1524 -> [w1539 _]
                      tunnel: w1523 -> [w1538 _]
                      tunnel: w1522 -> [w1537 _]
                      tunnel: w1521 -> [w1536 _]
                      frame True {
                        n909 = stacked-sequence {
                          tunnel: w1539 -> [w1543 _]
                          tunnel: w1538 -> [w1541 w1547]
                          tunnel: w1537 -> [_ w1550]
                          tunnel: w1536 -> [w1540 _]
                          frame #0 {
                            n910 = Build Array(w1541) -> (w1544:string[])
                            n911 = Build Array(w1543) -> (w1542:dbl[])
                            n912 = TDMS Write(0:w1540, 5:"TEST PASS", 7:w1544, 9:w1542) -> (15:w1546:errorcluster)  [unwired: 2 in, 3 out]
                            n913 = local write "data file error"(w1546) -> ()
                          }
                          frame #1 {
                            n914 = Bundle(cluster=w1550, "STATUS"=w1547) -> (w1548:T4)  [unwired: 2 in]
                            n915 = local write "RESULT LAB01-1"(TRUE) -> ()
                            n916 = local write "DISP LAB01-1"(w1548) -> ()
                          }
                        }
                      }
                      frame False {
                      }
                    }
                  }
                }
              }
              frame #1 {
                # "LAB01-2"
                n917 = Less?(x=w1551, y=2) -> (x < y?=w1554:bool)
                n918 = local read "DISP LAB01-2"() -> (w1556:T4)
                n919 = Unbundle(w1556) -> ("STATUS"=w1557:string)  [unwired: 2 out]
                n920 = Equal?(x=w1557, y="RUN") -> (x = y?=w1553:bool)
                n921 = And(x=w1553, y=w1554) -> (x .and. y?=w1552:bool)
                n922 = case shown="True" w1552 {
                  tunnel: w1556 -> [_ w1562]
                  tunnel: w1551 -> [_ w1566]
                  frame False {
                  }
                  frame True {
                    n923 = local read "SET LAB01-2"() -> (w1568:T5)
                    n924 = local read "TDMS LAB01-2"() -> (w1561:refnum<k34>)
                    n925 = Unbundle(w1568) -> ("CYCLES"=w1559:dbl, "T-RISE mins"=w1565:dbl)  [unwired: 3 out]
                    n926 = case shown="\"T-RISE TEST\"" w1566 {
                      tunnel: w1565 -> [_ _ w1575]
                      tunnel: [w1570 w1572 w1575] -> w1564
                      tunnel: w1559 -> [w1570 w1572 _]
                      tunnel: ["CHART PASS" "CYCLE PASS" "T-RISE PASS"] -> w1563
                      frame "CHART TEST", Default {
                      }
                      frame "CYCLE TEST" {
                      }
                      frame "T-RISE TEST" {
                      }
                    }
                    n927 = Unbundle(w1562) -> ("CYCLE"=w1567:dbl)  [unwired: 2 out]
                    n928 = Increment(x=w1559) -> (x+1=w1560:dbl)
                    n929 = Greater Or Equal?(x=w1567, y=w1560) -> (x >= y?=w1569:bool)
                    n930 = case shown="True" w1569 {
                      tunnel: w1564 -> [w1579 _]
                      tunnel: w1563 -> [w1578 _]
                      tunnel: w1562 -> [w1577 _]
                      tunnel: w1561 -> [w1576 _]
                      frame True {
                        n931 = stacked-sequence {
                          tunnel: w1579 -> [w1583 _]
                          tunnel: w1578 -> [w1581 w1587]
                          tunnel: w1577 -> [_ w1590]
                          tunnel: w1576 -> [w1580 _]
                          frame #0 {
                            n932 = Build Array(w1581) -> (w1584:string[])
                            n933 = Build Array(w1583) -> (w1582:dbl[])
                            n934 = TDMS Write(0:w1580, 5:"TEST PASS", 7:w1584, 9:w1582) -> (15:w1586:errorcluster)  [unwired: 2 in, 3 out]
                            n935 = local write "data file error"(w1586) -> ()
                          }
                          frame #1 {
                            n936 = Bundle(cluster=w1590, "STATUS"=w1587) -> (w1588:T4)  [unwired: 2 in]
                            n937 = local write "RESULT LAB01-2"(TRUE) -> ()
                            n938 = local write "DISP LAB01-2"(w1588) -> ()
                          }
                        }
                      }
                      frame False {
                      }
                    }
                  }
                }
              }
              frame #2 {
                # "LAB02-1"
                n939 = Less?(x=w1591, y=2) -> (x < y?=w1594:bool)
                n940 = local read "DISP LAB02-1"() -> (w1596:T4)
                n941 = Unbundle(w1596) -> ("STATUS"=w1597:string)  [unwired: 2 out]
                n942 = Equal?(x=w1597, y="RUN") -> (x = y?=w1593:bool)
                n943 = And(x=w1593, y=w1594) -> (x .and. y?=w1592:bool)
                n944 = case shown="True" w1592 {
                  tunnel: w1596 -> [_ w1602]
                  tunnel: w1591 -> [_ w1606]
                  frame False {
                  }
                  frame True {
                    n945 = local read "SET LAB02-1"() -> (w1608:T5)
                    n946 = local read "TDMS LAB02-1"() -> (w1601:refnum<k34>)
                    n947 = Unbundle(w1602) -> ("CYCLE"=w1607:dbl)  [unwired: 2 out]
                    n948 = Unbundle(w1608) -> ("CYCLES"=w1599:dbl, "T-RISE mins"=w1605:dbl)  [unwired: 3 out]
                    n949 = case shown="\"T-RISE TEST\"" w1606 {
                      tunnel: w1605 -> [_ _ w1615]
                      tunnel: [w1610 w1612 w1615] -> w1604
                      tunnel: w1599 -> [w1610 w1612 _]
                      tunnel: ["CHART PASS" "CYCLE PASS" "T-RISE PASS"] -> w1603
                      frame "CHART TEST", Default {
                      }
                      frame "CYCLE TEST" {
                      }
                      frame "T-RISE TEST" {
                      }
                    }
                    n950 = Increment(x=w1599) -> (x+1=w1600:dbl)
                    n951 = Greater Or Equal?(x=w1607, y=w1600) -> (x >= y?=w1609:bool)
                    n952 = case shown="True" w1609 {
                      tunnel: w1604 -> [w1619 _]
                      tunnel: w1603 -> [w1618 _]
                      tunnel: w1602 -> [w1617 _]
                      tunnel: w1601 -> [w1616 _]
                      frame True {
                        n953 = stacked-sequence {
                          tunnel: w1619 -> [w1623 _]
                          tunnel: w1618 -> [w1621 w1627]
                          tunnel: w1617 -> [_ w1630]
                          tunnel: w1616 -> [w1620 _]
                          frame #0 {
                            n954 = Build Array(w1621) -> (w1624:string[])
                            n955 = Build Array(w1623) -> (w1622:dbl[])
                            n956 = TDMS Write(0:w1620, 5:"TEST PASS", 7:w1624, 9:w1622) -> (15:w1626:errorcluster)  [unwired: 2 in, 3 out]
                            n957 = local write "data file error"(w1626) -> ()
                          }
                          frame #1 {
                            n958 = Bundle(cluster=w1630, "STATUS"=w1627) -> (w1628:T4)  [unwired: 2 in]
                            n959 = local write "RESULT LAB02-1"(TRUE) -> ()
                            n960 = local write "DISP LAB02-1"(w1628) -> ()
                          }
                        }
                      }
                      frame False {
                      }
                    }
                  }
                }
              }
              frame #3 {
                # "LAB02-2"
                n961 = Less?(x=w1631, y=2) -> (x < y?=w1634:bool)
                n962 = local read "DISP LAB02-2"() -> (w1636:T4)
                n963 = Unbundle(w1636) -> ("STATUS"=w1637:string)  [unwired: 2 out]
                n964 = Equal?(x=w1637, y="RUN") -> (x = y?=w1633:bool)
                n965 = And(x=w1633, y=w1634) -> (x .and. y?=w1632:bool)
                n966 = case shown="True" w1632 {
                  tunnel: w1636 -> [_ w1642]
                  tunnel: w1631 -> [_ w1646]
                  frame False {
                  }
                  frame True {
                    n967 = local read "SET LAB02-2"() -> (w1648:T5)
                    n968 = local read "TDMS LAB02-2"() -> (w1641:refnum<k34>)
                    n969 = Unbundle(w1642) -> ("CYCLE"=w1647:dbl)  [unwired: 2 out]
                    n970 = Unbundle(w1648) -> ("CYCLES"=w1639:dbl, "T-RISE mins"=w1645:dbl)  [unwired: 3 out]
                    n971 = case shown="\"T-RISE TEST\"" w1646 {
                      tunnel: w1645 -> [_ _ w1655]
                      tunnel: [w1650 w1652 w1655] -> w1644
                      tunnel: w1639 -> [w1650 w1652 _]
                      tunnel: ["CHART PASS" "CYCLE PASS" "T-RISE PASS"] -> w1643
                      frame "CHART TEST", Default {
                      }
                      frame "CYCLE TEST" {
                      }
                      frame "T-RISE TEST" {
                      }
                    }
                    n972 = Increment(x=w1639) -> (x+1=w1640:dbl)
                    n973 = Greater Or Equal?(x=w1647, y=w1640) -> (x >= y?=w1649:bool)
                    n974 = case shown="True" w1649 {
                      tunnel: w1644 -> [w1659 _]
                      tunnel: w1643 -> [w1658 _]
                      tunnel: w1642 -> [w1657 _]
                      tunnel: w1641 -> [w1656 _]
                      frame True {
                        n975 = stacked-sequence {
                          tunnel: w1659 -> [w1663 _]
                          tunnel: w1658 -> [w1661 w1667]
                          tunnel: w1657 -> [_ w1670]
                          tunnel: w1656 -> [w1660 _]
                          frame #0 {
                            n976 = Build Array(w1661) -> (w1664:string[])
                            n977 = Build Array(w1663) -> (w1662:dbl[])
                            n978 = TDMS Write(0:w1660, 5:"TEST PASS", 7:w1664, 9:w1662) -> (15:w1666:errorcluster)  [unwired: 2 in, 3 out]
                            n979 = local write "data file error"(w1666) -> ()
                          }
                          frame #1 {
                            n980 = Bundle(cluster=w1670, "STATUS"=w1667) -> (w1668:T4)  [unwired: 2 in]
                            n981 = local write "RESULT LAB02-2"(TRUE) -> ()
                            n982 = local write "DISP LAB02-2"(w1668) -> ()
                          }
                        }
                      }
                      frame False {
                      }
                    }
                  }
                }
              }
              frame #4 {
                # "LAB03-1"
                n983 = Less?(x=w1671, y=2) -> (x < y?=w1674:bool)
                n984 = local read "DISP LAB03-1"() -> (w1676:T4)
                n985 = Unbundle(w1676) -> ("STATUS"=w1677:string)  [unwired: 2 out]
                n986 = Equal?(x=w1677, y="RUN") -> (x = y?=w1673:bool)
                n987 = And(x=w1673, y=w1674) -> (x .and. y?=w1672:bool)
                n988 = case shown="True" w1672 {
                  tunnel: w1676 -> [_ w1682]
                  tunnel: w1671 -> [_ w1686]
                  frame False {
                  }
                  frame True {
                    n989 = local read "SET LAB03-1"() -> (w1688:T5)
                    n990 = local read "TDMS LAB03-1"() -> (w1681:refnum<k34>)
                    n991 = Unbundle(w1682) -> ("CYCLE"=w1687:dbl)  [unwired: 2 out]
                    n992 = Unbundle(w1688) -> ("CYCLES"=w1679:dbl, "T-RISE mins"=w1685:dbl)  [unwired: 3 out]
                    n993 = case shown="\"T-RISE TEST\"" w1686 {
                      tunnel: w1685 -> [_ _ w1695]
                      tunnel: [w1690 w1692 w1695] -> w1684
                      tunnel: w1679 -> [w1690 w1692 _]
                      tunnel: ["CHART PASS" "CYCLE PASS" "T-RISE PASS"] -> w1683
                      frame "CHART TEST", Default {
                      }
                      frame "CYCLE TEST" {
                      }
                      frame "T-RISE TEST" {
                      }
                    }
                    n994 = Increment(x=w1679) -> (x+1=w1680:dbl)
                    n995 = Greater Or Equal?(x=w1687, y=w1680) -> (x >= y?=w1689:bool)
                    n996 = case shown="True" w1689 {
                      tunnel: w1684 -> [w1699 _]
                      tunnel: w1683 -> [w1698 _]
                      tunnel: w1682 -> [w1697 _]
                      tunnel: w1681 -> [w1696 _]
                      frame True {
                        n997 = stacked-sequence {
                          tunnel: w1699 -> [w1703 _]
                          tunnel: w1698 -> [w1701 w1707]
                          tunnel: w1697 -> [_ w1710]
                          tunnel: w1696 -> [w1700 _]
                          frame #0 {
                            n998 = Build Array(w1701) -> (w1704:string[])
                            n999 = Build Array(w1703) -> (w1702:dbl[])
                            n1000 = TDMS Write(0:w1700, 5:"TEST PASS", 7:w1704, 9:w1702) -> (15:w1706:errorcluster)  [unwired: 2 in, 3 out]
                            n1001 = local write "data file error"(w1706) -> ()
                          }
                          frame #1 {
                            n1002 = Bundle(cluster=w1710, "STATUS"=w1707) -> (w1708:T4)  [unwired: 2 in]
                            n1003 = local write "RESULT LAB03-1"(TRUE) -> ()
                            n1004 = local write "DISP LAB03-1"(w1708) -> ()
                          }
                        }
                      }
                      frame False {
                      }
                    }
                  }
                }
              }
              frame #5 {
                # "LAB03-2"
                n1005 = Less?(x=w1711, y=2) -> (x < y?=w1714:bool)
                n1006 = local read "DISP LAB03-2"() -> (w1716:T4)
                n1007 = Unbundle(w1716) -> ("STATUS"=w1717:string)  [unwired: 2 out]
                n1008 = Equal?(x=w1717, y="RUN") -> (x = y?=w1713:bool)
                n1009 = And(x=w1713, y=w1714) -> (x .and. y?=w1712:bool)
                n1010 = case shown="True" w1712 {
                  tunnel: w1716 -> [_ w1722]
                  tunnel: w1711 -> [_ w1726]
                  frame False {
                  }
                  frame True {
                    n1011 = local read "SET LAB03-2"() -> (w1728:T5)
                    n1012 = local read "TDMS LAB03-2"() -> (w1721:refnum<k34>)
                    n1013 = Unbundle(w1722) -> ("CYCLE"=w1727:dbl)  [unwired: 2 out]
                    n1014 = Unbundle(w1728) -> ("CYCLES"=w1719:dbl, "T-RISE mins"=w1725:dbl)  [unwired: 3 out]
                    n1015 = case shown="\"T-RISE TEST\"" w1726 {
                      tunnel: w1725 -> [_ _ w1735]
                      tunnel: [w1730 w1732 w1735] -> w1724
                      tunnel: w1719 -> [w1730 w1732 _]
                      tunnel: ["CHART PASS" "CYCLE PASS" "T-RISE PASS"] -> w1723
                      frame "CHART TEST", Default {
                      }
                      frame "CYCLE TEST" {
                      }
                      frame "T-RISE TEST" {
                      }
                    }
                    n1016 = Increment(x=w1719) -> (x+1=w1720:dbl)
                    n1017 = Greater Or Equal?(x=w1727, y=w1720) -> (x >= y?=w1729:bool)
                    n1018 = case shown="True" w1729 {
                      tunnel: w1724 -> [w1739 _]
                      tunnel: w1723 -> [w1738 _]
                      tunnel: w1722 -> [w1737 _]
                      tunnel: w1721 -> [w1736 _]
                      frame True {
                        n1019 = stacked-sequence {
                          tunnel: w1739 -> [w1743 _]
                          tunnel: w1738 -> [w1741 w1747]
                          tunnel: w1737 -> [_ w1750]
                          tunnel: w1736 -> [w1740 _]
                          frame #0 {
                            n1020 = Build Array(w1741) -> (w1744:string[])
                            n1021 = Build Array(w1743) -> (w1742:dbl[])
                            n1022 = TDMS Write(0:w1740, 5:"TEST PASS", 7:w1744, 9:w1742) -> (15:w1746:errorcluster)  [unwired: 2 in, 3 out]
                            n1023 = local write "data file error"(w1746) -> ()
                          }
                          frame #1 {
                            n1024 = Bundle(cluster=w1750, "STATUS"=w1747) -> (w1748:T4)  [unwired: 2 in]
                            n1025 = local write "RESULT LAB03-2"(TRUE) -> ()
                            n1026 = local write "DISP LAB03-2"(w1748) -> ()
                          }
                        }
                      }
                      frame False {
                      }
                    }
                  }
                }
              }
              frame #6 {
                # "LAB04-1"
                n1027 = Less?(x=w1751, y=2) -> (x < y?=w1754:bool)
                n1028 = local read "DISP LAB04-1"() -> (w1756:T4)
                n1029 = Unbundle(w1756) -> ("STATUS"=w1757:string)  [unwired: 2 out]
                n1030 = Equal?(x=w1757, y="RUN") -> (x = y?=w1753:bool)
                n1031 = And(x=w1753, y=w1754) -> (x .and. y?=w1752:bool)
                n1032 = case shown="True" w1752 {
                  tunnel: w1756 -> [_ w1762]
                  tunnel: w1751 -> [_ w1766]
                  frame False {
                  }
                  frame True {
                    n1033 = local read "SET LAB04-1"() -> (w1768:T5)
                    n1034 = local read "TDMS LAB04-1"() -> (w1761:refnum<k34>)
                    n1035 = Unbundle(w1762) -> ("CYCLE"=w1767:dbl)  [unwired: 2 out]
                    n1036 = Unbundle(w1768) -> ("CYCLES"=w1759:dbl, "T-RISE mins"=w1765:dbl)  [unwired: 3 out]
                    n1037 = case shown="\"T-RISE TEST\"" w1766 {
                      tunnel: w1765 -> [_ _ w1775]
                      tunnel: [w1770 w1772 w1775] -> w1764
                      tunnel: w1759 -> [w1770 w1772 _]
                      tunnel: ["CHART PASS" "CYCLE PASS" "T-RISE PASS"] -> w1763
                      frame "CHART TEST", Default {
                      }
                      frame "CYCLE TEST" {
                      }
                      frame "T-RISE TEST" {
                      }
                    }
                    n1038 = Increment(x=w1759) -> (x+1=w1760:dbl)
                    n1039 = Greater Or Equal?(x=w1767, y=w1760) -> (x >= y?=w1769:bool)
                    n1040 = case shown="True" w1769 {
                      tunnel: w1764 -> [w1779 _]
                      tunnel: w1763 -> [w1778 _]
                      tunnel: w1762 -> [w1777 _]
                      tunnel: w1761 -> [w1776 _]
                      frame True {
                        n1041 = stacked-sequence {
                          tunnel: w1779 -> [w1783 _]
                          tunnel: w1778 -> [w1781 w1787]
                          tunnel: w1777 -> [_ w1790]
                          tunnel: w1776 -> [w1780 _]
                          frame #0 {
                            n1042 = Build Array(w1781) -> (w1784:string[])
                            n1043 = Build Array(w1783) -> (w1782:dbl[])
                            n1044 = TDMS Write(0:w1780, 5:"TEST PASS", 7:w1784, 9:w1782) -> (15:w1786:errorcluster)  [unwired: 2 in, 3 out]
                            n1045 = local write "data file error"(w1786) -> ()
                          }
                          frame #1 {
                            n1046 = Bundle(cluster=w1790, "STATUS"=w1787) -> (w1788:T4)  [unwired: 2 in]
                            n1047 = local write "RESULT LAB04-1"(TRUE) -> ()
                            n1048 = local write "DISP LAB04-1"(w1788) -> ()
                          }
                        }
                      }
                      frame False {
                      }
                    }
                  }
                }
              }
              frame #7 {
                # "LAB04-2"
                n1049 = Less?(x=w1791, y=2) -> (x < y?=w1794:bool)
                n1050 = local read "DISP LAB04-2"() -> (w1796:T4)
                n1051 = Unbundle(w1796) -> ("STATUS"=w1797:string)  [unwired: 2 out]
                n1052 = Equal?(x=w1797, y="RUN") -> (x = y?=w1793:bool)
                n1053 = And(x=w1793, y=w1794) -> (x .and. y?=w1792:bool)
                n1054 = case shown="True" w1792 {
                  tunnel: w1796 -> [_ w1802]
                  tunnel: w1791 -> [_ w1806]
                  frame False {
                  }
                  frame True {
                    n1055 = local read "SET LAB04-2"() -> (w1808:T5)
                    n1056 = local read "TDMS LAB04-2"() -> (w1801:refnum<k34>)
                    n1057 = Unbundle(w1802) -> ("CYCLE"=w1807:dbl)  [unwired: 2 out]
                    n1058 = Unbundle(w1808) -> ("CYCLES"=w1799:dbl, "T-RISE mins"=w1805:dbl)  [unwired: 3 out]
                    n1059 = case shown="\"T-RISE TEST\"" w1806 {
                      tunnel: w1805 -> [_ _ w1815]
                      tunnel: [w1810 w1812 w1815] -> w1804
                      tunnel: w1799 -> [w1810 w1812 _]
                      tunnel: ["CHART PASS" "CYCLE PASS" "T-RISE PASS"] -> w1803
                      frame "CHART TEST", Default {
                      }
                      frame "CYCLE TEST" {
                      }
                      frame "T-RISE TEST" {
                      }
                    }
                    n1060 = Increment(x=w1799) -> (x+1=w1800:dbl)
                    n1061 = Greater Or Equal?(x=w1807, y=w1800) -> (x >= y?=w1809:bool)
                    n1062 = case shown="True" w1809 {
                      tunnel: w1804 -> [w1819 _]
                      tunnel: w1803 -> [w1818 _]
                      tunnel: w1802 -> [w1817 _]
                      tunnel: w1801 -> [w1816 _]
                      frame True {
                        n1063 = stacked-sequence {
                          tunnel: w1819 -> [w1823 _]
                          tunnel: w1818 -> [w1821 w1827]
                          tunnel: w1817 -> [_ w1830]
                          tunnel: w1816 -> [w1820 _]
                          frame #0 {
                            n1064 = Build Array(w1821) -> (w1824:string[])
                            n1065 = Build Array(w1823) -> (w1822:dbl[])
                            n1066 = TDMS Write(0:w1820, 5:"TEST PASS", 7:w1824, 9:w1822) -> (15:w1826:errorcluster)  [unwired: 2 in, 3 out]
                            n1067 = local write "data file error"(w1826) -> ()
                          }
                          frame #1 {
                            n1068 = Bundle(cluster=w1830, "STATUS"=w1827) -> (w1828:T4)  [unwired: 2 in]
                            n1069 = local write "RESULT LAB04-2"(TRUE) -> ()
                            n1070 = local write "DISP LAB04-2"(w1828) -> ()
                          }
                        }
                      }
                      frame False {
                      }
                    }
                  }
                }
              }
              frame #8 {
                # "LAB05-1"
                n1071 = Less?(x=w1831, y=2) -> (x < y?=w1834:bool)
                n1072 = local read "DISP LAB05-1"() -> (w1836:T4)
                n1073 = Unbundle(w1836) -> ("STATUS"=w1837:string)  [unwired: 2 out]
                n1074 = Equal?(x=w1837, y="RUN") -> (x = y?=w1833:bool)
                n1075 = And(x=w1833, y=w1834) -> (x .and. y?=w1832:bool)
                n1076 = case shown="True" w1832 {
                  tunnel: w1836 -> [_ w1842]
                  tunnel: w1831 -> [_ w1846]
                  frame False {
                  }
                  frame True {
                    n1077 = local read "SET LAB05-1"() -> (w1848:T5)
                    n1078 = local read "TDMS LAB05-1"() -> (w1841:refnum<k34>)
                    n1079 = Unbundle(w1842) -> ("CYCLE"=w1847:dbl)  [unwired: 2 out]
                    n1080 = Unbundle(w1848) -> ("CYCLES"=w1839:dbl, "T-RISE mins"=w1845:dbl)  [unwired: 3 out]
                    n1081 = case shown="\"T-RISE TEST\"" w1846 {
                      tunnel: w1845 -> [_ _ w1855]
                      tunnel: [w1850 w1852 w1855] -> w1844
                      tunnel: w1839 -> [w1850 w1852 _]
                      tunnel: ["CHART PASS" "CYCLE PASS" "T-RISE PASS"] -> w1843
                      frame "CHART TEST", Default {
                      }
                      frame "CYCLE TEST" {
                      }
                      frame "T-RISE TEST" {
                      }
                    }
                    n1082 = Increment(x=w1839) -> (x+1=w1840:dbl)
                    n1083 = Greater Or Equal?(x=w1847, y=w1840) -> (x >= y?=w1849:bool)
                    n1084 = case shown="True" w1849 {
                      tunnel: w1844 -> [w1859 _]
                      tunnel: w1843 -> [w1858 _]
                      tunnel: w1842 -> [w1857 _]
                      tunnel: w1841 -> [w1856 _]
                      frame True {
                        n1085 = stacked-sequence {
                          tunnel: w1859 -> [w1863 _]
                          tunnel: w1858 -> [w1861 w1867]
                          tunnel: w1857 -> [_ w1870]
                          tunnel: w1856 -> [w1860 _]
                          frame #0 {
                            n1086 = Build Array(w1861) -> (w1864:string[])
                            n1087 = Build Array(w1863) -> (w1862:dbl[])
                            n1088 = TDMS Write(0:w1860, 5:"TEST PASS", 7:w1864, 9:w1862) -> (15:w1866:errorcluster)  [unwired: 2 in, 3 out]
                            n1089 = local write "data file error"(w1866) -> ()
                          }
                          frame #1 {
                            n1090 = Bundle(cluster=w1870, "STATUS"=w1867) -> (w1868:T4)  [unwired: 2 in]
                            n1091 = local write "RESULT LAB05-1"(TRUE) -> ()
                            n1092 = local write "DISP LAB05-1"(w1868) -> ()
                          }
                        }
                      }
                      frame False {
                      }
                    }
                  }
                }
              }
              frame #9 {
                # "LAB05-2"
                n1093 = Less?(x=w1871, y=2) -> (x < y?=w1874:bool)
                n1094 = local read "DISP LAB05-2"() -> (w1876:T4)
                n1095 = Unbundle(w1876) -> ("STATUS"=w1877:string)  [unwired: 2 out]
                n1096 = Equal?(x=w1877, y="RUN") -> (x = y?=w1873:bool)
                n1097 = And(x=w1873, y=w1874) -> (x .and. y?=w1872:bool)
                n1098 = case shown="True" w1872 {
                  tunnel: w1876 -> [_ w1882]
                  tunnel: w1871 -> [_ w1886]
                  frame False {
                  }
                  frame True {
                    n1099 = local read "SET LAB05-2"() -> (w1888:T5)
                    n1100 = local read "TDMS LAB05-2"() -> (w1881:refnum<k34>)
                    n1101 = Unbundle(w1882) -> ("CYCLE"=w1887:dbl)  [unwired: 2 out]
                    n1102 = Unbundle(w1888) -> ("CYCLES"=w1879:dbl, "T-RISE mins"=w1885:dbl)  [unwired: 3 out]
                    n1103 = case shown="\"T-RISE TEST\"" w1886 {
                      tunnel: w1885 -> [_ _ w1895]
                      tunnel: [w1890 w1892 w1895] -> w1884
                      tunnel: w1879 -> [w1890 w1892 _]
                      tunnel: ["CHART PASS" "CYCLE PASS" "T-RISE PASS"] -> w1883
                      frame "CHART TEST", Default {
                      }
                      frame "CYCLE TEST" {
                      }
                      frame "T-RISE TEST" {
                      }
                    }
                    n1104 = Increment(x=w1879) -> (x+1=w1880:dbl)
                    n1105 = Greater Or Equal?(x=w1887, y=w1880) -> (x >= y?=w1889:bool)
                    n1106 = case shown="True" w1889 {
                      tunnel: w1884 -> [w1899 _]
                      tunnel: w1883 -> [w1898 _]
                      tunnel: w1882 -> [w1897 _]
                      tunnel: w1881 -> [w1896 _]
                      frame True {
                        n1107 = stacked-sequence {
                          tunnel: w1899 -> [w1903 _]
                          tunnel: w1898 -> [w1901 w1907]
                          tunnel: w1897 -> [_ w1910]
                          tunnel: w1896 -> [w1900 _]
                          frame #0 {
                            n1108 = Build Array(w1901) -> (w1904:string[])
                            n1109 = Build Array(w1903) -> (w1902:dbl[])
                            n1110 = TDMS Write(0:w1900, 5:"TEST PASS", 7:w1904, 9:w1902) -> (15:w1906:errorcluster)  [unwired: 2 in, 3 out]
                            n1111 = local write "data file error"(w1906) -> ()
                          }
                          frame #1 {
                            n1112 = Bundle(cluster=w1910, "STATUS"=w1907) -> (w1908:T4)  [unwired: 2 in]
                            n1113 = local write "RESULT LAB05-2"(TRUE) -> ()
                            n1114 = local write "DISP LAB05-2"(w1908) -> ()
                          }
                        }
                      }
                      frame False {
                      }
                    }
                  }
                }
              }
            }
          }
          frame #5 {
            # "check if test cycles reached for temperature rise test"
            n1115 = stacked-sequence {
              tunnel: w1940 -> [_ _ _ _ _ _ _ _ _ _]
              tunnel: w1939 -> [_ _ _ _ _ _ _ _ _ _]
              tunnel: w1938 -> [_ _ _ _ _ _ _ _ _ _]
              tunnel: w1937 -> [_ _ _ _ _ _ _ _ _ _]
              tunnel: w1936 -> [_ _ _ _ _ _ _ _ _ _]
              tunnel: w1935 -> [_ _ _ _ _ _ _ _ _ _]
              tunnel: w1934 -> [_ _ _ _ _ _ _ _ _ _]
              tunnel: w1933 -> [_ _ _ _ _ _ _ _ _ _]
              tunnel: w1932 -> [_ _ _ _ _ _ _ _ _ _]
              tunnel: w1931 -> [_ _ _ _ _ _ _ _ _ _]
              tunnel: w1930 -> [w1946 _ _ _ _ _ _ _ _ _]
              tunnel: w1920 -> [w1941 _ _ _ _ _ _ _ _ _]
              tunnel: w1929 -> [_ w1972 _ _ _ _ _ _ _ _]
              tunnel: w1928 -> [_ _ w2002 _ _ _ _ _ _ _]
              tunnel: w1927 -> [_ _ _ w2032 _ _ _ _ _ _]
              tunnel: w1926 -> [_ _ _ _ w2062 _ _ _ _ _]
              tunnel: w1925 -> [_ _ _ _ _ w2092 _ _ _ _]
              tunnel: w1924 -> [_ _ _ _ _ _ w2122 _ _ _]
              tunnel: w1923 -> [_ _ _ _ _ _ _ w2152 _ _]
              tunnel: w1922 -> [_ _ _ _ _ _ _ _ w2182 _]
              tunnel: w1921 -> [_ _ _ _ _ _ _ _ _ w2212]
              tunnel: w1919 -> [_ w1971 _ _ _ _ _ _ _ _]
              tunnel: w1918 -> [_ _ w2001 _ _ _ _ _ _ _]
              tunnel: w1917 -> [_ _ _ w2031 _ _ _ _ _ _]
              tunnel: w1916 -> [_ _ _ _ w2061 _ _ _ _ _]
              tunnel: w1915 -> [_ _ _ _ _ w2091 _ _ _ _]
              tunnel: w1914 -> [_ _ _ _ _ _ w2121 _ _ _]
              tunnel: w1913 -> [_ _ _ _ _ _ _ w2151 _ _]
              tunnel: w1912 -> [_ _ _ _ _ _ _ _ w2181 _]
              tunnel: w1911 -> [_ _ _ _ _ _ _ _ _ w2211]
              frame #0 {
                # "LAB01-1"
                n1116 = Equal?(x=w1946, y=2) -> (x = y?=w1944:bool)
                n1117 = local read "DISP LAB01-1"() -> (w1947:T4)
                n1118 = Unbundle(w1947) -> ("STATUS"=w1948:string)  [unwired: 2 out]
                n1119 = Equal?(x=w1948, y="RUN") -> (x = y?=w1943:bool)
                n1120 = And(x=w1943, y=w1944) -> (x .and. y?=w1942:bool)
                n1121 = case shown="True" w1942 {
                  tunnel: w1947 -> [_ w1951]
                  tunnel: w1941 -> [_ w1954]
                  frame False {
                  }
                  frame True {
                    n1122 = local read "SET LAB01-1"() -> (w1953:T5)
                    n1123 = local read "TDMS LAB01-1"() -> (w1950:refnum<k34>)
                    n1124 = Unbundle(w1951) -> ("CYCLE"=w1955:dbl)  [unwired: 2 out]
                    n1125 = Unbundle(w1953) -> ("T-RISE mins"=w1952:dbl)  [unwired: 4 out]
                    n1126 = Greater Or Equal?(x=w1955, y=w1954) -> (x >= y?=w1956:bool)
                    n1127 = case shown="True" w1956 {
                      tunnel: w1952 -> [w1959 _]
                      tunnel: w1951 -> [w1958 _]
                      tunnel: w1950 -> [w1957 _]
                      frame True {
                        n1128 = stacked-sequence {
                          tunnel: w1959 -> [w1962 _]
                          tunnel: w1958 -> [_ w1967]
                          tunnel: w1957 -> [w1960 _]
                          frame #0 {
                            n1129 = Build Array("T-RISE") -> (w1964:string[])
                            n1130 = Build Array(w1962) -> (w1963:dbl[])
                            n1131 = TDMS Write(0:w1960, 5:"TEST PASS", 7:w1964, 9:w1963) -> (15:w1966:errorcluster)  [unwired: 2 in, 3 out]
                            n1132 = local write "data file error"(w1966) -> ()
                          }
                          frame #1 {
                            n1133 = Bundle(cluster=w1967, "STATUS"="T-RISE PASS") -> (w1969:T4)  [unwired: 2 in]
                            n1134 = local write "RESULT LAB01-1"(TRUE) -> ()
                            n1135 = local write "DISP LAB01-1"(w1969) -> ()
                          }
                        }
                      }
                      frame False {
                      }
                    }
                  }
                }
              }
              frame #1 {
                # "LAB01-2"
                n1136 = Equal?(x=w1972, y=2) -> (x = y?=w1975:bool)
                n1137 = local read "DISP LAB01-2"() -> (w1977:T4)
                n1138 = Unbundle(w1977) -> ("STATUS"=w1978:string)  [unwired: 2 out]
                n1139 = Equal?(x=w1978, y="RUN") -> (x = y?=w1974:bool)
                n1140 = And(x=w1974, y=w1975) -> (x .and. y?=w1973:bool)
                n1141 = case shown="True" w1973 {
                  tunnel: w1977 -> [_ w1981]
                  tunnel: w1971 -> [_ w1984]
                  frame False {
                  }
                  frame True {
                    n1142 = local read "SET LAB01-2"() -> (w1983:T5)
                    n1143 = local read "TDMS LAB01-2"() -> (w1980:refnum<k34>)
                    n1144 = Unbundle(w1981) -> ("CYCLE"=w1985:dbl)  [unwired: 2 out]
                    n1145 = Unbundle(w1983) -> ("T-RISE mins"=w1982:dbl)  [unwired: 4 out]
                    n1146 = Greater Or Equal?(x=w1985, y=w1984) -> (x >= y?=w1986:bool)
                    n1147 = case shown="True" w1986 {
                      tunnel: w1982 -> [w1989 _]
                      tunnel: w1981 -> [w1988 _]
                      tunnel: w1980 -> [w1987 _]
                      frame True {
                        n1148 = stacked-sequence {
                          tunnel: w1989 -> [w1992 _]
                          tunnel: w1988 -> [_ w1997]
                          tunnel: w1987 -> [w1990 _]
                          frame #0 {
                            n1149 = Build Array("T-RISE") -> (w1994:string[])
                            n1150 = Build Array(w1992) -> (w1993:dbl[])
                            n1151 = TDMS Write(0:w1990, 5:"TEST PASS", 7:w1994, 9:w1993) -> (15:w1996:errorcluster)  [unwired: 2 in, 3 out]
                            n1152 = local write "data file error"(w1996) -> ()
                          }
                          frame #1 {
                            n1153 = Bundle(cluster=w1997, "STATUS"="T-RISE PASS") -> (w1999:T4)  [unwired: 2 in]
                            n1154 = local write "RESULT LAB01-2"(TRUE) -> ()
                            n1155 = local write "DISP LAB01-2"(w1999) -> ()
                          }
                        }
                      }
                      frame False {
                      }
                    }
                  }
                }
              }
              frame #2 {
                # "LAB02-1"
                n1156 = Equal?(x=w2002, y=2) -> (x = y?=w2005:bool)
                n1157 = local read "DISP LAB02-1"() -> (w2007:T4)
                n1158 = Unbundle(w2007) -> ("STATUS"=w2008:string)  [unwired: 2 out]
                n1159 = Equal?(x=w2008, y="RUN") -> (x = y?=w2004:bool)
                n1160 = And(x=w2004, y=w2005) -> (x .and. y?=w2003:bool)
                n1161 = case shown="True" w2003 {
                  tunnel: w2007 -> [_ w2011]
                  tunnel: w2001 -> [_ w2014]
                  frame False {
                  }
                  frame True {
                    n1162 = local read "SET LAB02-1"() -> (w2013:T5)
                    n1163 = local read "TDMS LAB02-1"() -> (w2010:refnum<k34>)
                    n1164 = Unbundle(w2011) -> ("CYCLE"=w2015:dbl)  [unwired: 2 out]
                    n1165 = Unbundle(w2013) -> ("T-RISE mins"=w2012:dbl)  [unwired: 4 out]
                    n1166 = Greater Or Equal?(x=w2015, y=w2014) -> (x >= y?=w2016:bool)
                    n1167 = case shown="True" w2016 {
                      tunnel: w2012 -> [w2019 _]
                      tunnel: w2011 -> [w2018 _]
                      tunnel: w2010 -> [w2017 _]
                      frame True {
                        n1168 = stacked-sequence {
                          tunnel: w2019 -> [w2022 _]
                          tunnel: w2018 -> [_ w2027]
                          tunnel: w2017 -> [w2020 _]
                          frame #0 {
                            n1169 = Build Array("T-RISE") -> (w2024:string[])
                            n1170 = Build Array(w2022) -> (w2023:dbl[])
                            n1171 = TDMS Write(0:w2020, 5:"TEST PASS", 7:w2024, 9:w2023) -> (15:w2026:errorcluster)  [unwired: 2 in, 3 out]
                            n1172 = local write "data file error"(w2026) -> ()
                          }
                          frame #1 {
                            n1173 = Bundle(cluster=w2027, "STATUS"="T-RISE PASS") -> (w2029:T4)  [unwired: 2 in]
                            n1174 = local write "RESULT LAB02-1"(TRUE) -> ()
                            n1175 = local write "DISP LAB02-1"(w2029) -> ()
                          }
                        }
                      }
                      frame False {
                      }
                    }
                  }
                }
              }
              frame #3 {
                # "LAB02-2"
                n1176 = Equal?(x=w2032, y=2) -> (x = y?=w2035:bool)
                n1177 = local read "DISP LAB02-2"() -> (w2037:T4)
                n1178 = Unbundle(w2037) -> ("STATUS"=w2038:string)  [unwired: 2 out]
                n1179 = Equal?(x=w2038, y="RUN") -> (x = y?=w2034:bool)
                n1180 = And(x=w2034, y=w2035) -> (x .and. y?=w2033:bool)
                n1181 = case shown="True" w2033 {
                  tunnel: w2037 -> [_ w2041]
                  tunnel: w2031 -> [_ w2044]
                  frame False {
                  }
                  frame True {
                    n1182 = local read "SET LAB02-2"() -> (w2043:T5)
                    n1183 = local read "TDMS LAB02-2"() -> (w2040:refnum<k34>)
                    n1184 = Unbundle(w2041) -> ("CYCLE"=w2045:dbl)  [unwired: 2 out]
                    n1185 = Unbundle(w2043) -> ("T-RISE mins"=w2042:dbl)  [unwired: 4 out]
                    n1186 = Greater Or Equal?(x=w2045, y=w2044) -> (x >= y?=w2046:bool)
                    n1187 = case shown="True" w2046 {
                      tunnel: w2042 -> [w2049 _]
                      tunnel: w2041 -> [w2048 _]
                      tunnel: w2040 -> [w2047 _]
                      frame True {
                        n1188 = stacked-sequence {
                          tunnel: w2049 -> [w2052 _]
                          tunnel: w2048 -> [_ w2057]
                          tunnel: w2047 -> [w2050 _]
                          frame #0 {
                            n1189 = Build Array("T-RISE") -> (w2054:string[])
                            n1190 = Build Array(w2052) -> (w2053:dbl[])
                            n1191 = TDMS Write(0:w2050, 5:"TEST PASS", 7:w2054, 9:w2053) -> (15:w2056:errorcluster)  [unwired: 2 in, 3 out]
                            n1192 = local write "data file error"(w2056) -> ()
                          }
                          frame #1 {
                            n1193 = Bundle(cluster=w2057, "STATUS"="T-RISE PASS") -> (w2059:T4)  [unwired: 2 in]
                            n1194 = local write "RESULT LAB02-2"(TRUE) -> ()
                            n1195 = local write "DISP LAB02-2"(w2059) -> ()
                          }
                        }
                      }
                      frame False {
                      }
                    }
                  }
                }
              }
              frame #4 {
                # "LAB03-1"
                n1196 = Equal?(x=w2062, y=2) -> (x = y?=w2065:bool)
                n1197 = local read "DISP LAB03-1"() -> (w2067:T4)
                n1198 = Unbundle(w2067) -> ("STATUS"=w2068:string)  [unwired: 2 out]
                n1199 = Equal?(x=w2068, y="RUN") -> (x = y?=w2064:bool)
                n1200 = And(x=w2064, y=w2065) -> (x .and. y?=w2063:bool)
                n1201 = case shown="True" w2063 {
                  tunnel: w2067 -> [_ w2071]
                  tunnel: w2061 -> [_ w2074]
                  frame False {
                  }
                  frame True {
                    n1202 = local read "SET LAB03-1"() -> (w2073:T5)
                    n1203 = local read "TDMS LAB03-1"() -> (w2070:refnum<k34>)
                    n1204 = Unbundle(w2071) -> ("CYCLE"=w2075:dbl)  [unwired: 2 out]
                    n1205 = Unbundle(w2073) -> ("T-RISE mins"=w2072:dbl)  [unwired: 4 out]
                    n1206 = Greater Or Equal?(x=w2075, y=w2074) -> (x >= y?=w2076:bool)
                    n1207 = case shown="True" w2076 {
                      tunnel: w2072 -> [w2079 _]
                      tunnel: w2071 -> [w2078 _]
                      tunnel: w2070 -> [w2077 _]
                      frame True {
                        n1208 = stacked-sequence {
                          tunnel: w2079 -> [w2082 _]
                          tunnel: w2078 -> [_ w2087]
                          tunnel: w2077 -> [w2080 _]
                          frame #0 {
                            n1209 = Build Array("T-RISE") -> (w2084:string[])
                            n1210 = Build Array(w2082) -> (w2083:dbl[])
                            n1211 = TDMS Write(0:w2080, 5:"TEST PASS", 7:w2084, 9:w2083) -> (15:w2086:errorcluster)  [unwired: 2 in, 3 out]
                            n1212 = local write "data file error"(w2086) -> ()
                          }
                          frame #1 {
                            n1213 = Bundle(cluster=w2087, "STATUS"="T-RISE PASS") -> (w2089:T4)  [unwired: 2 in]
                            n1214 = local write "RESULT LAB03-1"(TRUE) -> ()
                            n1215 = local write "DISP LAB03-1"(w2089) -> ()
                          }
                        }
                      }
                      frame False {
                      }
                    }
                  }
                }
              }
              frame #5 {
                # "LAB03-2"
                n1216 = Equal?(x=w2092, y=2) -> (x = y?=w2095:bool)
                n1217 = local read "DISP LAB03-2"() -> (w2097:T4)
                n1218 = Unbundle(w2097) -> ("STATUS"=w2098:string)  [unwired: 2 out]
                n1219 = Equal?(x=w2098, y="RUN") -> (x = y?=w2094:bool)
                n1220 = And(x=w2094, y=w2095) -> (x .and. y?=w2093:bool)
                n1221 = case shown="True" w2093 {
                  tunnel: w2097 -> [_ w2101]
                  tunnel: w2091 -> [_ w2104]
                  frame False {
                  }
                  frame True {
                    n1222 = local read "SET LAB03-2"() -> (w2103:T5)
                    n1223 = local read "TDMS LAB03-2"() -> (w2100:refnum<k34>)
                    n1224 = Unbundle(w2101) -> ("CYCLE"=w2105:dbl)  [unwired: 2 out]
                    n1225 = Unbundle(w2103) -> ("T-RISE mins"=w2102:dbl)  [unwired: 4 out]
                    n1226 = Greater Or Equal?(x=w2105, y=w2104) -> (x >= y?=w2106:bool)
                    n1227 = case shown="True" w2106 {
                      tunnel: w2102 -> [w2109 _]
                      tunnel: w2101 -> [w2108 _]
                      tunnel: w2100 -> [w2107 _]
                      frame True {
                        n1228 = stacked-sequence {
                          tunnel: w2109 -> [w2112 _]
                          tunnel: w2108 -> [_ w2117]
                          tunnel: w2107 -> [w2110 _]
                          frame #0 {
                            n1229 = Build Array("T-RISE") -> (w2114:string[])
                            n1230 = Build Array(w2112) -> (w2113:dbl[])
                            n1231 = TDMS Write(0:w2110, 5:"TEST PASS", 7:w2114, 9:w2113) -> (15:w2116:errorcluster)  [unwired: 2 in, 3 out]
                            n1232 = local write "data file error"(w2116) -> ()
                          }
                          frame #1 {
                            n1233 = Bundle(cluster=w2117, "STATUS"="T-RISE PASS") -> (w2119:T4)  [unwired: 2 in]
                            n1234 = local write "RESULT LAB03-2"(TRUE) -> ()
                            n1235 = local write "DISP LAB03-2"(w2119) -> ()
                          }
                        }
                      }
                      frame False {
                      }
                    }
                  }
                }
              }
              frame #6 {
                # "LAB04-1"
                n1236 = Equal?(x=w2122, y=2) -> (x = y?=w2125:bool)
                n1237 = local read "DISP LAB04-1"() -> (w2127:T4)
                n1238 = Unbundle(w2127) -> ("STATUS"=w2128:string)  [unwired: 2 out]
                n1239 = Equal?(x=w2128, y="RUN") -> (x = y?=w2124:bool)
                n1240 = And(x=w2124, y=w2125) -> (x .and. y?=w2123:bool)
                n1241 = case shown="True" w2123 {
                  tunnel: w2127 -> [_ w2131]
                  tunnel: w2121 -> [_ w2134]
                  frame False {
                  }
                  frame True {
                    n1242 = local read "SET LAB04-1"() -> (w2133:T5)
                    n1243 = local read "TDMS LAB04-1"() -> (w2130:refnum<k34>)
                    n1244 = Unbundle(w2131) -> ("CYCLE"=w2135:dbl)  [unwired: 2 out]
                    n1245 = Unbundle(w2133) -> ("T-RISE mins"=w2132:dbl)  [unwired: 4 out]
                    n1246 = Greater Or Equal?(x=w2135, y=w2134) -> (x >= y?=w2136:bool)
                    n1247 = case shown="True" w2136 {
                      tunnel: w2132 -> [w2139 _]
                      tunnel: w2131 -> [w2138 _]
                      tunnel: w2130 -> [w2137 _]
                      frame True {
                        n1248 = stacked-sequence {
                          tunnel: w2139 -> [w2142 _]
                          tunnel: w2138 -> [_ w2147]
                          tunnel: w2137 -> [w2140 _]
                          frame #0 {
                            n1249 = Build Array("T-RISE") -> (w2144:string[])
                            n1250 = Build Array(w2142) -> (w2143:dbl[])
                            n1251 = TDMS Write(0:w2140, 5:"TEST PASS", 7:w2144, 9:w2143) -> (15:w2146:errorcluster)  [unwired: 2 in, 3 out]
                            n1252 = local write "data file error"(w2146) -> ()
                          }
                          frame #1 {
                            n1253 = Bundle(cluster=w2147, "STATUS"="T-RISE PASS") -> (w2149:T4)  [unwired: 2 in]
                            n1254 = local write "RESULT LAB04-1"(TRUE) -> ()
                            n1255 = local write "DISP LAB04-1"(w2149) -> ()
                          }
                        }
                      }
                      frame False {
                      }
                    }
                  }
                }
              }
              frame #7 {
                # "LAB04-2"
                n1256 = Equal?(x=w2152, y=2) -> (x = y?=w2155:bool)
                n1257 = local read "DISP LAB04-2"() -> (w2157:T4)
                n1258 = Unbundle(w2157) -> ("STATUS"=w2158:string)  [unwired: 2 out]
                n1259 = Equal?(x=w2158, y="RUN") -> (x = y?=w2154:bool)
                n1260 = And(x=w2154, y=w2155) -> (x .and. y?=w2153:bool)
                n1261 = case shown="True" w2153 {
                  tunnel: w2157 -> [_ w2161]
                  tunnel: w2151 -> [_ w2164]
                  frame False {
                  }
                  frame True {
                    n1262 = local read "SET LAB04-2"() -> (w2163:T5)
                    n1263 = local read "TDMS LAB04-2"() -> (w2160:refnum<k34>)
                    n1264 = Unbundle(w2161) -> ("CYCLE"=w2165:dbl)  [unwired: 2 out]
                    n1265 = Unbundle(w2163) -> ("T-RISE mins"=w2162:dbl)  [unwired: 4 out]
                    n1266 = Greater Or Equal?(x=w2165, y=w2164) -> (x >= y?=w2166:bool)
                    n1267 = case shown="True" w2166 {
                      tunnel: w2162 -> [w2169 _]
                      tunnel: w2161 -> [w2168 _]
                      tunnel: w2160 -> [w2167 _]
                      frame True {
                        n1268 = stacked-sequence {
                          tunnel: w2169 -> [w2172 _]
                          tunnel: w2168 -> [_ w2177]
                          tunnel: w2167 -> [w2170 _]
                          frame #0 {
                            n1269 = Build Array("T-RISE") -> (w2174:string[])
                            n1270 = Build Array(w2172) -> (w2173:dbl[])
                            n1271 = TDMS Write(0:w2170, 5:"TEST PASS", 7:w2174, 9:w2173) -> (15:w2176:errorcluster)  [unwired: 2 in, 3 out]
                            n1272 = local write "data file error"(w2176) -> ()
                          }
                          frame #1 {
                            n1273 = Bundle(cluster=w2177, "STATUS"="T-RISE PASS") -> (w2179:T4)  [unwired: 2 in]
                            n1274 = local write "RESULT LAB04-2"(TRUE) -> ()
                            n1275 = local write "DISP LAB04-2"(w2179) -> ()
                          }
                        }
                      }
                      frame False {
                      }
                    }
                  }
                }
              }
              frame #8 {
                # "LAB05-1"
                n1276 = Equal?(x=w2182, y=2) -> (x = y?=w2185:bool)
                n1277 = local read "DISP LAB05-1"() -> (w2187:T4)
                n1278 = Unbundle(w2187) -> ("STATUS"=w2188:string)  [unwired: 2 out]
                n1279 = Equal?(x=w2188, y="RUN") -> (x = y?=w2184:bool)
                n1280 = And(x=w2184, y=w2185) -> (x .and. y?=w2183:bool)
                n1281 = case shown="True" w2183 {
                  tunnel: w2187 -> [_ w2191]
                  tunnel: w2181 -> [_ w2194]
                  frame False {
                  }
                  frame True {
                    n1282 = local read "SET LAB05-1"() -> (w2193:T5)
                    n1283 = local read "TDMS LAB05-1"() -> (w2190:refnum<k34>)
                    n1284 = Unbundle(w2191) -> ("CYCLE"=w2195:dbl)  [unwired: 2 out]
                    n1285 = Unbundle(w2193) -> ("T-RISE mins"=w2192:dbl)  [unwired: 4 out]
                    n1286 = Greater Or Equal?(x=w2195, y=w2194) -> (x >= y?=w2196:bool)
                    n1287 = case shown="True" w2196 {
                      tunnel: w2192 -> [w2199 _]
                      tunnel: w2191 -> [w2198 _]
                      tunnel: w2190 -> [w2197 _]
                      frame True {
                        n1288 = stacked-sequence {
                          tunnel: w2199 -> [w2202 _]
                          tunnel: w2198 -> [_ w2207]
                          tunnel: w2197 -> [w2200 _]
                          frame #0 {
                            n1289 = Build Array("T-RISE") -> (w2204:string[])
                            n1290 = Build Array(w2202) -> (w2203:dbl[])
                            n1291 = TDMS Write(0:w2200, 5:"TEST PASS", 7:w2204, 9:w2203) -> (15:w2206:errorcluster)  [unwired: 2 in, 3 out]
                            n1292 = local write "data file error"(w2206) -> ()
                          }
                          frame #1 {
                            n1293 = Bundle(cluster=w2207, "STATUS"="T-RISE PASS") -> (w2209:T4)  [unwired: 2 in]
                            n1294 = local write "RESULT LAB05-1"(TRUE) -> ()
                            n1295 = local write "DISP LAB05-1"(w2209) -> ()
                          }
                        }
                      }
                      frame False {
                      }
                    }
                  }
                }
              }
              frame #9 {
                # "LAB05-2"
                n1296 = Equal?(x=w2212, y=2) -> (x = y?=w2215:bool)
                n1297 = local read "DISP LAB05-2"() -> (w2217:T4)
                n1298 = Unbundle(w2217) -> ("STATUS"=w2218:string)  [unwired: 2 out]
                n1299 = Equal?(x=w2218, y="RUN") -> (x = y?=w2214:bool)
                n1300 = And(x=w2214, y=w2215) -> (x .and. y?=w2213:bool)
                n1301 = case shown="True" w2213 {
                  tunnel: w2217 -> [_ w2221]
                  tunnel: w2211 -> [_ w2224]
                  frame False {
                  }
                  frame True {
                    n1302 = local read "SET LAB05-2"() -> (w2223:T5)
                    n1303 = local read "TDMS LAB05-2"() -> (w2220:refnum<k34>)
                    n1304 = Unbundle(w2221) -> ("CYCLE"=w2225:dbl)  [unwired: 2 out]
                    n1305 = Unbundle(w2223) -> ("T-RISE mins"=w2222:dbl)  [unwired: 4 out]
                    n1306 = Greater Or Equal?(x=w2225, y=w2224) -> (x >= y?=w2226:bool)
                    n1307 = case shown="True" w2226 {
                      tunnel: w2222 -> [w2229 _]
                      tunnel: w2221 -> [w2228 _]
                      tunnel: w2220 -> [w2227 _]
                      frame True {
                        n1308 = stacked-sequence {
                          tunnel: w2229 -> [w2232 _]
                          tunnel: w2228 -> [_ w2237]
                          tunnel: w2227 -> [w2230 _]
                          frame #0 {
                            n1309 = Build Array("T-RISE") -> (w2234:string[])
                            n1310 = Build Array(w2232) -> (w2233:dbl[])
                            n1311 = TDMS Write(0:w2230, 5:"TEST PASS", 7:w2234, 9:w2233) -> (15:w2236:errorcluster)  [unwired: 2 in, 3 out]
                            n1312 = local write "data file error"(w2236) -> ()
                          }
                          frame #1 {
                            n1313 = Bundle(cluster=w2237, "STATUS"="T-RISE PASS") -> (w2239:T4)  [unwired: 2 in]
                            n1314 = local write "RESULT LAB05-2"(TRUE) -> ()
                            n1315 = local write "DISP LAB05-2"(w2239) -> ()
                          }
                        }
                      }
                      frame False {
                      }
                    }
                  }
                }
              }
            }
          }
          frame #6 {
            # "end test & close test files"
            n1316 = stacked-sequence {
              tunnel: w2250 -> [_ _ _ _ _ _ _ _ _ _]
              tunnel: w2251 -> [_ _ _ _ _ _ _ _ _ _]
              tunnel: w2249 -> [_ _ _ _ _ _ _ _ _ _]
              tunnel: w2248 -> [_ _ _ _ _ _ _ _ _ _]
              tunnel: w2247 -> [_ _ _ _ _ _ _ _ _ _]
              tunnel: w2246 -> [_ _ _ _ _ _ _ _ _ _]
              tunnel: w2245 -> [_ _ _ _ _ _ _ _ _ _]
              tunnel: w2244 -> [_ _ _ _ _ _ _ _ _ _]
              tunnel: w2243 -> [_ _ _ _ _ _ _ _ _ _]
              tunnel: w2242 -> [_ _ _ _ _ _ _ _ _ _]
              frame #0 {
                # "LAB01-1"
                n1317 = local read "DISP LAB01-1"() -> (w2255:T4)
                n1318 = local read "run lab01-1"() -> (w2252:bool)
                n1319 = local read "TDMS LAB01-1"() -> (w2253:refnum<k34>)
                n1320 = Unbundle(w2255) -> ("CYCLE"=w2256:dbl, "STATUS"=w2254:string)  [unwired: 1 out]
                n1321 = case shown="True" w2252 {
                  tunnel: w2256 -> [_ w2260]
                  tunnel: w2255 -> [_ w2259]
                  tunnel: w2254 -> [_ w2258]
                  tunnel: w2253 -> [_ w2257]
                  frame False {
                  }
                  frame True {
                    n1322 = Not Equal?(x=w2258, y="RUN") -> (x != y?=w2261:bool)
                    n1323 = Greater?(x=w2260, y=2.0) -> (0:w2263:bool)
                    n1324 = And(x=w2263, y=w2261) -> (x .and. y?=w2262:bool)
                    n1325 = case shown="True" w2262 {
                      tunnel: w2259 -> [_ w2267]
                      tunnel: w2257 -> [_ w2266]
                      frame False {
                      }
                      frame True {
                        n1326 = stacked-sequence {
                          tunnel: w2267 -> [w2271 _ _]
                          tunnel: w2266 -> [_ w2273 _]
                          frame #0 {
                            w2268 = FALSE
                            n1327 = local write "mail control"("END") -> ()
                            n1328 = Bundle(cluster=w2271) -> (w2270:T4)  [unwired: 3 in]
                            n1329 = local write "DISP LAB01-1"(w2270) -> ()
                            n1330 = local write "O/I  LAB01-1"(w2268) -> ()
                            n1331 = local write "run lab01-1"(w2268) -> ()
                            n1332 = local write "RUN LAB01-1"(w2268) -> ()
                          }
                          frame #1 {
                            n1333 = TDMS Close(11:w2273) -> (0:w2272:errorcluster)  [unwired: 1 in, 1 out]
                            n1334 = local write "data file error"(w2272) -> ()
                          }
                          frame #2 {
                            n1335 = stacked-sequence {
                              tunnel: "LAB01-1" -> [w2276 w2278]
                              frame #0 {
                                n1336 = call "sub vi - defrag tdms v1.vi"("panel id"=w2276) -> ("error out"=w2275:errorcluster)  [unwired: 10 in]
                                n1337 = local write "data file error"(w2275) -> ()
                              }
                              frame #1 {
                                n1338 = call "Save data file to network drive v1.vi"("panel id"=w2278) -> ("network file save error"=w2277:errorcluster)  [unwired: 9 in, 1 out]
                                n1339 = local write "data file error"(w2277) -> ()
                              }
                            }
                          }
                        }
                      }
                    }
                  }
                }
              }
              frame #1 {
                # "LAB01-2"
                n1340 = local read "run lab01-2"() -> (w2279:bool)
                n1341 = case shown="True" w2279 {
                  frame False {
                  }
                  frame True {
                    n1342 = local read "DISP LAB01-2"() -> (w2286:T4)
                    n1343 = local read "TDMS LAB01-2"() -> (w2285:refnum<k34>)
                    n1344 = Unbundle(w2286) -> ("CYCLE"=w2282:dbl, "STATUS"=w2287:string)  [unwired: 1 out]
                    n1345 = Not Equal?(x=w2287, y="RUN") -> (x != y?=w2281:bool)
                    n1346 = Greater?(x=w2282, y=2.0) -> (0:w2283:bool)
                    n1347 = And(x=w2283, y=w2281) -> (x .and. y?=w2280:bool)
                    n1348 = case shown="True" w2280 {
                      tunnel: w2286 -> [_ w2290]
                      tunnel: w2285 -> [_ w2289]
                      frame False {
                      }
                      frame True {
                        n1349 = stacked-sequence {
                          tunnel: w2290 -> [w2293 _ _]
                          tunnel: w2289 -> [_ w2295 _]
                          frame #0 {
                            w2291 = FALSE
                            n1350 = local write "mail control"("END") -> ()
                            n1351 = Bundle(cluster=w2293) -> (w2294:T4)  [unwired: 3 in]
                            n1352 = local write "RUN LAB01-2"(w2291) -> ()
                            n1353 = local write "run lab01-2"(w2291) -> ()
                            n1354 = local write "O/I  LAB01-2"(w2291) -> ()
                            n1355 = local write "DISP LAB01-2"(w2294) -> ()
                          }
                          frame #1 {
                            n1356 = TDMS Close(11:w2295) -> (0:w2296:errorcluster)  [unwired: 1 in, 1 out]
                            n1357 = local write "data file error"(w2296) -> ()
                          }
                          frame #2 {
                            n1358 = stacked-sequence {
                              tunnel: "LAB01-2" -> [w2299 w2301]
                              frame #0 {
                                n1359 = call "sub vi - defrag tdms v1.vi"("panel id"=w2299) -> ("error out"=w2298:errorcluster)  [unwired: 10 in]
                                n1360 = local write "data file error"(w2298) -> ()
                              }
                              frame #1 {
                                n1361 = call "Save data file to network drive v1.vi"("panel id"=w2301) -> ("network file save error"=w2300:errorcluster)  [unwired: 9 in, 1 out]
                                n1362 = local write "data file error"(w2300) -> ()
                              }
                            }
                          }
                        }
                      }
                    }
                  }
                }
              }
              frame #2 {
                # "LAB02-1"
                n1363 = local read "run lab02-1"() -> (w2302:bool)
                n1364 = case shown="True" w2302 {
                  frame False {
                  }
                  frame True {
                    n1365 = local read "DISP LAB02-1"() -> (w2309:T4)
                    n1366 = Unbundle(w2309) -> ("CYCLE"=w2305:dbl, "STATUS"=w2310:string)  [unwired: 1 out]
                    n1367 = local read "TDMS LAB02-1"() -> (w2308:refnum<k34>)
                    n1368 = Not Equal?(x=w2310, y="RUN") -> (x != y?=w2304:bool)
                    n1369 = Greater?(x=w2305, y=2.0) -> (0:w2306:bool)
                    n1370 = And(x=w2306, y=w2304) -> (x .and. y?=w2303:bool)
                    n1371 = case shown="True" w2303 {
                      tunnel: w2309 -> [_ w2313]
                      tunnel: w2308 -> [_ w2312]
                      frame False {
                      }
                      frame True {
                        n1372 = stacked-sequence {
                          tunnel: w2313 -> [w2316 _ _]
                          tunnel: w2312 -> [_ w2318 _]
                          frame #0 {
                            w2314 = FALSE
                            n1373 = local write "mail control"("END") -> ()
                            n1374 = Bundle(cluster=w2316) -> (w2317:T4)  [unwired: 3 in]
                            n1375 = local write "O/I  LAB02-1"(w2314) -> ()
                            n1376 = local write "RUN LAB02-1"(w2314) -> ()
                            n1377 = local write "run lab02-1"(w2314) -> ()
                            n1378 = local write "DISP LAB02-1"(w2317) -> ()
                          }
                          frame #1 {
                            n1379 = TDMS Close(11:w2318) -> (0:w2319:errorcluster)  [unwired: 1 in, 1 out]
                            n1380 = local write "data file error"(w2319) -> ()
                          }
                          frame #2 {
                            n1381 = stacked-sequence {
                              tunnel: "LAB02-1" -> [w2322 w2324]
                              frame #0 {
                                n1382 = call "sub vi - defrag tdms v1.vi"("panel id"=w2322) -> ("error out"=w2321:errorcluster)  [unwired: 10 in]
                                n1383 = local write "data file error"(w2321) -> ()
                              }
                              frame #1 {
                                n1384 = call "Save data file to network drive v1.vi"("panel id"=w2324) -> ("network file save error"=w2323:errorcluster)  [unwired: 9 in, 1 out]
                                n1385 = local write "data file error"(w2323) -> ()
                              }
                            }
                          }
                        }
                      }
                    }
                  }
                }
              }
              frame #3 {
                # "LAB02-2"
                n1386 = local read "run lab02-2"() -> (w2325:bool)
                n1387 = case shown="True" w2325 {
                  frame False {
                  }
                  frame True {
                    n1388 = local read "DISP LAB02-2"() -> (w2332:T4)
                    n1389 = local read "TDMS LAB02-2"() -> (w2331:refnum<k34>)
                    n1390 = Unbundle(w2332) -> ("CYCLE"=w2328:dbl, "STATUS"=w2333:string)  [unwired: 1 out]
                    n1391 = Not Equal?(x=w2333, y="RUN") -> (x != y?=w2327:bool)
                    n1392 = Greater?(x=w2328, y=2.0) -> (0:w2329:bool)
                    n1393 = And(x=w2329, y=w2327) -> (x .and. y?=w2326:bool)
                    n1394 = case shown="True" w2326 {
                      tunnel: w2332 -> [_ w2336]
                      tunnel: w2331 -> [_ w2335]
                      frame False {
                      }
                      frame True {
                        n1395 = stacked-sequence {
                          tunnel: w2336 -> [w2339 _ _]
                          tunnel: w2335 -> [_ w2341 _]
                          frame #0 {
                            w2337 = FALSE
                            n1396 = local write "mail control"("END") -> ()
                            n1397 = Bundle(cluster=w2339) -> (w2340:T4)  [unwired: 3 in]
                            n1398 = local write "O/I  LAB02-2"(w2337) -> ()
                            n1399 = local write "run lab02-2"(w2337) -> ()
                            n1400 = local write "RUN LAB02-2"(w2337) -> ()
                            n1401 = local write "DISP LAB02-2"(w2340) -> ()
                          }
                          frame #1 {
                            n1402 = TDMS Close(11:w2341) -> (0:w2342:errorcluster)  [unwired: 1 in, 1 out]
                            n1403 = local write "data file error"(w2342) -> ()
                          }
                          frame #2 {
                            n1404 = stacked-sequence {
                              tunnel: "LAB02-2" -> [w2345 w2347]
                              frame #0 {
                                n1405 = call "sub vi - defrag tdms v1.vi"("panel id"=w2345) -> ("error out"=w2344:errorcluster)  [unwired: 10 in]
                                n1406 = local write "data file error"(w2344) -> ()
                              }
                              frame #1 {
                                n1407 = call "Save data file to network drive v1.vi"("panel id"=w2347) -> ("network file save error"=w2346:errorcluster)  [unwired: 9 in, 1 out]
                                n1408 = local write "data file error"(w2346) -> ()
                              }
                            }
                          }
                        }
                      }
                    }
                  }
                }
              }
              frame #4 {
                # "LAB03-1"
                n1409 = local read "run lab03-1"() -> (w2348:bool)
                n1410 = case shown="True" w2348 {
                  frame False {
                  }
                  frame True {
                    n1411 = local read "DISP LAB03-1"() -> (w2355:T4)
                    n1412 = local read "TDMS LAB03-1"() -> (w2354:refnum<k34>)
                    n1413 = Unbundle(w2355) -> ("CYCLE"=w2351:dbl, "STATUS"=w2356:string)  [unwired: 1 out]
                    n1414 = Not Equal?(x=w2356, y="RUN") -> (x != y?=w2350:bool)
                    n1415 = Greater?(x=w2351, y=2.0) -> (0:w2352:bool)
                    n1416 = And(x=w2352, y=w2350) -> (x .and. y?=w2349:bool)
                    n1417 = case shown="True" w2349 {
                      tunnel: w2355 -> [_ w2359]
                      tunnel: w2354 -> [_ w2358]
                      frame False {
                      }
                      frame True {
                        n1418 = stacked-sequence {
                          tunnel: w2359 -> [w2362 _ _]
                          tunnel: w2358 -> [_ w2364 _]
                          frame #0 {
                            w2360 = FALSE
                            n1419 = local write "mail control"("END") -> ()
                            n1420 = Bundle(cluster=w2362) -> (w2363:T4)  [unwired: 3 in]
                            n1421 = local write "O/I  LAB03-1"(w2360) -> ()
                            n1422 = local write "run lab03-1"(w2360) -> ()
                            n1423 = local write "RUN LAB03-1"(w2360) -> ()
                            n1424 = local write "DISP LAB03-1"(w2363) -> ()
                          }
                          frame #1 {
                            n1425 = TDMS Close(11:w2364) -> (0:w2365:errorcluster)  [unwired: 1 in, 1 out]
                            n1426 = local write "data file error"(w2365) -> ()
                          }
                          frame #2 {
                            n1427 = stacked-sequence {
                              tunnel: "LAB03-1" -> [w2368 w2370]
                              frame #0 {
                                n1428 = call "sub vi - defrag tdms v1.vi"("panel id"=w2368) -> ("error out"=w2367:errorcluster)  [unwired: 10 in]
                                n1429 = local write "data file error"(w2367) -> ()
                              }
                              frame #1 {
                                n1430 = call "Save data file to network drive v1.vi"("panel id"=w2370) -> ("network file save error"=w2369:errorcluster)  [unwired: 9 in, 1 out]
                                n1431 = local write "data file error"(w2369) -> ()
                              }
                            }
                          }
                        }
                      }
                    }
                  }
                }
              }
              frame #5 {
                # "LAB03-2"
                n1432 = local read "run lab03-2"() -> (w2371:bool)
                n1433 = case shown="True" w2371 {
                  frame False {
                  }
                  frame True {
                    n1434 = local read "DISP LAB03-2"() -> (w2378:T4)
                    n1435 = Unbundle(w2378) -> ("CYCLE"=w2374:dbl, "STATUS"=w2379:string)  [unwired: 1 out]
                    n1436 = local read "TDMS LAB03-2"() -> (w2377:refnum<k34>)
                    n1437 = Not Equal?(x=w2379, y="RUN") -> (x != y?=w2373:bool)
                    n1438 = Greater?(x=w2374, y=2.0) -> (0:w2375:bool)
                    n1439 = And(x=w2375, y=w2373) -> (x .and. y?=w2372:bool)
                    n1440 = case shown="True" w2372 {
                      tunnel: w2378 -> [_ w2382]
                      tunnel: w2377 -> [_ w2381]
                      frame False {
                      }
                      frame True {
                        n1441 = stacked-sequence {
                          tunnel: w2382 -> [w2385 _ _]
                          tunnel: w2381 -> [_ w2387 _]
                          frame #0 {
                            w2383 = FALSE
                            n1442 = local write "mail control"("END") -> ()
                            n1443 = Bundle(cluster=w2385) -> (w2386:T4)  [unwired: 3 in]
                            n1444 = local write "RUN LAB03-2"(w2383) -> ()
                            n1445 = local write "O/I  LAB03-2"(w2383) -> ()
                            n1446 = local write "DISP LAB03-2"(w2386) -> ()
                            n1447 = local write "run lab03-2"(w2383) -> ()
                          }
                          frame #1 {
                            n1448 = TDMS Close(11:w2387) -> (0:w2388:errorcluster)  [unwired: 1 in, 1 out]
                            n1449 = local write "data file error"(w2388) -> ()
                          }
                          frame #2 {
                            n1450 = stacked-sequence {
                              tunnel: "LAB03-2" -> [w2391 w2393]
                              frame #0 {
                                n1451 = call "sub vi - defrag tdms v1.vi"("panel id"=w2391) -> ("error out"=w2390:errorcluster)  [unwired: 10 in]
                                n1452 = local write "data file error"(w2390) -> ()
                              }
                              frame #1 {
                                n1453 = call "Save data file to network drive v1.vi"("panel id"=w2393) -> ("network file save error"=w2392:errorcluster)  [unwired: 9 in, 1 out]
                                n1454 = local write "data file error"(w2392) -> ()
                              }
                            }
                          }
                        }
                      }
                    }
                  }
                }
              }
              frame #6 {
                # "LAB04-1"
                n1455 = local read "run lab04-1"() -> (w2394:bool)
                n1456 = case shown="True" w2394 {
                  frame False {
                  }
                  frame True {
                    n1457 = local read "DISP LAB04-1"() -> (w2401:T4)
                    n1458 = Unbundle(w2401) -> ("CYCLE"=w2397:dbl, "STATUS"=w2402:string)  [unwired: 1 out]
                    n1459 = local read "TDMS LAB04-1"() -> (w2400:refnum<k34>)
                    n1460 = Not Equal?(x=w2402, y="RUN") -> (x != y?=w2396:bool)
                    n1461 = Greater?(x=w2397, y=2.0) -> (0:w2398:bool)
                    n1462 = And(x=w2398, y=w2396) -> (x .and. y?=w2395:bool)
                    n1463 = case shown="True" w2395 {
                      tunnel: w2401 -> [_ w2405]
                      tunnel: w2400 -> [_ w2404]
                      frame False {
                      }
                      frame True {
                        n1464 = stacked-sequence {
                          tunnel: w2405 -> [w2408 _ _]
                          tunnel: w2404 -> [_ w2410 _]
                          frame #0 {
                            w2406 = FALSE
                            n1465 = local write "mail control"("END") -> ()
                            n1466 = Bundle(cluster=w2408) -> (w2409:T4)  [unwired: 3 in]
                            n1467 = local write "RUN LAB04-1"(w2406) -> ()
                            n1468 = local write "O/I  LAB04-1"(w2406) -> ()
                            n1469 = local write "run lab04-1"(w2406) -> ()
                            n1470 = local write "DISP LAB04-1"(w2409) -> ()
                          }
                          frame #1 {
                            n1471 = TDMS Close(11:w2410) -> (0:w2411:errorcluster)  [unwired: 1 in, 1 out]
                            n1472 = local write "data file error"(w2411) -> ()
                          }
                          frame #2 {
                            n1473 = stacked-sequence {
                              tunnel: "LAB04-1" -> [w2414 w2416]
                              frame #0 {
                                n1474 = call "sub vi - defrag tdms v1.vi"("panel id"=w2414) -> ("error out"=w2413:errorcluster)  [unwired: 10 in]
                                n1475 = local write "data file error"(w2413) -> ()
                              }
                              frame #1 {
                                n1476 = call "Save data file to network drive v1.vi"("panel id"=w2416) -> ("network file save error"=w2415:errorcluster)  [unwired: 9 in, 1 out]
                                n1477 = local write "data file error"(w2415) -> ()
                              }
                            }
                          }
                        }
                      }
                    }
                  }
                }
              }
              frame #7 {
                # "LAB04-2"
                n1478 = local read "run lab04-2"() -> (w2417:bool)
                n1479 = case shown="True" w2417 {
                  frame False {
                  }
                  frame True {
                    n1480 = local read "DISP LAB04-2"() -> (w2424:T4)
                    n1481 = Unbundle(w2424) -> ("CYCLE"=w2420:dbl, "STATUS"=w2425:string)  [unwired: 1 out]
                    n1482 = Not Equal?(x=w2425, y="RUN") -> (x != y?=w2419:bool)
                    n1483 = local read "TDMS LAB04-2"() -> (w2423:refnum<k34>)
                    n1484 = Greater?(x=w2420, y=2.0) -> (0:w2421:bool)
                    n1485 = And(x=w2421, y=w2419) -> (x .and. y?=w2418:bool)
                    n1486 = case shown="True" w2418 {
                      tunnel: w2424 -> [_ w2428]
                      tunnel: w2423 -> [_ w2427]
                      frame False {
                      }
                      frame True {
                        n1487 = stacked-sequence {
                          tunnel: w2428 -> [w2431 _ _]
                          tunnel: w2427 -> [_ w2433 _]
                          frame #0 {
                            w2429 = FALSE
                            n1488 = local write "mail control"("END") -> ()
                            n1489 = Bundle(cluster=w2431) -> (w2432:T4)  [unwired: 3 in]
                            n1490 = local write "O/I  LAB04-2"(w2429) -> ()
                            n1491 = local write "RUN LAB04-2"(w2429) -> ()
                            n1492 = local write "run lab04-2"(w2429) -> ()
                            n1493 = local write "DISP LAB04-2"(w2432) -> ()
                          }
                          frame #1 {
                            n1494 = TDMS Close(11:w2433) -> (0:w2434:errorcluster)  [unwired: 1 in, 1 out]
                            n1495 = local write "data file error"(w2434) -> ()
                          }
                          frame #2 {
                            n1496 = stacked-sequence {
                              tunnel: "LAB04-2" -> [w2437 w2439]
                              frame #0 {
                                n1497 = call "sub vi - defrag tdms v1.vi"("panel id"=w2437) -> ("error out"=w2436:errorcluster)  [unwired: 10 in]
                                n1498 = local write "data file error"(w2436) -> ()
                              }
                              frame #1 {
                                n1499 = call "Save data file to network drive v1.vi"("panel id"=w2439) -> ("network file save error"=w2438:errorcluster)  [unwired: 9 in, 1 out]
                                n1500 = local write "data file error"(w2438) -> ()
                              }
                            }
                          }
                        }
                      }
                    }
                  }
                }
              }
              frame #8 {
                # "LAB05-1"
                n1501 = local read "run lab05-1"() -> (w2440:bool)
                n1502 = case shown="True" w2440 {
                  frame False {
                  }
                  frame True {
                    n1503 = local read "DISP LAB05-1"() -> (w2447:T4)
                    n1504 = Unbundle(w2447) -> ("CYCLE"=w2443:dbl, "STATUS"=w2448:string)  [unwired: 1 out]
                    n1505 = Not Equal?(x=w2448, y="RUN") -> (x != y?=w2442:bool)
                    n1506 = local read "TDMS LAB05-1"() -> (w2446:refnum<k34>)
                    n1507 = Greater?(x=w2443, y=2.0) -> (0:w2444:bool)
                    n1508 = And(x=w2444, y=w2442) -> (x .and. y?=w2441:bool)
                    n1509 = case shown="True" w2441 {
                      tunnel: w2447 -> [_ w2451]
                      tunnel: w2446 -> [_ w2450]
                      frame False {
                      }
                      frame True {
                        n1510 = stacked-sequence {
                          tunnel: w2451 -> [w2454 _ _]
                          tunnel: w2450 -> [_ w2456 _]
                          frame #0 {
                            w2452 = FALSE
                            n1511 = local write "mail control"("END") -> ()
                            n1512 = Bundle(cluster=w2454) -> (w2455:T4)  [unwired: 3 in]
                            n1513 = local write "O/I  LAB05-1"(w2452) -> ()
                            n1514 = local write "RUN LAB05-1"(w2452) -> ()
                            n1515 = local write "run lab05-1"(w2452) -> ()
                            n1516 = local write "DISP LAB05-1"(w2455) -> ()
                          }
                          frame #1 {
                            n1517 = TDMS Close(11:w2456) -> (0:w2457:errorcluster)  [unwired: 1 in, 1 out]
                            n1518 = local write "data file error"(w2457) -> ()
                          }
                          frame #2 {
                            n1519 = stacked-sequence {
                              tunnel: "LAB05-1" -> [w2460 w2462]
                              frame #0 {
                                n1520 = call "sub vi - defrag tdms v1.vi"("panel id"=w2460) -> ("error out"=w2459:errorcluster)  [unwired: 10 in]
                                n1521 = local write "data file error"(w2459) -> ()
                              }
                              frame #1 {
                                n1522 = call "Save data file to network drive v1.vi"("panel id"=w2462) -> ("network file save error"=w2461:errorcluster)  [unwired: 9 in, 1 out]
                                n1523 = local write "data file error"(w2461) -> ()
                              }
                            }
                          }
                        }
                      }
                    }
                  }
                }
              }
              frame #9 {
                # "LAB05-2"
                n1524 = local read "run lab05-2"() -> (w2463:bool)
                n1525 = case shown="True" w2463 {
                  frame False {
                  }
                  frame True {
                    n1526 = local read "DISP LAB05-2"() -> (w2470:T4)
                    n1527 = Unbundle(w2470) -> ("CYCLE"=w2466:dbl, "STATUS"=w2471:string)  [unwired: 1 out]
                    n1528 = Not Equal?(x=w2471, y="RUN") -> (x != y?=w2465:bool)
                    n1529 = local read "TDMS LAB05-2"() -> (w2469:refnum<k34>)
                    n1530 = Greater?(x=w2466, y=2.0) -> (0:w2467:bool)
                    n1531 = And(x=w2467, y=w2465) -> (x .and. y?=w2464:bool)
                    n1532 = case shown="True" w2464 {
                      tunnel: w2470 -> [_ w2474]
                      tunnel: w2469 -> [_ w2473]
                      frame False {
                      }
                      frame True {
                        n1533 = stacked-sequence {
                          tunnel: w2474 -> [w2477 _ _]
                          tunnel: w2473 -> [_ w2479 _]
                          frame #0 {
                            w2475 = FALSE
                            n1534 = local write "mail control"("END") -> ()
                            n1535 = Bundle(cluster=w2477) -> (w2478:T4)  [unwired: 3 in]
                            n1536 = local write "RUN LAB05-2"(w2475) -> ()
                            n1537 = local write "O/I  LAB05-2"(w2475) -> ()
                            n1538 = local write "run lab05-2"(w2475) -> ()
                            n1539 = local write "DISP LAB05-2"(w2478) -> ()
                          }
                          frame #1 {
                            n1540 = TDMS Close(11:w2479) -> (0:w2480:errorcluster)  [unwired: 1 in, 1 out]
                            n1541 = local write "data file error"(w2480) -> ()
                          }
                          frame #2 {
                            n1542 = stacked-sequence {
                              tunnel: "LAB05-2" -> [w2483 w2485]
                              frame #0 {
                                n1543 = call "sub vi - defrag tdms v1.vi"("panel id"=w2483) -> ("error out"=w2482:errorcluster)  [unwired: 10 in]
                                n1544 = local write "data file error"(w2482) -> ()
                              }
                              frame #1 {
                                n1545 = call "Save data file to network drive v1.vi"("panel id"=w2485) -> ("network file save error"=w2484:errorcluster)  [unwired: 9 in, 1 out]
                                n1546 = local write "data file error"(w2484) -> ()
                              }
                            }
                          }
                        }
                      }
                    }
                  }
                }
              }
            }
            n1547 = local read "Network Directory"() -> (w2241:path)
            n1548 = global write "Global 1.vi" "Network Drive"(w2241) -> ()
          }
          frame #7 {
            # "disable functions"
            n1549 = stacked-sequence {
              tunnel: w2495 -> [w2509 _ w2565]
              tunnel: w2494 -> [w2504 _ w2564]
              tunnel: w2493 -> [w2503 _ w2563]
              tunnel: w2492 -> [w2501 _ w2562]
              tunnel: w2491 -> [w2502 _ w2561]
              tunnel: w2490 -> [_ w2526 w2560]
              tunnel: w2489 -> [_ w2527 w2559]
              tunnel: w2488 -> [_ w2528 w2558]
              tunnel: w2487 -> [_ w2529 w2557]
              tunnel: w2486 -> [_ w2530 w2556]
              frame #0 {
                n1550 = Select(t=2, s=w2501, f=0) -> (s? t:f=w2497:i32)
                n1551 = Select(t=2, s=w2503, f=0) -> (s? t:f=w2498:i32)
                n1552 = Select(t=2, s=w2502, f=0) -> (s? t:f=w2496:i32)
                n1553 = Select(t=2, s=w2509, f=0) -> (s? t:f=w2500:i32)
                n1554 = Select(t=2, s=w2504, f=0) -> (s? t:f=w2499:i32)
                n1555 = property on="SELECT LAB02-2" class="RadioBtnsControl (strict)"("DisabledEnum"=w2497) -> ()  [unwired: 2 in, 2 out]
                n1556 = property on="SELECT LAB02-1" class="RadioBtnsControl (strict)"("DisabledEnum"=w2498) -> ()  [unwired: 2 in, 2 out]
                n1557 = property on="SELECT LAB03-1" class="RadioBtnsControl (strict)"("DisabledEnum"=w2496) -> ()  [unwired: 2 in, 2 out]
                n1558 = property on="SELECT LAB01-1" class="RadioBtnsControl (strict)"("DisabledEnum"=w2500) -> ()  [unwired: 2 in, 2 out]
                n1559 = property on="SELECT LAB01-2" class="RadioBtnsControl (strict)"("DisabledEnum"=w2499) -> ()  [unwired: 2 in, 2 out]
                n1560 = Not(x=w2509) -> (.not. x?=w2510:bool)
                n1561 = property on="RESULT LAB01-1" class="Bool (strict)"("Visible"=w2510) -> ()  [unwired: 2 in, 2 out]
                n1562 = Not(x=w2504) -> (.not. x?=w2508:bool)
                n1563 = Not(x=w2503) -> (.not. x?=w2507:bool)
                n1564 = Not(x=w2501) -> (.not. x?=w2506:bool)
                n1565 = property on="RESULT LAB01-2" class="Bool (strict)"("Visible"=w2508) -> ()  [unwired: 2 in, 2 out]
                n1566 = Not(x=w2502) -> (.not. x?=w2505:bool)
                n1567 = property on="RESULT LAB02-1" class="Bool (strict)"("Visible"=w2507) -> ()  [unwired: 2 in, 2 out]
                n1568 = property on="RESULT LAB02-2" class="Bool (strict)"("Visible"=w2506) -> ()  [unwired: 2 in, 2 out]
                n1569 = property on="RESULT LAB03-1" class="Bool (strict)"("Visible"=w2505) -> ()  [unwired: 2 in, 2 out]
                n1570 = property on="SET LAB01-1" class="Clust (strict)"("DisabledEnum"=w2500) -> ()  [unwired: 2 in, 2 out]
                n1571 = property on="SET LAB01-2" class="Clust (strict)"("DisabledEnum"=w2499) -> ()  [unwired: 2 in, 2 out]
                n1572 = property on="SET LAB02-1" class="Clust (strict)"("DisabledEnum"=w2498) -> ()  [unwired: 2 in, 2 out]
                n1573 = property on="SET LAB02-2" class="Clust (strict)"("DisabledEnum"=w2497) -> ()  [unwired: 2 in, 2 out]
                n1574 = property on="SET LAB03-1" class="Clust (strict)"("DisabledEnum"=w2496) -> ()  [unwired: 2 in, 2 out]
                n1575 = property on="O/I  LAB01-1" class="Bool (strict)"("DisabledEnum"=w2500) -> ()  [unwired: 2 in, 2 out]
                n1576 = property on="O/I  LAB01-2" class="Bool (strict)"("DisabledEnum"=w2499) -> ()  [unwired: 2 in, 2 out]
                n1577 = property on="O/I  LAB02-1" class="Bool (strict)"("DisabledEnum"=w2498) -> ()  [unwired: 2 in, 2 out]
                n1578 = property on="O/I  LAB02-2" class="Bool (strict)"("DisabledEnum"=w2497) -> ()  [unwired: 2 in, 2 out]
                n1579 = property on="O/I  LAB03-1" class="Bool (strict)"("DisabledEnum"=w2496) -> ()  [unwired: 2 in, 2 out]
              }
              frame #1 {
                n1580 = Select(t=2, s=w2530, f=0) -> (s? t:f=w2521:i32)
                n1581 = Select(t=2, s=w2529, f=0) -> (s? t:f=w2522:i32)
                n1582 = Select(t=2, s=w2526, f=0) -> (s? t:f=w2525:i32)
                n1583 = Select(t=2, s=w2527, f=0) -> (s? t:f=w2524:i32)
                n1584 = Select(t=2, s=w2528, f=0) -> (s? t:f=w2523:i32)
                n1585 = property on="SELECT LAB05-2" class="RadioBtnsControl (strict)"("DisabledEnum"=w2521) -> ()  [unwired: 2 in, 2 out]
                n1586 = property on="SELECT LAB05-1" class="RadioBtnsControl (strict)"("DisabledEnum"=w2522) -> ()  [unwired: 2 in, 2 out]
                n1587 = property on="SELECT LAB03-2" class="RadioBtnsControl (strict)"("DisabledEnum"=w2525) -> ()  [unwired: 2 in, 2 out]
                n1588 = property on="SELECT LAB04-1" class="RadioBtnsControl (strict)"("DisabledEnum"=w2524) -> ()  [unwired: 2 in, 2 out]
                n1589 = property on="SELECT LAB04-2" class="RadioBtnsControl (strict)"("DisabledEnum"=w2523) -> ()  [unwired: 2 in, 2 out]
                n1590 = property on="SET LAB05-2" class="Clust (strict)"("DisabledEnum"=w2521) -> ()  [unwired: 2 in, 2 out]
                n1591 = property on="SET LAB05-1" class="Clust (strict)"("DisabledEnum"=w2522) -> ()  [unwired: 2 in, 2 out]
                n1592 = property on="SET LAB03-2" class="Clust (strict)"("DisabledEnum"=w2525) -> ()  [unwired: 2 in, 2 out]
                n1593 = property on="SET LAB04-1" class="Clust (strict)"("DisabledEnum"=w2524) -> ()  [unwired: 2 in, 2 out]
                n1594 = property on="SET LAB04-2" class="Clust (strict)"("DisabledEnum"=w2523) -> ()  [unwired: 2 in, 2 out]
                n1595 = property on="O/I  LAB05-2" class="Bool (strict)"("DisabledEnum"=w2521) -> ()  [unwired: 2 in, 2 out]
                n1596 = property on="O/I  LAB05-1" class="Bool (strict)"("DisabledEnum"=w2522) -> ()  [unwired: 2 in, 2 out]
                n1597 = property on="O/I  LAB04-1" class="Bool (strict)"("DisabledEnum"=w2524) -> ()  [unwired: 2 in, 2 out]
                n1598 = property on="O/I  LAB04-2" class="Bool (strict)"("DisabledEnum"=w2523) -> ()  [unwired: 2 in, 2 out]
                n1599 = property on="O/I  LAB03-2" class="Bool (strict)"("DisabledEnum"=w2525) -> ()  [unwired: 2 in, 2 out]
                n1600 = Not(x=w2530) -> (.not. x?=w2531:bool)
                n1601 = Not(x=w2529) -> (.not. x?=w2532:bool)
                n1602 = Not(x=w2528) -> (.not. x?=w2533:bool)
                n1603 = property on="RESULT LAB05-2" class="Bool (strict)"("Visible"=w2531) -> ()  [unwired: 2 in, 2 out]
                n1604 = property on="RESULT LAB05-1" class="Bool (strict)"("Visible"=w2532) -> ()  [unwired: 2 in, 2 out]
                n1605 = Not(x=w2527) -> (.not. x?=w2534:bool)
                n1606 = property on="RESULT LAB04-2" class="Bool (strict)"("Visible"=w2533) -> ()  [unwired: 2 in, 2 out]
                n1607 = Not(x=w2526) -> (.not. x?=w2535:bool)
                n1608 = property on="RESULT LAB04-1" class="Bool (strict)"("Visible"=w2534) -> ()  [unwired: 2 in, 2 out]
                n1609 = property on="RESULT LAB03-2" class="Bool (strict)"("Visible"=w2535) -> ()  [unwired: 2 in, 2 out]
              }
              frame #2 {
                # "disable calibrate if any test running"
                n1610 = Or(x=w2557, y=w2556) -> (x .or. y?=w2550:bool)
                n1611 = Or(x=w2559, y=w2558) -> (x .or. y?=w2552:bool)
                n1612 = Or(x=w2563, y=w2562) -> (x .or. y?=w2554:bool)
                n1613 = Or(x=w2561, y=w2560) -> (x .or. y?=w2553:bool)
                n1614 = Or(x=w2565, y=w2564) -> (x .or. y?=w2555:bool)
                n1615 = Or(x=w2553, y=w2552) -> (x .or. y?=w2551:bool)
                n1616 = Or(x=w2555, y=w2554) -> (x .or. y?=w2549:bool)
                n1617 = Or(x=w2551, y=w2550) -> (x .or. y?=w2548:bool)
                n1618 = Or(x=w2549, y=w2548) -> (x .or. y?=w2547:bool)
                n1619 = case shown="True" w2547 {
                  tunnel: [0 2] -> w2546
                  frame False {
                  }
                  frame True {
                  }
                }
                n1620 = property on="JIG TEST" class="Clust (strict)"("DisabledEnum"=w2546) -> ()  [unwired: 2 in, 2 out]
                n1621 = property on="Network Directory" class="Path"("DisabledEnum"=w2546) -> ()  [unwired: 2 in, 2 out]
                n1622 = property on="MAIL SETTINGS" class="Clust (strict)"("DisabledEnum"=w2546) -> ()  [unwired: 2 in, 2 out]
                n1623 = property on="CALIBRATE" class="Bool (strict)"("DisabledEnum"=w2546) -> ()  [unwired: 2 in, 2 out]
                n1624 = property on="ADMIN PAGE" class="Bool (strict)"("DisabledEnum"=w2546) -> ()  [unwired: 2 in, 2 out]
              }
            }
          }
          frame #8 {
            # "drive jigs"
            n1625 = stacked-sequence {
              frame #0 {
                # "jig on"
                n1626 = local read "jig cycle"() -> (w2573:dbl)
                n1627 = property on="JIG TEST" class="Clust (strict)"() -> ("DisabledEnum"=w2570:T15)  [unwired: 2 in, 2 out]
                n1628 = Equal?(x=w2570, y=2) -> (x = y?=w2569:bool)
                n1629 = Equal?(x=w2573, y=0) -> (x = y?=w2571:bool)
                n1630 = And(x=w2571, y=w2569) -> (x .and. y?=w2568:bool)
                n1631 = case shown="True" w2568 {
                  frame False {
                  }
                  frame True {
                    n1632 = local read "run lab01-1"() -> (w2584:bool)
                    n1633 = local read "run lab01-2"() -> (w2583:bool)
                    n1634 = local read "run lab02-1"() -> (w2582:bool)
                    n1635 = local read "run lab02-2"() -> (w2581:bool)
                    n1636 = local read "run lab03-1"() -> (w2580:bool)
                    n1637 = local read "run lab03-2"() -> (w2579:bool)
                    n1638 = local read "run lab04-1"() -> (w2578:bool)
                    n1639 = local read "run lab04-2"() -> (w2577:bool)
                    n1640 = local read "run lab05-1"() -> (w2576:bool)
                    n1641 = local read "run lab05-2"() -> (w2575:bool)
                    n1642 = local write "JIG LAB03-2"(w2579) -> ()
                    n1643 = local write "JIG LAB01-1"(w2584) -> ()
                    n1644 = local write "JIG LAB01-2"(w2583) -> ()
                    n1645 = local write "JIG LAB02-1"(w2582) -> ()
                    n1646 = local write "JIG LAB02-2"(w2581) -> ()
                    n1647 = local write "JIG LAB03-1"(w2580) -> ()
                    n1648 = local write "JIG LAB04-1"(w2578) -> ()
                    n1649 = local write "JIG LAB04-2"(w2577) -> ()
                    n1650 = local write "JIG LAB05-1"(w2576) -> ()
                    n1651 = local write "JIG LAB05-2"(w2575) -> ()
                  }
                }
              }
              frame #1 {
                # "jig off"
                n1652 = local read "jig cycle"() -> (w2591:dbl)
                n1653 = local read "on loops"() -> (w2590:dbl)
                n1654 = property on="JIG TEST" class="Clust (strict)"() -> ("DisabledEnum"=w2589:T15)  [unwired: 2 in, 2 out]
                n1655 = Equal?(x=w2589, y=2) -> (x = y?=w2587:bool)
                n1656 = Equal?(x=w2591, y=w2590) -> (x = y?=w2586:bool)
                n1657 = And(x=w2586, y=w2587) -> (x .and. y?=w2585:bool)
                n1658 = case shown="True" w2585 {
                  frame False {
                  }
                  frame True {
                    w2642 = FALSE
                    w2643 = TRUE
                    w2641 = 2
                    n1659 = local read "SELECT LAB05-2"() -> (w2632:T3)
                    n1660 = local read "SELECT LAB04-2"() -> (w2634:T3)
                    n1661 = local read "SELECT LAB04-1"() -> (w2635:T3)
                    n1662 = local read "SELECT LAB05-1"() -> (w2633:T3)
                    n1663 = local read "SELECT LAB03-2"() -> (w2636:T3)
                    n1664 = local read "SELECT LAB02-1"() -> (w2639:T3)
                    n1665 = local read "SELECT LAB03-1"() -> (w2637:T3)
                    n1666 = local read "SELECT LAB02-2"() -> (w2638:T3)
                    n1667 = local read "SELECT LAB01-2"() -> (w2640:T3)
                    n1668 = local read "run lab05-1"() -> (w2602:bool)
                    n1669 = local read "run lab05-2"() -> (w2601:bool)
                    n1670 = local read "SELECT LAB01-1"() -> (w2644:T3)
                    n1671 = local read "run lab04-2"() -> (w2603:bool)
                    n1672 = local read "run lab04-1"() -> (w2604:bool)
                    n1673 = local read "run lab01-1"() -> (w2620:bool)
                    n1674 = local read "run lab01-2"() -> (w2609:bool)
                    n1675 = local read "run lab03-2"() -> (w2605:bool)
                    n1676 = local read "run lab03-1"() -> (w2606:bool)
                    n1677 = local read "run lab02-1"() -> (w2608:bool)
                    n1678 = local read "run lab02-2"() -> (w2607:bool)
                    n1679 = Equal?(x=w2641, y=w2637) -> (x = y?=w2615:bool)
                    n1680 = Equal?(x=w2641, y=w2636) -> (x = y?=w2614:bool)
                    n1681 = Equal?(x=w2641, y=w2635) -> (x = y?=w2613:bool)
                    n1682 = Equal?(x=w2641, y=w2634) -> (x = y?=w2612:bool)
                    n1683 = Equal?(x=w2641, y=w2633) -> (x = y?=w2611:bool)
                    n1684 = Equal?(x=w2641, y=w2632) -> (x = y?=w2610:bool)
                    n1685 = Equal?(x=w2641, y=w2644) -> (x = y?=w2621:bool)
                    n1686 = Equal?(x=w2641, y=w2639) -> (x = y?=w2617:bool)
                    n1687 = Equal?(x=w2641, y=w2638) -> (x = y?=w2616:bool)
                    n1688 = Equal?(x=w2641, y=w2640) -> (x = y?=w2618:bool)
                    n1689 = And(x=w2612, y=w2603) -> (x .and. y?=w2594:bool)
                    n1690 = And(x=w2615, y=w2606) -> (x .and. y?=w2597:bool)
                    n1691 = And(x=w2613, y=w2604) -> (x .and. y?=w2595:bool)
                    n1692 = And(x=w2610, y=w2601) -> (x .and. y?=w2592:bool)
                    n1693 = And(x=w2616, y=w2607) -> (x .and. y?=w2598:bool)
                    n1694 = And(x=w2614, y=w2605) -> (x .and. y?=w2596:bool)
                    n1695 = And(x=w2611, y=w2602) -> (x .and. y?=w2593:bool)
                    n1696 = And(x=w2618, y=w2609) -> (x .and. y?=w2600:bool)
                    n1697 = And(x=w2621, y=w2620) -> (x .and. y?=w2619:bool)
                    n1698 = And(x=w2617, y=w2608) -> (x .and. y?=w2599:bool)
                    n1699 = Select(t=w2643, s=w2619, f=w2642) -> (s? t:f=w2622:bool)
                    n1700 = Select(t=w2643, s=w2600, f=w2642) -> (s? t:f=w2623:bool)
                    n1701 = Select(t=w2643, s=w2599, f=w2642) -> (s? t:f=w2624:bool)
                    n1702 = Select(t=w2643, s=w2598, f=w2642) -> (s? t:f=w2625:bool)
                    n1703 = Select(t=w2643, s=w2597, f=w2642) -> (s? t:f=w2626:bool)
                    n1704 = Select(t=w2643, s=w2596, f=w2642) -> (s? t:f=w2627:bool)
                    n1705 = Select(t=w2643, s=w2595, f=w2642) -> (s? t:f=w2628:bool)
                    n1706 = Select(t=w2643, s=w2594, f=w2642) -> (s? t:f=w2629:bool)
                    n1707 = Select(t=w2643, s=w2593, f=w2642) -> (s? t:f=w2630:bool)
                    n1708 = Select(t=w2643, s=w2592, f=w2642) -> (s? t:f=w2631:bool)
                    n1709 = local write "JIG LAB03-2"(w2627) -> ()
                    n1710 = local write "JIG LAB02-1"(w2624) -> ()
                    n1711 = local write "JIG LAB02-2"(w2625) -> ()
                    n1712 = local write "JIG LAB01-2"(w2623) -> ()
                    n1713 = local write "JIG LAB03-1"(w2626) -> ()
                    n1714 = local write "JIG LAB01-1"(w2622) -> ()
                    n1715 = local write "JIG LAB05-2"(w2631) -> ()
                    n1716 = local write "JIG LAB04-1"(w2628) -> ()
                    n1717 = local write "JIG LAB05-1"(w2630) -> ()
                    n1718 = local write "JIG LAB04-2"(w2629) -> ()
                  }
                }
              }
            }
          }
          frame #9 {
            # "enable  jig test output if no test busy"
            n1719 = property on="JIG TEST" class="Clust (strict)"() -> ("DisabledEnum"=w2647:T15)  [unwired: 2 in, 2 out]
            n1720 = Equal?(x=w2647, y=0) -> (x = y?=w2645:bool)
            n1721 = case shown="True" w2645 {
              frame False {
              }
              frame True {
                n1722 = local read "JIG TEST"() -> (w2658:T12)
                n1723 = Unbundle(w2658) -> ("LAB01-1"=w2657:bool, "LAB01-2"=w2656:bool, "LAB02-1"=w2655:bool, "LAB02-2"=w2654:bool, "LAB03-1"=w2653:bool, "LAB03-2"=w2652:bool, "LAB04-1"=w2651:bool, "LAB04-2"=w2650:bool, "LAB05-1"=w2649:bool, "LAB05-2"=w2648:bool)
                n1724 = local write "JIG LAB05-1"(w2649) -> ()
                n1725 = local write "JIG LAB05-2"(w2648) -> ()
                n1726 = local write "JIG LAB04-1"(w2651) -> ()
                n1727 = local write "JIG LAB04-2"(w2650) -> ()
                n1728 = local write "JIG LAB03-2"(w2652) -> ()
                n1729 = local write "JIG LAB01-1"(w2657) -> ()
                n1730 = local write "JIG LAB02-1"(w2655) -> ()
                n1731 = local write "JIG LAB03-1"(w2653) -> ()
                n1732 = local write "JIG LAB01-2"(w2656) -> ()
                n1733 = local write "JIG LAB02-2"(w2654) -> ()
              }
            }
          }
          frame #10 {
            # "drive digital output"
            n1734 = local read "O/I  LAB05-2"() -> (w2665:bool)
            n1735 = local read "O/I  LAB05-1"() -> (w2667:bool)
            n1736 = local read "JIG LAB05-2"() -> (w2664:bool)
            n1737 = local read "O/I  LAB04-2"() -> (w2669:bool)
            n1738 = local read "JIG LAB05-1"() -> (w2666:bool)
            n1739 = local read "JIG LAB04-2"() -> (w2668:bool)
            n1740 = local read "O/I  LAB03-1"() -> (w2674:bool)
            n1741 = local read "O/I  LAB04-1"() -> (w2670:bool)
            n1742 = local read "O/I  LAB02-1"() -> (w2678:bool)
            n1743 = local read "O/I  LAB02-2"() -> (w2676:bool)
            n1744 = local read "O/I  LAB03-2"() -> (w2672:bool)
            n1745 = local read "JIG LAB04-1"() -> (w2663:bool)
            n1746 = local read "JIG LAB03-2"() -> (w2671:bool)
            n1747 = local read "O/I  LAB01-2"() -> (w2680:bool)
            n1748 = local read "JIG LAB02-1"() -> (w2677:bool)
            n1749 = local read "JIG LAB02-2"() -> (w2675:bool)
            n1750 = local read "JIG LAB03-1"() -> (w2673:bool)
            n1751 = local read "O/I  LAB01-1"() -> (w2682:bool)
            n1752 = local read "JIG LAB01-2"() -> (w2679:bool)
            n1753 = local read "JIG LAB01-1"() -> (w2681:bool)
            n1754 = Build Array(w2669, w2668, w2667, w2666, w2665, w2664) -> (w2660:bool[])
            n1755 = Build Array(w2675, w2674, w2673, w2672, w2671, w2670, w2663) -> (w2661:bool[])
            n1756 = Build Array(w2682, w2681, w2680, w2679, w2678, w2677, w2676) -> (w2662:bool[])
            n1757 = local read "simulate"() -> (w2659:bool)
            n1758 = case shown="False" w2659 {
              tunnel: w2662 -> [w2685 _]
              tunnel: w2661 -> [w2684 _]
              tunnel: w2660 -> [w2683 _]
              frame False {
                n1759 = call "sub vi - Drive Relays All v6.vi"("Array #2"=w2683, "Array #1"=w2684, "Array #0"=w2685) -> ()  [unwired: 8 in, 1 out]
              }
              frame True {
              }
            }
          }
          frame #11 {
            # "get temperature values"
            n1760 = local read "simulate"() -> (w2687:bool)
            n1761 = stacked-sequence {
              tunnel: w2687 -> [_ w2723 w2747 w2771 w2795 w2819]
              tunnel: T8 {"1  (A) cal"=1.0, "1 (V) cal"=1.0, "1 (PF) cal"=1.0, "1 (TL) cal"=1.0, "1 (TN) cal"=1.0, "2 (A) cal"=1.0, "2 (V) cal"=1.0, "2 (PF) cal"=1.0, "2 (TL) cal"=1.0, "2 (TN) cal"=1.0} ("CAL LAB01") -> [_ w2722 w2746 w2770 w2794 w2818]
              frame #0 {
                n1762 = local read "Select COM port"() -> (w2691:refnum<visa-resource-name>)
                "COM port" <- w2691
                n1763 = local read "jig cycle"() -> (w2692:dbl)
                n1764 = local read "on loops"() -> (w2695:dbl)
                n1765 = local read "jig cycle"() -> (w2697:dbl)
                n1766 = global write "Global 1.vi" "tmp dly lps"("Temp Delay Lps") -> ()
                n1767 = global write "Global 1.vi" "dly value"("Temp Value") -> ()
                n1768 = Add(x=w2695, y=2) -> (x+y=w2696:dbl)
                n1769 = global write "Global 1.vi" "COM port"(w2691) -> ()
                n1770 = Equal?(x=w2697, y=0) -> (x = y?=w2698:bool)
                n1771 = Equal?(x=w2692, y=w2696) -> (x = y?=w2693:bool)
                n1772 = local read "simulate"() -> (w2688:bool)
                n1773 = case shown="True" w2693 {
                  tunnel: w2688 -> [_ w2700]
                  frame False {
                  }
                  frame True {
                    n1774 = case shown="False" w2700 {
                      tunnel: [w2705 w2709] -> w2702
                      tunnel: [w2704 w2709] -> w2701
                      frame False {
                        w2707 = TRUE
                        w2708 = FALSE
                        n1775 = call "sub vi - GET ALL TEMP v4.vi"("LA01-EN"=w2708, "LA02-EN"=w2708, "LA03-EN"=w2708, "LA04-EN"=w2707, "LA05-EN"=w2707, "Gen Cal Value"=1.0) -> ("LA04 TEMP"=w2705:T23, "LA05 TEMP"=w2704:T23)  [unwired: 4 in, 4 out]
                      }
                      frame True {
                        w2709 = T14 {"T1 Live"=21.0, "T1 Neut"=22.0, "T2 Live"=23.0, "T2 Neut"=24.0, "ID"=6.0, "ER"=10.0} ("LAB01 TEMP")
                      }
                    }
                    n1776 = local write "TEMP update"(TRUE) -> ()
                    n1777 = local write "LAB04 TEMP"(w2702) -> ()
                    n1778 = local write "LAB05 TEMP"(w2701) -> ()
                  }
                }
                n1779 = case shown="True" w2698 {
                  tunnel: w2688 -> [_ w2713]
                  frame False {
                  }
                  frame True {
                    n1780 = case shown="False" w2713 {
                      tunnel: [w2717 w2721] -> w2712
                      tunnel: [w2716 w2721] -> w2711
                      tunnel: [w2715 w2721] -> w2710
                      frame False {
                        w2719 = FALSE
                        w2720 = TRUE
                        n1781 = call "sub vi - GET ALL TEMP v4.vi"("LA01-EN"=w2720, "LA02-EN"=w2720, "LA03-EN"=w2720, "LA04-EN"=w2719, "LA05-EN"=w2719, "Gen Cal Value"=1.0) -> ("LA01 TEMP"=w2717:T23, "LA02 TEMP"=w2716:T23, "LA03 TEMP"=w2715:T23)  [unwired: 4 in, 3 out]
                      }
                      frame True {
                        w2721 = T14 {"T1 Live"=21.0, "T1 Neut"=22.0, "T2 Live"=23.0, "T2 Neut"=24.0, "ID"=6.0, "ER"=10.0} ("LAB01 TEMP")
                      }
                    }
                    n1782 = local write "TEMP update"(TRUE) -> ()
                    n1783 = local write "LAB03 TEMP"(w2710) -> ()
                    n1784 = local write "LAB02 TEMP"(w2711) -> ()
                    n1785 = local write "LAB01 TEMP"(w2712) -> ()
                  }
                }
              }
              frame #1 {
                n1786 = case shown="False" w2723 {
                  tunnel: [w2744 w2745] -> w2743
                  tunnel: w2722 -> [_ w2745]
                  frame False {
                    n1787 = local read "CAL LAB01"() -> (w2744:T8)
                  }
                  frame True {
                  }
                }
                n1788 = local read "LAB01 TEMP"() -> (w2729:T14)
                n1789 = local read "TEMP LA01"() -> (w2730:T11)
                n1790 = call "sub vi - temperature delay v2.vi"("temp values IN"=w2730, "temp signals"=w2729) -> ("T2-N"=w2725:dbl, "T2-L"=w2726:dbl, "T1-N"=w2727:dbl, "T1-L"=w2728:dbl, "temp values OUT"=w2724:T24)  [unwired: 5 in]
                n1791 = Unbundle By Name(w2743) -> ("1 (TL) cal"=w2734:dbl, "1 (TN) cal"=w2733:dbl, "2 (TL) cal"=w2732:dbl, "2 (TN) cal"=w2731:dbl)  [unwired: 6 out]
                n1792 = local write "TEMP LA01"(w2724) -> ()
                n1793 = Multiply(x=w2728, y=w2734) -> (x*y=w2740:dbl)
                n1794 = Multiply(x=w2727, y=w2733) -> (x*y=w2739:dbl)
                n1795 = Multiply(x=w2726, y=w2732) -> (x*y=w2736:dbl)
                n1796 = Multiply(x=w2725, y=w2731) -> (x*y=w2735:dbl)
                n1797 = local read "SIG LAB01-2"() -> (w2738:T2)
                n1798 = local read "SIG LAB01-1"() -> (w2742:T2)
                n1799 = Bundle By Name(cluster=w2742, "Tmp Live"=w2740, "Tmp Neut"=w2739) -> (w2741:T2)
                n1800 = Bundle By Name(cluster=w2738, "Tmp Live"=w2736, "Tmp Neut"=w2735) -> (w2737:T2)
                n1801 = local write "SIG LAB01-1"(w2741) -> ()
                n1802 = local write "SIG LAB01-2"(w2737) -> ()
              }
              frame #2 {
                n1803 = case shown="True" w2747 {
                  tunnel: [w2768 w2769] -> w2767
                  tunnel: w2746 -> [_ w2769]
                  frame False {
                    n1804 = local read "CAL LAB02"() -> (w2768:T9)
                  }
                  frame True {
                  }
                }
                n1805 = local read "LAB02 TEMP"() -> (w2754:T14)
                n1806 = local read "TEMP LA02"() -> (w2753:T11)
                n1807 = call "sub vi - temperature delay v2.vi"("temp values IN"=w2753, "temp signals"=w2754) -> ("T2-N"=w2748:dbl, "T2-L"=w2749:dbl, "T1-N"=w2750:dbl, "T1-L"=w2751:dbl, "temp values OUT"=w2752:T24)  [unwired: 5 in]
                n1808 = Unbundle By Name(w2767) -> ("1 (TL) cal"=w2758:dbl, "1 (TN) cal"=w2757:dbl, "2 (TL) cal"=w2756:dbl, "2 (TN) cal"=w2755:dbl)  [unwired: 6 out]
                n1809 = local write "TEMP LA02"(w2752) -> ()
                n1810 = Multiply(x=w2751, y=w2758) -> (x*y=w2764:dbl)
                n1811 = Multiply(x=w2750, y=w2757) -> (x*y=w2763:dbl)
                n1812 = Multiply(x=w2749, y=w2756) -> (x*y=w2760:dbl)
                n1813 = Multiply(x=w2748, y=w2755) -> (x*y=w2759:dbl)
                n1814 = local read "SIG LAB02-2"() -> (w2762:T2)
                n1815 = local read "SIG LAB02-1"() -> (w2766:T2)
                n1816 = Bundle By Name(cluster=w2766, "Tmp Live"=w2764, "Tmp Neut"=w2763) -> (w2765:T2)
                n1817 = Bundle By Name(cluster=w2762, "Tmp Live"=w2760, "Tmp Neut"=w2759) -> (w2761:T2)
                n1818 = local write "SIG LAB02-1"(w2765) -> ()
                n1819 = local write "SIG LAB02-2"(w2761) -> ()
              }
              frame #3 {
                n1820 = case shown="False" w2771 {
                  tunnel: [w2792 w2793] -> w2791
                  tunnel: w2770 -> [_ w2793]
                  frame False {
                    n1821 = local read "CAL LAB03"() -> (w2792:T8)
                  }
                  frame True {
                  }
                }
                n1822 = local read "TEMP LA03"() -> (w2777:T11)
                n1823 = local read "LAB03 TEMP"() -> (w2778:T14)
                n1824 = call "sub vi - temperature delay v2.vi"("temp values IN"=w2777, "temp signals"=w2778) -> ("T2-N"=w2772:dbl, "T2-L"=w2773:dbl, "T1-N"=w2774:dbl, "T1-L"=w2775:dbl, "temp values OUT"=w2776:T24)  [unwired: 5 in]
                n1825 = Unbundle By Name(w2791) -> ("1 (TL) cal"=w2782:dbl, "1 (TN) cal"=w2781:dbl, "2 (TL) cal"=w2780:dbl, "2 (TN) cal"=w2779:dbl)  [unwired: 6 out]
                n1826 = local write "TEMP LA03"(w2776) -> ()
                n1827 = Multiply(x=w2775, y=w2782) -> (x*y=w2788:dbl)
                n1828 = Multiply(x=w2774, y=w2781) -> (x*y=w2787:dbl)
                n1829 = Multiply(x=w2773, y=w2780) -> (x*y=w2784:dbl)
                n1830 = Multiply(x=w2772, y=w2779) -> (x*y=w2783:dbl)
                n1831 = local read "SIG LAB03-2"() -> (w2786:T2)
                n1832 = local read "SIG LAB03-1"() -> (w2790:T2)
                n1833 = Bundle By Name(cluster=w2790, "Tmp Live"=w2788, "Tmp Neut"=w2787) -> (w2789:T2)
                n1834 = Bundle By Name(cluster=w2786, "Tmp Live"=w2784, "Tmp Neut"=w2783) -> (w2785:T2)
                n1835 = local write "SIG LAB03-1"(w2789) -> ()
                n1836 = local write "SIG LAB03-2"(w2785) -> ()
              }
              frame #4 {
                n1837 = case shown="False" w2795 {
                  tunnel: [w2816 w2817] -> w2815
                  tunnel: w2794 -> [_ w2817]
                  frame False {
                    n1838 = local read "CAL LAB04"() -> (w2816:T8)
                  }
                  frame True {
                  }
                }
                n1839 = local read "LAB04 TEMP"() -> (w2801:T14)
                n1840 = local read "TEMP LA04"() -> (w2802:T11)
                n1841 = call "sub vi - temperature delay v2.vi"("temp values IN"=w2802, "temp signals"=w2801) -> ("T2-N"=w2796:dbl, "T2-L"=w2797:dbl, "T1-N"=w2798:dbl, "T1-L"=w2799:dbl, "temp values OUT"=w2800:T24)  [unwired: 5 in]
                n1842 = Unbundle By Name(w2815) -> ("1 (TL) cal"=w2806:dbl, "1 (TN) cal"=w2805:dbl, "2 (TL) cal"=w2804:dbl, "2 (TN) cal"=w2803:dbl)  [unwired: 6 out]
                n1843 = local write "TEMP LA04"(w2800) -> ()
                n1844 = Multiply(x=w2799, y=w2806) -> (x*y=w2812:dbl)
                n1845 = Multiply(x=w2798, y=w2805) -> (x*y=w2811:dbl)
                n1846 = Multiply(x=w2797, y=w2804) -> (x*y=w2808:dbl)
                n1847 = Multiply(x=w2796, y=w2803) -> (x*y=w2807:dbl)
                n1848 = local read "SIG LAB04-2"() -> (w2810:T2)
                n1849 = local read "SIG LAB04-1"() -> (w2814:T2)
                n1850 = Bundle By Name(cluster=w2814, "Tmp Live"=w2812, "Tmp Neut"=w2811) -> (w2813:T2)
                n1851 = Bundle By Name(cluster=w2810, "Tmp Live"=w2808, "Tmp Neut"=w2807) -> (w2809:T2)
                n1852 = local write "SIG LAB04-1"(w2813) -> ()
                n1853 = local write "SIG LAB04-2"(w2809) -> ()
              }
              frame #5 {
                n1854 = case shown="False" w2819 {
                  tunnel: [w2840 w2841] -> w2839
                  tunnel: w2818 -> [_ w2841]
                  frame False {
                    n1855 = local read "CAL LAB05"() -> (w2840:T8)
                  }
                  frame True {
                  }
                }
                n1856 = local read "LAB05 TEMP"() -> (w2825:T14)
                n1857 = local read "TEMP LA05"() -> (w2826:T11)
                n1858 = call "sub vi - temperature delay v2.vi"("temp values IN"=w2826, "temp signals"=w2825) -> ("T2-N"=w2821:dbl, "T2-L"=w2822:dbl, "T1-N"=w2823:dbl, "T1-L"=w2824:dbl, "temp values OUT"=w2820:T24)  [unwired: 5 in]
                n1859 = local write "TEMP LA05"(w2820) -> ()
                n1860 = Unbundle By Name(w2839) -> ("1 (TL) cal"=w2827:dbl, "1 (TN) cal"=w2830:dbl, "2 (TL) cal"=w2829:dbl, "2 (TN) cal"=w2828:dbl)  [unwired: 6 out]
                n1861 = Multiply(x=w2824, y=w2827) -> (x*y=w2836:dbl)
                n1862 = Multiply(x=w2823, y=w2830) -> (x*y=w2835:dbl)
                n1863 = Multiply(x=w2822, y=w2829) -> (x*y=w2832:dbl)
                n1864 = Multiply(x=w2821, y=w2828) -> (x*y=w2831:dbl)
                n1865 = local read "SIG LAB05-2"() -> (w2834:T2)
                n1866 = local read "SIG LAB05-1"() -> (w2838:T2)
                n1867 = Bundle By Name(cluster=w2838, "Tmp Live"=w2836, "Tmp Neut"=w2835) -> (w2837:T2)
                n1868 = Bundle By Name(cluster=w2834, "Tmp Live"=w2832, "Tmp Neut"=w2831) -> (w2833:T2)
                n1869 = local write "SIG LAB05-1"(w2837) -> ()
                n1870 = local write "SIG LAB05-2"(w2833) -> ()
              }
            }
          }
          frame #12 {
            # "get analog values"
            n1871 = local read "on loops"() -> (w2848:dbl)
            n1872 = local read "jig cycle"() -> (w2845:dbl)
            n1873 = Add(x=w2848, y=1) -> (x+y=w2846:dbl)
            n1874 = Equal?(x=w2845, y=1) -> (x = y?=w2843:bool)
            n1875 = Equal?(x=w2845, y=w2846) -> (x = y?=w2844:bool)
            n1876 = Or(x=w2843, y=w2844) -> (x .or. y?=w2842:bool)
            n1877 = case shown="True" w2842 {
              frame False {
              }
              frame True {
                n1878 = local read "simulate"() -> (w2852:bool)
                n1879 = case shown="False" w2852 {
                  tunnel: [w2868 errorcluster[] [] ("array ERROR")] -> w2860
                  tunnel: [w2867 0.3 ("Analog loop time")] -> w2859
                  tunnel: [w2866 dynamicdata[] [] ("array GRAPH")] -> w2858
                  tunnel: [w2865 w2870] -> w2857
                  tunnel: [w2864 w2870] -> w2856
                  tunnel: [w2863 w2870] -> w2855
                  tunnel: [w2862 w2870] -> w2854
                  tunnel: [w2861 w2870] -> w2853
                  frame False {
                    n1880 = call "sub vi - Read Analog All v8.vi"() -> ("Analog loop time"=w2867:dbl, "array GRAPH"=w2866:dynamicdata[], "LAB01"=w2865:T25, "LAB02"=w2864:T26, "LAB03"=w2863:T27, "LAB04"=w2862:T28, "array ERROR"=w2868:errorcluster[], "LAB05"=w2861:T29)  [unwired: 8 in]
                  }
                  frame True {
                    w2870 = T29 {"LAB05-1 (A)"=10.0, "LAB05-1 (V)"=220.0, "LAB05-1 (PF)"=0.5, "LAB05-2 (A)"=15.0, "LAB05-2 (V)"=225.0, "LAB05-2 (PF)"=0.6} ("LAB05")
                  }
                }
                n1881 = local read "simulate"() -> (w2851:bool)
                n1882 = stacked-sequence {
                  tunnel: w2860 -> [w2877 _ _ _ _ _]
                  tunnel: w2859 -> [w2876 _ _ _ _ _]
                  tunnel: w2858 -> [w2875 _ _ _ _ _]
                  tunnel: w2857 -> [_ w2924 _ _ _ _]
                  tunnel: w2856 -> [_ _ w2929 _ _ _]
                  tunnel: w2855 -> [_ _ _ w2958 _ _]
                  tunnel: w2854 -> [_ _ _ _ w2985 _]
                  tunnel: w2853 -> [_ _ _ _ _ w3014]
                  tunnel: w2851 -> [_ w2900 w2928 w2956 w2984 w3012]
                  tunnel: T8 {"1  (A) cal"=1.0, "1 (V) cal"=1.0, "1 (PF) cal"=1.0, "1 (TL) cal"=1.0, "1 (TN) cal"=1.0, "2 (A) cal"=1.0, "2 (V) cal"=1.0, "2 (PF) cal"=1.0, "2 (TL) cal"=1.0, "2 (TN) cal"=1.0} ("CAL LAB01") -> [_ w2899 w2927 w2955 w2983 w3011]
                  frame #0 {
                    n1883 = local write "AI update"(TRUE) -> ()
                    n1884 = global write "Global 1.vi" "RATE(Hz)"("RATE (Hz)") -> ()
                    n1885 = global write "Global 1.vi" "SAMPLES"("SAMPLES") -> ()
                    n1886 = Index Array(array=w2875, index=6) -> (element=→"LAB04-1 (GRAPH)":dynamicdata)
                    n1887 = Index Array(array=w2875, index=7) -> (element=→"LAB04-2 (GRAPH)":dynamicdata)
                    n1888 = Index Array(array=w2875, index=9) -> (element=→"LAB05-2 (GRAPH)":dynamicdata)
                    n1889 = Index Array(array=w2875, index=8) -> (element=→"LAB05-1 (GRAPH)":dynamicdata)
                    n1890 = Index Array(array=w2875, index=5) -> (element=→"LAB03-2 (GRAPH)":dynamicdata)
                    n1891 = Index Array(array=w2875, index=0) -> (element=→"LAB01-1 (GRAPH)":dynamicdata)
                    n1892 = Index Array(array=w2875, index=1) -> (element=→"LAB01-2 (GRAPH)":dynamicdata)
                    n1893 = Index Array(array=w2875, index=2) -> (element=→"LAB02-1 (GRAPH)":dynamicdata)
                    n1894 = Index Array(array=w2875, index=3) -> (element=→"LAB02-2 (GRAPH)":dynamicdata)
                    n1895 = Index Array(array=w2875, index=4) -> (element=→"LAB03-1 (GRAPH)":dynamicdata)
                    "AI loop time" <- w2876
                    "Analog Error Array" <- w2877
                  }
                  frame #1 {
                    n1896 = Unbundle By Name(w2924) -> ("LAB05-1 (A)"=w2922:dbl, "LAB05-1 (V)"=w2921:dbl, "LAB05-1 (PF)"=w2920:dbl, "LAB05-2 (A)"=w2919:dbl, "LAB05-2 (V)"=w2918:dbl, "LAB05-2 (PF)"=w2917:dbl)
                    n1897 = case shown="False" w2900 {
                      tunnel: [w2925 w2926] -> w2923
                      tunnel: w2899 -> [_ w2926]
                      frame False {
                        n1898 = local read "CAL LAB01"() -> (w2925:T8)
                      }
                      frame True {
                      }
                    }
                    n1899 = Unbundle By Name(w2923) -> ("1  (A) cal"=w2916:dbl, "1 (V) cal"=w2915:dbl, "1 (PF) cal"=w2914:dbl, "2 (A) cal"=w2913:dbl, "2 (V) cal"=w2912:dbl, "2 (PF) cal"=w2911:dbl)  [unwired: 4 out]
                    n1900 = Multiply(x=w2922, y=w2916) -> (x*y=w2909:dbl)
                    n1901 = Multiply(x=w2921, y=w2915) -> (x*y=w2908:dbl)
                    n1902 = Multiply(x=w2920, y=w2914) -> (x*y=w2907:dbl)
                    n1903 = Multiply(x=w2919, y=w2913) -> (x*y=w2903:dbl)
                    n1904 = Multiply(x=w2918, y=w2912) -> (x*y=w2902:dbl)
                    n1905 = Multiply(x=w2917, y=w2911) -> (x*y=w2901:dbl)
                    n1906 = local read "SIG LAB01-1"() -> (w2910:T2)
                    n1907 = local read "SIG LAB01-2"() -> (w2905:T2)
                    n1908 = Bundle By Name(cluster=w2910, "AMPS"=w2909, "VOLTS"=w2908, "PF"=w2907) -> (w2906:T2)
                    n1909 = Bundle By Name(cluster=w2905, "AMPS"=w2903, "VOLTS"=w2902, "PF"=w2901) -> (w2904:T2)
                    n1910 = local write "SIG LAB01-2"(w2904) -> ()
                    n1911 = local write "SIG LAB01-1"(w2906) -> ()
                  }
                  frame #2 {
                    n1912 = Unbundle By Name(w2929) -> ("LAB05-1 (A)"=w2951:dbl, "LAB05-1 (V)"=w2950:dbl, "LAB05-1 (PF)"=w2949:dbl, "LAB05-2 (A)"=w2948:dbl, "LAB05-2 (V)"=w2947:dbl, "LAB05-2 (PF)"=w2946:dbl)
                    n1913 = case shown="True" w2928 {
                      tunnel: [w2953 w2954] -> w2952
                      tunnel: w2927 -> [_ w2954]
                      frame False {
                        n1914 = local read "CAL LAB02"() -> (w2953:T9)
                      }
                      frame True {
                      }
                    }
                    n1915 = Unbundle By Name(w2952) -> ("1  (A) cal"=w2945:dbl, "1 (V) cal"=w2944:dbl, "1 (PF) cal"=w2943:dbl, "2 (A) cal"=w2942:dbl, "2 (V) cal"=w2941:dbl, "2 (PF) cal"=w2940:dbl)  [unwired: 4 out]
                    n1916 = Multiply(x=w2951, y=w2945) -> (x*y=w2938:dbl)
                    n1917 = Multiply(x=w2950, y=w2944) -> (x*y=w2937:dbl)
                    n1918 = Multiply(x=w2949, y=w2943) -> (x*y=w2936:dbl)
                    n1919 = Multiply(x=w2948, y=w2942) -> (x*y=w2932:dbl)
                    n1920 = Multiply(x=w2947, y=w2941) -> (x*y=w2931:dbl)
                    n1921 = Multiply(x=w2946, y=w2940) -> (x*y=w2930:dbl)
                    n1922 = local read "SIG LAB02-1"() -> (w2939:T2)
                    n1923 = local read "SIG LAB02-2"() -> (w2934:T2)
                    n1924 = Bundle By Name(cluster=w2939, "AMPS"=w2938, "VOLTS"=w2937, "PF"=w2936) -> (w2935:T2)
                    n1925 = Bundle By Name(cluster=w2934, "AMPS"=w2932, "VOLTS"=w2931, "PF"=w2930) -> (w2933:T2)
                    n1926 = local write "SIG LAB02-2"(w2933) -> ()
                    n1927 = local write "SIG LAB02-1"(w2935) -> ()
                  }
                  frame #3 {
                    n1928 = Unbundle By Name(w2958) -> ("LAB05-1 (A)"=w2979:dbl, "LAB05-1 (V)"=w2978:dbl, "LAB05-1 (PF)"=w2977:dbl, "LAB05-2 (A)"=w2976:dbl, "LAB05-2 (V)"=w2975:dbl, "LAB05-2 (PF)"=w2974:dbl)
                    n1929 = case shown="True" w2956 {
                      tunnel: [w2981 w2982] -> w2980
                      tunnel: w2955 -> [_ w2982]
                      frame False {
                        n1930 = local read "CAL LAB03"() -> (w2981:T8)
                      }
                      frame True {
                      }
                    }
                    n1931 = Unbundle By Name(w2980) -> ("1  (A) cal"=w2973:dbl, "1 (V) cal"=w2972:dbl, "1 (PF) cal"=w2971:dbl, "2 (A) cal"=w2970:dbl, "2 (V) cal"=w2969:dbl, "2 (PF) cal"=w2968:dbl)  [unwired: 4 out]
                    n1932 = Multiply(x=w2979, y=w2973) -> (x*y=w2966:dbl)
                    n1933 = Multiply(x=w2978, y=w2972) -> (x*y=w2957:dbl)
                    n1934 = Multiply(x=w2977, y=w2971) -> (x*y=w2965:dbl)
                    n1935 = Multiply(x=w2976, y=w2970) -> (x*y=w2961:dbl)
                    n1936 = Multiply(x=w2975, y=w2969) -> (x*y=w2960:dbl)
                    n1937 = Multiply(x=w2974, y=w2968) -> (x*y=w2959:dbl)
                    n1938 = local read "SIG LAB03-1"() -> (w2967:T2)
                    n1939 = local read "SIG LAB03-2"() -> (w2963:T2)
                    n1940 = Bundle By Name(cluster=w2967, "AMPS"=w2966, "VOLTS"=w2957, "PF"=w2965) -> (w2964:T2)
                    n1941 = Bundle By Name(cluster=w2963, "AMPS"=w2961, "VOLTS"=w2960, "PF"=w2959) -> (w2962:T2)
                    n1942 = local write "SIG LAB03-2"(w2962) -> ()
                    n1943 = local write "SIG LAB03-1"(w2964) -> ()
                  }
                  frame #4 {
                    n1944 = Unbundle By Name(w2985) -> ("LAB05-1 (A)"=w3007:dbl, "LAB05-1 (V)"=w3006:dbl, "LAB05-1 (PF)"=w3005:dbl, "LAB05-2 (A)"=w3004:dbl, "LAB05-2 (V)"=w3003:dbl, "LAB05-2 (PF)"=w3002:dbl)
                    n1945 = case shown="False" w2984 {
                      tunnel: [w3009 w3010] -> w3008
                      tunnel: w2983 -> [_ w3010]
                      frame False {
                        n1946 = local read "CAL LAB04"() -> (w3009:T8)
                      }
                      frame True {
                      }
                    }
                    n1947 = Unbundle By Name(w3008) -> ("1  (A) cal"=w3001:dbl, "1 (V) cal"=w3000:dbl, "1 (PF) cal"=w2999:dbl, "2 (A) cal"=w2998:dbl, "2 (V) cal"=w2997:dbl, "2 (PF) cal"=w2996:dbl)  [unwired: 4 out]
                    n1948 = Multiply(x=w3007, y=w3001) -> (x*y=w2994:dbl)
                    n1949 = Multiply(x=w3006, y=w3000) -> (x*y=w2993:dbl)
                    n1950 = Multiply(x=w3005, y=w2999) -> (x*y=w2992:dbl)
                    n1951 = Multiply(x=w3004, y=w2998) -> (x*y=w2988:dbl)
                    n1952 = Multiply(x=w3003, y=w2997) -> (x*y=w2987:dbl)
                    n1953 = Multiply(x=w3002, y=w2996) -> (x*y=w2986:dbl)
                    n1954 = local read "SIG LAB04-1"() -> (w2995:T2)
                    n1955 = local read "SIG LAB04-2"() -> (w2990:T2)
                    n1956 = Bundle By Name(cluster=w2995, "AMPS"=w2994, "VOLTS"=w2993, "PF"=w2992) -> (w2991:T2)
                    n1957 = Bundle By Name(cluster=w2990, "AMPS"=w2988, "VOLTS"=w2987, "PF"=w2986) -> (w2989:T2)
                    n1958 = local write "SIG LAB04-2"(w2989) -> ()
                    n1959 = local write "SIG LAB04-1"(w2991) -> ()
                  }
                  frame #5 {
                    n1960 = Unbundle By Name(w3014) -> ("LAB05-1 (A)"=w3035:dbl, "LAB05-1 (V)"=w3013:dbl, "LAB05-1 (PF)"=w3034:dbl, "LAB05-2 (A)"=w3033:dbl, "LAB05-2 (V)"=w3032:dbl, "LAB05-2 (PF)"=w3031:dbl)
                    n1961 = case shown="False" w3012 {
                      tunnel: [w3037 w3038] -> w3036
                      tunnel: w3011 -> [_ w3038]
                      frame False {
                        n1962 = local read "CAL LAB05"() -> (w3037:T8)
                      }
                      frame True {
                      }
                    }
                    n1963 = Unbundle By Name(w3036) -> ("1  (A) cal"=w3030:dbl, "1 (V) cal"=w3029:dbl, "1 (PF) cal"=w3028:dbl, "2 (A) cal"=w3027:dbl, "2 (V) cal"=w3026:dbl, "2 (PF) cal"=w3025:dbl)  [unwired: 4 out]
                    n1964 = Multiply(x=w3035, y=w3030) -> (x*y=w3023:dbl)
                    n1965 = Multiply(x=w3013, y=w3029) -> (x*y=w3022:dbl)
                    n1966 = Multiply(x=w3034, y=w3028) -> (x*y=w3021:dbl)
                    n1967 = Multiply(x=w3033, y=w3027) -> (x*y=w3017:dbl)
                    n1968 = Multiply(x=w3032, y=w3026) -> (x*y=w3016:dbl)
                    n1969 = Multiply(x=w3031, y=w3025) -> (x*y=w3015:dbl)
                    n1970 = local read "SIG LAB05-1"() -> (w3024:T2)
                    n1971 = local read "SIG LAB05-2"() -> (w3019:T2)
                    n1972 = Bundle By Name(cluster=w3024, "AMPS"=w3023, "VOLTS"=w3022, "PF"=w3021) -> (w3020:T2)
                    n1973 = Bundle By Name(cluster=w3019, "AMPS"=w3017, "VOLTS"=w3016, "PF"=w3015) -> (w3018:T2)
                    n1974 = local write "SIG LAB05-2"(w3018) -> ()
                    n1975 = local write "SIG LAB05-1"(w3020) -> ()
                  }
                }
              }
            }
          }
          frame #13 {
            # "save test data to file"
            n1976 = Get Date/Time In Seconds() -> (seconds since 1Jan1904=w3039:timestamp)
            "File Time Stamp" <- w3039
            n1977 = local read "on loops"() -> (w3058:dbl)
            n1978 = local read "jig cycle"() -> (w3055:dbl)
            n1979 = Format Date/Time String(time format string (%c)="%H:%M%:%S", seconds (now)=w3039) -> (date/time string=w3043:string)  [unwired: 1 in]
            n1980 = Add(x=w3058, y=2) -> (x+y=w3056:dbl)
            n1981 = Build Array(w3043) -> (w3042:string[])
            n1982 = Equal?(x=w3055, y=1) -> (x = y?=w3041:bool)
            n1983 = Equal?(x=w3055, y=w3056) -> (x = y?=w3040:bool)
            n1984 = stacked-sequence {
              tunnel: w3054 -> [w3064 _ _ _ _ _ _ _ _ _]
              tunnel: w3053 -> [_ w3140 _ _ _ _ _ _ _ _]
              tunnel: w3052 -> [_ _ w3220 _ _ _ _ _ _ _]
              tunnel: w3051 -> [_ _ _ w3300 _ _ _ _ _ _]
              tunnel: w3050 -> [_ _ _ _ w3380 _ _ _ _ _]
              tunnel: w3049 -> [_ _ _ _ _ w3460 _ _ _ _]
              tunnel: w3048 -> [_ _ _ _ _ _ w3540 _ _ _]
              tunnel: w3047 -> [_ _ _ _ _ _ _ w3620 _ _]
              tunnel: w3046 -> [_ _ _ _ _ _ _ _ w3700 _]
              tunnel: w3045 -> [_ _ _ _ _ _ _ _ _ w3780]
              tunnel: w3042 -> [w3063 w3144 w3224 w3304 w3384 w3464 w3544 w3624 w3704 w3784]
              tunnel: w3041 -> [w3062 w3143 w3223 w3303 w3383 w3463 w3543 w3623 w3703 w3783]
              tunnel: w3040 -> [w3061 w3142 w3222 w3302 w3382 w3462 w3542 w3622 w3702 w3782]
              tunnel: w3039 -> [w3060 w3141 w3221 w3301 w3381 w3461 w3541 w3621 w3701 w3781]
              frame #0 {
                n1985 = case shown="True" w3064 {
                  tunnel: w3063 -> [_ w3069]
                  tunnel: w3062 -> [_ w3068]
                  tunnel: w3061 -> [_ w3066]
                  tunnel: w3060 -> [_ w3065]
                  frame False {
                  }
                  frame True {
                    n1986 = local read "DISP LAB01-1"() -> (w3070:T4)
                    n1987 = local read "SIG LAB01-1"() -> (w3071:T2)
                    n1988 = local read "ON L01-1"() -> (w3067:cluster{"amps":dbl, "volts":dbl, "pf":dbl})
                    n1989 = Unbundle(w3071) -> ("AMPS"=w3077:dbl, "VOLTS"=w3075:dbl, "PF"=w3074:dbl, "Tmp Live"=w3073:dbl, "Tmp Neut"=w3076:dbl)
                    n1990 = Unbundle(w3070) -> ("CYCLE"=w3072:dbl)  [unwired: 2 out]
                    n1991 = stacked-sequence {
                      tunnel: w3077 -> [w3081 w3100]
                      tunnel: w3076 -> [_ w3099]
                      tunnel: w3075 -> [w3080 w3098]
                      tunnel: w3074 -> [w3079 w3097]
                      tunnel: w3073 -> [_ w3096]
                      tunnel: w3072 -> [_ w3095]
                      tunnel: w3069 -> [_ w3094]
                      tunnel: w3068 -> [w3082 _]
                      tunnel: w3067 -> [w3078 w3092]
                      tunnel: w3066 -> [_ w3093]
                      tunnel: w3065 -> [_ w3088]
                      frame #0 {
                        n1992 = case shown="True" w3082 {
                          tunnel: w3081 -> [_ w3087]
                          tunnel: w3080 -> [_ w3086]
                          tunnel: w3079 -> [_ w3085]
                          tunnel: w3078 -> [_ w3083]
                          frame False {
                          }
                          frame True {
                            n1993 = Bundle(cluster=w3083, "amps"=w3087, "volts"=w3086, "pf"=w3085) -> (w3084:cluster{"amps":dbl, "volts":dbl, "pf":dbl})
                            n1994 = local write "ON L01-1"(w3084) -> ()
                          }
                        }
                      }
                      frame #1 {
                        n1995 = Unbundle(w3092) -> ("amps"=w3091:dbl, "volts"=w3090:dbl, "pf"=w3089:dbl)
                        n1996 = case shown="True" w3093 {
                          tunnel: w3100 -> [_ w3101]
                          tunnel: w3099 -> [_ w3139]
                          tunnel: w3098 -> [_ _]
                          tunnel: w3097 -> [_ _]
                          tunnel: w3096 -> [_ w3138]
                          tunnel: w3095 -> [_ w3137]
                          tunnel: w3094 -> [_ w3105]
                          tunnel: w3091 -> [_ w3102]
                          tunnel: w3090 -> [_ w3134]
                          tunnel: w3089 -> [_ w3133]
                          tunnel: w3088 -> [_ w3103]
                          frame False {
                          }
                          frame True {
                            n1997 = local read "TDMS LAB01-1"() -> (w3136:refnum<k34>)
                            n1998 = Build Array(w3134) -> (w3130:dbl[])
                            n1999 = Build Array(w3133) -> (w3129:dbl[])
                            n2000 = Build Array(w3138) -> (w3128:dbl[])
                            n2001 = Build Array(w3139) -> (w3127:dbl[])
                            n2002 = Build Array(w3102) -> (w3132:dbl[])
                            n2003 = Build Array(w3101) -> (w3131:dbl[])
                            n2004 = Build Array(w3137) -> (w3126:dbl[])
                            n2005 = Build Array("AMPS ON", "AMPS OFF", "VOLTS", "PF", "TEMP Live", "TEMP Neut", "CYCLE") -> (w3110:string[])
                            n2006 = Bundle By Name("Y"=w3132, "t0"=w3103) -> (w3125:waveform(dbl))  [unwired: 1 in]
                            n2007 = Bundle By Name("Y"=w3131, "t0"=w3103) -> (w3124:waveform(dbl))  [unwired: 1 in]
                            n2008 = Bundle By Name("Y"=w3130, "t0"=w3103) -> (w3123:waveform(dbl))  [unwired: 1 in]
                            n2009 = Bundle By Name("Y"=w3129, "t0"=w3103) -> (w3122:waveform(dbl))  [unwired: 1 in]
                            n2010 = Bundle By Name("Y"=w3128, "t0"=w3103) -> (w3121:waveform(dbl))  [unwired: 1 in]
                            n2011 = Bundle By Name("Y"=w3127, "t0"=w3103) -> (w3120:waveform(dbl))  [unwired: 1 in]
                            n2012 = Bundle By Name("Y"=w3126, "t0"=w3103) -> (w3119:waveform(dbl))  [unwired: 1 in]
                            n2013 = Build Array(w3125, w3124, w3123, w3122, w3121, w3120, w3119) -> (w3118:waveform(dbl)[])
                            n2014 = TDMS Write(0:w3136, 5:"TEST VALUES", 7:w3110, 9:w3118) -> (4:w3109:refnum<k34>, 6:w3108:string, 15:w3107:errorcluster)  [unwired: 2 in, 1 out]
                            n2015 = TDMS Write(0:w3109, 5:w3108, 7:"TIME", 9:w3105, 11:w3107) -> (15:w3104:errorcluster)  [unwired: 1 in, 3 out]
                            n2016 = local write "data file error"(w3104) -> ()
                          }
                        }
                      }
                    }
                  }
                }
              }
              frame #1 {
                n2017 = case shown="True" w3140 {
                  tunnel: w3144 -> [_ w3149]
                  tunnel: w3143 -> [_ w3148]
                  tunnel: w3142 -> [_ w3146]
                  tunnel: w3141 -> [_ w3145]
                  frame False {
                  }
                  frame True {
                    n2018 = local read "DISP LAB01-2"() -> (w3150:T4)
                    n2019 = local read "SIG LAB01-2"() -> (w3151:T2)
                    n2020 = local read "ON L01-2"() -> (w3147:cluster{"amps":dbl, "volts":dbl, "pf":dbl})
                    n2021 = Unbundle(w3151) -> ("AMPS"=w3157:dbl, "VOLTS"=w3155:dbl, "PF"=w3154:dbl, "Tmp Live"=w3153:dbl, "Tmp Neut"=w3156:dbl)
                    n2022 = Unbundle(w3150) -> ("CYCLE"=w3152:dbl)  [unwired: 2 out]
                    n2023 = stacked-sequence {
                      tunnel: w3157 -> [w3161 w3180]
                      tunnel: w3156 -> [_ w3179]
                      tunnel: w3155 -> [w3160 w3178]
                      tunnel: w3154 -> [w3159 w3177]
                      tunnel: w3153 -> [_ w3176]
                      tunnel: w3152 -> [_ w3175]
                      tunnel: w3149 -> [_ w3174]
                      tunnel: w3148 -> [w3162 _]
                      tunnel: w3147 -> [w3158 w3172]
                      tunnel: w3146 -> [_ w3173]
                      tunnel: w3145 -> [_ w3168]
                      frame #0 {
                        n2024 = case shown="True" w3162 {
                          tunnel: w3161 -> [_ w3167]
                          tunnel: w3160 -> [_ w3166]
                          tunnel: w3159 -> [_ w3165]
                          tunnel: w3158 -> [_ w3163]
                          frame False {
                          }
                          frame True {
                            n2025 = Bundle(cluster=w3163, "amps"=w3167, "volts"=w3166, "pf"=w3165) -> (w3164:cluster{"amps":dbl, "volts":dbl, "pf":dbl})
                            n2026 = local write "ON L01-2"(w3164) -> ()
                          }
                        }
                      }
                      frame #1 {
                        n2027 = Unbundle(w3172) -> ("amps"=w3171:dbl, "volts"=w3170:dbl, "pf"=w3169:dbl)
                        n2028 = case shown="True" w3173 {
                          tunnel: w3180 -> [_ w3212]
                          tunnel: w3179 -> [_ w3219]
                          tunnel: w3178 -> [_ _]
                          tunnel: w3177 -> [_ _]
                          tunnel: w3176 -> [_ w3218]
                          tunnel: w3175 -> [_ w3217]
                          tunnel: w3174 -> [_ w3182]
                          tunnel: w3171 -> [_ w3214]
                          tunnel: w3170 -> [_ w3213]
                          tunnel: w3169 -> [_ w3211]
                          tunnel: w3168 -> [_ w3203]
                          frame False {
                          }
                          frame True {
                            n2029 = local read "TDMS LAB01-2"() -> (w3216:refnum<k34>)
                            n2030 = Build Array(w3213) -> (w3208:dbl[])
                            n2031 = Build Array(w3211) -> (w3207:dbl[])
                            n2032 = Build Array(w3218) -> (w3206:dbl[])
                            n2033 = Build Array(w3219) -> (w3205:dbl[])
                            n2034 = Build Array(w3214) -> (w3210:dbl[])
                            n2035 = Build Array(w3212) -> (w3209:dbl[])
                            n2036 = Build Array(w3217) -> (w3204:dbl[])
                            n2037 = Build Array("AMPS ON", "AMPS OFF", "VOLTS", "PF", "TEMP Live", "TEMP Neut", "CYCLE") -> (w3187:string[])
                            n2038 = Bundle By Name("Y"=w3210, "t0"=w3203) -> (w3202:waveform(dbl))  [unwired: 1 in]
                            n2039 = Bundle By Name("Y"=w3209, "t0"=w3203) -> (w3201:waveform(dbl))  [unwired: 1 in]
                            n2040 = Bundle By Name("Y"=w3208, "t0"=w3203) -> (w3200:waveform(dbl))  [unwired: 1 in]
                            n2041 = Bundle By Name("Y"=w3207, "t0"=w3203) -> (w3199:waveform(dbl))  [unwired: 1 in]
                            n2042 = Bundle By Name("Y"=w3206, "t0"=w3203) -> (w3198:waveform(dbl))  [unwired: 1 in]
                            n2043 = Bundle By Name("Y"=w3205, "t0"=w3203) -> (w3197:waveform(dbl))  [unwired: 1 in]
                            n2044 = Bundle By Name("Y"=w3204, "t0"=w3203) -> (w3196:waveform(dbl))  [unwired: 1 in]
                            n2045 = Build Array(w3202, w3201, w3200, w3199, w3198, w3197, w3196) -> (w3195:waveform(dbl)[])
                            n2046 = TDMS Write(0:w3216, 5:"TEST VALUES", 7:w3187, 9:w3195) -> (4:w3186:refnum<k34>, 6:w3185:string, 15:w3184:errorcluster)  [unwired: 2 in, 1 out]
                            n2047 = TDMS Write(0:w3186, 5:w3185, 7:"TIME", 9:w3182, 11:w3184) -> (15:w3181:errorcluster)  [unwired: 1 in, 3 out]
                            n2048 = local write "data file error"(w3181) -> ()
                          }
                        }
                      }
                    }
                  }
                }
              }
              frame #2 {
                n2049 = case shown="True" w3220 {
                  tunnel: w3224 -> [_ w3229]
                  tunnel: w3223 -> [_ w3228]
                  tunnel: w3222 -> [_ w3226]
                  tunnel: w3221 -> [_ w3225]
                  frame False {
                  }
                  frame True {
                    n2050 = local read "DISP LAB02-1"() -> (w3230:T4)
                    n2051 = local read "SIG LAB02-1"() -> (w3231:T2)
                    n2052 = local read "ON L02-1"() -> (w3227:cluster{"amps":dbl, "volts":dbl, "pf":dbl})
                    n2053 = Unbundle(w3231) -> ("AMPS"=w3237:dbl, "VOLTS"=w3235:dbl, "PF"=w3234:dbl, "Tmp Live"=w3233:dbl, "Tmp Neut"=w3236:dbl)
                    n2054 = Unbundle(w3230) -> ("CYCLE"=w3232:dbl)  [unwired: 2 out]
                    n2055 = stacked-sequence {
                      tunnel: w3237 -> [w3241 w3260]
                      tunnel: w3236 -> [_ w3259]
                      tunnel: w3235 -> [w3240 w3258]
                      tunnel: w3234 -> [w3239 w3257]
                      tunnel: w3233 -> [_ w3256]
                      tunnel: w3232 -> [_ w3255]
                      tunnel: w3229 -> [_ w3254]
                      tunnel: w3228 -> [w3242 _]
                      tunnel: w3227 -> [w3238 w3252]
                      tunnel: w3226 -> [_ w3253]
                      tunnel: w3225 -> [_ w3248]
                      frame #0 {
                        n2056 = case shown="True" w3242 {
                          tunnel: w3241 -> [_ w3247]
                          tunnel: w3240 -> [_ w3246]
                          tunnel: w3239 -> [_ w3245]
                          tunnel: w3238 -> [_ w3243]
                          frame False {
                          }
                          frame True {
                            n2057 = Bundle(cluster=w3243, "amps"=w3247, "volts"=w3246, "pf"=w3245) -> (w3244:cluster{"amps":dbl, "volts":dbl, "pf":dbl})
                            n2058 = local write "ON L02-1"(w3244) -> ()
                          }
                        }
                      }
                      frame #1 {
                        n2059 = Unbundle(w3252) -> ("amps"=w3251:dbl, "volts"=w3250:dbl, "pf"=w3249:dbl)
                        n2060 = case shown="True" w3253 {
                          tunnel: w3260 -> [_ w3292]
                          tunnel: w3259 -> [_ w3299]
                          tunnel: w3258 -> [_ _]
                          tunnel: w3257 -> [_ _]
                          tunnel: w3256 -> [_ w3298]
                          tunnel: w3255 -> [_ w3297]
                          tunnel: w3254 -> [_ w3262]
                          tunnel: w3251 -> [_ w3294]
                          tunnel: w3250 -> [_ w3293]
                          tunnel: w3249 -> [_ w3291]
                          tunnel: w3248 -> [_ w3283]
                          frame False {
                          }
                          frame True {
                            n2061 = local read "TDMS LAB02-1"() -> (w3296:refnum<k34>)
                            n2062 = Build Array(w3293) -> (w3288:dbl[])
                            n2063 = Build Array(w3291) -> (w3287:dbl[])
                            n2064 = Build Array(w3298) -> (w3286:dbl[])
                            n2065 = Build Array(w3299) -> (w3285:dbl[])
                            n2066 = Build Array(w3294) -> (w3290:dbl[])
                            n2067 = Build Array(w3292) -> (w3289:dbl[])
                            n2068 = Build Array(w3297) -> (w3284:dbl[])
                            n2069 = Build Array("AMPS ON", "AMPS OFF", "VOLTS", "PF", "TEMP Live", "TEMP Neut", "CYCLE") -> (w3267:string[])
                            n2070 = Bundle By Name("Y"=w3290, "t0"=w3283) -> (w3282:waveform(dbl))  [unwired: 1 in]
                            n2071 = Bundle By Name("Y"=w3289, "t0"=w3283) -> (w3281:waveform(dbl))  [unwired: 1 in]
                            n2072 = Bundle By Name("Y"=w3288, "t0"=w3283) -> (w3280:waveform(dbl))  [unwired: 1 in]
                            n2073 = Bundle By Name("Y"=w3287, "t0"=w3283) -> (w3279:waveform(dbl))  [unwired: 1 in]
                            n2074 = Bundle By Name("Y"=w3286, "t0"=w3283) -> (w3278:waveform(dbl))  [unwired: 1 in]
                            n2075 = Bundle By Name("Y"=w3285, "t0"=w3283) -> (w3277:waveform(dbl))  [unwired: 1 in]
                            n2076 = Bundle By Name("Y"=w3284, "t0"=w3283) -> (w3276:waveform(dbl))  [unwired: 1 in]
                            n2077 = Build Array(w3282, w3281, w3280, w3279, w3278, w3277, w3276) -> (w3275:waveform(dbl)[])
                            n2078 = TDMS Write(0:w3296, 5:"TEST VALUES", 7:w3267, 9:w3275) -> (4:w3266:refnum<k34>, 6:w3265:string, 15:w3264:errorcluster)  [unwired: 2 in, 1 out]
                            n2079 = TDMS Write(0:w3266, 5:w3265, 7:"TIME", 9:w3262, 11:w3264) -> (15:w3261:errorcluster)  [unwired: 1 in, 3 out]
                            n2080 = local write "data file error"(w3261) -> ()
                          }
                        }
                      }
                    }
                  }
                }
              }
              frame #3 {
                n2081 = case shown="True" w3300 {
                  tunnel: w3304 -> [_ w3309]
                  tunnel: w3303 -> [_ w3308]
                  tunnel: w3302 -> [_ w3306]
                  tunnel: w3301 -> [_ w3305]
                  frame False {
                  }
                  frame True {
                    n2082 = local read "DISP LAB02-2"() -> (w3310:T4)
                    n2083 = local read "SIG LAB02-2"() -> (w3311:T2)
                    n2084 = local read "ON L02-2"() -> (w3307:cluster{"amps":dbl, "volts":dbl, "pf":dbl})
                    n2085 = Unbundle(w3311) -> ("AMPS"=w3317:dbl, "VOLTS"=w3315:dbl, "PF"=w3314:dbl, "Tmp Live"=w3313:dbl, "Tmp Neut"=w3316:dbl)
                    n2086 = Unbundle(w3310) -> ("CYCLE"=w3312:dbl)  [unwired: 2 out]
                    n2087 = stacked-sequence {
                      tunnel: w3317 -> [w3321 w3340]
                      tunnel: w3316 -> [_ w3339]
                      tunnel: w3315 -> [w3320 w3338]
                      tunnel: w3314 -> [w3319 w3337]
                      tunnel: w3313 -> [_ w3336]
                      tunnel: w3312 -> [_ w3335]
                      tunnel: w3309 -> [_ w3334]
                      tunnel: w3308 -> [w3322 _]
                      tunnel: w3307 -> [w3318 w3332]
                      tunnel: w3306 -> [_ w3333]
                      tunnel: w3305 -> [_ w3328]
                      frame #0 {
                        n2088 = case shown="True" w3322 {
                          tunnel: w3321 -> [_ w3327]
                          tunnel: w3320 -> [_ w3326]
                          tunnel: w3319 -> [_ w3325]
                          tunnel: w3318 -> [_ w3323]
                          frame False {
                          }
                          frame True {
                            n2089 = Bundle(cluster=w3323, "amps"=w3327, "volts"=w3326, "pf"=w3325) -> (w3324:cluster{"amps":dbl, "volts":dbl, "pf":dbl})
                            n2090 = local write "ON L02-2"(w3324) -> ()
                          }
                        }
                      }
                      frame #1 {
                        n2091 = Unbundle(w3332) -> ("amps"=w3331:dbl, "volts"=w3330:dbl, "pf"=w3329:dbl)
                        n2092 = case shown="True" w3333 {
                          tunnel: w3340 -> [_ w3372]
                          tunnel: w3339 -> [_ w3379]
                          tunnel: w3338 -> [_ _]
                          tunnel: w3337 -> [_ _]
                          tunnel: w3336 -> [_ w3378]
                          tunnel: w3335 -> [_ w3377]
                          tunnel: w3334 -> [_ w3342]
                          tunnel: w3331 -> [_ w3374]
                          tunnel: w3330 -> [_ w3373]
                          tunnel: w3329 -> [_ w3371]
                          tunnel: w3328 -> [_ w3363]
                          frame False {
                          }
                          frame True {
                            n2093 = local read "TDMS LAB02-2"() -> (w3376:refnum<k34>)
                            n2094 = Build Array(w3373) -> (w3368:dbl[])
                            n2095 = Build Array(w3371) -> (w3367:dbl[])
                            n2096 = Build Array(w3378) -> (w3366:dbl[])
                            n2097 = Build Array(w3379) -> (w3365:dbl[])
                            n2098 = Build Array(w3374) -> (w3370:dbl[])
                            n2099 = Build Array(w3372) -> (w3369:dbl[])
                            n2100 = Build Array(w3377) -> (w3364:dbl[])
                            n2101 = Build Array("AMPS ON", "AMPS OFF", "VOLTS", "PF", "TEMP Live", "TEMP Neut", "CYCLE") -> (w3347:string[])
                            n2102 = Bundle By Name("Y"=w3370, "t0"=w3363) -> (w3362:waveform(dbl))  [unwired: 1 in]
                            n2103 = Bundle By Name("Y"=w3369, "t0"=w3363) -> (w3361:waveform(dbl))  [unwired: 1 in]
                            n2104 = Bundle By Name("Y"=w3368, "t0"=w3363) -> (w3360:waveform(dbl))  [unwired: 1 in]
                            n2105 = Bundle By Name("Y"=w3367, "t0"=w3363) -> (w3359:waveform(dbl))  [unwired: 1 in]
                            n2106 = Bundle By Name("Y"=w3366, "t0"=w3363) -> (w3358:waveform(dbl))  [unwired: 1 in]
                            n2107 = Bundle By Name("Y"=w3365, "t0"=w3363) -> (w3357:waveform(dbl))  [unwired: 1 in]
                            n2108 = Bundle By Name("Y"=w3364, "t0"=w3363) -> (w3356:waveform(dbl))  [unwired: 1 in]
                            n2109 = Build Array(w3362, w3361, w3360, w3359, w3358, w3357, w3356) -> (w3355:waveform(dbl)[])
                            n2110 = TDMS Write(0:w3376, 5:"TEST VALUES", 7:w3347, 9:w3355) -> (4:w3346:refnum<k34>, 6:w3345:string, 15:w3344:errorcluster)  [unwired: 2 in, 1 out]
                            n2111 = TDMS Write(0:w3346, 5:w3345, 7:"TIME", 9:w3342, 11:w3344) -> (15:w3341:errorcluster)  [unwired: 1 in, 3 out]
                            n2112 = local write "data file error"(w3341) -> ()
                          }
                        }
                      }
                    }
                  }
                }
              }
              frame #4 {
                n2113 = case shown="True" w3380 {
                  tunnel: w3384 -> [_ w3389]
                  tunnel: w3383 -> [_ w3388]
                  tunnel: w3382 -> [_ w3386]
                  tunnel: w3381 -> [_ w3385]
                  frame False {
                  }
                  frame True {
                    n2114 = local read "DISP LAB03-1"() -> (w3390:T4)
                    n2115 = local read "SIG LAB03-1"() -> (w3391:T2)
                    n2116 = local read "ON L03-1"() -> (w3387:cluster{"amps":dbl, "volts":dbl, "pf":dbl})
                    n2117 = Unbundle(w3391) -> ("AMPS"=w3397:dbl, "VOLTS"=w3395:dbl, "PF"=w3394:dbl, "Tmp Live"=w3393:dbl, "Tmp Neut"=w3396:dbl)
                    n2118 = Unbundle(w3390) -> ("CYCLE"=w3392:dbl)  [unwired: 2 out]
                    n2119 = stacked-sequence {
                      tunnel: w3397 -> [w3401 w3420]
                      tunnel: w3396 -> [_ w3419]
                      tunnel: w3395 -> [w3400 w3418]
                      tunnel: w3394 -> [w3399 w3417]
                      tunnel: w3393 -> [_ w3416]
                      tunnel: w3392 -> [_ w3415]
                      tunnel: w3389 -> [_ w3414]
                      tunnel: w3388 -> [w3402 _]
                      tunnel: w3387 -> [w3398 w3412]
                      tunnel: w3386 -> [_ w3413]
                      tunnel: w3385 -> [_ w3408]
                      frame #0 {
                        n2120 = case shown="True" w3402 {
                          tunnel: w3401 -> [_ w3407]
                          tunnel: w3400 -> [_ w3406]
                          tunnel: w3399 -> [_ w3405]
                          tunnel: w3398 -> [_ w3403]
                          frame False {
                          }
                          frame True {
                            n2121 = Bundle(cluster=w3403, "amps"=w3407, "volts"=w3406, "pf"=w3405) -> (w3404:cluster{"amps":dbl, "volts":dbl, "pf":dbl})
                            n2122 = local write "ON L03-1"(w3404) -> ()
                          }
                        }
                      }
                      frame #1 {
                        n2123 = Unbundle(w3412) -> ("amps"=w3411:dbl, "volts"=w3410:dbl, "pf"=w3409:dbl)
                        n2124 = case shown="True" w3413 {
                          tunnel: w3420 -> [_ w3452]
                          tunnel: w3419 -> [_ w3459]
                          tunnel: w3418 -> [_ _]
                          tunnel: w3417 -> [_ _]
                          tunnel: w3416 -> [_ w3458]
                          tunnel: w3415 -> [_ w3457]
                          tunnel: w3414 -> [_ w3422]
                          tunnel: w3411 -> [_ w3454]
                          tunnel: w3410 -> [_ w3453]
                          tunnel: w3409 -> [_ w3451]
                          tunnel: w3408 -> [_ w3443]
                          frame False {
                          }
                          frame True {
                            n2125 = local read "TDMS LAB03-1"() -> (w3456:refnum<k34>)
                            n2126 = Build Array(w3453) -> (w3448:dbl[])
                            n2127 = Build Array(w3451) -> (w3447:dbl[])
                            n2128 = Build Array(w3458) -> (w3446:dbl[])
                            n2129 = Build Array(w3459) -> (w3445:dbl[])
                            n2130 = Build Array(w3454) -> (w3450:dbl[])
                            n2131 = Build Array(w3452) -> (w3449:dbl[])
                            n2132 = Build Array(w3457) -> (w3444:dbl[])
                            n2133 = Build Array("AMPS ON", "AMPS OFF", "VOLTS", "PF", "TEMP Live", "TEMP Neut", "CYCLE") -> (w3427:string[])
                            n2134 = Bundle By Name("Y"=w3450, "t0"=w3443) -> (w3442:waveform(dbl))  [unwired: 1 in]
                            n2135 = Bundle By Name("Y"=w3449, "t0"=w3443) -> (w3441:waveform(dbl))  [unwired: 1 in]
                            n2136 = Bundle By Name("Y"=w3448, "t0"=w3443) -> (w3440:waveform(dbl))  [unwired: 1 in]
                            n2137 = Bundle By Name("Y"=w3447, "t0"=w3443) -> (w3439:waveform(dbl))  [unwired: 1 in]
                            n2138 = Bundle By Name("Y"=w3446, "t0"=w3443) -> (w3438:waveform(dbl))  [unwired: 1 in]
                            n2139 = Bundle By Name("Y"=w3445, "t0"=w3443) -> (w3437:waveform(dbl))  [unwired: 1 in]
                            n2140 = Bundle By Name("Y"=w3444, "t0"=w3443) -> (w3436:waveform(dbl))  [unwired: 1 in]
                            n2141 = Build Array(w3442, w3441, w3440, w3439, w3438, w3437, w3436) -> (w3435:waveform(dbl)[])
                            n2142 = TDMS Write(0:w3456, 5:"TEST VALUES", 7:w3427, 9:w3435) -> (4:w3426:refnum<k34>, 6:w3425:string, 15:w3424:errorcluster)  [unwired: 2 in, 1 out]
                            n2143 = TDMS Write(0:w3426, 5:w3425, 7:"TIME", 9:w3422, 11:w3424) -> (15:w3421:errorcluster)  [unwired: 1 in, 3 out]
                            n2144 = local write "data file error"(w3421) -> ()
                          }
                        }
                      }
                    }
                  }
                }
              }
              frame #5 {
                n2145 = case shown="True" w3460 {
                  tunnel: w3464 -> [_ w3469]
                  tunnel: w3463 -> [_ w3468]
                  tunnel: w3462 -> [_ w3466]
                  tunnel: w3461 -> [_ w3465]
                  frame False {
                  }
                  frame True {
                    n2146 = local read "DISP LAB03-2"() -> (w3470:T4)
                    n2147 = local read "SIG LAB03-2"() -> (w3471:T2)
                    n2148 = local read "ON L03-2"() -> (w3467:cluster{"amps":dbl, "volts":dbl, "pf":dbl})
                    n2149 = Unbundle(w3471) -> ("AMPS"=w3477:dbl, "VOLTS"=w3475:dbl, "PF"=w3474:dbl, "Tmp Live"=w3473:dbl, "Tmp Neut"=w3476:dbl)
                    n2150 = Unbundle(w3470) -> ("CYCLE"=w3472:dbl)  [unwired: 2 out]
                    n2151 = stacked-sequence {
                      tunnel: w3477 -> [w3481 w3500]
                      tunnel: w3476 -> [_ w3499]
                      tunnel: w3475 -> [w3480 w3498]
                      tunnel: w3474 -> [w3479 w3497]
                      tunnel: w3473 -> [_ w3496]
                      tunnel: w3472 -> [_ w3495]
                      tunnel: w3469 -> [_ w3494]
                      tunnel: w3468 -> [w3482 _]
                      tunnel: w3467 -> [w3478 w3492]
                      tunnel: w3466 -> [_ w3493]
                      tunnel: w3465 -> [_ w3488]
                      frame #0 {
                        n2152 = case shown="True" w3482 {
                          tunnel: w3481 -> [_ w3487]
                          tunnel: w3480 -> [_ w3486]
                          tunnel: w3479 -> [_ w3485]
                          tunnel: w3478 -> [_ w3483]
                          frame False {
                          }
                          frame True {
                            n2153 = Bundle(cluster=w3483, "amps"=w3487, "volts"=w3486, "pf"=w3485) -> (w3484:cluster{"amps":dbl, "volts":dbl, "pf":dbl})
                            n2154 = local write "ON L03-2"(w3484) -> ()
                          }
                        }
                      }
                      frame #1 {
                        n2155 = Unbundle(w3492) -> ("amps"=w3491:dbl, "volts"=w3490:dbl, "pf"=w3489:dbl)
                        n2156 = case shown="True" w3493 {
                          tunnel: w3500 -> [_ w3532]
                          tunnel: w3499 -> [_ w3539]
                          tunnel: w3498 -> [_ _]
                          tunnel: w3497 -> [_ _]
                          tunnel: w3496 -> [_ w3538]
                          tunnel: w3495 -> [_ w3537]
                          tunnel: w3494 -> [_ w3502]
                          tunnel: w3491 -> [_ w3534]
                          tunnel: w3490 -> [_ w3533]
                          tunnel: w3489 -> [_ w3531]
                          tunnel: w3488 -> [_ w3523]
                          frame False {
                          }
                          frame True {
                            n2157 = local read "TDMS LAB03-2"() -> (w3536:refnum<k34>)
                            n2158 = Build Array(w3533) -> (w3528:dbl[])
                            n2159 = Build Array(w3531) -> (w3527:dbl[])
                            n2160 = Build Array(w3538) -> (w3526:dbl[])
                            n2161 = Build Array(w3539) -> (w3525:dbl[])
                            n2162 = Build Array(w3534) -> (w3530:dbl[])
                            n2163 = Build Array(w3532) -> (w3529:dbl[])
                            n2164 = Build Array(w3537) -> (w3524:dbl[])
                            n2165 = Build Array("AMPS ON", "AMPS OFF", "VOLTS", "PF", "TEMP Live", "TEMP Neut", "CYCLE") -> (w3507:string[])
                            n2166 = Bundle By Name("Y"=w3530, "t0"=w3523) -> (w3522:waveform(dbl))  [unwired: 1 in]
                            n2167 = Bundle By Name("Y"=w3529, "t0"=w3523) -> (w3521:waveform(dbl))  [unwired: 1 in]
                            n2168 = Bundle By Name("Y"=w3528, "t0"=w3523) -> (w3520:waveform(dbl))  [unwired: 1 in]
                            n2169 = Bundle By Name("Y"=w3527, "t0"=w3523) -> (w3519:waveform(dbl))  [unwired: 1 in]
                            n2170 = Bundle By Name("Y"=w3526, "t0"=w3523) -> (w3518:waveform(dbl))  [unwired: 1 in]
                            n2171 = Bundle By Name("Y"=w3525, "t0"=w3523) -> (w3517:waveform(dbl))  [unwired: 1 in]
                            n2172 = Bundle By Name("Y"=w3524, "t0"=w3523) -> (w3516:waveform(dbl))  [unwired: 1 in]
                            n2173 = Build Array(w3522, w3521, w3520, w3519, w3518, w3517, w3516) -> (w3515:waveform(dbl)[])
                            n2174 = TDMS Write(0:w3536, 5:"TEST VALUES", 7:w3507, 9:w3515) -> (4:w3506:refnum<k34>, 6:w3505:string, 15:w3504:errorcluster)  [unwired: 2 in, 1 out]
                            n2175 = TDMS Write(0:w3506, 5:w3505, 7:"TIME", 9:w3502, 11:w3504) -> (15:w3501:errorcluster)  [unwired: 1 in, 3 out]
                            n2176 = local write "data file error"(w3501) -> ()
                          }
                        }
                      }
                    }
                  }
                }
              }
              frame #6 {
                n2177 = case shown="True" w3540 {
                  tunnel: w3544 -> [_ w3549]
                  tunnel: w3543 -> [_ w3548]
                  tunnel: w3542 -> [_ w3546]
                  tunnel: w3541 -> [_ w3545]
                  frame False {
                  }
                  frame True {
                    n2178 = local read "DISP LAB04-1"() -> (w3550:T4)
                    n2179 = local read "SIG LAB04-1"() -> (w3551:T2)
                    n2180 = local read "ON L04-1"() -> (w3547:cluster{"amps":dbl, "volts":dbl, "pf":dbl})
                    n2181 = Unbundle(w3551) -> ("AMPS"=w3557:dbl, "VOLTS"=w3555:dbl, "PF"=w3554:dbl, "Tmp Live"=w3553:dbl, "Tmp Neut"=w3556:dbl)
                    n2182 = Unbundle(w3550) -> ("CYCLE"=w3552:dbl)  [unwired: 2 out]
                    n2183 = stacked-sequence {
                      tunnel: w3557 -> [w3561 w3580]
                      tunnel: w3556 -> [_ w3579]
                      tunnel: w3555 -> [w3560 w3578]
                      tunnel: w3554 -> [w3559 w3577]
                      tunnel: w3553 -> [_ w3576]
                      tunnel: w3552 -> [_ w3575]
                      tunnel: w3549 -> [_ w3574]
                      tunnel: w3548 -> [w3562 _]
                      tunnel: w3547 -> [w3558 w3572]
                      tunnel: w3546 -> [_ w3573]
                      tunnel: w3545 -> [_ w3568]
                      frame #0 {
                        n2184 = case shown="True" w3562 {
                          tunnel: w3561 -> [_ w3567]
                          tunnel: w3560 -> [_ w3566]
                          tunnel: w3559 -> [_ w3565]
                          tunnel: w3558 -> [_ w3563]
                          frame False {
                          }
                          frame True {
                            n2185 = Bundle(cluster=w3563, "amps"=w3567, "volts"=w3566, "pf"=w3565) -> (w3564:cluster{"amps":dbl, "volts":dbl, "pf":dbl})
                            n2186 = local write "ON L04-1"(w3564) -> ()
                          }
                        }
                      }
                      frame #1 {
                        n2187 = Unbundle(w3572) -> ("amps"=w3571:dbl, "volts"=w3570:dbl, "pf"=w3569:dbl)
                        n2188 = case shown="True" w3573 {
                          tunnel: w3580 -> [_ w3612]
                          tunnel: w3579 -> [_ w3619]
                          tunnel: w3578 -> [_ _]
                          tunnel: w3577 -> [_ _]
                          tunnel: w3576 -> [_ w3618]
                          tunnel: w3575 -> [_ w3617]
                          tunnel: w3574 -> [_ w3582]
                          tunnel: w3571 -> [_ w3614]
                          tunnel: w3570 -> [_ w3613]
                          tunnel: w3569 -> [_ w3611]
                          tunnel: w3568 -> [_ w3603]
                          frame False {
                          }
                          frame True {
                            n2189 = local read "TDMS LAB04-1"() -> (w3616:refnum<k34>)
                            n2190 = Build Array(w3613) -> (w3608:dbl[])
                            n2191 = Build Array(w3611) -> (w3607:dbl[])
                            n2192 = Build Array(w3618) -> (w3606:dbl[])
                            n2193 = Build Array(w3619) -> (w3605:dbl[])
                            n2194 = Build Array(w3614) -> (w3610:dbl[])
                            n2195 = Build Array(w3612) -> (w3609:dbl[])
                            n2196 = Build Array(w3617) -> (w3604:dbl[])
                            n2197 = Build Array("AMPS ON", "AMPS OFF", "VOLTS", "PF", "TEMP Live", "TEMP Neut", "CYCLE") -> (w3587:string[])
                            n2198 = Bundle By Name("Y"=w3610, "t0"=w3603) -> (w3602:waveform(dbl))  [unwired: 1 in]
                            n2199 = Bundle By Name("Y"=w3609, "t0"=w3603) -> (w3601:waveform(dbl))  [unwired: 1 in]
                            n2200 = Bundle By Name("Y"=w3608, "t0"=w3603) -> (w3600:waveform(dbl))  [unwired: 1 in]
                            n2201 = Bundle By Name("Y"=w3607, "t0"=w3603) -> (w3599:waveform(dbl))  [unwired: 1 in]
                            n2202 = Bundle By Name("Y"=w3606, "t0"=w3603) -> (w3598:waveform(dbl))  [unwired: 1 in]
                            n2203 = Bundle By Name("Y"=w3605, "t0"=w3603) -> (w3597:waveform(dbl))  [unwired: 1 in]
                            n2204 = Bundle By Name("Y"=w3604, "t0"=w3603) -> (w3596:waveform(dbl))  [unwired: 1 in]
                            n2205 = Build Array(w3602, w3601, w3600, w3599, w3598, w3597, w3596) -> (w3595:waveform(dbl)[])
                            n2206 = TDMS Write(0:w3616, 5:"TEST VALUES", 7:w3587, 9:w3595) -> (4:w3586:refnum<k34>, 6:w3585:string, 15:w3584:errorcluster)  [unwired: 2 in, 1 out]
                            n2207 = TDMS Write(0:w3586, 5:w3585, 7:"TIME", 9:w3582, 11:w3584) -> (15:w3581:errorcluster)  [unwired: 1 in, 3 out]
                            n2208 = local write "data file error"(w3581) -> ()
                          }
                        }
                      }
                    }
                  }
                }
              }
              frame #7 {
                n2209 = case shown="True" w3620 {
                  tunnel: w3624 -> [_ w3629]
                  tunnel: w3623 -> [_ w3628]
                  tunnel: w3622 -> [_ w3626]
                  tunnel: w3621 -> [_ w3625]
                  frame False {
                  }
                  frame True {
                    n2210 = local read "DISP LAB04-2"() -> (w3630:T4)
                    n2211 = local read "SIG LAB04-2"() -> (w3631:T2)
                    n2212 = local read "ON L04-2"() -> (w3627:cluster{"amps":dbl, "volts":dbl, "pf":dbl})
                    n2213 = Unbundle(w3631) -> ("AMPS"=w3637:dbl, "VOLTS"=w3635:dbl, "PF"=w3634:dbl, "Tmp Live"=w3633:dbl, "Tmp Neut"=w3636:dbl)
                    n2214 = Unbundle(w3630) -> ("CYCLE"=w3632:dbl)  [unwired: 2 out]
                    n2215 = stacked-sequence {
                      tunnel: w3637 -> [w3641 w3660]
                      tunnel: w3636 -> [_ w3659]
                      tunnel: w3635 -> [w3640 w3658]
                      tunnel: w3634 -> [w3639 w3657]
                      tunnel: w3633 -> [_ w3656]
                      tunnel: w3632 -> [_ w3655]
                      tunnel: w3629 -> [_ w3654]
                      tunnel: w3628 -> [w3642 _]
                      tunnel: w3627 -> [w3638 w3652]
                      tunnel: w3626 -> [_ w3653]
                      tunnel: w3625 -> [_ w3648]
                      frame #0 {
                        n2216 = case shown="True" w3642 {
                          tunnel: w3641 -> [_ w3647]
                          tunnel: w3640 -> [_ w3646]
                          tunnel: w3639 -> [_ w3645]
                          tunnel: w3638 -> [_ w3643]
                          frame False {
                          }
                          frame True {
                            n2217 = Bundle(cluster=w3643, "amps"=w3647, "volts"=w3646, "pf"=w3645) -> (w3644:cluster{"amps":dbl, "volts":dbl, "pf":dbl})
                            n2218 = local write "ON L04-2"(w3644) -> ()
                          }
                        }
                      }
                      frame #1 {
                        n2219 = Unbundle(w3652) -> ("amps"=w3651:dbl, "volts"=w3650:dbl, "pf"=w3649:dbl)
                        n2220 = case shown="True" w3653 {
                          tunnel: w3660 -> [_ w3692]
                          tunnel: w3659 -> [_ w3699]
                          tunnel: w3658 -> [_ _]
                          tunnel: w3657 -> [_ _]
                          tunnel: w3656 -> [_ w3698]
                          tunnel: w3655 -> [_ w3697]
                          tunnel: w3654 -> [_ w3662]
                          tunnel: w3651 -> [_ w3694]
                          tunnel: w3650 -> [_ w3693]
                          tunnel: w3649 -> [_ w3691]
                          tunnel: w3648 -> [_ w3683]
                          frame False {
                          }
                          frame True {
                            n2221 = local read "TDMS LAB04-2"() -> (w3696:refnum<k34>)
                            n2222 = Build Array(w3693) -> (w3688:dbl[])
                            n2223 = Build Array(w3691) -> (w3687:dbl[])
                            n2224 = Build Array(w3698) -> (w3686:dbl[])
                            n2225 = Build Array(w3699) -> (w3685:dbl[])
                            n2226 = Build Array(w3694) -> (w3690:dbl[])
                            n2227 = Build Array(w3692) -> (w3689:dbl[])
                            n2228 = Build Array(w3697) -> (w3684:dbl[])
                            n2229 = Build Array("AMPS ON", "AMPS OFF", "VOLTS", "PF", "TEMP Live", "TEMP Neut", "CYCLE") -> (w3667:string[])
                            n2230 = Bundle By Name("Y"=w3690, "t0"=w3683) -> (w3682:waveform(dbl))  [unwired: 1 in]
                            n2231 = Bundle By Name("Y"=w3689, "t0"=w3683) -> (w3681:waveform(dbl))  [unwired: 1 in]
                            n2232 = Bundle By Name("Y"=w3688, "t0"=w3683) -> (w3680:waveform(dbl))  [unwired: 1 in]
                            n2233 = Bundle By Name("Y"=w3687, "t0"=w3683) -> (w3679:waveform(dbl))  [unwired: 1 in]
                            n2234 = Bundle By Name("Y"=w3686, "t0"=w3683) -> (w3678:waveform(dbl))  [unwired: 1 in]
                            n2235 = Bundle By Name("Y"=w3685, "t0"=w3683) -> (w3677:waveform(dbl))  [unwired: 1 in]
                            n2236 = Bundle By Name("Y"=w3684, "t0"=w3683) -> (w3676:waveform(dbl))  [unwired: 1 in]
                            n2237 = Build Array(w3682, w3681, w3680, w3679, w3678, w3677, w3676) -> (w3675:waveform(dbl)[])
                            n2238 = TDMS Write(0:w3696, 5:"TEST VALUES", 7:w3667, 9:w3675) -> (4:w3666:refnum<k34>, 6:w3665:string, 15:w3664:errorcluster)  [unwired: 2 in, 1 out]
                            n2239 = TDMS Write(0:w3666, 5:w3665, 7:"TIME", 9:w3662, 11:w3664) -> (15:w3661:errorcluster)  [unwired: 1 in, 3 out]
                            n2240 = local write "data file error"(w3661) -> ()
                          }
                        }
                      }
                    }
                  }
                }
              }
              frame #8 {
                n2241 = case shown="True" w3700 {
                  tunnel: w3704 -> [_ w3709]
                  tunnel: w3703 -> [_ w3708]
                  tunnel: w3702 -> [_ w3706]
                  tunnel: w3701 -> [_ w3705]
                  frame False {
                  }
                  frame True {
                    n2242 = local read "DISP LAB05-1"() -> (w3710:T4)
                    n2243 = local read "SIG LAB05-1"() -> (w3711:T2)
                    n2244 = local read "ON L05-1"() -> (w3707:cluster{"amps":dbl, "volts":dbl, "pf":dbl})
                    n2245 = Unbundle(w3711) -> ("AMPS"=w3717:dbl, "VOLTS"=w3715:dbl, "PF"=w3714:dbl, "Tmp Live"=w3713:dbl, "Tmp Neut"=w3716:dbl)
                    n2246 = Unbundle(w3710) -> ("CYCLE"=w3712:dbl)  [unwired: 2 out]
                    n2247 = stacked-sequence {
                      tunnel: w3717 -> [w3721 w3740]
                      tunnel: w3716 -> [_ w3739]
                      tunnel: w3715 -> [w3720 w3738]
                      tunnel: w3714 -> [w3719 w3737]
                      tunnel: w3713 -> [_ w3736]
                      tunnel: w3712 -> [_ w3735]
                      tunnel: w3709 -> [_ w3734]
                      tunnel: w3708 -> [w3722 _]
                      tunnel: w3707 -> [w3718 w3732]
                      tunnel: w3706 -> [_ w3733]
                      tunnel: w3705 -> [_ w3728]
                      frame #0 {
                        n2248 = case shown="True" w3722 {
                          tunnel: w3721 -> [_ w3727]
                          tunnel: w3720 -> [_ w3726]
                          tunnel: w3719 -> [_ w3725]
                          tunnel: w3718 -> [_ w3723]
                          frame False {
                          }
                          frame True {
                            n2249 = Bundle(cluster=w3723, "amps"=w3727, "volts"=w3726, "pf"=w3725) -> (w3724:cluster{"amps":dbl, "volts":dbl, "pf":dbl})
                            n2250 = local write "ON L05-1"(w3724) -> ()
                          }
                        }
                      }
                      frame #1 {
                        n2251 = Unbundle(w3732) -> ("amps"=w3731:dbl, "volts"=w3730:dbl, "pf"=w3729:dbl)
                        n2252 = case shown="True" w3733 {
                          tunnel: w3740 -> [_ w3772]
                          tunnel: w3739 -> [_ w3779]
                          tunnel: w3738 -> [_ _]
                          tunnel: w3737 -> [_ _]
                          tunnel: w3736 -> [_ w3778]
                          tunnel: w3735 -> [_ w3777]
                          tunnel: w3734 -> [_ w3742]
                          tunnel: w3731 -> [_ w3774]
                          tunnel: w3730 -> [_ w3773]
                          tunnel: w3729 -> [_ w3771]
                          tunnel: w3728 -> [_ w3763]
                          frame False {
                          }
                          frame True {
                            n2253 = local read "TDMS LAB05-1"() -> (w3776:refnum<k34>)
                            n2254 = Build Array(w3773) -> (w3768:dbl[])
                            n2255 = Build Array(w3771) -> (w3767:dbl[])
                            n2256 = Build Array(w3778) -> (w3766:dbl[])
                            n2257 = Build Array(w3779) -> (w3765:dbl[])
                            n2258 = Build Array(w3774) -> (w3770:dbl[])
                            n2259 = Build Array(w3772) -> (w3769:dbl[])
                            n2260 = Build Array(w3777) -> (w3764:dbl[])
                            n2261 = Build Array("AMPS ON", "AMPS OFF", "VOLTS", "PF", "TEMP Live", "TEMP Neut", "CYCLE") -> (w3747:string[])
                            n2262 = Bundle By Name("Y"=w3770, "t0"=w3763) -> (w3762:waveform(dbl))  [unwired: 1 in]
                            n2263 = Bundle By Name("Y"=w3769, "t0"=w3763) -> (w3761:waveform(dbl))  [unwired: 1 in]
                            n2264 = Bundle By Name("Y"=w3768, "t0"=w3763) -> (w3760:waveform(dbl))  [unwired: 1 in]
                            n2265 = Bundle By Name("Y"=w3767, "t0"=w3763) -> (w3759:waveform(dbl))  [unwired: 1 in]
                            n2266 = Bundle By Name("Y"=w3766, "t0"=w3763) -> (w3758:waveform(dbl))  [unwired: 1 in]
                            n2267 = Bundle By Name("Y"=w3765, "t0"=w3763) -> (w3757:waveform(dbl))  [unwired: 1 in]
                            n2268 = Bundle By Name("Y"=w3764, "t0"=w3763) -> (w3756:waveform(dbl))  [unwired: 1 in]
                            n2269 = Build Array(w3762, w3761, w3760, w3759, w3758, w3757, w3756) -> (w3755:waveform(dbl)[])
                            n2270 = TDMS Write(0:w3776, 5:"TEST VALUES", 7:w3747, 9:w3755) -> (4:w3746:refnum<k34>, 6:w3745:string, 15:w3744:errorcluster)  [unwired: 2 in, 1 out]
                            n2271 = TDMS Write(0:w3746, 5:w3745, 7:"TIME", 9:w3742, 11:w3744) -> (15:w3741:errorcluster)  [unwired: 1 in, 3 out]
                            n2272 = local write "data file error"(w3741) -> ()
                          }
                        }
                      }
                    }
                  }
                }
              }
              frame #9 {
                n2273 = case shown="True" w3780 {
                  tunnel: w3784 -> [_ w3789]
                  tunnel: w3783 -> [_ w3788]
                  tunnel: w3782 -> [_ w3786]
                  tunnel: w3781 -> [_ w3785]
                  frame False {
                  }
                  frame True {
                    n2274 = local read "DISP LAB05-2"() -> (w3790:T4)
                    n2275 = local read "SIG LAB05-2"() -> (w3791:T2)
                    n2276 = local read "ON L05-2"() -> (w3787:cluster{"amps":dbl, "volts":dbl, "pf":dbl})
                    n2277 = Unbundle(w3791) -> ("AMPS"=w3797:dbl, "VOLTS"=w3795:dbl, "PF"=w3794:dbl, "Tmp Live"=w3793:dbl, "Tmp Neut"=w3796:dbl)
                    n2278 = Unbundle(w3790) -> ("CYCLE"=w3792:dbl)  [unwired: 2 out]
                    n2279 = stacked-sequence {
                      tunnel: w3797 -> [w3801 w3820]
                      tunnel: w3796 -> [_ w3819]
                      tunnel: w3795 -> [w3800 w3818]
                      tunnel: w3794 -> [w3799 w3817]
                      tunnel: w3793 -> [_ w3816]
                      tunnel: w3792 -> [_ w3815]
                      tunnel: w3789 -> [_ w3814]
                      tunnel: w3788 -> [w3802 _]
                      tunnel: w3787 -> [w3798 w3812]
                      tunnel: w3786 -> [_ w3813]
                      tunnel: w3785 -> [_ w3808]
                      frame #0 {
                        n2280 = case shown="True" w3802 {
                          tunnel: w3801 -> [_ w3807]
                          tunnel: w3800 -> [_ w3806]
                          tunnel: w3799 -> [_ w3805]
                          tunnel: w3798 -> [_ w3803]
                          frame False {
                          }
                          frame True {
                            n2281 = Bundle(cluster=w3803, "amps"=w3807, "volts"=w3806, "pf"=w3805) -> (w3804:cluster{"amps":dbl, "volts":dbl, "pf":dbl})
                            n2282 = local write "ON L05-2"(w3804) -> ()
                          }
                        }
                      }
                      frame #1 {
                        n2283 = Unbundle(w3812) -> ("amps"=w3811:dbl, "volts"=w3810:dbl, "pf"=w3809:dbl)
                        n2284 = case shown="True" w3813 {
                          tunnel: w3820 -> [_ w3852]
                          tunnel: w3819 -> [_ w3859]
                          tunnel: w3818 -> [_ _]
                          tunnel: w3817 -> [_ _]
                          tunnel: w3816 -> [_ w3858]
                          tunnel: w3815 -> [_ w3857]
                          tunnel: w3814 -> [_ w3822]
                          tunnel: w3811 -> [_ w3854]
                          tunnel: w3810 -> [_ w3853]
                          tunnel: w3809 -> [_ w3851]
                          tunnel: w3808 -> [_ w3843]
                          frame False {
                          }
                          frame True {
                            n2285 = local read "TDMS LAB05-2"() -> (w3856:refnum<k34>)
                            n2286 = Build Array(w3853) -> (w3848:dbl[])
                            n2287 = Build Array(w3851) -> (w3847:dbl[])
                            n2288 = Build Array(w3858) -> (w3846:dbl[])
                            n2289 = Build Array(w3859) -> (w3845:dbl[])
                            n2290 = Build Array(w3854) -> (w3850:dbl[])
                            n2291 = Build Array(w3852) -> (w3849:dbl[])
                            n2292 = Build Array(w3857) -> (w3844:dbl[])
                            n2293 = Build Array("AMPS ON", "AMPS OFF", "VOLTS", "PF", "TEMP Live", "TEMP Neut", "CYCLE") -> (w3827:string[])
                            n2294 = Bundle By Name("Y"=w3850, "t0"=w3843) -> (w3842:waveform(dbl))  [unwired: 1 in]
                            n2295 = Bundle By Name("Y"=w3849, "t0"=w3843) -> (w3841:waveform(dbl))  [unwired: 1 in]
                            n2296 = Bundle By Name("Y"=w3848, "t0"=w3843) -> (w3840:waveform(dbl))  [unwired: 1 in]
                            n2297 = Bundle By Name("Y"=w3847, "t0"=w3843) -> (w3839:waveform(dbl))  [unwired: 1 in]
                            n2298 = Bundle By Name("Y"=w3846, "t0"=w3843) -> (w3838:waveform(dbl))  [unwired: 1 in]
                            n2299 = Bundle By Name("Y"=w3845, "t0"=w3843) -> (w3837:waveform(dbl))  [unwired: 1 in]
                            n2300 = Bundle By Name("Y"=w3844, "t0"=w3843) -> (w3836:waveform(dbl))  [unwired: 1 in]
                            n2301 = Build Array(w3842, w3841, w3840, w3839, w3838, w3837, w3836) -> (w3835:waveform(dbl)[])
                            n2302 = TDMS Write(0:w3856, 5:"TEST VALUES", 7:w3827, 9:w3835) -> (4:w3826:refnum<k34>, 6:w3825:string, 15:w3824:errorcluster)  [unwired: 2 in, 1 out]
                            n2303 = TDMS Write(0:w3826, 5:w3825, 7:"TIME", 9:w3822, 11:w3824) -> (15:w3821:errorcluster)  [unwired: 1 in, 3 out]
                            n2304 = local write "data file error"(w3821) -> ()
                          }
                        }
                      }
                    }
                  }
                }
              }
            }
          }
          frame #14 {
            # "display test values on chart"
            n2305 = case shown="\"OFF CYCLE\"" "Select  Cycle" {
              tunnel: [1 w3865] -> w3860
              frame "ON CYCLE", Default {
              }
              frame "OFF CYCLE" {
                n2306 = local read "on loops"() -> (w3867:dbl)
                n2307 = Add(x=w3867, y=2) -> (x+y=w3865:dbl)
              }
            }
            n2308 = local read "jig cycle"() -> (w3862:dbl)
            n2309 = Equal?(x=w3862, y=w3860) -> (x = y?=w3863:bool)
            n2310 = case shown="True" w3863 {
              frame False {
              }
              frame True {
                n2311 = local read "SIG LAB05-1"() -> (w3909:T2)
                n2312 = local read "SIG LAB04-2"() -> (w3910:T2)
                n2313 = local read "SIG LAB05-2"() -> (w3908:T2)
                n2314 = local read "SIG LAB04-1"() -> (w3911:T2)
                n2315 = local read "SIG LAB03-1"() -> (w3913:T2)
                n2316 = local read "SIG LAB03-2"() -> (w3912:T2)
                n2317 = local read "SIG LAB01-1"() -> (w3917:T2)
                n2318 = local read "SIG LAB02-2"() -> (w3914:T2)
                n2319 = local read "SIG LAB02-1"() -> (w3915:T2)
                n2320 = local read "SIG LAB01-2"() -> (w3916:T2)
                n2321 = Unbundle(w3910) -> ("AMPS"=w3900:dbl, "VOLTS"=w3890:dbl, "Tmp Live"=w3880:dbl, "Tmp Neut"=w3870:dbl)  [unwired: 1 out]
                n2322 = Unbundle(w3909) -> ("AMPS"=w3899:dbl, "VOLTS"=w3889:dbl, "Tmp Live"=w3879:dbl, "Tmp Neut"=w3869:dbl)  [unwired: 1 out]
                n2323 = Unbundle(w3908) -> ("AMPS"=w3898:dbl, "VOLTS"=w3888:dbl, "Tmp Live"=w3878:dbl, "Tmp Neut"=w3868:dbl)  [unwired: 1 out]
                n2324 = Unbundle(w3911) -> ("AMPS"=w3901:dbl, "VOLTS"=w3891:dbl, "Tmp Live"=w3881:dbl, "Tmp Neut"=w3871:dbl)  [unwired: 1 out]
                n2325 = Unbundle(w3912) -> ("AMPS"=w3902:dbl, "VOLTS"=w3892:dbl, "Tmp Live"=w3882:dbl, "Tmp Neut"=w3872:dbl)  [unwired: 1 out]
                n2326 = Unbundle(w3913) -> ("AMPS"=w3903:dbl, "VOLTS"=w3893:dbl, "Tmp Live"=w3883:dbl, "Tmp Neut"=w3873:dbl)  [unwired: 1 out]
                n2327 = Unbundle(w3914) -> ("AMPS"=w3904:dbl, "VOLTS"=w3894:dbl, "Tmp Live"=w3884:dbl, "Tmp Neut"=w3874:dbl)  [unwired: 1 out]
                n2328 = Unbundle(w3915) -> ("AMPS"=w3905:dbl, "VOLTS"=w3895:dbl, "Tmp Live"=w3885:dbl, "Tmp Neut"=w3875:dbl)  [unwired: 1 out]
                n2329 = Unbundle(w3917) -> ("AMPS"=w3907:dbl, "VOLTS"=w3897:dbl, "Tmp Live"=w3887:dbl, "Tmp Neut"=w3877:dbl)  [unwired: 1 out]
                n2330 = Unbundle(w3916) -> ("AMPS"=w3906:dbl, "VOLTS"=w3896:dbl, "Tmp Live"=w3886:dbl, "Tmp Neut"=w3876:dbl)  [unwired: 1 out]
                n2331 = stacked-sequence {
                  tunnel: w3907 -> [w3928 _ _ _]
                  tunnel: w3906 -> [w3927 _ _ _]
                  tunnel: w3905 -> [w3926 _ _ _]
                  tunnel: w3904 -> [w3925 _ _ _]
                  tunnel: w3903 -> [w3924 _ _ _]
                  tunnel: w3902 -> [w3923 _ _ _]
                  tunnel: w3901 -> [w3922 _ _ _]
                  tunnel: w3900 -> [w3921 _ _ _]
                  tunnel: w3899 -> [w3920 _ _ _]
                  tunnel: w3898 -> [w3919 _ _ _]
                  tunnel: w3897 -> [_ w3939 _ _]
                  tunnel: w3896 -> [_ w3938 _ _]
                  tunnel: w3895 -> [_ w3937 _ _]
                  tunnel: w3894 -> [_ w3936 _ _]
                  tunnel: w3893 -> [_ w3935 _ _]
                  tunnel: w3892 -> [_ w3934 _ _]
                  tunnel: w3891 -> [_ w3933 _ _]
                  tunnel: w3890 -> [_ w3932 _ _]
                  tunnel: w3889 -> [_ w3931 _ _]
                  tunnel: w3888 -> [_ w3930 _ _]
                  tunnel: w3887 -> [_ _ w3950 _]
                  tunnel: w3886 -> [_ _ w3949 _]
                  tunnel: w3885 -> [_ _ w3948 _]
                  tunnel: w3884 -> [_ _ w3947 _]
                  tunnel: w3883 -> [_ _ w3946 _]
                  tunnel: w3882 -> [_ _ w3945 _]
                  tunnel: w3881 -> [_ _ w3944 _]
                  tunnel: w3880 -> [_ _ w3943 _]
                  tunnel: w3879 -> [_ _ w3942 _]
                  tunnel: w3878 -> [_ _ w3941 _]
                  tunnel: w3877 -> [_ _ _ w3961]
                  tunnel: w3876 -> [_ _ _ w3960]
                  tunnel: w3875 -> [_ _ _ w3959]
                  tunnel: w3874 -> [_ _ _ w3958]
                  tunnel: w3873 -> [_ _ _ w3957]
                  tunnel: w3872 -> [_ _ _ w3956]
                  tunnel: w3871 -> [_ _ _ w3955]
                  tunnel: w3870 -> [_ _ _ w3954]
                  tunnel: w3869 -> [_ _ _ w3953]
                  tunnel: w3868 -> [_ _ _ w3952]
                  frame #0 {
                    n2332 = Bundle("AMPS"=w3928, "AMPS"=w3927, "AMPS"=w3926, "AMPS"=w3925, "AMPS"=w3924, "AMPS"=w3923, "AMPS"=w3922, "AMPS"=w3921, "AMPS"=w3920, "AMPS"=w3919) -> (→"TEST AMPS CHART":T6)  [unwired: 1 in]
                  }
                  frame #1 {
                    n2333 = Bundle("VOLTS"=w3939, "VOLTS"=w3938, "VOLTS"=w3937, "VOLTS"=w3936, "VOLTS"=w3935, "VOLTS"=w3934, "VOLTS"=w3933, "VOLTS"=w3932, "VOLTS"=w3931, "VOLTS"=w3930) -> (→"TEST VOLTS CHART":T30)  [unwired: 1 in]
                  }
                  frame #2 {
                    n2334 = Bundle("Tmp Live"=w3950, "Tmp Live"=w3949, "Tmp Live"=w3948, "Tmp Live"=w3947, "Tmp Live"=w3946, "Tmp Live"=w3945, "Tmp Live"=w3944, "Tmp Live"=w3943, "Tmp Live"=w3942, "Tmp Live"=w3941) -> (→"TEMPERATURE (L) CHART":T31)  [unwired: 1 in]
                  }
                  frame #3 {
                    n2335 = Bundle("Tmp Neut"=w3961, "Tmp Neut"=w3960, "Tmp Neut"=w3959, "Tmp Neut"=w3958, "Tmp Neut"=w3957, "Tmp Neut"=w3956, "Tmp Neut"=w3955, "Tmp Neut"=w3954, "Tmp Neut"=w3953, "Tmp Neut"=w3952) -> (→"TEMPERATURE (N) CHART":T32)  [unwired: 1 in]
                  }
                }
              }
            }
          }
          frame #15 {
            # "check for amps fail"
            # "check for cycle test & temperature rise fail conditions"
            n2336 = local read "on loops"() -> (w3988:dbl)
            n2337 = local read "jig cycle"() -> (w3985:dbl)
            n2338 = local read "jig cycle"() -> (w3990:dbl)
            n2339 = Add(x=w3988, y=3.0) -> (x+y=w3986:dbl)
            n2340 = Equal?(x=w3985, y=w3986) -> (x = y?=w3981:bool)
            n2341 = local read "Fail Loops"() -> (w3962:dbl)
            n2342 = Equal?(x=w3990, y=1.0) -> (x = y?=w3983:bool)
            n2343 = global write "Global 1.vi" "fail count"(w3962) -> ()
            n2344 = stacked-sequence {
              tunnel: w3984 -> [w3993 _ _ _ _ _ _ _ _ _]
              tunnel: w3983 -> [w3994 w4014 w4034 w4054 w4074 w4094 w4114 w4134 w4154 w4174]
              tunnel: w3982 -> [w3991 _ _ _ _ _ _ _ _ _]
              tunnel: w3981 -> [w3992 w4013 w4033 w4053 w4073 w4093 w4113 w4133 w4153 w4173]
              tunnel: w3980 -> [_ w4012 _ _ _ _ _ _ _ _]
              tunnel: w3979 -> [_ w4011 _ _ _ _ _ _ _ _]
              tunnel: w3978 -> [_ _ w4032 _ _ _ _ _ _ _]
              tunnel: w3977 -> [_ _ w4031 _ _ _ _ _ _ _]
              tunnel: w3976 -> [_ _ _ w4052 _ _ _ _ _ _]
              tunnel: w3975 -> [_ _ _ w4051 _ _ _ _ _ _]
              tunnel: w3974 -> [_ _ _ _ w4072 _ _ _ _ _]
              tunnel: w3973 -> [_ _ _ _ w4071 _ _ _ _ _]
              tunnel: w3972 -> [_ _ _ _ _ w4092 _ _ _ _]
              tunnel: w3971 -> [_ _ _ _ _ w4091 _ _ _ _]
              tunnel: w3970 -> [_ _ _ _ _ _ w4112 _ _ _]
              tunnel: w3969 -> [_ _ _ _ _ _ w4111 _ _ _]
              tunnel: w3968 -> [_ _ _ _ _ _ _ w4132 _ _]
              tunnel: w3967 -> [_ _ _ _ _ _ _ w4131 _ _]
              tunnel: w3966 -> [_ _ _ _ _ _ _ _ w4152 _]
              tunnel: w3965 -> [_ _ _ _ _ _ _ _ w4151 _]
              tunnel: w3964 -> [_ _ _ _ _ _ _ _ _ w4172]
              tunnel: w3963 -> [_ _ _ _ _ _ _ _ _ w4171]
              frame #0 {
                # "LAB01-1"
                n2345 = case shown="True" w3991 {
                  tunnel: w3994 -> [_ w4007]
                  tunnel: w3993 -> [_ w4004]
                  tunnel: w3992 -> [_ w4003]
                  frame False {
                  }
                  frame True {
                    n2346 = local read "TEMP START LAB01-1"() -> (w4009:cluster{"TL":dbl, "TN":dbl})
                    n2347 = local read "RESULT LAB01-1"() -> (w3998:bool)
                    n2348 = local read "FAIL LAB01-1"() -> (w4001:cluster{"LO":dbl, "HI":dbl})
                    n2349 = local read "TDMS LAB01-1"() -> (w4008:refnum<k34>)
                    n2350 = local read "SET LAB01-1"() -> (w4005:T5)
                    n2351 = local read "DISP LAB01-1"() -> (w4006:T4)
                    n2352 = local read "SIG LAB01-1"() -> (w4010:T2)
                    n2353 = Bundle("FAIL LAB01-1"=w4001, "SIG LAB01-1"=w4010, "TEMP START LAB01-1"=w4009, "DISP LAB01-1"=w4006, "SET LAB01-1"=w4005, "TDMS LAB01-1"=w4008) -> (w3995:T33)  [unwired: 1 in]
                    n2354 = call "sub vi - cycle&temp fail v6.vi"("Amps Lo?"=w4007, "Input Cluster"=w3995, "SELECT"=w4004, "Amps Hi?"=w4003, "Result In"=w3998) -> ("(FAIL) out"=w4000:cluster{"FAIL LO":dbl, "FAIL HI":dbl}, "(DISP) out"=w3996:T4, "T-RISE"=w3997:cluster{"T-RISE (L)":dbl, "T-RISE (N)":dbl}, "Result Out"=w3999:bool, "file error"=w4002:errorcluster)  [unwired: 10 in]
                    n2355 = local write "TEMP RISE LAB01-1"(w3997) -> ()
                    n2356 = local write "FAIL LAB01-1"(w4000) -> ()
                    n2357 = local write "DISP LAB01-1"(w3996) -> ()
                    n2358 = local write "RESULT LAB01-1"(w3999) -> ()
                    n2359 = local write "data file error"(w4002) -> ()
                  }
                }
              }
              frame #1 {
                # "LAB01-2"
                n2360 = case shown="True" w4012 {
                  tunnel: w4014 -> [_ w4027]
                  tunnel: w4011 -> [_ w4024]
                  tunnel: w4013 -> [_ w4023]
                  frame False {
                  }
                  frame True {
                    n2361 = local read "TEMP START LAB01-2"() -> (w4029:cluster{"TL":dbl, "TN":dbl})
                    n2362 = local read "FAIL LAB01-2"() -> (w4020:cluster{"LO":dbl, "HI":dbl})
                    n2363 = local read "TDMS LAB01-2"() -> (w4028:refnum<k34>)
                    n2364 = local read "SET LAB01-2"() -> (w4025:T5)
                    n2365 = local read "DISP LAB01-2"() -> (w4026:T4)
                    n2366 = local read "RESULT LAB01-2"() -> (w4017:bool)
                    n2367 = local read "SIG LAB01-2"() -> (w4030:T2)
                    n2368 = Bundle("FAIL LAB01-2"=w4020, "SIG LAB01-2"=w4030, "TEMP START LAB01-2"=w4029, "DISP LAB01-2"=w4026, "SET LAB01-2"=w4025, "TDMS LAB01-2"=w4028) -> (w4015:T34)  [unwired: 1 in]
                    n2369 = call "sub vi - cycle&temp fail v6.vi"("Amps Lo?"=w4027, "Input Cluster"=w4015, "SELECT"=w4024, "Amps Hi?"=w4023, "Result In"=w4017) -> ("(FAIL) out"=w4019:cluster{"FAIL LO":dbl, "FAIL HI":dbl}, "(DISP) out"=w4022:T4, "T-RISE"=w4016:cluster{"T-RISE (L)":dbl, "T-RISE (N)":dbl}, "Result Out"=w4018:bool, "file error"=w4021:errorcluster)  [unwired: 10 in]
                    n2370 = local write "TEMP RISE LAB01-2"(w4016) -> ()
                    n2371 = local write "FAIL LAB01-2"(w4019) -> ()
                    n2372 = local write "DISP LAB01-2"(w4022) -> ()
                    n2373 = local write "RESULT LAB01-2"(w4018) -> ()
                    n2374 = local write "data file error"(w4021) -> ()
                  }
                }
              }
              frame #2 {
                # "LAB02-1"
                n2375 = case shown="True" w4032 {
                  tunnel: w4034 -> [_ w4047]
                  tunnel: w4031 -> [_ w4044]
                  tunnel: w4033 -> [_ w4043]
                  frame False {
                  }
                  frame True {
                    n2376 = local read "TEMP START LAB02-1"() -> (w4049:cluster{"TL":dbl, "TN":dbl})
                    n2377 = local read "FAIL LAB02-1"() -> (w4040:cluster{"LO":dbl, "HI":dbl})
                    n2378 = local read "TDMS LAB02-1"() -> (w4048:refnum<k34>)
                    n2379 = local read "SET LAB02-1"() -> (w4045:T5)
                    n2380 = local read "DISP LAB02-1"() -> (w4046:T4)
                    n2381 = local read "SIG LAB02-1"() -> (w4050:T2)
                    n2382 = local read "RESULT LAB02-1"() -> (w4037:bool)
                    n2383 = Bundle("FAIL LAB02-1"=w4040, "SIG LAB02-1"=w4050, "TEMP START LAB02-1"=w4049, "DISP LAB02-1"=w4046, "SET LAB02-1"=w4045, "TDMS LAB02-1"=w4048) -> (w4035:T35)  [unwired: 1 in]
                    n2384 = call "sub vi - cycle&temp fail v6.vi"("Amps Lo?"=w4047, "Input Cluster"=w4035, "SELECT"=w4044, "Amps Hi?"=w4043, "Result In"=w4037) -> ("(FAIL) out"=w4039:cluster{"FAIL LO":dbl, "FAIL HI":dbl}, "(DISP) out"=w4042:T4, "T-RISE"=w4036:cluster{"T-RISE (L)":dbl, "T-RISE (N)":dbl}, "Result Out"=w4038:bool, "file error"=w4041:errorcluster)  [unwired: 10 in]
                    n2385 = local write "TEMP RISE LAB02-1"(w4036) -> ()
                    n2386 = local write "FAIL LAB02-1"(w4039) -> ()
                    n2387 = local write "DISP LAB02-1"(w4042) -> ()
                    n2388 = local write "RESULT LAB02-1"(w4038) -> ()
                    n2389 = local write "data file error"(w4041) -> ()
                  }
                }
              }
              frame #3 {
                # "LAB02-2"
                n2390 = case shown="True" w4052 {
                  tunnel: w4054 -> [_ w4067]
                  tunnel: w4051 -> [_ w4064]
                  tunnel: w4053 -> [_ w4063]
                  frame False {
                  }
                  frame True {
                    n2391 = local read "TEMP START LAB02-2"() -> (w4069:cluster{"TL":dbl, "TN":dbl})
                    n2392 = local read "FAIL LAB02-2"() -> (w4060:cluster{"LO":dbl, "HI":dbl})
                    n2393 = local read "TDMS LAB02-2"() -> (w4068:refnum<k34>)
                    n2394 = local read "SET LAB02-2"() -> (w4065:T5)
                    n2395 = local read "DISP LAB02-2"() -> (w4066:T4)
                    n2396 = local read "SIG LAB02-2"() -> (w4070:T2)
                    n2397 = local read "RESULT LAB02-2"() -> (w4057:bool)
                    n2398 = Bundle("FAIL LAB02-2"=w4060, "SIG LAB02-2"=w4070, "TEMP START LAB02-2"=w4069, "DISP LAB02-2"=w4066, "SET LAB02-2"=w4065, "TDMS LAB02-2"=w4068) -> (w4055:T36)  [unwired: 1 in]
                    n2399 = call "sub vi - cycle&temp fail v6.vi"("Amps Lo?"=w4067, "Input Cluster"=w4055, "SELECT"=w4064, "Amps Hi?"=w4063, "Result In"=w4057) -> ("(FAIL) out"=w4059:cluster{"FAIL LO":dbl, "FAIL HI":dbl}, "(DISP) out"=w4062:T4, "T-RISE"=w4056:cluster{"T-RISE (L)":dbl, "T-RISE (N)":dbl}, "Result Out"=w4058:bool, "file error"=w4061:errorcluster)  [unwired: 10 in]
                    n2400 = local write "TEMP RISE LAB02-2"(w4056) -> ()
                    n2401 = local write "FAIL LAB02-2"(w4059) -> ()
                    n2402 = local write "DISP LAB02-2"(w4062) -> ()
                    n2403 = local write "RESULT LAB02-2"(w4058) -> ()
                    n2404 = local write "data file error"(w4061) -> ()
                  }
                }
              }
              frame #4 {
                # "LAB03-1"
                n2405 = case shown="True" w4072 {
                  tunnel: w4074 -> [_ w4087]
                  tunnel: w4071 -> [_ w4084]
                  tunnel: w4073 -> [_ w4083]
                  frame False {
                  }
                  frame True {
                    n2406 = local read "TEMP START LAB03-1"() -> (w4089:cluster{"TL":dbl, "TN":dbl})
                    n2407 = local read "FAIL LAB03-1"() -> (w4080:cluster{"LO":dbl, "HI":dbl})
                    n2408 = local read "TDMS LAB03-1"() -> (w4088:refnum<k34>)
                    n2409 = local read "SET LAB03-1"() -> (w4085:T5)
                    n2410 = local read "DISP LAB03-1"() -> (w4086:T4)
                    n2411 = local read "SIG LAB03-1"() -> (w4090:T2)
                    n2412 = local read "RESULT LAB03-1"() -> (w4077:bool)
                    n2413 = Bundle("FAIL LAB03-1"=w4080, "SIG LAB03-1"=w4090, "TEMP START LAB03-1"=w4089, "DISP LAB03-1"=w4086, "SET LAB03-1"=w4085, "TDMS LAB03-1"=w4088) -> (w4075:T37)  [unwired: 1 in]
                    n2414 = call "sub vi - cycle&temp fail v6.vi"("Amps Lo?"=w4087, "Input Cluster"=w4075, "SELECT"=w4084, "Amps Hi?"=w4083, "Result In"=w4077) -> ("(FAIL) out"=w4079:cluster{"FAIL LO":dbl, "FAIL HI":dbl}, "(DISP) out"=w4082:T4, "T-RISE"=w4076:cluster{"T-RISE (L)":dbl, "T-RISE (N)":dbl}, "Result Out"=w4078:bool, "file error"=w4081:errorcluster)  [unwired: 10 in]
                    n2415 = local write "TEMP RISE LAB03-1"(w4076) -> ()
                    n2416 = local write "FAIL LAB03-1"(w4079) -> ()
                    n2417 = local write "DISP LAB03-1"(w4082) -> ()
                    n2418 = local write "RESULT LAB03-1"(w4078) -> ()
                    n2419 = local write "data file error"(w4081) -> ()
                  }
                }
              }
              frame #5 {
                # "LAB03-2"
                n2420 = case shown="True" w4092 {
                  tunnel: w4094 -> [_ w4107]
                  tunnel: w4091 -> [_ w4104]
                  tunnel: w4093 -> [_ w4103]
                  frame False {
                  }
                  frame True {
                    n2421 = local read "TEMP START LAB03-2"() -> (w4109:cluster{"TL":dbl, "TN":dbl})
                    n2422 = local read "FAIL LAB03-2"() -> (w4100:cluster{"LO":dbl, "HI":dbl})
                    n2423 = local read "TDMS LAB03-2"() -> (w4108:refnum<k34>)
                    n2424 = local read "SET LAB03-2"() -> (w4105:T5)
                    n2425 = local read "DISP LAB03-2"() -> (w4106:T4)
                    n2426 = local read "RESULT LAB03-2"() -> (w4097:bool)
                    n2427 = local read "SIG LAB03-2"() -> (w4110:T2)
                    n2428 = Bundle("FAIL LAB03-2"=w4100, "SIG LAB03-2"=w4110, "TEMP START LAB03-2"=w4109, "DISP LAB03-2"=w4106, "SET LAB03-2"=w4105, "TDMS LAB03-2"=w4108) -> (w4095:T38)  [unwired: 1 in]
                    n2429 = call "sub vi - cycle&temp fail v6.vi"("Amps Lo?"=w4107, "Input Cluster"=w4095, "SELECT"=w4104, "Amps Hi?"=w4103, "Result In"=w4097) -> ("(FAIL) out"=w4099:cluster{"FAIL LO":dbl, "FAIL HI":dbl}, "(DISP) out"=w4102:T4, "T-RISE"=w4096:cluster{"T-RISE (L)":dbl, "T-RISE (N)":dbl}, "Result Out"=w4098:bool, "file error"=w4101:errorcluster)  [unwired: 10 in]
                    n2430 = local write "FAIL LAB03-2"(w4099) -> ()
                    n2431 = local write "TEMP RISE LAB03-2"(w4096) -> ()
                    n2432 = local write "DISP LAB03-2"(w4102) -> ()
                    n2433 = local write "RESULT LAB03-2"(w4098) -> ()
                    n2434 = local write "data file error"(w4101) -> ()
                  }
                }
              }
              frame #6 {
                # "LAB04-1"
                n2435 = case shown="True" w4112 {
                  tunnel: w4114 -> [_ w4127]
                  tunnel: w4111 -> [_ w4124]
                  tunnel: w4113 -> [_ w4123]
                  frame False {
                  }
                  frame True {
                    n2436 = local read "TEMP START LAB04-1"() -> (w4129:cluster{"TL":dbl, "TN":dbl})
                    n2437 = local read "FAIL LAB04-1"() -> (w4120:cluster{"LO":dbl, "HI":dbl})
                    n2438 = local read "TDMS LAB04-1"() -> (w4128:refnum<k34>)
                    n2439 = local read "SET LAB04-1"() -> (w4125:T5)
                    n2440 = local read "DISP LAB04-1"() -> (w4126:T4)
                    n2441 = local read "SIG LAB04-1"() -> (w4130:T2)
                    n2442 = local read "RESULT LAB04-1"() -> (w4117:bool)
                    n2443 = Bundle("FAIL LAB04-1"=w4120, "SIG LAB04-1"=w4130, "TEMP START LAB04-1"=w4129, "DISP LAB04-1"=w4126, "SET LAB04-1"=w4125, "TDMS LAB04-1"=w4128) -> (w4115:T39)  [unwired: 1 in]
                    n2444 = call "sub vi - cycle&temp fail v6.vi"("Amps Lo?"=w4127, "Input Cluster"=w4115, "SELECT"=w4124, "Amps Hi?"=w4123, "Result In"=w4117) -> ("(FAIL) out"=w4119:cluster{"FAIL LO":dbl, "FAIL HI":dbl}, "(DISP) out"=w4122:T4, "T-RISE"=w4116:cluster{"T-RISE (L)":dbl, "T-RISE (N)":dbl}, "Result Out"=w4118:bool, "file error"=w4121:errorcluster)  [unwired: 10 in]
                    n2445 = local write "TEMP RISE LAB04-1"(w4116) -> ()
                    n2446 = local write "FAIL LAB04-1"(w4119) -> ()
                    n2447 = local write "DISP LAB04-1"(w4122) -> ()
                    n2448 = local write "RESULT LAB04-1"(w4118) -> ()
                    n2449 = local write "data file error"(w4121) -> ()
                  }
                }
              }
              frame #7 {
                # "LAB04-2"
                n2450 = case shown="True" w4132 {
                  tunnel: w4134 -> [_ w4147]
                  tunnel: w4131 -> [_ w4144]
                  tunnel: w4133 -> [_ w4143]
                  frame False {
                  }
                  frame True {
                    n2451 = local read "TEMP START LAB04-2"() -> (w4149:cluster{"TL":dbl, "TN":dbl})
                    n2452 = local read "FAIL LAB04-2"() -> (w4140:cluster{"LO":dbl, "HI":dbl})
                    n2453 = local read "TDMS LAB04-2"() -> (w4148:refnum<k34>)
                    n2454 = local read "SET LAB04-2"() -> (w4145:T5)
                    n2455 = local read "DISP LAB04-2"() -> (w4146:T4)
                    n2456 = local read "SIG LAB04-2"() -> (w4150:T2)
                    n2457 = local read "RESULT LAB04-2"() -> (w4137:bool)
                    n2458 = Bundle("FAIL LAB04-2"=w4140, "SIG LAB04-2"=w4150, "TEMP START LAB04-2"=w4149, "DISP LAB04-2"=w4146, "SET LAB04-2"=w4145, "TDMS LAB04-2"=w4148) -> (w4135:T40)  [unwired: 1 in]
                    n2459 = call "sub vi - cycle&temp fail v6.vi"("Amps Lo?"=w4147, "Input Cluster"=w4135, "SELECT"=w4144, "Amps Hi?"=w4143, "Result In"=w4137) -> ("(FAIL) out"=w4139:cluster{"FAIL LO":dbl, "FAIL HI":dbl}, "(DISP) out"=w4142:T4, "T-RISE"=w4136:cluster{"T-RISE (L)":dbl, "T-RISE (N)":dbl}, "Result Out"=w4138:bool, "file error"=w4141:errorcluster)  [unwired: 10 in]
                    n2460 = local write "TEMP RISE LAB04-2"(w4136) -> ()
                    n2461 = local write "FAIL LAB04-2"(w4139) -> ()
                    n2462 = local write "DISP LAB04-2"(w4142) -> ()
                    n2463 = local write "RESULT LAB04-2"(w4138) -> ()
                    n2464 = local write "data file error"(w4141) -> ()
                  }
                }
              }
              frame #8 {
                # "LAB05-1"
                n2465 = case shown="True" w4152 {
                  tunnel: w4154 -> [_ w4167]
                  tunnel: w4151 -> [_ w4164]
                  tunnel: w4153 -> [_ w4163]
                  frame False {
                  }
                  frame True {
                    n2466 = local read "TEMP START LAB05-1"() -> (w4169:cluster{"TL":dbl, "TN":dbl})
                    n2467 = local read "FAIL LAB05-1"() -> (w4160:cluster{"LO":dbl, "HI":dbl})
                    n2468 = local read "TDMS LAB05-1"() -> (w4168:refnum<k34>)
                    n2469 = local read "SET LAB05-1"() -> (w4165:T5)
                    n2470 = local read "DISP LAB05-1"() -> (w4166:T4)
                    n2471 = local read "SIG LAB05-1"() -> (w4170:T2)
                    n2472 = local read "RESULT LAB05-1"() -> (w4157:bool)
                    n2473 = Bundle("FAIL LAB05-1"=w4160, "SIG LAB05-1"=w4170, "TEMP START LAB05-1"=w4169, "DISP LAB05-1"=w4166, "SET LAB05-1"=w4165, "TDMS LAB05-1"=w4168) -> (w4155:T41)  [unwired: 1 in]
                    n2474 = call "sub vi - cycle&temp fail v6.vi"("Amps Lo?"=w4167, "Input Cluster"=w4155, "SELECT"=w4164, "Amps Hi?"=w4163, "Result In"=w4157) -> ("(FAIL) out"=w4159:cluster{"FAIL LO":dbl, "FAIL HI":dbl}, "(DISP) out"=w4162:T4, "T-RISE"=w4156:cluster{"T-RISE (L)":dbl, "T-RISE (N)":dbl}, "Result Out"=w4158:bool, "file error"=w4161:errorcluster)  [unwired: 10 in]
                    n2475 = local write "TEMP RISE LAB05-1"(w4156) -> ()
                    n2476 = local write "FAIL LAB05-1"(w4159) -> ()
                    n2477 = local write "DISP LAB05-1"(w4162) -> ()
                    n2478 = local write "RESULT LAB05-1"(w4158) -> ()
                    n2479 = local write "data file error"(w4161) -> ()
                  }
                }
              }
              frame #9 {
                # "LAB05-2"
                n2480 = case shown="True" w4172 {
                  tunnel: w4174 -> [_ w4187]
                  tunnel: w4171 -> [_ w4184]
                  tunnel: w4173 -> [_ w4183]
                  frame False {
                  }
                  frame True {
                    n2481 = local read "TEMP START LAB05-2"() -> (w4189:cluster{"TL":dbl, "TN":dbl})
                    n2482 = local read "FAIL LAB05-2"() -> (w4180:cluster{"LO":dbl, "HI":dbl})
                    n2483 = local read "TDMS LAB05-2"() -> (w4188:refnum<k34>)
                    n2484 = local read "SET LAB05-2"() -> (w4185:T5)
                    n2485 = local read "DISP LAB05-2"() -> (w4186:T4)
                    n2486 = local read "SIG LAB05-2"() -> (w4190:T2)
                    n2487 = local read "RESULT LAB05-2"() -> (w4177:bool)
                    n2488 = Bundle("FAIL LAB05-2"=w4180, "SIG LAB05-2"=w4190, "TEMP START LAB05-2"=w4189, "DISP LAB05-2"=w4186, "SET LAB05-2"=w4185, "TDMS LAB05-2"=w4188) -> (w4175:T42)  [unwired: 1 in]
                    n2489 = call "sub vi - cycle&temp fail v6.vi"("Amps Lo?"=w4187, "Input Cluster"=w4175, "SELECT"=w4184, "Amps Hi?"=w4183, "Result In"=w4177) -> ("(FAIL) out"=w4179:cluster{"FAIL LO":dbl, "FAIL HI":dbl}, "(DISP) out"=w4182:T4, "T-RISE"=w4176:cluster{"T-RISE (L)":dbl, "T-RISE (N)":dbl}, "Result Out"=w4178:bool, "file error"=w4181:errorcluster)  [unwired: 10 in]
                    n2490 = local write "TEMP RISE LAB05-2"(w4176) -> ()
                    n2491 = local write "FAIL LAB05-2"(w4179) -> ()
                    n2492 = local write "DISP LAB05-2"(w4182) -> ()
                    n2493 = local write "RESULT LAB05-2"(w4178) -> ()
                    n2494 = local write "data file error"(w4181) -> ()
                  }
                }
              }
            }
          }
          frame #16 {
            # "run calibration routine"
            n2495 = local read "CALIBRATE"() -> (w4191:bool)
            n2496 = case shown="True" w4191 {
              frame False {
              }
              frame True {
                n2497 = stacked-sequence {
                  seq-local: [w4192 _ _] -> [_ w4194 _]
                  frame #0 {
                    n2498 = call "CALIBRATION PASSWORD"() -> ("PASSWORD"=w4192:string)  [unwired: 17 in, 2 out]
                  }
                  frame #1 {
                    n2499 = Equal?(x=w4194, y="7777") -> (x = y?=w4193:bool)
                    n2500 = case shown="True" w4193 {
                      frame False {
                      }
                      frame True {
                        n2501 = stacked-sequence {
                          frame #0 {
                            n2502 = call "sub vi - calibration v1.vi"() -> ()  [unwired: 12 in]
                          }
                          frame #1 {
                            n2503 = call "sub vi - get calibration values v1.vi"() -> ("LAB01 (CAL)"=w4200:T8, "LAB02 (CAL)"=w4199:T9, "LAB03 (CAL)"=w4198:T8, "LAB04 (CAL)"=w4197:T8, "calibration file error out"=w4201:errorcluster, "LAB05 (CAL)"=w4196:T8)  [unwired: 10 in]
                            n2504 = local write "calibration file error out"(w4201) -> ()
                            n2505 = local write "CAL LAB04"(w4197) -> ()
                            n2506 = local write "CAL LAB05"(w4196) -> ()
                            n2507 = local write "CAL LAB01"(w4200) -> ()
                            n2508 = local write "CAL LAB02"(w4199) -> ()
                            n2509 = local write "CAL LAB03"(w4198) -> ()
                          }
                        }
                      }
                    }
                  }
                  frame #2 {
                    n2510 = local write "CALIBRATE"(FALSE) -> ()
                  }
                }
              }
            }
          }
          frame #17 {
            # "save certain settings to file"
            n2511 = String To Path(string="c:\\crabtree\\Set Up\\") -> (path=w4204:path)
            n2512 = Build Path(base path=w4204, name or relative path="settings.bin") -> (appended path=w4206:path)
            n2513 = Build Path(base path=w4204, name or relative path="mail.bin") -> (appended path=w4203:path)
            n2514 = Create Folder(path (use dialog)=w4204) -> (error out=w4209:errorcluster)  [unwired: 2 in, 2 out]
            n2515 = call <vilib>:"Clear Errors.vi"("error in (no error)"=w4209) -> ()  [unwired: 6 in, 1 out]
            n2516 = stacked-sequence {
              seq-local: [w4217 _] -> [_ w4230]
              tunnel: w4206 -> [_ w4231]
              tunnel: w4203 -> [_ w4229]
              frame #0 {
                n2517 = local read "C drive data root dir"() -> (w4216:path)
                n2518 = local read "Select COM port"() -> (w4213:refnum<visa-resource-name>)
                n2519 = local read "Network Directory"() -> (w4222:path)
                n2520 = local read "SET LAB05-2"() -> (w4221:T5)
                n2521 = local read "SET LAB05-1"() -> (w4220:T5)
                n2522 = local read "SET LAB04-2"() -> (w4219:T5)
                n2523 = local read "SET LAB03-2"() -> (w4223:T5)
                n2524 = local read "SET LAB04-1"() -> (w4218:T5)
                n2525 = local read "SET LAB03-1"() -> (w4224:T5)
                n2526 = local read "SET LAB02-2"() -> (w4225:T5)
                n2527 = local read "SET LAB02-1"() -> (w4226:T5)
                n2528 = local read "Temp Delay Lps"() -> (w4212:dbl)
                n2529 = local read "SET LAB01-2"() -> (w4227:T5)
                n2530 = local read "SET LAB01-1"() -> (w4228:T5)
                n2531 = local read "Temp Value"() -> (w4211:dbl)
                n2532 = local read "Fail Loops"() -> (w4210:dbl)
                n2533 = local read "RATE (Hz)"() -> (w4215:dbl)
                n2534 = local read "SAMPLES"() -> (w4214:dbl)
                n2535 = Bundle("SET LAB01-1"=w4228, "SET LAB01-2"=w4227, "SET LAB02-1"=w4226, "SET LAB02-2"=w4225, "SET LAB03-1"=w4224, "SET LAB03-2"=w4223, "SET LAB04-1"=w4218, "SET LAB04-2"=w4219, "SET LAB05-1"=w4220, "SET LAB05-2"=w4221, "Network Directory"=w4222, "C drive data root dir"=w4216, "RATE (Hz)"=w4215, "SAMPLES"=w4214, "Select COM port"=w4213, "Temp Delay Lps"=w4212, "Temp Value"=w4211, "Fail Loops"=w4210) -> (w4217:T21)  [unwired: 1 in]
              }
              frame #1 {
                n2536 = event shown="[2] \"MAIL SETTINGS.OUT SERVER ADDRESS\", \"MAIL SETTINGS.FROM ACCOUNT\", \"MAIL SETTINGS.USER NAME\", \"MAIL SETTINGS.PASSWORD\", \"Auto Mail Send\", \"TO (string):\": Value Change" {
                  selector: _ -> [_ _ _]
                  dyn-events: _ -> [_ _ _]
                  timeout: 10.0 -> [_ _ _]
                  tunnel: w4231 -> [_ w4233 _]
                  tunnel: w4230 -> [_ w4234 _]
                  tunnel: w4229 -> [_ _ w4245]
                  event Timeout {
                    n2537 = event-data() -> ()  [unwired: 1 in, 3 out]
                  }
                  event "SET LAB01-1", "SET LAB01-2", "SET LAB02-1", "SET LAB02-2", "SET LAB03-1", "SET LAB03-2", "SET LAB04-1", "SET LAB04-2", "SET LAB05-1", "SET LAB05-2", "Network Directory", "C drive data root dir", "RATE (Hz)", "SAMPLES", "Select COM port", "Temp Delay Lps", "Temp Value", "Fail Loops": Value Change {
                    n2538 = event-data() -> ()  [unwired: 1 in, 6 out]
                    n2539 = Open/Create/Replace File(file path (use dialog)=w4233, operation (0:open)=T20."replace or create") -> (refnum out=w4239:refnum<file>, error out=w4238:errorcluster)  [unwired: 4 in, 1 out]
                    n2540 = Write to Binary File(file (use dialog)=w4239, data=w4234, error in=w4238) -> (refnum out=w4237:refnum<file>, error out=w4236:errorcluster)  [unwired: 3 in, 1 out]
                    n2541 = Close File(refnum=w4237, error in=w4236) -> (error out=w4235:errorcluster)  [unwired: 1 out]
                    n2542 = local write "data file error"(w4235) -> ()
                  }
                  event "MAIL SETTINGS.OUT SERVER ADDRESS", "MAIL SETTINGS.FROM ACCOUNT", "MAIL SETTINGS.USER NAME", "MAIL SETTINGS.PASSWORD", "Auto Mail Send", "TO (string):": Value Change {
                    n2543 = event-data() -> ()  [unwired: 1 in, 6 out]
                    n2544 = local read "MAIL SETTINGS"() -> (w4244:T7)
                    n2545 = local read "Auto Mail Send"() -> (w4242:bool)
                    n2546 = local read "TO (string):"() -> (w4241:string)
                    n2547 = Open/Create/Replace File(file path (use dialog)=w4245, operation (0:open)=T20."replace or create") -> (refnum out=w4250:refnum<file>, error out=w4249:errorcluster)  [unwired: 4 in, 1 out]
                    n2548 = Bundle("MAIL SETTINGS"=w4244, "Auto Mail Send"=w4242, "TO (string):"=w4241) -> (w4243:T43)  [unwired: 1 in]
                    n2549 = Write to Binary File(file (use dialog)=w4250, data=w4243, error in=w4249) -> (refnum out=w4248:refnum<file>, error out=w4247:errorcluster)  [unwired: 3 in, 1 out]
                    n2550 = Close File(refnum=w4248, error in=w4247) -> (error out=w4246:errorcluster)  [unwired: 1 out]
                    n2551 = local write "data file error"(w4246) -> ()
                  }
                }
              }
            }
          }
          frame #18 {
            # "mail control"
            n2552 = local read "MAIL SETTINGS"() -> (w4267:T7)
            n2553 = local read "Auto Mail Send"() -> (w4253:bool)
            n2554 = Unbundle(w4267) -> ("OUT SERVER ADDRESS"=w4266:string, "FROM ACCOUNT"=w4265:string, "TEST MAIL"=w4264:bool)  [unwired: 4 out]
            n2555 = stacked-sequence {
              tunnel: "TO (string):" -> [_ w4306]
              tunnel: w4267 -> [w4272 w4305]
              tunnel: w4266 -> [w4271 w4304]
              tunnel: w4265 -> [w4270 w4303]
              tunnel: w4264 -> [w4269 _]
              tunnel: w4253 -> [_ w4302]
              tunnel: w4263 -> [_ w4301]
              tunnel: w4262 -> [_ w4300]
              tunnel: w4261 -> [_ w4299]
              tunnel: w4260 -> [_ w4298]
              tunnel: w4259 -> [_ w4297]
              tunnel: w4258 -> [_ w4296]
              tunnel: w4257 -> [_ w4295]
              tunnel: w4256 -> [_ w4294]
              tunnel: w4255 -> [_ w4293]
              tunnel: w4254 -> [_ w4292]
              tunnel: "TO (string):" -> [w4268 _]
              frame #0 {
                # "mail test"
                n2556 = case shown="True" w4269 {
                  tunnel: w4272 -> [_ w4276]
                  tunnel: w4268 -> [_ w4275]
                  tunnel: w4271 -> [_ w4274]
                  tunnel: w4270 -> [_ w4273]
                  frame False {
                  }
                  frame True {
                    n2557 = stacked-sequence {
                      seq-local: [_ _ w4286 _] -> [_ _ _ w4287]
                      tunnel: w4276 -> [w4279 _ _ w4291]
                      tunnel: w4275 -> [_ _ w4284 _]
                      tunnel: w4274 -> [_ _ w4282 _]
                      tunnel: w4273 -> [_ _ w4283 _]
                      frame #0 {
                        n2558 = Bundle(cluster=w4279, "TEST MAIL STATUS"="TEST START") -> (w4277:T7)  [unwired: 6 in]
                        n2559 = local write "MAIL SETTINGS"(w4277) -> ()
                      }
                      frame #1 {
                        n2560 = Wait (ms)(milliseconds to wait=500) -> ()  [unwired: 1 out]
                      }
                      frame #2 {
                        n2561 = call "sub vi - send mail with attach v5.vi"("TO:"=w4284, "subject"="MAIL TEST FROM LAB PANEL", "from"=w4283, "out going server"=w4282, "message"="TEST MESSAGE") -> ("error out"=w4286:errorcluster)  [unwired: 10 in]
                      }
                      frame #3 {
                        n2562 = Bundle(cluster=w4291, "TEST MAIL"=FALSE, "TEST MAIL STATUS"="TEST END", "mail error"=w4287) -> (w4289:T7)  [unwired: 4 in]
                        n2563 = local write "MAIL SETTINGS"(w4289) -> ()
                      }
                    }
                  }
                }
              }
              frame #1 {
                # "mail report"
                n2564 = stacked-sequence {
                  seq-local: [_ w4371 _ _] -> [_ _ _ w4539]
                  seq-local: [_ _ w4452 _] -> [_ _ _ w4529]
                  seq-local: [w4316 _ _ _] -> [_ w4365 _ _]
                  seq-local: [w4315 _ _ _] -> [_ w4364 _ _]
                  seq-local: [w4313 _ _ _] -> [_ w4362 _ _]
                  seq-local: [w4314 _ _ _] -> [_ w4363 _ _]
                  seq-local: [w4312 _ _ _] -> [_ w4361 _ _]
                  seq-local: [w4311 _ _ _] -> [_ w4356 _ _]
                  seq-local: [w4310 _ _ _] -> [_ w4357 _ _]
                  seq-local: [w4309 _ _ _] -> [_ w4358 _ _]
                  seq-local: [w4308 _ _ _] -> [_ w4359 _ _]
                  seq-local: [w4307 _ _ _] -> [_ w4360 _ _]
                  tunnel: w4306 -> [_ _ _ w4540]
                  tunnel: w4305 -> [_ _ _ w4523]
                  tunnel: w4304 -> [_ _ _ w4537]
                  tunnel: w4303 -> [_ _ _ w4536]
                  tunnel: w4302 -> [w4347 _ _ w4531]
                  tunnel: w4301 -> [_ _ w4482 _]
                  tunnel: w4300 -> [_ _ w4479 _]
                  tunnel: w4299 -> [_ _ w4478 _]
                  tunnel: w4298 -> [_ _ w4477 _]
                  tunnel: w4297 -> [_ _ w4476 _]
                  tunnel: w4296 -> [_ _ w4475 _]
                  tunnel: w4295 -> [_ _ w4474 _]
                  tunnel: w4294 -> [_ _ w4473 _]
                  tunnel: w4293 -> [_ _ w4472 _]
                  tunnel: w4292 -> [_ _ w4471 _]
                  frame #0 {
                    n2565 = case shown="False" w4347 {
                      frame False {
                        n2566 = local write "mail control"("") -> ()
                      }
                      frame True {
                      }
                    }
                    n2567 = local read "SET LAB01-1"() -> (w4346:T5)
                    n2568 = local read "SET LAB01-2"() -> (w4345:T5)
                    n2569 = local read "SET LAB02-1"() -> (w4344:T5)
                    n2570 = local read "SET LAB02-2"() -> (w4343:T5)
                    n2571 = local read "SET LAB03-1"() -> (w4342:T5)
                    n2572 = local read "SET LAB04-1"() -> (w4340:T5)
                    n2573 = local read "SET LAB05-1"() -> (w4338:T5)
                    n2574 = local read "SET LAB03-2"() -> (w4341:T5)
                    n2575 = local read "SET LAB04-2"() -> (w4339:T5)
                    n2576 = local read "SET LAB05-2"() -> (w4337:T5)
                    n2577 = Unbundle(w4342) -> ("DESCRIPTION"=w4322:string)  [unwired: 4 out]
                    n2578 = Unbundle(w4341) -> ("DESCRIPTION"=w4321:string)  [unwired: 4 out]
                    n2579 = Unbundle(w4340) -> ("DESCRIPTION"=w4320:string)  [unwired: 4 out]
                    n2580 = Unbundle(w4337) -> ("DESCRIPTION"=w4317:string)  [unwired: 4 out]
                    n2581 = Unbundle(w4343) -> ("DESCRIPTION"=w4323:string)  [unwired: 4 out]
                    n2582 = Unbundle(w4339) -> ("DESCRIPTION"=w4319:string)  [unwired: 4 out]
                    n2583 = Unbundle(w4346) -> ("DESCRIPTION"=w4335:string)  [unwired: 4 out]
                    n2584 = Unbundle(w4344) -> ("DESCRIPTION"=w4324:string)  [unwired: 4 out]
                    n2585 = Unbundle(w4338) -> ("DESCRIPTION"=w4318:string)  [unwired: 4 out]
                    n2586 = Unbundle(w4345) -> ("DESCRIPTION"=w4325:string)  [unwired: 4 out]
                    n2587 = Concatenate Strings("[LAB05-2/", w4317) -> (w4307:string)
                    n2588 = Concatenate Strings("[LAB05-1/", w4318) -> (w4308:string)
                    n2589 = Concatenate Strings("[LAB04-2/", w4319) -> (w4309:string)
                    n2590 = Concatenate Strings("[LAB03-2/", w4321) -> (w4311:string)
                    n2591 = Concatenate Strings("[LAB04-1/", w4320) -> (w4310:string)
                    n2592 = Concatenate Strings("[LAB03-1/", w4322) -> (w4312:string)
                    n2593 = Concatenate Strings("[LAB01-2/", w4325) -> (w4315:string)
                    n2594 = Concatenate Strings("[LAB02-2/", w4323) -> (w4313:string)
                    n2595 = Concatenate Strings("[LAB01-1/", w4335) -> (w4316:string)
                    n2596 = Concatenate Strings("[LAB02-1/", w4324) -> (w4314:string)
                  }
                  frame #1 {
                    w4369 = "/"
                    w4370 = 2.0
                    n2597 = local read "DISP LAB01-2"() -> (w4450:T4)
                    n2598 = local read "DISP LAB01-1"() -> (w4451:T4)
                    n2599 = local read "DISP LAB02-1"() -> (w4449:T4)
                    n2600 = local read "DISP LAB03-2"() -> (w4446:T4)
                    n2601 = local read "DISP LAB02-2"() -> (w4448:T4)
                    n2602 = local read "DISP LAB03-1"() -> (w4447:T4)
                    n2603 = local read "DISP LAB04-2"() -> (w4444:T4)
                    n2604 = local read "DISP LAB04-1"() -> (w4445:T4)
                    n2605 = local read "DISP LAB05-1"() -> (w4443:T4)
                    n2606 = local read "DISP LAB05-2"() -> (w4442:T4)
                    n2607 = Unbundle(w4450) -> ("CYCLE"=w4434:dbl, "MINS"=w4433:dbl, "STATUS"=w4430:string)
                    n2608 = Unbundle(w4451) -> ("CYCLE"=w4439:dbl, "MINS"=w4438:dbl, "STATUS"=w4435:string)
                    n2609 = Unbundle(w4449) -> ("CYCLE"=w4427:dbl, "MINS"=w4426:dbl, "STATUS"=w4425:string)
                    n2610 = Unbundle(w4446) -> ("CYCLE"=w4414:dbl, "MINS"=w4413:dbl, "STATUS"=w4410:string)
                    n2611 = Unbundle(w4447) -> ("CYCLE"=w4419:dbl, "MINS"=w4418:dbl, "STATUS"=w4415:string)
                    n2612 = Unbundle(w4448) -> ("CYCLE"=w4424:dbl, "MINS"=w4423:dbl, "STATUS"=w4420:string)
                    n2613 = Unbundle(w4445) -> ("CYCLE"=w4409:dbl, "MINS"=w4408:dbl, "STATUS"=w4405:string)
                    n2614 = Unbundle(w4444) -> ("CYCLE"=w4404:dbl, "MINS"=w4403:dbl, "STATUS"=w4400:string)
                    n2615 = Unbundle(w4443) -> ("CYCLE"=w4399:dbl, "MINS"=w4398:dbl, "STATUS"=w4395:string)
                    n2616 = Unbundle(w4442) -> ("CYCLE"=w4441:dbl, "MINS"=w4440:dbl, "STATUS"=w4392:string)
                    n2617 = Number To Decimal String(number=w4427) -> (decimal integer string=w4429:string)  [unwired: 1 in]
                    n2618 = Number To Decimal String(number=w4424) -> (decimal integer string=w4422:string)  [unwired: 1 in]
                    n2619 = Number To Decimal String(number=w4419) -> (decimal integer string=w4417:string)  [unwired: 1 in]
                    n2620 = Number To Decimal String(number=w4434) -> (decimal integer string=w4432:string)  [unwired: 1 in]
                    n2621 = Number To Decimal String(number=w4414) -> (decimal integer string=w4412:string)  [unwired: 1 in]
                    n2622 = Number To Decimal String(number=w4439) -> (decimal integer string=w4437:string)  [unwired: 1 in]
                    n2623 = Number To Decimal String(number=w4441) -> (decimal integer string=w4394:string)  [unwired: 1 in]
                    n2624 = Number To Decimal String(number=w4409) -> (decimal integer string=w4407:string)  [unwired: 1 in]
                    n2625 = Number To Decimal String(number=w4404) -> (decimal integer string=w4402:string)  [unwired: 1 in]
                    n2626 = Number To Decimal String(number=w4399) -> (decimal integer string=w4397:string)  [unwired: 1 in]
                    n2627 = Number To Fractional String(number=w4426, precision (6)=w4370) -> (F-format string=w4428:string)  [unwired: 2 in]
                    n2628 = Number To Fractional String(number=w4413, precision (6)=w4370) -> (F-format string=w4411:string)  [unwired: 2 in]
                    n2629 = Number To Fractional String(number=w4423, precision (6)=w4370) -> (F-format string=w4421:string)  [unwired: 2 in]
                    n2630 = Number To Fractional String(number=w4418, precision (6)=w4370) -> (F-format string=w4416:string)  [unwired: 2 in]
                    n2631 = Number To Fractional String(number=w4403, precision (6)=w4370) -> (F-format string=w4401:string)  [unwired: 2 in]
                    n2632 = Number To Fractional String(number=w4408, precision (6)=w4370) -> (F-format string=w4406:string)  [unwired: 2 in]
                    n2633 = Number To Fractional String(number=w4433, precision (6)=w4370) -> (F-format string=w4431:string)  [unwired: 2 in]
                    n2634 = Number To Fractional String(number=w4398, precision (6)=w4370) -> (F-format string=w4396:string)  [unwired: 2 in]
                    n2635 = Number To Fractional String(number=w4438, precision (6)=w4370) -> (F-format string=w4436:string)  [unwired: 2 in]
                    n2636 = Number To Fractional String(number=w4440, precision (6)=w4370) -> (F-format string=w4393:string)  [unwired: 2 in]
                    n2637 = Concatenate Strings(w4369, w4412, w4369, w4411, w4369, w4410) -> (w4386:string)
                    n2638 = Concatenate Strings(w4369, w4407, w4369, w4406, w4369, w4405) -> (w4385:string)
                    n2639 = Concatenate Strings(w4369, w4402, w4369, w4401, w4369, w4400) -> (w4384:string)
                    n2640 = Concatenate Strings(w4369, w4397, w4369, w4396, w4369, w4395) -> (w4383:string)
                    n2641 = Concatenate Strings(w4369, w4394, w4369, w4393, w4369, w4392) -> (w4382:string)
                    n2642 = Concatenate Strings(w4369, w4437, w4369, w4436, w4369, w4435) -> (w4391:string)
                    n2643 = Concatenate Strings(w4369, w4417, w4369, w4416, w4369, w4415) -> (w4387:string)
                    n2644 = Concatenate Strings(w4369, w4432, w4369, w4431, w4369, w4430) -> (w4390:string)
                    n2645 = Concatenate Strings(w4369, w4429, w4369, w4428, w4369, w4425) -> (w4389:string)
                    n2646 = Concatenate Strings(w4369, w4422, w4369, w4421, w4369, w4420) -> (w4388:string)
                    n2647 = Concatenate Strings("]", "\r") -> (w4366:string)
                    n2648 = Concatenate Strings(w4361, w4387, w4366) -> (w4377:string)
                    n2649 = Concatenate Strings(w4363, w4389, w4366) -> (w4379:string)
                    n2650 = Concatenate Strings(w4362, w4388, w4366) -> (w4378:string)
                    n2651 = Concatenate Strings(w4358, w4384, w4366) -> (w4374:string)
                    n2652 = Concatenate Strings(w4359, w4383, w4366) -> (w4375:string)
                    n2653 = Concatenate Strings(w4357, w4385, w4366) -> (w4373:string)
                    n2654 = Concatenate Strings(w4356, w4386, w4366) -> (w4372:string)
                    n2655 = Concatenate Strings(w4360, w4382, w4366) -> (w4376:string)
                    n2656 = Concatenate Strings(w4364, w4390, w4366) -> (w4380:string)
                    n2657 = Concatenate Strings(w4365, w4391, w4366) -> (w4381:string)
                    n2658 = Concatenate Strings(w4381, w4380, w4379, w4378, w4377, w4372, w4373, w4374, w4375, w4376) -> (w4349:string)
                    n2659 = Concatenate Strings("[PANEL/", "DESC/", "CYCLES/", "MINS/", "STATUS]", "\r", w4349) -> (w4371:string)
                    "MAIL REPORT" <- w4371
                  }
                  frame #2 {
                    w4480 = "END"
                    n2660 = local read "mail control"() -> (w4481:string)
                    n2661 = case shown="False" w4476 {
                      tunnel: w4481 -> [w4505 _]
                      tunnel: w4480 -> [w4504 _]
                      tunnel: [w4503 FALSE] -> w4466
                      frame False {
                        n2662 = Equal?(x=w4505, y=w4504) -> (x = y?=w4503:bool)
                      }
                      frame True {
                      }
                    }
                    n2663 = case shown="False" w4482 {
                      tunnel: w4481 -> [w4521 _]
                      tunnel: w4480 -> [w4520 _]
                      tunnel: [w4519 FALSE] -> w4470
                      frame False {
                        n2664 = Equal?(x=w4521, y=w4520) -> (x = y?=w4519:bool)
                      }
                      frame True {
                      }
                    }
                    n2665 = case shown="False" w4479 {
                      tunnel: w4481 -> [w4517 _]
                      tunnel: w4480 -> [w4516 _]
                      tunnel: [w4515 FALSE] -> w4469
                      frame False {
                        n2666 = Equal?(x=w4517, y=w4516) -> (x = y?=w4515:bool)
                      }
                      frame True {
                      }
                    }
                    n2667 = case shown="False" w4477 {
                      tunnel: w4481 -> [w4509 _]
                      tunnel: w4480 -> [w4508 _]
                      tunnel: [w4507 FALSE] -> w4467
                      frame False {
                        n2668 = Equal?(x=w4509, y=w4508) -> (x = y?=w4507:bool)
                      }
                      frame True {
                      }
                    }
                    n2669 = case shown="False" w4478 {
                      tunnel: w4481 -> [w4513 _]
                      tunnel: w4480 -> [w4512 _]
                      tunnel: [w4511 FALSE] -> w4468
                      frame False {
                        n2670 = Equal?(x=w4513, y=w4512) -> (x = y?=w4511:bool)
                      }
                      frame True {
                      }
                    }
                    n2671 = Or(x=w4468, y=w4467) -> (x .or. y?=w4459:bool)
                    n2672 = Or(x=w4470, y=w4469) -> (x .or. y?=w4460:bool)
                    n2673 = Or(x=w4460, y=w4459) -> (x .or. y?=w4455:bool)
                    n2674 = case shown="False" w4472 {
                      tunnel: w4481 -> [w4489 _]
                      tunnel: w4480 -> [w4488 _]
                      tunnel: [w4487 FALSE] -> w4461
                      frame False {
                        n2675 = Equal?(x=w4489, y=w4488) -> (x = y?=w4487:bool)
                      }
                      frame True {
                      }
                    }
                    n2676 = case shown="False" w4471 {
                      tunnel: w4481 -> [w4485 _]
                      tunnel: w4480 -> [w4484 _]
                      tunnel: [w4483 FALSE] -> w4465
                      frame False {
                        n2677 = Equal?(x=w4485, y=w4484) -> (x = y?=w4483:bool)
                      }
                      frame True {
                      }
                    }
                    n2678 = case shown="False" w4473 {
                      tunnel: w4481 -> [w4493 _]
                      tunnel: w4480 -> [w4492 _]
                      tunnel: [w4491 FALSE] -> w4462
                      frame False {
                        n2679 = Equal?(x=w4493, y=w4492) -> (x = y?=w4491:bool)
                      }
                      frame True {
                      }
                    }
                    n2680 = case shown="False" w4475 {
                      tunnel: w4481 -> [w4501 _]
                      tunnel: w4480 -> [w4500 _]
                      tunnel: [w4499 FALSE] -> w4464
                      frame False {
                        n2681 = Equal?(x=w4501, y=w4500) -> (x = y?=w4499:bool)
                      }
                      frame True {
                      }
                    }
                    n2682 = case shown="False" w4474 {
                      tunnel: w4481 -> [w4497 _]
                      tunnel: w4480 -> [w4496 _]
                      tunnel: [w4495 FALSE] -> w4463
                      frame False {
                        n2683 = Equal?(x=w4497, y=w4496) -> (x = y?=w4495:bool)
                      }
                      frame True {
                      }
                    }
                    n2684 = Or(x=w4464, y=w4463) -> (x .or. y?=w4458:bool)
                    n2685 = Or(x=w4462, y=w4461) -> (x .or. y?=w4457:bool)
                    n2686 = Or(x=w4465, y=w4466) -> (x .or. y?=w4453:bool)
                    n2687 = Or(x=w4458, y=w4457) -> (x .or. y?=w4456:bool)
                    n2688 = Or(x=w4455, y=w4456) -> (x .or. y?=w4454:bool)
                    n2689 = Or(x=w4454, y=w4453) -> (x .or. y?=w4452:bool)
                  }
                  frame #3 {
                    n2690 = local read "on loops"() -> (w4535:dbl)
                    n2691 = local read "jig cycle"() -> (w4532:dbl)
                    n2692 = local read "Send Mail Now"() -> (w4526:bool)
                    n2693 = Add(x=w4535, y=3.0) -> (x+y=w4533:dbl)
                    n2694 = Equal?(x=w4532, y=w4533) -> (x = y?=w4527:bool)
                    n2695 = And(x=w4527, y=w4526) -> (x .and. y?=w4525:bool)
                    n2696 = And(x=w4531, y=w4527) -> (x .and. y?=w4530:bool)
                    n2697 = And(x=w4530, y=w4529) -> (x .and. y?=w4528:bool)
                    n2698 = Or(x=w4528, y=w4525) -> (x .or. y?=w4524:bool)
                    n2699 = case shown="True" w4524 {
                      tunnel: w4540 -> [_ w4546]
                      tunnel: w4539 -> [_ w4545]
                      tunnel: "Lab Panel Test Status" -> [_ w4544]
                      tunnel: w4537 -> [_ w4543]
                      tunnel: w4536 -> [_ w4542]
                      tunnel: w4523 -> [_ w4541]
                      frame False {
                      }
                      frame True {
                        n2700 = stacked-sequence {
                          tunnel: w4546 -> [w4554 _]
                          tunnel: w4545 -> [w4553 _]
                          tunnel: w4544 -> [w4552 _]
                          tunnel: w4543 -> [w4551 _]
                          tunnel: w4542 -> [w4550 _]
                          tunnel: w4541 -> [w4549 _]
                          frame #0 {
                            n2701 = call "sub vi - send mail with attach v5.vi"("TO:"=w4554, "subject"=w4552, "from"=w4550, "out going server"=w4551, "message"=w4553) -> ("error out"=w4548:errorcluster)  [unwired: 10 in]
                            n2702 = Bundle(cluster=w4549, "mail error"=w4548) -> (w4547:T7)  [unwired: 6 in]
                            n2703 = local write "MAIL SETTINGS"(w4547) -> ()
                          }
                          frame #1 {
                            n2704 = local write "mail control"("") -> ()
                            n2705 = local write "Send Mail Now"(FALSE) -> ()
                          }
                        }
                      }
                    }
                  }
                }
              }
            }
          }
          frame #19 {
            # "save jig cycle values once all run switches are off"
            n2706 = stacked-sequence {
              tunnel: w4566 -> [_ w4595]
              tunnel: w4565 -> [_ w4594]
              tunnel: w4564 -> [_ w4593]
              tunnel: w4563 -> [_ w4592]
              tunnel: w4562 -> [_ w4591]
              tunnel: w4561 -> [_ w4590]
              tunnel: w4560 -> [_ w4589]
              tunnel: w4559 -> [_ w4588]
              tunnel: w4558 -> [_ w4587]
              tunnel: w4557 -> [_ w4586]
              frame #0 {
              }
              frame #1 {
                n2707 = Not(x=w4586) -> (.not. x?=w4569:bool)
                n2708 = Not(x=w4594) -> (.not. x?=w4584:bool)
                n2709 = Not(x=w4591) -> (.not. x?=w4579:bool)
                n2710 = Not(x=w4589) -> (.not. x?=w4575:bool)
                n2711 = Not(x=w4587) -> (.not. x?=w4571:bool)
                n2712 = Not(x=w4595) -> (.not. x?=w4585:bool)
                n2713 = Not(x=w4593) -> (.not. x?=w4583:bool)
                n2714 = Not(x=w4590) -> (.not. x?=w4577:bool)
                n2715 = Not(x=w4592) -> (.not. x?=w4581:bool)
                n2716 = Not(x=w4588) -> (.not. x?=w4573:bool)
                n2717 = local read "Save JC"() -> (w4597:bool)
                n2718 = And(x=w4585, y=w4584) -> (x .and. y?=w4582:bool)
                n2719 = And(x=w4582, y=w4583) -> (x .and. y?=w4580:bool)
                n2720 = And(x=w4580, y=w4581) -> (x .and. y?=w4578:bool)
                n2721 = And(x=w4578, y=w4579) -> (x .and. y?=w4576:bool)
                n2722 = And(x=w4576, y=w4577) -> (x .and. y?=w4574:bool)
                n2723 = And(x=w4574, y=w4575) -> (x .and. y?=w4572:bool)
                n2724 = And(x=w4572, y=w4573) -> (x .and. y?=w4570:bool)
                n2725 = And(x=w4570, y=w4571) -> (x .and. y?=w4568:bool)
                n2726 = And(x=w4568, y=w4569) -> (x .and. y?=w4567:bool)
                n2727 = And(x=w4567, y=w4597) -> (x .and. y?=w4596:bool)
                n2728 = case shown="True" w4596 {
                  tunnel: w4567 -> [w4598 _]
                  frame False {
                    n2729 = case shown="False" w4598 {
                      frame False {
                        n2730 = local write "Save JC"(TRUE) -> ()
                      }
                      frame True {
                      }
                    }
                  }
                  frame True {
                    n2731 = stacked-sequence {
                      frame #0 {
                        n2732 = String To Path(string="c:\\crabtree\\Jig Cycles\\") -> (path=w4610:path)
                        n2733 = Build Path(base path=w4610, name or relative path="jigcycles.bin") -> (appended path=w4608:path)
                        n2734 = Create Folder(path (use dialog)=w4610) -> (error out=w4612:errorcluster)  [unwired: 2 in, 2 out]
                        n2735 = local read "JIG RELAY CYCLES"() -> (w4602:T10)
                        n2736 = call <vilib>:"Clear Errors.vi"("error in (no error)"=w4612) -> ()  [unwired: 6 in, 1 out]
                        n2737 = local write "Save JC"(FALSE) -> ()
                        n2738 = Open/Create/Replace File(file path (use dialog)=w4608, operation (0:open)=T20."replace or create") -> (refnum out=w4606:refnum<file>, error out=w4607:errorcluster)  [unwired: 4 in, 1 out]
                        n2739 = Write to Binary File(file (use dialog)=w4606, data=w4602, error in=w4607) -> (refnum out=w4605:refnum<file>, error out=w4604:errorcluster)  [unwired: 3 in, 1 out]
                        n2740 = Close File(refnum=w4605, error in=w4604) -> (error out=w4603:errorcluster)  [unwired: 1 out]
                        n2741 = local write "data file error"(w4603) -> ()
                      }
                      frame #1 {
                        n2742 = local read "JIG RELAY CYCLES"() -> (w4635:T10)
                        n2743 = Unbundle By Name(w4635) -> ("LAB01-1"=w4630:dbl, "LAB01-2"=w4629:dbl, "LAB02-1"=w4627:dbl, "LAB02-2"=w4626:dbl, "LAB03-1"=w4624:dbl, "LAB03-2"=w4621:dbl, "LAB04-1"=w4620:dbl, "LAB04-2"=w4618:dbl, "LAB05-1"=w4616:dbl, "LAB05-2"=w4614:dbl)
                        n2744 = stacked-sequence {
                          tunnel: w4630 -> [w4638 _ _ _ _ _ _ _ _ _]
                          tunnel: 1000000 -> [w4641 w4651 w4661 w4671 w4681 w4691 w4701 w4711 w4721 w4731]
                          tunnel: [w4639 _ _ _ _ _ _ _ _ _] -> w4633
                          tunnel: "TEST STATION HAS REACHED 1 MILLION CYCLES, REPLACE  CONTROL RELAYS" -> [w4637 w4649 w4659 w4669 w4679 w4689 w4699 w4709 w4719 w4729]
                          tunnel: [_ w4648 _ _ _ _ _ _ _ _] -> w4631
                          tunnel: w4629 -> [_ w4647 _ _ _ _ _ _ _ _]
                          tunnel: [_ _ w4658 _ _ _ _ _ _ _] -> w4628
                          tunnel: w4627 -> [_ _ w4657 _ _ _ _ _ _ _]
                          tunnel: w4626 -> [_ _ _ w4668 _ _ _ _ _ _]
                          tunnel: [_ _ _ w4667 _ _ _ _ _ _] -> w4625
                          tunnel: w4624 -> [_ _ _ _ w4678 _ _ _ _ _]
                          tunnel: [_ _ _ _ w4677 _ _ _ _ _] -> w4623
                          tunnel: [_ _ _ _ _ w4688 _ _ _ _] -> w4622
                          tunnel: w4621 -> [_ _ _ _ _ w4687 _ _ _ _]
                          tunnel: w4620 -> [_ _ _ _ _ _ w4698 _ _ _]
                          tunnel: [_ _ _ _ _ _ w4697 _ _ _] -> w4619
                          tunnel: w4618 -> [_ _ _ _ _ _ _ w4708 _ _]
                          tunnel: [_ _ _ _ _ _ _ w4707 _ _] -> w4617
                          tunnel: w4616 -> [_ _ _ _ _ _ _ _ w4718 _]
                          tunnel: [_ _ _ _ _ _ _ _ w4717 _] -> w4615
                          tunnel: w4614 -> [_ _ _ _ _ _ _ _ _ w4728]
                          tunnel: [_ _ _ _ _ _ _ _ _ w4727] -> w4613
                          frame #0 {
                            n2745 = Greater?(x=w4638, y=w4641) -> (0:w4640:bool)
                            n2746 = case shown="True" w4640 {
                              tunnel: [w4642 0] -> w4639
                              tunnel: w4638 -> [w4642 _]
                              tunnel: w4637 -> [_ w4643]
                              frame False {
                              }
                              frame True {
                                n2747 = Concatenate Strings("LA01-1 ", w4643) -> (w4646:string)
                                n2748 = One Button Dialog(message=w4646) -> ()  [unwired: 1 in, 1 out]
                              }
                            }
                          }
                          frame #1 {
                            n2749 = Greater?(x=w4647, y=w4651) -> (0:w4650:bool)
                            n2750 = case shown="True" w4650 {
                              tunnel: [w4652 0] -> w4648
                              tunnel: w4647 -> [w4652 _]
                              tunnel: w4649 -> [_ w4653]
                              frame False {
                              }
                              frame True {
                                n2751 = Concatenate Strings("LA01-2 ", w4653) -> (w4656:string)
                                n2752 = One Button Dialog(message=w4656) -> ()  [unwired: 1 in, 1 out]
                              }
                            }
                          }
                          frame #2 {
                            n2753 = Greater?(x=w4657, y=w4661) -> (0:w4660:bool)
                            n2754 = case shown="True" w4660 {
                              tunnel: [w4662 0] -> w4658
                              tunnel: w4657 -> [w4662 _]
                              tunnel: w4659 -> [_ w4663]
                              frame False {
                              }
                              frame True {
                                n2755 = Concatenate Strings("LA02-1 ", w4663) -> (w4666:string)
                                n2756 = One Button Dialog(message=w4666) -> ()  [unwired: 1 in, 1 out]
                              }
                            }
                          }
                          frame #3 {
                            n2757 = Greater?(x=w4668, y=w4671) -> (0:w4670:bool)
                            n2758 = case shown="True" w4670 {
                              tunnel: [w4672 0] -> w4667
                              tunnel: w4668 -> [w4672 _]
                              tunnel: w4669 -> [_ w4673]
                              frame False {
                              }
                              frame True {
                                n2759 = Concatenate Strings("LA02-2 ", w4673) -> (w4676:string)
                                n2760 = One Button Dialog(message=w4676) -> ()  [unwired: 1 in, 1 out]
                              }
                            }
                          }
                          frame #4 {
                            n2761 = Greater?(x=w4678, y=w4681) -> (0:w4680:bool)
                            n2762 = case shown="True" w4680 {
                              tunnel: [w4682 0] -> w4677
                              tunnel: w4678 -> [w4682 _]
                              tunnel: w4679 -> [_ w4683]
                              frame False {
                              }
                              frame True {
                                n2763 = Concatenate Strings("LA03-1 ", w4683) -> (w4686:string)
                                n2764 = One Button Dialog(message=w4686) -> ()  [unwired: 1 in, 1 out]
                              }
                            }
                          }
                          frame #5 {
                            n2765 = Greater?(x=w4687, y=w4691) -> (0:w4690:bool)
                            n2766 = case shown="True" w4690 {
                              tunnel: [w4692 0] -> w4688
                              tunnel: w4687 -> [w4692 _]
                              tunnel: w4689 -> [_ w4693]
                              frame False {
                              }
                              frame True {
                                n2767 = Concatenate Strings("LA03-2 ", w4693) -> (w4696:string)
                                n2768 = One Button Dialog(message=w4696) -> ()  [unwired: 1 in, 1 out]
                              }
                            }
                          }
                          frame #6 {
                            n2769 = Greater?(x=w4698, y=w4701) -> (0:w4700:bool)
                            n2770 = case shown="True" w4700 {
                              tunnel: [w4702 0] -> w4697
                              tunnel: w4698 -> [w4702 _]
                              tunnel: w4699 -> [_ w4703]
                              frame False {
                              }
                              frame True {
                                n2771 = Concatenate Strings("LA04-1 ", w4703) -> (w4706:string)
                                n2772 = One Button Dialog(message=w4706) -> ()  [unwired: 1 in, 1 out]
                              }
                            }
                          }
                          frame #7 {
                            n2773 = Greater?(x=w4708, y=w4711) -> (0:w4710:bool)
                            n2774 = case shown="True" w4710 {
                              tunnel: [w4712 0] -> w4707
                              tunnel: w4708 -> [w4712 _]
                              tunnel: w4709 -> [_ w4713]
                              frame False {
                              }
                              frame True {
                                n2775 = Concatenate Strings("LA04-2 ", w4713) -> (w4716:string)
                                n2776 = One Button Dialog(message=w4716) -> ()  [unwired: 1 in, 1 out]
                              }
                            }
                          }
                          frame #8 {
                            n2777 = Greater?(x=w4718, y=w4721) -> (0:w4720:bool)
                            n2778 = case shown="True" w4720 {
                              tunnel: [w4722 0] -> w4717
                              tunnel: w4718 -> [w4722 _]
                              tunnel: w4719 -> [_ w4723]
                              frame False {
                              }
                              frame True {
                                n2779 = Concatenate Strings("LA05-1 ", w4723) -> (w4726:string)
                                n2780 = One Button Dialog(message=w4726) -> ()  [unwired: 1 in, 1 out]
                              }
                            }
                          }
                          frame #9 {
                            n2781 = Greater?(x=w4728, y=w4731) -> (0:w4730:bool)
                            n2782 = case shown="True" w4730 {
                              tunnel: [w4732 0] -> w4727
                              tunnel: w4728 -> [w4732 _]
                              tunnel: w4729 -> [_ w4733]
                              frame False {
                              }
                              frame True {
                                n2783 = Concatenate Strings("LA05-2 ", w4733) -> (w4736:string)
                                n2784 = One Button Dialog(message=w4736) -> ()  [unwired: 1 in, 1 out]
                              }
                            }
                          }
                        }
                        n2785 = Bundle By Name(cluster=w4635, "LAB01-1"=w4633, "LAB01-2"=w4631, "LAB02-1"=w4628, "LAB02-2"=w4625, "LAB03-1"=w4623, "LAB03-2"=w4622, "LAB04-1"=w4619, "LAB04-2"=w4617, "LAB05-1"=w4615, "LAB05-2"=w4613) -> (w4634:T10)
                        n2786 = local write "JIG RELAY CYCLES"(w4634) -> ()
                      }
                    }
                  }
                }
              }
            }
          }
        }
        n2787 = node-c288() -> ()  [unwired: 1 in, 1 out]
        "loops" <- w251
      }
      n2788 = node-c288(w228) -> ()  [unwired: 1 out]
    }
  }
